vi "CRYO_MASTER_FULL_old.vi"() -> ()   [LabVIEW 2017]
uses:
  LSI218Data.lvclass
  LSI336Data.lvclass
  USBData.lvclass
  6240AData.lvclass
  DMMsData.lvclass
  <vilib>/DAQmx/miscellaneous.llb/DAQmx Fill In Error Info.vi
  <vilib>/DAQmx/create/channels.llb/DAQmx Create Channel (DO-Digital Output).vi
  <vilib>/DAQmx/create/channels.llb/DAQmx Create Channel (AO-Voltage-Basic).vi
  <vilib>/express/express arith-compare/Formula/XNode/ExpressFormulaBlockNode.xnode
  <vilib>/Analysis/NI_AALBase.lvlib
panel:
  in  "Automatic \nScreenshots?":bool=TRUE
  in  "Frontpanel screenshots":bool
  in  "Screenshots interval":i64=3605
  in  "Record interval":i64=10
  out "Cycle #":u32=48
  in  "Measurement Interval (s)":dbl=1.0
  in  "Stop Button":bool
  in  "?":T1(tab)=enum."VALVE/HEATER CTRL"
  out "RUN Identifier":string="20201116_123919_RUNII"
  in  "Base Path (screenshots)":path=path "C:/LabVIEW/DATA/Google/TUCAN Experiments/KEK_cryotests_2019-2020/data/screenshots"
  out "error out (USB6210/6218 AOUT)":errorcluster
  in  "AOUT Labels":string[](array[string])=["PWR400H_I", "PMC183A_I"]
  in  "DOUT Labels":string[](array[string])=["D_V1_NO", "D_V2_NC", "D_CV1", "D_H1"]
  in  "AOUT assignment":tag[](array[tag])=["Dev1/ao0", "Dev1/ao1"]
  out "AO task out":refnum<k21>="20201116_123919_RUNII_AO"
  in  "Analog Out ON?":bool=TRUE
  in  "InstName (USB6218)":string="USB6218"
  in  "USB6218 Config":T2(array[cluster])=[{"Label"="F_1", "FileFormat"="%5.5f", "Active?"=TRUE, "Physical CH"="Dev1/ai0", " terminal\n type"=10083, "ConversionType"={"Type"=enum."SimpleProp", "ConversionParameters"=[0.0, 5.0, 0.0, 500.0]}, "VoltageLimits"=[0.0, 5.0]}, {"Label"="F_2", "FileFormat"="%5.5f", "Active?"=TRUE, "Physical CH"="Dev1/ai1", " terminal\n type"=10083, "ConversionType"={"Type"=enum."SimpleProp", "ConversionParameters"=[0.0, 5.0, 0.0, 200.0]}, "VoltageLimits"=[0.0, 5.0]}, {"Label"="F_3", "FileFormat"="%5.5f", "Active?"=TRUE, "Physical CH"="Dev1/ai2", " terminal\n type"=10083, "ConversionType"={"Type"=enum."SimpleProp", "ConversionParameters"=[0.0, 5.0, 0.0, 200.0]}, "VoltageLimits"=[0.0, 5.0]}, {"Label"="F_4", "FileFormat"="%5.5f", "Active?"=TRUE, "Physical CH"="Dev1/ai3", " terminal\n type"=10083, "ConversionType"={"Type"=enum."SimpleProp", "ConversionParameters"=[0.0, 5.0, 0.0, 500.0]}, "VoltageLimits"=[0.0, 5.0]}, {"Label"="F_5", "FileFormat"="%5.5f", "Active?"=TRUE, "Physical CH"="Dev1/ai4", " terminal\n type"=10083, "ConversionType"={"Type"=enum."SimpleProp", "ConversionParameters"=[0.0, 5.0, 0.0, 500.0]}, "VoltageLimits"=[0.0, 5.0]}, {"Label"="I_CV", "FileFormat"="%3.5f", "Active?"=TRUE, "Physical CH"="Dev1/ai5", " terminal\n type"=10083, "ConversionType"={"Type"=enum."Raw", "ConversionParameters"=[0.0, 0.0, 0.0, 0.0]}, "VoltageLimits"=[0.0, 10.0]}, {"Label"="CV1_answer", "FileFormat"="%3.5f", "Active?"=TRUE, "Physical CH"="Dev1/ai6", " terminal\n type"=10083, "ConversionType"={"Type"=enum."SimpleProp", "ConversionParameters"=[1.0, 5.0, 0.0, 100.0]}, "VoltageLimits"=[0.0, 5.0]}, {"Label"="P_Dewar", "FileFormat"="%5.5e", "Active?"=TRUE, "Physical CH"="Dev1/ai7", " terminal\n type"=10083, "ConversionType"={"Type"=enum."SimpleProp", "ConversionParameters"=[1.0, 5.0, 0.0, 200000.0]}, "VoltageLimits"=[0.0, 5.0]}] {"terminal\n type" items=["Default"=-1, "RSE"=10083, "NRSE"=10078, "Differential"=10106, "Pseudodifferential"=12529]}
  out "error out (USB6218)":errorcluster
  out "error out (USB6210/6218 DOUT)":errorcluster
  out "DOUT task out":refnum<k21>="20201116_123919_DO"
  in  "DOUT Physical CH":tag[](array[tag])=["Dev1/port1/line0", "Dev1/port1/line1", "Dev1/port1/line2", "Dev1/port1/line3"]
  in  "Digital Out ON?":bool=TRUE
  in  "USB6210 Config":T2(array[cluster])=[{"Label"="P_ins", "FileFormat"="%5.5e", "Active?"=TRUE, "Physical CH"="Dev2/ai0", " terminal\n type"=10083, "ConversionType"={"Type"=enum."CC-10_LOG", "ConversionParameters"=[0.5, 9.0, 0.0, 1.0]}, "VoltageLimits"=[0.0, 10.0]}, {"Label"="P_4Kres", "FileFormat"="%5.5e", "Active?"=TRUE, "Physical CH"="Dev2/ai1", " terminal\n type"=10083, "ConversionType"={"Type"=enum."SimpleProp", "ConversionParameters"=[1.0, 5.0, 0.0, 200000.0]}, "VoltageLimits"=[0.0, 5.0]}, {"Label"="P_3HeIN", "FileFormat"="%5.5e", "Active?"=TRUE, "Physical CH"="Dev2/ai2", " terminal\n type"=10083, "ConversionType"={"Type"=enum."SimpleProp", "ConversionParameters"=[1.0, 5.0, 0.0, 200000.0]}, "VoltageLimits"=[0.0, 5.0]}, {"Label"="P_SldRTN", "FileFormat"="%5.5e", "Active?"=TRUE, "Physical CH"="Dev2/ai3", " terminal\n type"=10083, "ConversionType"={"Type"=enum."SimpleProp", "ConversionParameters"=[1.0, 5.0, 0.0, 200000.0]}, "VoltageLimits"=[0.0, 5.0]}, {"Label"="P_3Hepot", "FileFormat"="%5.5e", "Active?"=TRUE, "Physical CH"="Dev2/ai4", " terminal\n type"=10083, "ConversionType"={"Type"=enum."SimpleProp", "ConversionParameters"=[0.0, 10.0, 0.0, 133320.0]}, "VoltageLimits"=[0.0, 10.0]}, {"Label"="P_1Kpot", "FileFormat"="%5.5e", "Active?"=TRUE, "Physical CH"="Dev2/ai5", " terminal\n type"=10083, "ConversionType"={"Type"=enum."SimpleProp", "ConversionParameters"=[0.0, 10.0, 0.0, 133320.0]}, "VoltageLimits"=[0.0, 10.0]}, {"Label"="P_Dewar(old)", "FileFormat"="%5.5e", "Active?"=FALSE, "Physical CH"="Dev2/ai6", " terminal\n type"=10083, "ConversionType"={"Type"=enum."SimpleProp", "ConversionParameters"=[1.0, 5.0, 0.0, 200000.0]}, "VoltageLimits"=[0.0, 5.0]}, {"Label"="DP_HEX4", "FileFormat"="%5.5e", "Active?"=TRUE, "Physical CH"="Dev2/ai7", " terminal\n type"=10083, "ConversionType"={"Type"=enum."SimpleProp", "ConversionParameters"=[1.0, 5.0, 0.0, 1000.0]}, "VoltageLimits"=[0.0, 5.0]}, {"Label"="DP_HEX5", "FileFormat"="%5.5e", "Active?"=TRUE, "Physical CH"="Dev2/ai8", " terminal\n type"=10083, "ConversionType"={"Type"=enum."SimpleProp", "ConversionParameters"=[1.0, 5.0, 0.0, 20000.0]}, "VoltageLimits"=[0.0, 5.0]}, {"Label"="L1", "FileFormat"="%5.5f", "Active?"=TRUE, "Physical CH"="Dev2/ai9", " terminal\n type"=10083, "ConversionType"={"Type"=enum."SimpleProp", "ConversionParameters"=[0.0, 10.0, 0.0, 100.0]}, "VoltageLimits"=[0.0, 10.0]}, {"Label"="L2-1", "FileFormat"="%5.5f", "Active?"=TRUE, "Physical CH"="Dev2/ai10", " terminal\n type"=10083, "ConversionType"={"Type"=enum."SimpleProp", "ConversionParameters"=[0.0, 10.0, 0.0, 100.0]}, "VoltageLimits"=[0.0, 10.0]}, {"Label"="L2-2", "FileFormat"="%5.5f", "Active?"=TRUE, "Physical CH"="Dev2/ai11", " terminal\n type"=10083, "ConversionType"={"Type"=enum."SimpleProp", "ConversionParameters"=[0.0, 10.0, 0.0, 100.0]}, "VoltageLimits"=[0.0, 10.0]}, {"Label"="L3", "FileFormat"="%5.5f", "Active?"=TRUE, "Physical CH"="Dev2/ai12", " terminal\n type"=10083, "ConversionType"={"Type"=enum."SimpleProp", "ConversionParameters"=[0.0, 10.0, 0.0, 100.0]}, "VoltageLimits"=[0.0, 10.0]}, {"Label"="P_HEX7OUT", "FileFormat"="%5.5e", "Active?"=TRUE, "Physical CH"="Dev2/ai13", " terminal\n type"=10083, "ConversionType"={"Type"=enum."SimpleProp", "ConversionParameters"=[1.0, 5.0, 0.0, 200000.0]}, "VoltageLimits"=[0.0, 5.0]}, {"Label"="P_IP", "FileFormat"="%5.5e", "Active?"=TRUE, "Physical CH"="Dev2/ai14", " terminal\n type"=10083, "ConversionType"={"Type"=enum."CC-10_LOG", "ConversionParameters"=[0.5, 9.0, 0.0, 1.0]}, "VoltageLimits"=[0.0, 10.0]}, {"Label"="V_H1", "FileFormat"="%3.5f", "Active?"=TRUE, "Physical CH"="Dev2/ai15", " terminal\n type"=10083, "ConversionType"={"Type"=enum."Raw", "ConversionParameters"=[0.0, 1.0, 0.0, 1.0]}, "VoltageLimits"=[0.0, 10.0]}] {"terminal\n type" items=["Default"=-1, "RSE"=10083, "NRSE"=10078, "Differential"=10106, "Pseudodifferential"=12529]}
  in  "RUN label":string="RUNII"
  in  "Base Path":path=path "C:/LabVIEW/DATA/RUN_2"
  in  "InstName (USB6210)":string="USB6210"
  out "error out (USB6210)":errorcluster
  out "File Refn USB AO":refnum<file>
  out "File Refn USB DO":refnum<file>
  out "error out (LSI336)":errorcluster
  in  "InstName (LSI336)":string="LSI336"
  in  "FileFormat (336)":string="%4.4f"
  in  "LSI336Settings(X,Y)":T3(array[cluster])=[{"LSIName"="LSi336X", "Labels"=["T1K3-1", "T1K3-2", "T3He5", "T3He8"], "SensorLocations"=[enum."T1K3-1", enum."T1K3-2", enum."T3He5", enum."T3He8"], "Active?"=TRUE, "VISA res. name"="GPIB0::6::INSTR"}, {"LSIName"="LSi336Y", "Labels"=["T3He6-1", "T3He6-2", "T3He7-1", "T3He7-2"], "SensorLocations"=[enum."T3He6-1", enum."T3He6-2", enum."T3He7-1", enum."T3He7-2"], "Active?"=TRUE, "VISA res. name"="GPIB0::2::INSTR"}]
  in  "FileFormat (218)":string="%4.4f"
  in  "InstName (LSI218)":string="LSI218"
  in  "LSI218Settings(A-F)":T3(array[cluster])=[{"LSIName"="LSI218A", "Labels"=["T3He10", "T3He1-1", "TTH3", "TTH4", "TTH1", "TTH2", "T4He1", "T1K1"], "SensorLocations"=[enum."T3He10", enum."T3He1-1", enum."TTH3", enum."TTH4", enum."TTH1", enum."TTH2", enum."T4He1", enum."T1K1"], "Active?"=TRUE, "VISA res. name"="GPIB0::7::INSTR"}, {"LSIName"="LSI218B", "Labels"=["N.C.", "N.C.", "N.C.", "N.C.", "T3He2-1", "T3He2-2", "T3He3", "T3He1-4"], "SensorLocations"=[enum."N.C.", enum."N.C.", enum."N.C.", enum."N.C.", enum."T3He2-1", enum."T3He2-2", enum."T3He3", enum."T3He1-4"], "Active?"=TRUE, "VISA res. name"="GPIB0::4::INSTR"}, {"LSIName"="LSI218C", "Labels"=["T4He3-1", "T4He3-2", "T4He3-3", "T4He3-4", "T4He2-1", "T4He2-2", "T4He4", "T4He5"], "SensorLocations"=[enum."T4He3-1", enum."T4He3-2", enum."T4He3-3", enum."T4He3-4", enum."T4He2-1", enum."T4He2-2", enum."T4He4", enum."T4He5"], "Active?"=TRUE, "VISA res. name"="GPIB0::3::INSTR"}, {"LSIName"="LSI218D", "Labels"=["T4He6", "T4He9", "T3He1-2", "T3He1-3", "T4He7", "T4He8", "T4He10", "T1K6"], "SensorLocations"=[enum."T4He6", enum."T4He9", enum."T3He1-2", enum."T3He1-3", enum."T4He7", enum."T4He8", enum."T4He10", enum."T1K6"], "Active?"=TRUE, "VISA res. name"="GPIB0::5::INSTR"}, {"LSIName"="LSI218E", "Labels"=["TIP1", "N.C.", "TIP2", "N.C.", "TIP3", "TIP4", "TIP5", "N.C."], "SensorLocations"=[enum."TIP1", enum."N.C.", enum."TIP2", enum."N.C.", enum."TIP3", enum."TIP4", enum."TIP5", enum."N.C."], "Active?"=TRUE, "VISA res. name"="GPIB0::11::INSTR"}, {"LSIName"="LSI218F", "Labels"=["T1K2", "T1K4", "T1K5", "T3He4", "T3He9", "TIP6", "N.C.", "N.C."], "SensorLocations"=[enum."T1K2", enum."T1K4", enum."T1K5", enum."T3He4", enum."T3He9", enum."TIP6", enum."N.C.", enum."N.C."], "Active?"=TRUE, "VISA res. name"="GPIB0::8::INSTR"}]
  out "error out (LSI218)":errorcluster
  out "RUN Identifier 2":string="20201116_123919_RUNII" caption="RUN Identifier"
  out "Graph 3":T4(graph)=[{"TimeArray"=[timestamp(3688342761.3994594 s since 1904-01-01), timestamp(3688342762.4680505 s since 1904-01-01), timestamp(3688342763.4675946 s since 1904-01-01), timestamp(3688342764.4676514 s since 1904-01-01), timestamp(3688342765.4686737 s since 1904-01-01), timestamp(3688342766.469984 s since 1904-01-01), timestamp(3688342767.470159 s since 1904-01-01), timestamp(3688342768.47213 s since 1904-01-01), timestamp(3688342769.8238606 s since 1904-01-01), timestamp(3688342770.8245606 s since 1904-01-01), timestamp(3688342771.8237367 s since 1904-01-01), timestamp(3688342772.8240294 s since 1904-01-01), timestamp(3688342773.823701 s since 1904-01-01), timestamp(3688342774.8247466 s since 1904-01-01), timestamp(3688342775.8255386 s since 1904-01-01), timestamp(3688342776.8254576 s since 1904-01-01), timestamp(3688342777.825836 s since 1904-01-01), timestamp(3688342778.8261266 s since 1904-01-01), timestamp(3688342779.826581 s since 1904-01-01), timestamp(3688342780.8273554 s since 1904-01-01), timestamp(3688342781.826626 s since 1904-01-01), timestamp(3688342782.8268657 s since 1904-01-01), timestamp(3688342783.8258696 s since 1904-01-01), timestamp(3688342784.825906 s since 1904-01-01), timestamp(3688342785.825819 s since 1904-01-01), timestamp(3688342786.827296 s since 1904-01-01), timestamp(3688342787.829418 s since 1904-01-01), timestamp(3688342788.8291 s since 1904-01-01), timestamp(3688342789.8296633 s since 1904-01-01), timestamp(3688342790.829848 s since 1904-01-01), timestamp(3688342791.829139 s since 1904-01-01), timestamp(3688342792.8296423 s since 1904-01-01), timestamp(3688342793.831637 s since 1904-01-01), timestamp(3688342794.8306546 s since 1904-01-01), timestamp(3688342795.829824 s since 1904-01-01), timestamp(3688342796.830819 s since 1904-01-01), timestamp(3688342798.0479465 s since 1904-01-01), timestamp(3688342799.047389 s since 1904-01-01), timestamp(3688342800.047347 s since 1904-01-01), timestamp(3688342801.0487537 s since 1904-01-01), timestamp(3688342802.047892 s since 1904-01-01), timestamp(3688342803.047963 s since 1904-01-01), timestamp(3688342804.0478578 s since 1904-01-01), timestamp(3688342805.0488462 s since 1904-01-01), timestamp(3688342806.0497985 s since 1904-01-01), timestamp(3688342807.0502543 s since 1904-01-01), timestamp(3688342808.049495 s since 1904-01-01), timestamp(3688342809.0488415 s since 1904-01-01)], "DataArray"=[1.6108772064644081, 1.4727858772132323, 1.1538606722402807, 1.28208833184731, 1.7785595282840228, 1.0256330125875925, 1.6897865359634758, 0.7987686882211862, 0.8809659041921434, 1.3248308864318687, 1.1111181148543707, 1.2492094468908674, 0.8415112314716219, 1.2031790040723394, 0.8645264589454551, 1.702938093987531, 0.8711022389190866, 1.7686958683374852, 1.6569076467914272, 1.3248308880823247, 1.1275575630145545, 1.9002114182612835, 0.9006932376829025, 1.4892253229450763, 0.976314680985114, 1.5221042083621306, 0.6606773585654712, 1.3807249976849918, 1.4366191035745401, 1.4333312156222522, 1.4366191049902393, 1.8180141959680036, 1.1505727850948726, 0.7330109051260003, 1.7917110860245415, 1.1538606736707524, 1.5056647632332703, 0.9269963444433174, 1.7128017563643017, 1.449770660594799, 1.5681346563036929, 0.8283596875451974, 0.6902683536947601, 0.8415112382027863, 1.6108772080587708, 1.7785595285218954, 1.5418315461474963, 1.236057890033779]}, {"TimeArray"=[timestamp(3688342761.3994594 s since 1904-01-01), timestamp(3688342762.4680505 s since 1904-01-01), timestamp(3688342763.4675946 s since 1904-01-01), timestamp(3688342764.4676514 s since 1904-01-01), timestamp(3688342765.4686737 s since 1904-01-01), timestamp(3688342766.469984 s since 1904-01-01), timestamp(3688342767.470159 s since 1904-01-01), timestamp(3688342768.47213 s since 1904-01-01), timestamp(3688342769.8238606 s since 1904-01-01), timestamp(3688342770.8245606 s since 1904-01-01), timestamp(3688342771.8237367 s since 1904-01-01), timestamp(3688342772.8240294 s since 1904-01-01), timestamp(3688342773.823701 s since 1904-01-01), timestamp(3688342774.8247466 s since 1904-01-01), timestamp(3688342775.8255386 s since 1904-01-01), timestamp(3688342776.8254576 s since 1904-01-01), timestamp(3688342777.825836 s since 1904-01-01), timestamp(3688342778.8261266 s since 1904-01-01), timestamp(3688342779.826581 s since 1904-01-01), timestamp(3688342780.8273554 s since 1904-01-01), timestamp(3688342781.826626 s since 1904-01-01), timestamp(3688342782.8268657 s since 1904-01-01), timestamp(3688342783.8258696 s since 1904-01-01), timestamp(3688342784.825906 s since 1904-01-01), timestamp(3688342785.825819 s since 1904-01-01), timestamp(3688342786.827296 s since 1904-01-01), timestamp(3688342787.829418 s since 1904-01-01), timestamp(3688342788.8291 s since 1904-01-01), timestamp(3688342789.8296633 s since 1904-01-01), timestamp(3688342790.829848 s since 1904-01-01), timestamp(3688342791.829139 s since 1904-01-01), timestamp(3688342792.8296423 s since 1904-01-01), timestamp(3688342793.831637 s since 1904-01-01), timestamp(3688342794.8306546 s since 1904-01-01), timestamp(3688342795.829824 s since 1904-01-01), timestamp(3688342796.830819 s since 1904-01-01), timestamp(3688342798.0479465 s since 1904-01-01), timestamp(3688342799.047389 s since 1904-01-01), timestamp(3688342800.047347 s since 1904-01-01), timestamp(3688342801.0487537 s since 1904-01-01), timestamp(3688342802.047892 s since 1904-01-01), timestamp(3688342803.047963 s since 1904-01-01), timestamp(3688342804.0478578 s since 1904-01-01), timestamp(3688342805.0488462 s since 1904-01-01), timestamp(3688342806.0497985 s since 1904-01-01), timestamp(3688342807.0502543 s since 1904-01-01), timestamp(3688342808.049495 s since 1904-01-01), timestamp(3688342809.0488415 s since 1904-01-01)], "DataArray"=[0.11960383538282587, 0.12354930467748859, 0.16957974721691593, 0.3168771630474284, 0.10513712477879456, 0.14327663545986008, -0.056627000773362635, 0.020967174002287814, -0.09345135530386744, 0.06173699470083205, 0.40630773776805706, 0.03543388286570193, -0.015857179683996525, 0.43787147030971574, 0.1353857036464915, 0.2813679649924926, 0.06305215107903633, 0.3707985383052794, 0.16168881415673564, 0.05910668305857897, 0.07488855063108274, -0.05925731348622698, 0.08804010289037423, 0.3655379148996485, 0.152482725397677, 0.42603506628065013, 0.3537015180628369, 0.3168771643021264, 0.084094637595031, 0.10776743816760453, 0.31687716261188875, 0.2116647226957259, 0.007815619052014, 0.09724619411048441, -0.14868788814255518, 0.26032547695418784, 0.21955565491787643, 0.26690125441051665, 0.4457624026836094, 0.1774706797542605, 0.114343214789281, 0.0380641963143703, -0.1026574444303443, 0.013076240296714503, 0.1840464575827528, 0.055161216108252864, 0.06042183752267505, 0.32608325247707837]}, {"TimeArray"=[timestamp(3688342761.3994594 s since 1904-01-01), timestamp(3688342762.4680505 s since 1904-01-01), timestamp(3688342763.4675946 s since 1904-01-01), timestamp(3688342764.4676514 s since 1904-01-01), timestamp(3688342765.4686737 s since 1904-01-01), timestamp(3688342766.469984 s since 1904-01-01), timestamp(3688342767.470159 s since 1904-01-01), timestamp(3688342768.47213 s since 1904-01-01), timestamp(3688342769.8238606 s since 1904-01-01), timestamp(3688342770.8245606 s since 1904-01-01), timestamp(3688342771.8237367 s since 1904-01-01), timestamp(3688342772.8240294 s since 1904-01-01), timestamp(3688342773.823701 s since 1904-01-01), timestamp(3688342774.8247466 s since 1904-01-01), timestamp(3688342775.8255386 s since 1904-01-01), timestamp(3688342776.8254576 s since 1904-01-01), timestamp(3688342777.825836 s since 1904-01-01), timestamp(3688342778.8261266 s since 1904-01-01), timestamp(3688342779.826581 s since 1904-01-01), timestamp(3688342780.8273554 s since 1904-01-01), timestamp(3688342781.826626 s since 1904-01-01), timestamp(3688342782.8268657 s since 1904-01-01), timestamp(3688342783.8258696 s since 1904-01-01), timestamp(3688342784.825906 s since 1904-01-01), timestamp(3688342785.825819 s since 1904-01-01), timestamp(3688342786.827296 s since 1904-01-01), timestamp(3688342787.829418 s since 1904-01-01), timestamp(3688342788.8291 s since 1904-01-01), timestamp(3688342789.8296633 s since 1904-01-01), timestamp(3688342790.829848 s since 1904-01-01), timestamp(3688342791.829139 s since 1904-01-01), timestamp(3688342792.8296423 s since 1904-01-01), timestamp(3688342793.831637 s since 1904-01-01), timestamp(3688342794.8306546 s since 1904-01-01), timestamp(3688342795.829824 s since 1904-01-01), timestamp(3688342796.830819 s since 1904-01-01), timestamp(3688342798.0479465 s since 1904-01-01), timestamp(3688342799.047389 s since 1904-01-01), timestamp(3688342800.047347 s since 1904-01-01), timestamp(3688342801.0487537 s since 1904-01-01), timestamp(3688342802.047892 s since 1904-01-01), timestamp(3688342803.047963 s since 1904-01-01), timestamp(3688342804.0478578 s since 1904-01-01), timestamp(3688342805.0488462 s since 1904-01-01), timestamp(3688342806.0497985 s since 1904-01-01), timestamp(3688342807.0502543 s since 1904-01-01), timestamp(3688342808.049495 s since 1904-01-01), timestamp(3688342809.0488415 s since 1904-01-01)], "DataArray"=[0.19719801289443417, 0.3234529413982592, 0.41025320470314475, 0.35501667385679236, 0.08277948336150942, 0.1866767679337933, 0.03674904061937184, 0.11434321402546777, 0.22481627750062233, 0.47995644469336163, 0.5549203093056583, 0.29320436503981057, 0.10382197109764235, 0.46680489114965856, 0.36553791656749685, 0.37605916077701856, 0.3721136950929542, 0.09856134863620536, 0.282683121071797, 0.16957974638882117, 0.28268311956998077, -0.015857180631994205, 0.30241045223936386, 0.13275539146300835, 0.19325254588015484, 0.3984168045158203, 0.5391384442450727, 0.3971016486305656, 0.17878583614480142, 0.43129569272124, 0.47469582441796065, -0.01848749114242587, 0.11039774877546588, 0.31950747311050975, 0.2392829882600312, 0.5102050229214992, 0.24717392215355527, 0.5036292443284728, 0.30372560924621067, 0.293204364993237, 0.19851316847145212, 0.7219450557978133, 0.04332481675159766, 0.4273502264943859, 0.27347703224226, -0.006651091545683108, 0.16300396733772582, 0.27610734304609297]}, {"TimeArray"=[timestamp(3688342761.3994594 s since 1904-01-01), timestamp(3688342762.4680505 s since 1904-01-01), timestamp(3688342763.4675946 s since 1904-01-01), timestamp(3688342764.4676514 s since 1904-01-01), timestamp(3688342765.4686737 s since 1904-01-01), timestamp(3688342766.469984 s since 1904-01-01), timestamp(3688342767.470159 s since 1904-01-01), timestamp(3688342768.47213 s since 1904-01-01), timestamp(3688342769.8238606 s since 1904-01-01), timestamp(3688342770.8245606 s since 1904-01-01), timestamp(3688342771.8237367 s since 1904-01-01), timestamp(3688342772.8240294 s since 1904-01-01), timestamp(3688342773.823701 s since 1904-01-01), timestamp(3688342774.8247466 s since 1904-01-01), timestamp(3688342775.8255386 s since 1904-01-01), timestamp(3688342776.8254576 s since 1904-01-01), timestamp(3688342777.825836 s since 1904-01-01), timestamp(3688342778.8261266 s since 1904-01-01), timestamp(3688342779.826581 s since 1904-01-01), timestamp(3688342780.8273554 s since 1904-01-01), timestamp(3688342781.826626 s since 1904-01-01), timestamp(3688342782.8268657 s since 1904-01-01), timestamp(3688342783.8258696 s since 1904-01-01), timestamp(3688342784.825906 s since 1904-01-01), timestamp(3688342785.825819 s since 1904-01-01), timestamp(3688342786.827296 s since 1904-01-01), timestamp(3688342787.829418 s since 1904-01-01), timestamp(3688342788.8291 s since 1904-01-01), timestamp(3688342789.8296633 s since 1904-01-01), timestamp(3688342790.829848 s since 1904-01-01), timestamp(3688342791.829139 s since 1904-01-01), timestamp(3688342792.8296423 s since 1904-01-01), timestamp(3688342793.831637 s since 1904-01-01), timestamp(3688342794.8306546 s since 1904-01-01), timestamp(3688342795.829824 s since 1904-01-01), timestamp(3688342796.830819 s since 1904-01-01), timestamp(3688342798.0479465 s since 1904-01-01), timestamp(3688342799.047389 s since 1904-01-01), timestamp(3688342800.047347 s since 1904-01-01), timestamp(3688342801.0487537 s since 1904-01-01), timestamp(3688342802.047892 s since 1904-01-01), timestamp(3688342803.047963 s since 1904-01-01), timestamp(3688342804.0478578 s since 1904-01-01), timestamp(3688342805.0488462 s since 1904-01-01), timestamp(3688342806.0497985 s since 1904-01-01), timestamp(3688342807.0502543 s since 1904-01-01), timestamp(3688342808.049495 s since 1904-01-01), timestamp(3688342809.0488415 s since 1904-01-01)], "DataArray"=[-8.8117305470801, -8.611169313327453, -8.785427429519835, -9.633702805164498, -8.772275883378784, -8.920230878437964, -7.933864177873465, -7.756318171036431, -8.183743745254892, -8.699942315071391, -8.959685549532404, -8.683502874153833, -8.36128975034523, -8.739396983469396, -8.20675896381145, -8.427047526402006, -7.808924396791847, -9.295050229778404, -8.23634996633052, -8.41718386312757, -8.07195551659595, -7.6774088373668965, -7.749742396156548, -8.279092521170103, -8.10483440461572, -8.831457878899462, -9.27532289384464, -9.120792109971513, -7.831939618345252, -9.48574779160318, -9.683021136151854, -8.413895971885601, -8.085107074198529, -7.924000508555038, -7.595211611507303, -8.81830632687022, -8.31525930182675, -8.736109095904842, -9.702748470003478, -9.081337441634272, -7.989758296191559, -8.542123642001318, -7.108604041882277, -7.187513380811203, -9.581096575868242, -8.374441303730787, -8.496093212698424, -8.229774188754428]}, {"TimeArray"=[timestamp(3688342761.3994594 s since 1904-01-01), timestamp(3688342762.4680505 s since 1904-01-01), timestamp(3688342763.4675946 s since 1904-01-01), timestamp(3688342764.4676514 s since 1904-01-01), timestamp(3688342765.4686737 s since 1904-01-01), timestamp(3688342766.469984 s since 1904-01-01), timestamp(3688342767.470159 s since 1904-01-01), timestamp(3688342768.47213 s since 1904-01-01), timestamp(3688342769.8238606 s since 1904-01-01), timestamp(3688342770.8245606 s since 1904-01-01), timestamp(3688342771.8237367 s since 1904-01-01), timestamp(3688342772.8240294 s since 1904-01-01), timestamp(3688342773.823701 s since 1904-01-01), timestamp(3688342774.8247466 s since 1904-01-01), timestamp(3688342775.8255386 s since 1904-01-01), timestamp(3688342776.8254576 s since 1904-01-01), timestamp(3688342777.825836 s since 1904-01-01), timestamp(3688342778.8261266 s since 1904-01-01), timestamp(3688342779.826581 s since 1904-01-01), timestamp(3688342780.8273554 s since 1904-01-01), timestamp(3688342781.826626 s since 1904-01-01), timestamp(3688342782.8268657 s since 1904-01-01), timestamp(3688342783.8258696 s since 1904-01-01), timestamp(3688342784.825906 s since 1904-01-01), timestamp(3688342785.825819 s since 1904-01-01), timestamp(3688342786.827296 s since 1904-01-01), timestamp(3688342787.829418 s since 1904-01-01), timestamp(3688342788.8291 s since 1904-01-01), timestamp(3688342789.8296633 s since 1904-01-01), timestamp(3688342790.829848 s since 1904-01-01), timestamp(3688342791.829139 s since 1904-01-01), timestamp(3688342792.8296423 s since 1904-01-01), timestamp(3688342793.831637 s since 1904-01-01), timestamp(3688342794.8306546 s since 1904-01-01), timestamp(3688342795.829824 s since 1904-01-01), timestamp(3688342796.830819 s since 1904-01-01), timestamp(3688342798.0479465 s since 1904-01-01), timestamp(3688342799.047389 s since 1904-01-01), timestamp(3688342800.047347 s since 1904-01-01), timestamp(3688342801.0487537 s since 1904-01-01), timestamp(3688342802.047892 s since 1904-01-01), timestamp(3688342803.047963 s since 1904-01-01), timestamp(3688342804.0478578 s since 1904-01-01), timestamp(3688342805.0488462 s since 1904-01-01), timestamp(3688342806.0497985 s since 1904-01-01), timestamp(3688342807.0502543 s since 1904-01-01), timestamp(3688342808.049495 s since 1904-01-01), timestamp(3688342809.0488415 s since 1904-01-01)], "DataArray"=[25.42834097532839, 24.86611211032151, 25.507250294604013, 25.129143157252333, 25.579583820368846, 25.043658067331226, 26.286479774866073, 25.80316022068847, 26.358813307865177, 24.87597576883828, 24.58006584160019, 25.240931356366875, 25.586159610342886, 24.67870248438199, 25.918236307585516, 25.471083526447114, 25.704523579221565, 24.5636263966979, 25.540129173409465, 25.257370793132907, 25.448068304775234, 26.15496424988605, 25.28367389255778, 25.826175439613337, 25.58287171880491, 24.889127324747573, 23.883033555139072, 24.55376273747171, 25.990569845070805, 25.408613646662076, 24.132913048272638, 25.536841282754608, 26.227297790428917, 26.043176056850676, 25.582871718122018, 24.68856614483606, 25.6552052559632, 24.58006583695763, 24.626096274245686, 24.879263660377774, 25.740690349871215, 24.504444409982383, 26.365389089597326, 26.010297173875607, 25.066673284606118, 25.717675133782908, 25.54341705535066, 25.19818880738261]}, {"TimeArray"=[timestamp(3688342761.3994594 s since 1904-01-01), timestamp(3688342762.4680505 s since 1904-01-01), timestamp(3688342763.4675946 s since 1904-01-01), timestamp(3688342764.4676514 s since 1904-01-01), timestamp(3688342765.4686737 s since 1904-01-01), timestamp(3688342766.469984 s since 1904-01-01), timestamp(3688342767.470159 s since 1904-01-01), timestamp(3688342768.47213 s since 1904-01-01), timestamp(3688342769.8238606 s since 1904-01-01), timestamp(3688342770.8245606 s since 1904-01-01), timestamp(3688342771.8237367 s since 1904-01-01), timestamp(3688342772.8240294 s since 1904-01-01), timestamp(3688342773.823701 s since 1904-01-01), timestamp(3688342774.8247466 s since 1904-01-01), timestamp(3688342775.8255386 s since 1904-01-01), timestamp(3688342776.8254576 s since 1904-01-01), timestamp(3688342777.825836 s since 1904-01-01), timestamp(3688342778.8261266 s since 1904-01-01), timestamp(3688342779.826581 s since 1904-01-01), timestamp(3688342780.8273554 s since 1904-01-01), timestamp(3688342781.826626 s since 1904-01-01), timestamp(3688342782.8268657 s since 1904-01-01), timestamp(3688342783.8258696 s since 1904-01-01), timestamp(3688342784.825906 s since 1904-01-01), timestamp(3688342785.825819 s since 1904-01-01), timestamp(3688342786.827296 s since 1904-01-01), timestamp(3688342787.829418 s since 1904-01-01), timestamp(3688342788.8291 s since 1904-01-01), timestamp(3688342789.8296633 s since 1904-01-01), timestamp(3688342790.829848 s since 1904-01-01), timestamp(3688342791.829139 s since 1904-01-01), timestamp(3688342792.8296423 s since 1904-01-01), timestamp(3688342793.831637 s since 1904-01-01), timestamp(3688342794.8306546 s since 1904-01-01), timestamp(3688342795.829824 s since 1904-01-01), timestamp(3688342796.830819 s since 1904-01-01), timestamp(3688342798.0479465 s since 1904-01-01), timestamp(3688342799.047389 s since 1904-01-01), timestamp(3688342800.047347 s since 1904-01-01), timestamp(3688342801.0487537 s since 1904-01-01), timestamp(3688342802.047892 s since 1904-01-01), timestamp(3688342803.047963 s since 1904-01-01), timestamp(3688342804.0478578 s since 1904-01-01), timestamp(3688342805.0488462 s since 1904-01-01), timestamp(3688342806.0497985 s since 1904-01-01), timestamp(3688342807.0502543 s since 1904-01-01), timestamp(3688342808.049495 s since 1904-01-01), timestamp(3688342809.0488415 s since 1904-01-01)], "DataArray"=[-0.005193268383660984, -0.004930182610743403, -0.007561039877274372, -0.007824125581124733, 0.0005946176173860784, 0.0009892461834888455, -0.008350297054780385, 0.0020415890984940926, -0.010586525749650461, -0.0165717259712373, -0.004009382596067648, 0.0044751320298084376, -0.006508696976678557, -0.003746296849714206, 0.01644553246086406, 0.018418675382905786, 0.006777132117386087, 0.022299189798510845, 0.01986564686698383, 0.0103945608264739, 0.015722046716312395, 0.015590503844082615, 0.007961017869320528, 0.01703747532627037, 0.019668332547804077, 0.02052336112517377, 0.01598513245021415, 0.018089818237418558, 0.0174978753332058, 0.019339475400628702, 0.013946218060777175, 0.024206561247617227, 0.027823989933317538, 0.019142161099012175, 0.008355646456888863, 0.021838789776919672, 0.016379761005772927, 0.019931418285493475, 0.028284389977942748, 0.026377018469227166, 0.018155589606191617, -0.0012469824561334246, 0.009473760777586143, 0.010328789405961273, 0.025850847009992406, 0.020720675452570142, 0.021509932578620914, 0.004212046304753189]}, {"TimeArray"=[timestamp(3688342761.3994594 s since 1904-01-01), timestamp(3688342762.4680505 s since 1904-01-01), timestamp(3688342763.4675946 s since 1904-01-01), timestamp(3688342764.4676514 s since 1904-01-01), timestamp(3688342765.4686737 s since 1904-01-01), timestamp(3688342766.469984 s since 1904-01-01), timestamp(3688342767.470159 s since 1904-01-01), timestamp(3688342768.47213 s since 1904-01-01), timestamp(3688342769.8238606 s since 1904-01-01), timestamp(3688342770.8245606 s since 1904-01-01), timestamp(3688342771.8237367 s since 1904-01-01), timestamp(3688342772.8240294 s since 1904-01-01), timestamp(3688342773.823701 s since 1904-01-01), timestamp(3688342774.8247466 s since 1904-01-01), timestamp(3688342775.8255386 s since 1904-01-01), timestamp(3688342776.8254576 s since 1904-01-01), timestamp(3688342777.825836 s since 1904-01-01), timestamp(3688342778.8261266 s since 1904-01-01), timestamp(3688342779.826581 s since 1904-01-01), timestamp(3688342780.8273554 s since 1904-01-01), timestamp(3688342781.826626 s since 1904-01-01), timestamp(3688342782.8268657 s since 1904-01-01), timestamp(3688342783.8258696 s since 1904-01-01), timestamp(3688342784.825906 s since 1904-01-01), timestamp(3688342785.825819 s since 1904-01-01), timestamp(3688342786.827296 s since 1904-01-01), timestamp(3688342787.829418 s since 1904-01-01), timestamp(3688342788.8291 s since 1904-01-01), timestamp(3688342789.8296633 s since 1904-01-01), timestamp(3688342790.829848 s since 1904-01-01), timestamp(3688342791.829139 s since 1904-01-01), timestamp(3688342792.8296423 s since 1904-01-01), timestamp(3688342793.831637 s since 1904-01-01), timestamp(3688342794.8306546 s since 1904-01-01), timestamp(3688342795.829824 s since 1904-01-01), timestamp(3688342796.830819 s since 1904-01-01), timestamp(3688342798.0479465 s since 1904-01-01), timestamp(3688342799.047389 s since 1904-01-01), timestamp(3688342800.047347 s since 1904-01-01), timestamp(3688342801.0487537 s since 1904-01-01), timestamp(3688342802.047892 s since 1904-01-01), timestamp(3688342803.047963 s since 1904-01-01), timestamp(3688342804.0478578 s since 1904-01-01), timestamp(3688342805.0488462 s since 1904-01-01), timestamp(3688342806.0497985 s since 1904-01-01), timestamp(3688342807.0502543 s since 1904-01-01), timestamp(3688342808.049495 s since 1904-01-01), timestamp(3688342809.0488415 s since 1904-01-01)], "DataArray"=[101763.76778005705, 101441.5552574628, 101712.80559595322, 101605.94940418932, 102048.16965721699, 102148.45008278092, 101822.94967516132, 102820.8221420409, 101765.41172578087, 101411.96430850294, 102064.60907132704, 102385.17765603494, 102021.8665918818, 102113.92731541373, 102342.43517662614, 101952.82105008146, 101640.47217360992, 101982.41199679034, 101883.77551160513, 101275.51716733717, 101554.98721685537, 101314.97176370079, 101619.10093268016, 102457.51108097668, 101859.11638700173, 101990.63170464033, 101625.67670103439, 101686.50253584248, 102230.6471546882, 102110.63943060939, 101563.20692537277, 102686.0189403731, 102615.32945958685, 102125.43490180184, 101106.19119599719, 101730.88895455986, 101977.48017289658, 101563.20692370029, 102720.54171254052, 101992.275644626, 101596.08575338517, 101114.41090367321, 101762.12384323322, 101748.97231164195, 102429.56407407322, 102166.53343982312, 102163.24555458283, 102197.76832945186]}] caption="XY Graph"
  out "Graph 1":T4(graph)=[{"TimeArray"=[timestamp(3688342761.39444 s since 1904-01-01), timestamp(3688342762.463024 s since 1904-01-01), timestamp(3688342763.463638 s since 1904-01-01), timestamp(3688342764.463637 s since 1904-01-01), timestamp(3688342765.464684 s since 1904-01-01), timestamp(3688342766.465038 s since 1904-01-01), timestamp(3688342767.4661665 s since 1904-01-01), timestamp(3688342768.4671426 s since 1904-01-01), timestamp(3688342769.818876 s since 1904-01-01), timestamp(3688342770.819616 s since 1904-01-01), timestamp(3688342771.819715 s since 1904-01-01), timestamp(3688342772.8190737 s since 1904-01-01), timestamp(3688342773.819743 s since 1904-01-01), timestamp(3688342774.820112 s since 1904-01-01), timestamp(3688342775.820584 s since 1904-01-01), timestamp(3688342776.8214664 s since 1904-01-01), timestamp(3688342777.821848 s since 1904-01-01), timestamp(3688342778.822177 s since 1904-01-01), timestamp(3688342779.8225975 s since 1904-01-01), timestamp(3688342780.8223686 s since 1904-01-01), timestamp(3688342781.8226385 s since 1904-01-01), timestamp(3688342782.8219137 s since 1904-01-01), timestamp(3688342783.8218846 s since 1904-01-01), timestamp(3688342784.821887 s since 1904-01-01), timestamp(3688342785.821828 s since 1904-01-01), timestamp(3688342786.8223386 s since 1904-01-01), timestamp(3688342787.825325 s since 1904-01-01), timestamp(3688342788.8251424 s since 1904-01-01), timestamp(3688342789.825672 s since 1904-01-01), timestamp(3688342790.824856 s since 1904-01-01), timestamp(3688342791.8251505 s since 1904-01-01), timestamp(3688342792.8256593 s since 1904-01-01), timestamp(3688342793.8266897 s since 1904-01-01), timestamp(3688342794.826625 s since 1904-01-01), timestamp(3688342795.825836 s since 1904-01-01), timestamp(3688342796.826832 s since 1904-01-01), timestamp(3688342798.0429673 s since 1904-01-01), timestamp(3688342799.0433993 s since 1904-01-01), timestamp(3688342800.043396 s since 1904-01-01), timestamp(3688342801.0437655 s since 1904-01-01), timestamp(3688342802.0438714 s since 1904-01-01), timestamp(3688342803.043973 s since 1904-01-01), timestamp(3688342804.043901 s since 1904-01-01), timestamp(3688342805.044822 s since 1904-01-01), timestamp(3688342806.0448112 s since 1904-01-01), timestamp(3688342807.045269 s since 1904-01-01), timestamp(3688342808.0455375 s since 1904-01-01), timestamp(3688342809.0448914 s since 1904-01-01)], "DataArray"=[0.0016985076469113389, 0.0016856962957262024, 0.001682126465642948, 0.001715567839314439, 0.0016892737021061356, 0.0016856962957120887, 0.001702112241654899, 0.0017052079822400363, 0.0016933714637543337, 0.0017072749367236463, 0.0016826359779464751, 0.0016872285413077606, 0.0016821264654510507, 0.0016780559153745326, 0.0016765319999805606, 0.0016790726286288712, 0.0016897853794054498, 0.0016811079031505553, 0.0016760243357404382, 0.001691833639435517, 0.0016938843822185505, 0.0017093443965102329, 0.0017129719893116283, 0.0017129719890873456, 0.0016938843822442617, 0.0016959376109104611, 0.0016785641952298419, 0.0017160874811014547, 0.0017021122417920991, 0.0017072749366225796, 0.0016892737021326888, 0.0016918336397340093, 0.0016933714635912413, 0.001678564194927532, 0.001717647351208853, 0.0016985076469424835, 0.001697993328234986, 0.001678564194898545, 0.0016918336395347422, 0.0016949106856096797, 0.0016816171071247375, 0.0016877395991853987, 0.0016867176382062941, 0.0017077920665341275, 0.001709344396578268, 0.0017166072803434422, 0.001694910685758757, 0.001713490844762899]}, {"TimeArray"=[timestamp(3688342761.39444 s since 1904-01-01), timestamp(3688342762.463024 s since 1904-01-01), timestamp(3688342763.463638 s since 1904-01-01), timestamp(3688342764.463637 s since 1904-01-01), timestamp(3688342765.464684 s since 1904-01-01), timestamp(3688342766.465038 s since 1904-01-01), timestamp(3688342767.4661665 s since 1904-01-01), timestamp(3688342768.4671426 s since 1904-01-01), timestamp(3688342769.818876 s since 1904-01-01), timestamp(3688342770.819616 s since 1904-01-01), timestamp(3688342771.819715 s since 1904-01-01), timestamp(3688342772.8190737 s since 1904-01-01), timestamp(3688342773.819743 s since 1904-01-01), timestamp(3688342774.820112 s since 1904-01-01), timestamp(3688342775.820584 s since 1904-01-01), timestamp(3688342776.8214664 s since 1904-01-01), timestamp(3688342777.821848 s since 1904-01-01), timestamp(3688342778.822177 s since 1904-01-01), timestamp(3688342779.8225975 s since 1904-01-01), timestamp(3688342780.8223686 s since 1904-01-01), timestamp(3688342781.8226385 s since 1904-01-01), timestamp(3688342782.8219137 s since 1904-01-01), timestamp(3688342783.8218846 s since 1904-01-01), timestamp(3688342784.821887 s since 1904-01-01), timestamp(3688342785.821828 s since 1904-01-01), timestamp(3688342786.8223386 s since 1904-01-01), timestamp(3688342787.825325 s since 1904-01-01), timestamp(3688342788.8251424 s since 1904-01-01), timestamp(3688342789.825672 s since 1904-01-01), timestamp(3688342790.824856 s since 1904-01-01), timestamp(3688342791.8251505 s since 1904-01-01), timestamp(3688342792.8256593 s since 1904-01-01), timestamp(3688342793.8266897 s since 1904-01-01), timestamp(3688342794.826625 s since 1904-01-01), timestamp(3688342795.825836 s since 1904-01-01), timestamp(3688342796.826832 s since 1904-01-01), timestamp(3688342798.0429673 s since 1904-01-01), timestamp(3688342799.0433993 s since 1904-01-01), timestamp(3688342800.043396 s since 1904-01-01), timestamp(3688342801.0437655 s since 1904-01-01), timestamp(3688342802.0438714 s since 1904-01-01), timestamp(3688342803.043973 s since 1904-01-01), timestamp(3688342804.043901 s since 1904-01-01), timestamp(3688342805.044822 s since 1904-01-01), timestamp(3688342806.0448112 s since 1904-01-01), timestamp(3688342807.045269 s since 1904-01-01), timestamp(3688342808.0455375 s since 1904-01-01), timestamp(3688342809.0448914 s since 1904-01-01)], "DataArray"=[101832.16872606815, 101865.05725721586, 101930.83432063498, 102022.92221153466, 101886.43480239325, 101893.01250845697, 101917.67890710325, 102090.34370130418, 101930.83432102836, 101925.90103834363, 101820.6577388149, 101919.32333270369, 101893.01250808984, 101911.10120015097, 101958.78957279451, 101945.63415735995, 101975.23383811218, 101929.18989874606, 101787.76920710821, 101911.10120028359, 101893.01250978821, 101934.12317371284, 101873.2793909497, 101835.45757890653, 101912.74562778191, 101993.32253005449, 101904.52349626606, 101916.03448062438, 101930.8343234091, 101950.56744309909, 101833.81315271331, 101981.81154448308, 101891.36808722572, 101957.14514474105, 102044.2997573318, 101948.92301428551, 101907.81234645745, 101993.32253287372, 101868.34611126423, 101939.05645180488, 102022.92220923673, 102031.14434168766, 101929.18989208799, 101962.07842325009, 101833.81315122647, 101971.94498410224, 102072.25500773212, 102021.27778594472]}, {"TimeArray"=[timestamp(3688342761.39444 s since 1904-01-01), timestamp(3688342762.463024 s since 1904-01-01), timestamp(3688342763.463638 s since 1904-01-01), timestamp(3688342764.463637 s since 1904-01-01), timestamp(3688342765.464684 s since 1904-01-01), timestamp(3688342766.465038 s since 1904-01-01), timestamp(3688342767.4661665 s since 1904-01-01), timestamp(3688342768.4671426 s since 1904-01-01), timestamp(3688342769.818876 s since 1904-01-01), timestamp(3688342770.819616 s since 1904-01-01), timestamp(3688342771.819715 s since 1904-01-01), timestamp(3688342772.8190737 s since 1904-01-01), timestamp(3688342773.819743 s since 1904-01-01), timestamp(3688342774.820112 s since 1904-01-01), timestamp(3688342775.820584 s since 1904-01-01), timestamp(3688342776.8214664 s since 1904-01-01), timestamp(3688342777.821848 s since 1904-01-01), timestamp(3688342778.822177 s since 1904-01-01), timestamp(3688342779.8225975 s since 1904-01-01), timestamp(3688342780.8223686 s since 1904-01-01), timestamp(3688342781.8226385 s since 1904-01-01), timestamp(3688342782.8219137 s since 1904-01-01), timestamp(3688342783.8218846 s since 1904-01-01), timestamp(3688342784.821887 s since 1904-01-01), timestamp(3688342785.821828 s since 1904-01-01), timestamp(3688342786.8223386 s since 1904-01-01), timestamp(3688342787.825325 s since 1904-01-01), timestamp(3688342788.8251424 s since 1904-01-01), timestamp(3688342789.825672 s since 1904-01-01), timestamp(3688342790.824856 s since 1904-01-01), timestamp(3688342791.8251505 s since 1904-01-01), timestamp(3688342792.8256593 s since 1904-01-01), timestamp(3688342793.8266897 s since 1904-01-01), timestamp(3688342794.826625 s since 1904-01-01), timestamp(3688342795.825836 s since 1904-01-01), timestamp(3688342796.826832 s since 1904-01-01), timestamp(3688342798.0429673 s since 1904-01-01), timestamp(3688342799.0433993 s since 1904-01-01), timestamp(3688342800.043396 s since 1904-01-01), timestamp(3688342801.0437655 s since 1904-01-01), timestamp(3688342802.0438714 s since 1904-01-01), timestamp(3688342803.043973 s since 1904-01-01), timestamp(3688342804.043901 s since 1904-01-01), timestamp(3688342805.044822 s since 1904-01-01), timestamp(3688342806.0448112 s since 1904-01-01), timestamp(3688342807.045269 s since 1904-01-01), timestamp(3688342808.0455375 s since 1904-01-01), timestamp(3688342809.0448914 s since 1904-01-01)], "DataArray"=[101220.44208291276, 101199.06455156975, 101513.14998300378, 101241.81962803326, 101463.81719402097, 101481.90587993711, 101340.4852112232, 101508.21670489587, 101490.12801634865, 101248.39733731847, 101335.55193726094, 101240.17520126232, 101286.21914874509, 101169.46487132157, 101356.92948141521, 101490.12802344664, 101320.75209365552, 101351.99619589996, 101036.26634084422, 101345.41848871365, 101351.9961964771, 101264.84160035982, 101332.26307903595, 101389.81800331481, 101445.72850297844, 101478.61702956482, 101273.0637300145, 101495.06129681651, 101328.97422691758, 101363.50717862732, 101166.17602163501, 101279.64143487849, 101210.57553413912, 101274.70816508321, 101365.15161434854, 101356.92947504071, 101422.70654141511, 101406.26226875046, 101207.2866806673, 101467.10604803392, 101179.33142810284, 101250.04176417911, 101281.28585936227, 101361.86275192664, 101404.6178377322, 101240.17521622375, 101356.92948144057, 101355.28505120106]}, {"TimeArray"=[timestamp(3688342761.39444 s since 1904-01-01), timestamp(3688342762.463024 s since 1904-01-01), timestamp(3688342763.463638 s since 1904-01-01), timestamp(3688342764.463637 s since 1904-01-01), timestamp(3688342765.464684 s since 1904-01-01), timestamp(3688342766.465038 s since 1904-01-01), timestamp(3688342767.4661665 s since 1904-01-01), timestamp(3688342768.4671426 s since 1904-01-01), timestamp(3688342769.818876 s since 1904-01-01), timestamp(3688342770.819616 s since 1904-01-01), timestamp(3688342771.819715 s since 1904-01-01), timestamp(3688342772.8190737 s since 1904-01-01), timestamp(3688342773.819743 s since 1904-01-01), timestamp(3688342774.820112 s since 1904-01-01), timestamp(3688342775.820584 s since 1904-01-01), timestamp(3688342776.8214664 s since 1904-01-01), timestamp(3688342777.821848 s since 1904-01-01), timestamp(3688342778.822177 s since 1904-01-01), timestamp(3688342779.8225975 s since 1904-01-01), timestamp(3688342780.8223686 s since 1904-01-01), timestamp(3688342781.8226385 s since 1904-01-01), timestamp(3688342782.8219137 s since 1904-01-01), timestamp(3688342783.8218846 s since 1904-01-01), timestamp(3688342784.821887 s since 1904-01-01), timestamp(3688342785.821828 s since 1904-01-01), timestamp(3688342786.8223386 s since 1904-01-01), timestamp(3688342787.825325 s since 1904-01-01), timestamp(3688342788.8251424 s since 1904-01-01), timestamp(3688342789.825672 s since 1904-01-01), timestamp(3688342790.824856 s since 1904-01-01), timestamp(3688342791.8251505 s since 1904-01-01), timestamp(3688342792.8256593 s since 1904-01-01), timestamp(3688342793.8266897 s since 1904-01-01), timestamp(3688342794.826625 s since 1904-01-01), timestamp(3688342795.825836 s since 1904-01-01), timestamp(3688342796.826832 s since 1904-01-01), timestamp(3688342798.0429673 s since 1904-01-01), timestamp(3688342799.0433993 s since 1904-01-01), timestamp(3688342800.043396 s since 1904-01-01), timestamp(3688342801.0437655 s since 1904-01-01), timestamp(3688342802.0438714 s since 1904-01-01), timestamp(3688342803.043973 s since 1904-01-01), timestamp(3688342804.043901 s since 1904-01-01), timestamp(3688342805.044822 s since 1904-01-01), timestamp(3688342806.0448112 s since 1904-01-01), timestamp(3688342807.045269 s since 1904-01-01), timestamp(3688342808.0455375 s since 1904-01-01), timestamp(3688342809.0448914 s since 1904-01-01)], "DataArray"=[101291.15241755564, 101499.99457770793, 101284.57471698422, 101526.30539526748, 101231.95306928418, 101401.32898870594, 101355.28504938849, 101585.50475168884, 101388.17357644875, 101391.46242696735, 101504.92785874543, 101241.81963982515, 101294.44127166664, 101383.24029797112, 101342.1296400169, 101347.06292102697, 101164.53158856047, 101488.48359058959, 101437.5063683032, 101294.44127569096, 101261.55274654811, 101279.64143503254, 101430.92866322373, 101332.26308075344, 101411.19554633378, 101524.66097025927, 101291.1524215649, 101412.83997287438, 101286.21914323398, 101555.90507255693, 101358.57390073559, 101368.44045797281, 101192.48683711959, 101281.28586588813, 101457.23948682897, 101399.68455922755, 101325.68537368043, 101376.66259333238, 101246.75290715377, 101345.41848776913, 101210.57552840498, 101284.57471573919, 101601.94901872858, 101427.63981002072, 101253.33061046888, 101187.55356507898, 101386.52915740103, 101348.70734634637]}, {"TimeArray"=[timestamp(3688342761.39444 s since 1904-01-01), timestamp(3688342762.463024 s since 1904-01-01), timestamp(3688342763.463638 s since 1904-01-01), timestamp(3688342764.463637 s since 1904-01-01), timestamp(3688342765.464684 s since 1904-01-01), timestamp(3688342766.465038 s since 1904-01-01), timestamp(3688342767.4661665 s since 1904-01-01), timestamp(3688342768.4671426 s since 1904-01-01), timestamp(3688342769.818876 s since 1904-01-01), timestamp(3688342770.819616 s since 1904-01-01), timestamp(3688342771.819715 s since 1904-01-01), timestamp(3688342772.8190737 s since 1904-01-01), timestamp(3688342773.819743 s since 1904-01-01), timestamp(3688342774.820112 s since 1904-01-01), timestamp(3688342775.820584 s since 1904-01-01), timestamp(3688342776.8214664 s since 1904-01-01), timestamp(3688342777.821848 s since 1904-01-01), timestamp(3688342778.822177 s since 1904-01-01), timestamp(3688342779.8225975 s since 1904-01-01), timestamp(3688342780.8223686 s since 1904-01-01), timestamp(3688342781.8226385 s since 1904-01-01), timestamp(3688342782.8219137 s since 1904-01-01), timestamp(3688342783.8218846 s since 1904-01-01), timestamp(3688342784.821887 s since 1904-01-01), timestamp(3688342785.821828 s since 1904-01-01), timestamp(3688342786.8223386 s since 1904-01-01), timestamp(3688342787.825325 s since 1904-01-01), timestamp(3688342788.8251424 s since 1904-01-01), timestamp(3688342789.825672 s since 1904-01-01), timestamp(3688342790.824856 s since 1904-01-01), timestamp(3688342791.8251505 s since 1904-01-01), timestamp(3688342792.8256593 s since 1904-01-01), timestamp(3688342793.8266897 s since 1904-01-01), timestamp(3688342794.826625 s since 1904-01-01), timestamp(3688342795.825836 s since 1904-01-01), timestamp(3688342796.826832 s since 1904-01-01), timestamp(3688342798.0429673 s since 1904-01-01), timestamp(3688342799.0433993 s since 1904-01-01), timestamp(3688342800.043396 s since 1904-01-01), timestamp(3688342801.0437655 s since 1904-01-01), timestamp(3688342802.0438714 s since 1904-01-01), timestamp(3688342803.043973 s since 1904-01-01), timestamp(3688342804.043901 s since 1904-01-01), timestamp(3688342805.044822 s since 1904-01-01), timestamp(3688342806.0448112 s since 1904-01-01), timestamp(3688342807.045269 s since 1904-01-01), timestamp(3688342808.0455375 s since 1904-01-01), timestamp(3688342809.0448914 s since 1904-01-01)], "DataArray"=[101690.29108855205, 101706.07288687328, 101675.38605520307, 101749.03445268972, 101701.68905404501, 101739.39002005248, 101753.41828612429, 101697.30522150912, 101732.37588687218, 101737.63648599591, 101693.79815439775, 101743.77385267452, 101720.97791972595, 101739.3900203105, 101716.59408645888, 101754.29505288789, 101722.73145375543, 101703.44258741802, 101696.42845503839, 101717.47085415754, 101697.30522122844, 101685.90725504457, 101710.45672222658, 101704.31935497867, 101701.68905363319, 101707.82642008652, 101717.47085340918, 101688.5375550485, 101753.4182860876, 101699.05875491144, 101680.64665537974, 101713.08702017475, 101727.11528707815, 101705.19612072366, 101756.92535255839, 101705.19612113175, 101735.88295381088, 101695.55168733191, 101716.59408829284, 101769.20008581369, 101698.1819880936, 101747.28092016382, 101728.8688195061, 101726.2385198258, 101671.87898830316, 101719.22438681862, 101725.36175301031, 101748.15768651912]}, {"TimeArray"=[timestamp(3688342761.39444 s since 1904-01-01), timestamp(3688342762.463024 s since 1904-01-01), timestamp(3688342763.463638 s since 1904-01-01), timestamp(3688342764.463637 s since 1904-01-01), timestamp(3688342765.464684 s since 1904-01-01), timestamp(3688342766.465038 s since 1904-01-01), timestamp(3688342767.4661665 s since 1904-01-01), timestamp(3688342768.4671426 s since 1904-01-01), timestamp(3688342769.818876 s since 1904-01-01), timestamp(3688342770.819616 s since 1904-01-01), timestamp(3688342771.819715 s since 1904-01-01), timestamp(3688342772.8190737 s since 1904-01-01), timestamp(3688342773.819743 s since 1904-01-01), timestamp(3688342774.820112 s since 1904-01-01), timestamp(3688342775.820584 s since 1904-01-01), timestamp(3688342776.8214664 s since 1904-01-01), timestamp(3688342777.821848 s since 1904-01-01), timestamp(3688342778.822177 s since 1904-01-01), timestamp(3688342779.8225975 s since 1904-01-01), timestamp(3688342780.8223686 s since 1904-01-01), timestamp(3688342781.8226385 s since 1904-01-01), timestamp(3688342782.8219137 s since 1904-01-01), timestamp(3688342783.8218846 s since 1904-01-01), timestamp(3688342784.821887 s since 1904-01-01), timestamp(3688342785.821828 s since 1904-01-01), timestamp(3688342786.8223386 s since 1904-01-01), timestamp(3688342787.825325 s since 1904-01-01), timestamp(3688342788.8251424 s since 1904-01-01), timestamp(3688342789.825672 s since 1904-01-01), timestamp(3688342790.824856 s since 1904-01-01), timestamp(3688342791.8251505 s since 1904-01-01), timestamp(3688342792.8256593 s since 1904-01-01), timestamp(3688342793.8266897 s since 1904-01-01), timestamp(3688342794.826625 s since 1904-01-01), timestamp(3688342795.825836 s since 1904-01-01), timestamp(3688342796.826832 s since 1904-01-01), timestamp(3688342798.0429673 s since 1904-01-01), timestamp(3688342799.0433993 s since 1904-01-01), timestamp(3688342800.043396 s since 1904-01-01), timestamp(3688342801.0437655 s since 1904-01-01), timestamp(3688342802.0438714 s since 1904-01-01), timestamp(3688342803.043973 s since 1904-01-01), timestamp(3688342804.043901 s since 1904-01-01), timestamp(3688342805.044822 s since 1904-01-01), timestamp(3688342806.0448112 s since 1904-01-01), timestamp(3688342807.045269 s since 1904-01-01), timestamp(3688342808.0455375 s since 1904-01-01), timestamp(3688342809.0448914 s since 1904-01-01)], "DataArray"=[101713.08702033253, 101745.52738662114, 101709.57995401025, 101737.63648680823, 101773.58391905762, 101769.20008681675, 101756.04858572363, 101706.94965350973, 101773.58391935991, 101720.97792017243, 101706.94965427966, 101733.25265412086, 101763.06271961458, 101814.79195255824, 101707.82642020396, 101784.10511980281, 101777.0909881104, 101734.12942049542, 101721.85468829313, 101765.6930191484, 101707.82642028482, 101744.65061930713, 101763.06272007298, 101747.28092162542, 101754.29505260289, 101720.97792120202, 101717.47085454458, 101753.4182864131, 101756.92535364449, 101742.02032019466, 101687.66078754594, 101706.07288789151, 101737.6364877865, 101731.49912168967, 101740.26678735143, 101770.07685262537, 101733.25265347392, 101722.73145330299, 101719.22438845664, 101777.96775212817, 101749.03445332125, 101742.89708621129, 101774.46068564971, 101760.43242115337, 101678.89312250512, 101748.15768582988, 101777.9677527887, 101758.67888665742]}, {"TimeArray"=[timestamp(3688342761.39444 s since 1904-01-01), timestamp(3688342762.463024 s since 1904-01-01), timestamp(3688342763.463638 s since 1904-01-01), timestamp(3688342764.463637 s since 1904-01-01), timestamp(3688342765.464684 s since 1904-01-01), timestamp(3688342766.465038 s since 1904-01-01), timestamp(3688342767.4661665 s since 1904-01-01), timestamp(3688342768.4671426 s since 1904-01-01), timestamp(3688342769.818876 s since 1904-01-01), timestamp(3688342770.819616 s since 1904-01-01), timestamp(3688342771.819715 s since 1904-01-01), timestamp(3688342772.8190737 s since 1904-01-01), timestamp(3688342773.819743 s since 1904-01-01), timestamp(3688342774.820112 s since 1904-01-01), timestamp(3688342775.820584 s since 1904-01-01), timestamp(3688342776.8214664 s since 1904-01-01), timestamp(3688342777.821848 s since 1904-01-01), timestamp(3688342778.822177 s since 1904-01-01), timestamp(3688342779.8225975 s since 1904-01-01), timestamp(3688342780.8223686 s since 1904-01-01), timestamp(3688342781.8226385 s since 1904-01-01), timestamp(3688342782.8219137 s since 1904-01-01), timestamp(3688342783.8218846 s since 1904-01-01), timestamp(3688342784.821887 s since 1904-01-01), timestamp(3688342785.821828 s since 1904-01-01), timestamp(3688342786.8223386 s since 1904-01-01), timestamp(3688342787.825325 s since 1904-01-01), timestamp(3688342788.8251424 s since 1904-01-01), timestamp(3688342789.825672 s since 1904-01-01), timestamp(3688342790.824856 s since 1904-01-01), timestamp(3688342791.8251505 s since 1904-01-01), timestamp(3688342792.8256593 s since 1904-01-01), timestamp(3688342793.8266897 s since 1904-01-01), timestamp(3688342794.826625 s since 1904-01-01), timestamp(3688342795.825836 s since 1904-01-01), timestamp(3688342796.826832 s since 1904-01-01), timestamp(3688342798.0429673 s since 1904-01-01), timestamp(3688342799.0433993 s since 1904-01-01), timestamp(3688342800.043396 s since 1904-01-01), timestamp(3688342801.0437655 s since 1904-01-01), timestamp(3688342802.0438714 s since 1904-01-01), timestamp(3688342803.043973 s since 1904-01-01), timestamp(3688342804.043901 s since 1904-01-01), timestamp(3688342805.044822 s since 1904-01-01), timestamp(3688342806.0448112 s since 1904-01-01), timestamp(3688342807.045269 s since 1904-01-01), timestamp(3688342808.0455375 s since 1904-01-01), timestamp(3688342809.0448914 s since 1904-01-01)], "DataArray"=[0.0, 0.0, 0.0, 0.0, 0.0, 0.0, 0.0, 0.0, 0.0, 0.0, 0.0, 0.0, 0.0, 0.0, 0.0, 0.0, 0.0, 0.0, 0.0, 0.0, 0.0, 0.0, 0.0, 0.0, 0.0, 0.0, 0.0, 0.0, 0.0, 0.0, 0.0, 0.0, 0.0, 0.0, 0.0, 0.0, 0.0, 0.0, 0.0, 0.0, 0.0, 0.0, 0.0, 0.0, 0.0, 0.0, 0.0, 0.0]}, {"TimeArray"=[timestamp(3688342761.39444 s since 1904-01-01), timestamp(3688342762.463024 s since 1904-01-01), timestamp(3688342763.463638 s since 1904-01-01), timestamp(3688342764.463637 s since 1904-01-01), timestamp(3688342765.464684 s since 1904-01-01), timestamp(3688342766.465038 s since 1904-01-01), timestamp(3688342767.4661665 s since 1904-01-01), timestamp(3688342768.4671426 s since 1904-01-01), timestamp(3688342769.818876 s since 1904-01-01), timestamp(3688342770.819616 s since 1904-01-01), timestamp(3688342771.819715 s since 1904-01-01), timestamp(3688342772.8190737 s since 1904-01-01), timestamp(3688342773.819743 s since 1904-01-01), timestamp(3688342774.820112 s since 1904-01-01), timestamp(3688342775.820584 s since 1904-01-01), timestamp(3688342776.8214664 s since 1904-01-01), timestamp(3688342777.821848 s since 1904-01-01), timestamp(3688342778.822177 s since 1904-01-01), timestamp(3688342779.8225975 s since 1904-01-01), timestamp(3688342780.8223686 s since 1904-01-01), timestamp(3688342781.8226385 s since 1904-01-01), timestamp(3688342782.8219137 s since 1904-01-01), timestamp(3688342783.8218846 s since 1904-01-01), timestamp(3688342784.821887 s since 1904-01-01), timestamp(3688342785.821828 s since 1904-01-01), timestamp(3688342786.8223386 s since 1904-01-01), timestamp(3688342787.825325 s since 1904-01-01), timestamp(3688342788.8251424 s since 1904-01-01), timestamp(3688342789.825672 s since 1904-01-01), timestamp(3688342790.824856 s since 1904-01-01), timestamp(3688342791.8251505 s since 1904-01-01), timestamp(3688342792.8256593 s since 1904-01-01), timestamp(3688342793.8266897 s since 1904-01-01), timestamp(3688342794.826625 s since 1904-01-01), timestamp(3688342795.825836 s since 1904-01-01), timestamp(3688342796.826832 s since 1904-01-01), timestamp(3688342798.0429673 s since 1904-01-01), timestamp(3688342799.0433993 s since 1904-01-01), timestamp(3688342800.043396 s since 1904-01-01), timestamp(3688342801.0437655 s since 1904-01-01), timestamp(3688342802.0438714 s since 1904-01-01), timestamp(3688342803.043973 s since 1904-01-01), timestamp(3688342804.043901 s since 1904-01-01), timestamp(3688342805.044822 s since 1904-01-01), timestamp(3688342806.0448112 s since 1904-01-01), timestamp(3688342807.045269 s since 1904-01-01), timestamp(3688342808.0455375 s since 1904-01-01), timestamp(3688342809.0448914 s since 1904-01-01)], "DataArray"=[101445.72850084068, 101493.4168698453, 101467.10605043583, 101475.32818254823, 101401.3289997052, 101401.32899644942, 101603.59344600132, 101195.77569372964, 101572.34933848385, 101430.92866380943, 101485.19473516897, 101715.41444699641, 101230.30864340856, 101506.57229160522, 101273.06373993873, 101325.68539825853, 101550.97180146168, 101394.75128129986, 101547.68293945766, 101677.59263162475, 101598.66016783372, 101601.94901782386, 101667.72607876257, 101427.63982190206, 101404.61784928897, 101435.86194323712, 101472.03932931261, 101513.14999647114, 101463.81719326794, 101435.86195303871, 101480.2614619057, 101399.68456194161, 101605.2378738045, 101467.10605565517, 101394.75128367601, 101350.35177321837, 101593.72689368669, 101728.56986132935, 101552.616232476, 101532.88310808288, 101541.10523583164, 101274.70815979305, 101180.97587496797, 101504.9278637119, 101710.48117470111, 101698.97019386955, 101266.48603690336, 101325.68537503395]}, {"TimeArray"=[timestamp(3688342761.39444 s since 1904-01-01), timestamp(3688342762.463024 s since 1904-01-01), timestamp(3688342763.463638 s since 1904-01-01), timestamp(3688342764.463637 s since 1904-01-01), timestamp(3688342765.464684 s since 1904-01-01), timestamp(3688342766.465038 s since 1904-01-01), timestamp(3688342767.4661665 s since 1904-01-01), timestamp(3688342768.4671426 s since 1904-01-01), timestamp(3688342769.818876 s since 1904-01-01), timestamp(3688342770.819616 s since 1904-01-01), timestamp(3688342771.819715 s since 1904-01-01), timestamp(3688342772.8190737 s since 1904-01-01), timestamp(3688342773.819743 s since 1904-01-01), timestamp(3688342774.820112 s since 1904-01-01), timestamp(3688342775.820584 s since 1904-01-01), timestamp(3688342776.8214664 s since 1904-01-01), timestamp(3688342777.821848 s since 1904-01-01), timestamp(3688342778.822177 s since 1904-01-01), timestamp(3688342779.8225975 s since 1904-01-01), timestamp(3688342780.8223686 s since 1904-01-01), timestamp(3688342781.8226385 s since 1904-01-01), timestamp(3688342782.8219137 s since 1904-01-01), timestamp(3688342783.8218846 s since 1904-01-01), timestamp(3688342784.821887 s since 1904-01-01), timestamp(3688342785.821828 s since 1904-01-01), timestamp(3688342786.8223386 s since 1904-01-01), timestamp(3688342787.825325 s since 1904-01-01), timestamp(3688342788.8251424 s since 1904-01-01), timestamp(3688342789.825672 s since 1904-01-01), timestamp(3688342790.824856 s since 1904-01-01), timestamp(3688342791.8251505 s since 1904-01-01), timestamp(3688342792.8256593 s since 1904-01-01), timestamp(3688342793.8266897 s since 1904-01-01), timestamp(3688342794.826625 s since 1904-01-01), timestamp(3688342795.825836 s since 1904-01-01), timestamp(3688342796.826832 s since 1904-01-01), timestamp(3688342798.0429673 s since 1904-01-01), timestamp(3688342799.0433993 s since 1904-01-01), timestamp(3688342800.043396 s since 1904-01-01), timestamp(3688342801.0437655 s since 1904-01-01), timestamp(3688342802.0438714 s since 1904-01-01), timestamp(3688342803.043973 s since 1904-01-01), timestamp(3688342804.043901 s since 1904-01-01), timestamp(3688342805.044822 s since 1904-01-01), timestamp(3688342806.0448112 s since 1904-01-01), timestamp(3688342807.045269 s since 1904-01-01), timestamp(3688342808.0455375 s since 1904-01-01), timestamp(3688342809.0448914 s since 1904-01-01)], "DataArray"=[0.00015794392082601466, 0.00014527857457659758, 0.0001612303236722782, 0.00013225994060034175, 0.00014558688545089616, 0.00014624975809092566, 0.00014745054197010484, 0.00016270186273131826, 0.00015083803725969138, 0.000153000418941653, 0.00016142575747488726, 0.00014361624215080963, 0.00014825653834920106, 0.0001447954042376404, 0.00015885537746714444, 0.0001444887692259696, 0.0001483912978320738, 0.00015406987566298966, 0.00015318587672950214, 0.00015047302647334682, 0.00015102087320363603, 0.00015263017661396096, 0.00015239923156078213, 0.00014970031234038994, 0.00015514680781186815, 0.00015775270241722642, 0.00015718043610256062, 0.0001610839043479135, 0.00013992401920005955, 0.0001550998287190593, 0.00016816241133741627, 0.00015369704584851536, 0.00015661024640693013, 0.0001551468076217685, 0.0001533251178390125, 0.00015074670138303243, 0.00015083803621330125, 0.0001478082195316557, 0.00015379016984874418, 0.00013707190891229566, 0.0001470046627129244, 0.00015276891279361772, 0.00014514664144137354, 0.00014669334861615104, 0.00015775270273420098, 0.00014453253399511162, 0.00014673778134435226, 0.00015001800729686586]}] caption="XY Graph"
  in  "FIle suffix 4":string="Graph4_1KPot_oscillation"
  in  "Take Screenshot! 4":bool
  in  "Take Screenshot! 3":bool
  in  "Take Screenshot! 2":bool
  in  "Take Screenshot! 1":bool
  in  "FIle suffix 3":string="Graph3_1KPot_oscillation"
  in  "FIle suffix 2":string="Graph2_1KPot_oscillation"
  in  "FIle suffix 1":string="Graph1_1KPot_oscillation"
  in  "log/linear 2":bool
  in  "Tab Control 2":T5(tab)=enum."USB6218"
  in  "Plot selecter (USB6210)\n    1      2     3     4":bool[][](array[boolean])=[[TRUE, FALSE, FALSE, FALSE], [TRUE, FALSE, FALSE, FALSE], [TRUE, FALSE, FALSE, FALSE], [TRUE, FALSE, FALSE, FALSE], [TRUE, FALSE, FALSE, FALSE], [TRUE, FALSE, FALSE, FALSE], [TRUE, FALSE, FALSE, FALSE], [FALSE, TRUE, FALSE, FALSE], [FALSE, TRUE, FALSE, FALSE], [FALSE, TRUE, FALSE, FALSE], [FALSE, TRUE, FALSE, FALSE], [FALSE, TRUE, FALSE, FALSE], [FALSE, TRUE, FALSE, FALSE], [TRUE, FALSE, FALSE, FALSE], [TRUE, FALSE, FALSE, FALSE], [FALSE, FALSE, FALSE, FALSE]]
  out "All Labels (USB6210)":string[](array[string])=["P_ins", "P_4Kres", "P_3HeIN", "P_SldRTN", "P_3Hepot", "P_1Kpot", "P_Dewar(old)", "DP_HEX4", "DP_HEX5", "L1", "L2-1", "L2-2", "L3", "P_HEX7OUT", "P_IP", "V_H1"]
  out "Last Data \n(USB6210)":dbl[](array[numeric])=[0.001713490844762899, 102021.27778594472, 101355.28505120106, 101348.70734634637, 101748.15768651912, 101758.67888665742, 0.0, -12.307228287251254, -3.5949330203699503, 100.19921295176155, 0.09220134592968446, 0.08102171791361665, 0.09614709699847113, 101325.68537503395, 0.00015001800729686586, 5.514153752001237] format="%#_6e"
  out "Time of Last Measurement (USB6210)":timestamp=timestamp(3688342809.0448914 s since 1904-01-01)
  out "USB6210 Status":T6(ring)=enum."Ready"
  out "Last Vol\n(USB6210)":dbl[](array[numeric])=[6.116940894161298, 3.0404255557188944, 3.027105701024021, 3.0269741469269276, 7.631875013990333, 7.6326641829175985, 0.0, 0.950771086850995, 0.999281013395926, 10.019921295176156, 0.009220134592968447, 0.008102171791361665, 0.009614709699847113, 3.026513707500679, 5.588071696195447, 5.514153752001237] format="%_5f"
  out "Time of Last Measurement (USB6218)":timestamp=timestamp(3688342809.0488415 s since 1904-01-01)
  out "USB6218 Status":T6(ring)=enum."Ready"
  out "Last Vol \n(USB6218)":dbl[](array[numeric])=[0.012360578900337791, 0.008152081311926958, 0.006902683576152324, -0.08229774188754428, 0.2519818880738261, 0.004212046304753189, -0.00016627727782198148, 3.0439553665890373] format="%_5f"
  out "Last Data \n(USB6218)":dbl[](array[numeric])=[1.236057890033779, 0.32608325247707837, 0.27610734304609297, -8.229774188754428, 25.19818880738261, 0.004212046304753189, -25.00415693194555, 102197.76832945186] format="%#_6e"
  out "All Labels (USB6218)":string[](array[string])=["F_1", "F_2", "F_3", "F_4", "F_5", "I_CV", "CV1_answer", "P_Dewar"]
  in  "Plot selecter (USB6218)\n    1      2     3     4":bool[][](array[boolean])=[[FALSE, FALSE, TRUE, FALSE], [FALSE, FALSE, TRUE, FALSE], [FALSE, FALSE, TRUE, FALSE], [FALSE, FALSE, TRUE, FALSE], [FALSE, FALSE, TRUE, FALSE], [FALSE, FALSE, TRUE, FALSE], [FALSE, FALSE, FALSE, FALSE], [FALSE, FALSE, TRUE, FALSE], [FALSE, FALSE, TRUE, FALSE], [FALSE, FALSE, FALSE, TRUE], [FALSE, FALSE, FALSE, TRUE], [FALSE, FALSE, FALSE, TRUE], [FALSE, FALSE, FALSE, TRUE], [FALSE, FALSE, FALSE, FALSE], [FALSE, FALSE, FALSE, FALSE], [FALSE, FALSE, FALSE, FALSE]]
  out "Time of Last Measurement (LSI218)":timestamp=timestamp(3688342809.0448914 s since 1904-01-01)
  out "LSI218 Status":T7(ring)=enum."Measuring"
  out "Last Data \nLSI218 (1)":dbl[](array[numeric])=[278.76, 287.23, 205.57, 197.31, 93.015, 90.402, 59.35, 73.73, 30.0, 0.0, 0.0, 0.0, 149.39, 148.1, 73.063, 286.33, 289.87, 290.01, 289.1, 289.16, 148.02, 152.67, 122.79, 109.94]
  out "Labels LSI218 (1)":string[](array[string])=["T3He10", "T3He1-1", "TTH3", "TTH4", "TTH1", "TTH2", "T4He1", "T1K1", "N.C.", "N.C.", "N.C.", "N.C.", "T3He2-1", "T3He2-2", "T3He3", "T3He1-4", "T4He3-1", "T4He3-2", "T4He3-3", "T4He3-4", "T4He2-1", "T4He2-2", "T4He4", "T4He5"]
  in  "Plot selecter LSI218(1)\n    1      2     3     4":bool[][](array[boolean])=[[FALSE, FALSE, FALSE, FALSE], [FALSE, FALSE, FALSE, FALSE], [FALSE, FALSE, FALSE, TRUE], [FALSE, FALSE, FALSE, TRUE], [FALSE, FALSE, FALSE, TRUE], [FALSE, FALSE, FALSE, TRUE], [FALSE, FALSE, FALSE, TRUE], [FALSE, FALSE, FALSE, TRUE], [FALSE, FALSE, FALSE, FALSE], [FALSE, FALSE, FALSE, FALSE], [FALSE, FALSE, FALSE, FALSE], [FALSE, FALSE, FALSE, FALSE], [FALSE, FALSE, FALSE, TRUE], [FALSE, FALSE, FALSE, TRUE], [FALSE, FALSE, FALSE, FALSE], [FALSE, FALSE, FALSE, FALSE], [FALSE, FALSE, FALSE, TRUE], [FALSE, FALSE, FALSE, TRUE], [FALSE, FALSE, FALSE, TRUE], [FALSE, FALSE, FALSE, TRUE], [FALSE, FALSE, FALSE, TRUE], [FALSE, FALSE, FALSE, TRUE], [FALSE, FALSE, FALSE, TRUE], [FALSE, FALSE, FALSE, FALSE]]
  out "Active?\n (1)":bool[](array[boolean])=[TRUE, TRUE, TRUE, TRUE, TRUE, TRUE, TRUE, TRUE, TRUE, TRUE, TRUE, TRUE, TRUE, TRUE, TRUE, TRUE, TRUE, TRUE, TRUE, TRUE, TRUE, TRUE, TRUE, TRUE]
  out "Labels LSI218 (2)":string[](array[string])=["T4He6", "T4He9", "T3He1-2", "T3He1-3", "T4He7", "T4He8", "T4He10", "T1K6", "TIP1", "N.C.", "TIP2", "N.C.", "TIP3", "TIP4", "TIP5", "N.C.", "T1K2", "T1K4", "T1K5", "T3He4", "T3He9", "TIP6", "N.C.", "N.C."]
  out "Active?\n(2)":bool[](array[boolean])=[TRUE, TRUE, TRUE, TRUE, TRUE, TRUE, TRUE, TRUE, TRUE, TRUE, TRUE, TRUE, TRUE, TRUE, TRUE, TRUE, TRUE, TRUE, TRUE, TRUE, TRUE, TRUE, TRUE, TRUE]
  out "Last Data \nLSI218 (2)":dbl[](array[numeric])=[115.85, 186.16, 287.33, 286.78, 211.21, 254.77, 250.0, 277.86, 265.54, 0.0, 182.55, 688.49, 128.86, 64.91, 64.659, 688.58, 59.451, 48.966, 66.774, 56.763, 67.829, 63.827, 0.433, 0.0]
  in  "Plot selecter LSI218(2)\n    1      2     3     4":bool[][](array[boolean])=[[FALSE, FALSE, FALSE, FALSE], [FALSE, FALSE, FALSE, FALSE], [FALSE, FALSE, FALSE, FALSE], [FALSE, FALSE, FALSE, FALSE], [FALSE, FALSE, FALSE, FALSE], [FALSE, FALSE, FALSE, FALSE], [FALSE, FALSE, FALSE, FALSE], [FALSE, FALSE, FALSE, FALSE], [FALSE, FALSE, FALSE, FALSE], [FALSE, FALSE, FALSE, FALSE], [FALSE, FALSE, FALSE, FALSE], [FALSE, FALSE, FALSE, FALSE], [FALSE, FALSE, FALSE, FALSE], [FALSE, FALSE, FALSE, FALSE], [FALSE, FALSE, FALSE, FALSE], [FALSE, FALSE, FALSE, FALSE], [FALSE, FALSE, FALSE, TRUE], [FALSE, FALSE, FALSE, TRUE], [FALSE, FALSE, FALSE, TRUE], [FALSE, FALSE, FALSE, FALSE], [FALSE, FALSE, FALSE, FALSE], [FALSE, FALSE, FALSE, FALSE], [FALSE, FALSE, FALSE, FALSE], [FALSE, FALSE, FALSE, FALSE]]
  in  "Plot selecter LSI336 \n     1      2     3     4":bool[][](array[boolean])=[[FALSE, FALSE, FALSE, TRUE], [FALSE, FALSE, FALSE, TRUE], [FALSE, FALSE, FALSE, TRUE], [FALSE, FALSE, FALSE, TRUE], [FALSE, FALSE, FALSE, TRUE], [FALSE, FALSE, FALSE, TRUE], [FALSE, FALSE, FALSE, TRUE], [FALSE, FALSE, FALSE, TRUE]]
  out "Time of Last Measurement (LSI336)":timestamp=timestamp(3688342809.0448914 s since 1904-01-01)
  out "Last Data \nLSI336":dbl[](array[numeric])=[44.0737, 44.0488, 63.4557, 53.3294, 56.5704, 56.5561, 56.5737, 56.1152]
  out "Active?\n(LSI336)":bool[](array[boolean])=[TRUE, TRUE, TRUE, TRUE, TRUE, TRUE, TRUE, TRUE]
  out "Labels LSI336":string[](array[string])=["T1K3-1", "T1K3-2", "T3He5", "T3He8", "T3He6-1", "T3He6-2", "T3He7-1", "T3He7-2"]
  out "LSI336 Status":T7(ring)=enum."Measuring"
  in  "log/linear 1":bool
  out "Graph 2":T4(graph)=[{"TimeArray"=[timestamp(3688342761.39444 s since 1904-01-01), timestamp(3688342762.463024 s since 1904-01-01), timestamp(3688342763.463638 s since 1904-01-01), timestamp(3688342764.463637 s since 1904-01-01), timestamp(3688342765.464684 s since 1904-01-01), timestamp(3688342766.465038 s since 1904-01-01), timestamp(3688342767.4661665 s since 1904-01-01), timestamp(3688342768.4671426 s since 1904-01-01), timestamp(3688342769.818876 s since 1904-01-01), timestamp(3688342770.819616 s since 1904-01-01), timestamp(3688342771.819715 s since 1904-01-01), timestamp(3688342772.8190737 s since 1904-01-01), timestamp(3688342773.819743 s since 1904-01-01), timestamp(3688342774.820112 s since 1904-01-01), timestamp(3688342775.820584 s since 1904-01-01), timestamp(3688342776.8214664 s since 1904-01-01), timestamp(3688342777.821848 s since 1904-01-01), timestamp(3688342778.822177 s since 1904-01-01), timestamp(3688342779.8225975 s since 1904-01-01), timestamp(3688342780.8223686 s since 1904-01-01), timestamp(3688342781.8226385 s since 1904-01-01), timestamp(3688342782.8219137 s since 1904-01-01), timestamp(3688342783.8218846 s since 1904-01-01), timestamp(3688342784.821887 s since 1904-01-01), timestamp(3688342785.821828 s since 1904-01-01), timestamp(3688342786.8223386 s since 1904-01-01), timestamp(3688342787.825325 s since 1904-01-01), timestamp(3688342788.8251424 s since 1904-01-01), timestamp(3688342789.825672 s since 1904-01-01), timestamp(3688342790.824856 s since 1904-01-01), timestamp(3688342791.8251505 s since 1904-01-01), timestamp(3688342792.8256593 s since 1904-01-01), timestamp(3688342793.8266897 s since 1904-01-01), timestamp(3688342794.826625 s since 1904-01-01), timestamp(3688342795.825836 s since 1904-01-01), timestamp(3688342796.826832 s since 1904-01-01), timestamp(3688342798.0429673 s since 1904-01-01), timestamp(3688342799.0433993 s since 1904-01-01), timestamp(3688342800.043396 s since 1904-01-01), timestamp(3688342801.0437655 s since 1904-01-01), timestamp(3688342802.0438714 s since 1904-01-01), timestamp(3688342803.043973 s since 1904-01-01), timestamp(3688342804.043901 s since 1904-01-01), timestamp(3688342805.044822 s since 1904-01-01), timestamp(3688342806.0448112 s since 1904-01-01), timestamp(3688342807.045269 s since 1904-01-01), timestamp(3688342808.0455375 s since 1904-01-01), timestamp(3688342809.0448914 s since 1904-01-01)], "DataArray"=[-14.58472805516084, -11.665910666875446, -11.05748111470345, -12.035901604533272, -11.115035260684719, -9.93106421754808, -11.411027997547091, -12.6689972146794, -13.022544125408208, -12.019457533253814, -10.86015261028711, -11.56724640891954, -11.337029835953722, -12.183897976992764, -10.90948473209355, -12.915657844999012, -11.961903396566553, -14.453175739544522, -12.175675957747822, -11.024593017420786, -12.134565860956126, -14.634060181933917, -11.871461182531961, -11.427472064826361, -12.825215618469166, -12.077011703639117, -11.896127252572164, -10.728600276382366, -11.72346482206929, -14.27229128211488, -13.663861749815403, -12.553888925297462, -11.961903410629526, -10.720378254392315, -13.12120837957803, -11.961903433253346, -12.01945757468495, -13.236316654715807, -11.698798761406643, -10.547715817769282, -13.762525973974732, -13.524087373262356, -11.35347387159888, -11.378139941417592, -11.27125364694509, -10.21061294287512, -13.071876252658488, -12.307228287251254]}, {"TimeArray"=[timestamp(3688342761.39444 s since 1904-01-01), timestamp(3688342762.463024 s since 1904-01-01), timestamp(3688342763.463638 s since 1904-01-01), timestamp(3688342764.463637 s since 1904-01-01), timestamp(3688342765.464684 s since 1904-01-01), timestamp(3688342766.465038 s since 1904-01-01), timestamp(3688342767.4661665 s since 1904-01-01), timestamp(3688342768.4671426 s since 1904-01-01), timestamp(3688342769.818876 s since 1904-01-01), timestamp(3688342770.819616 s since 1904-01-01), timestamp(3688342771.819715 s since 1904-01-01), timestamp(3688342772.8190737 s since 1904-01-01), timestamp(3688342773.819743 s since 1904-01-01), timestamp(3688342774.820112 s since 1904-01-01), timestamp(3688342775.820584 s since 1904-01-01), timestamp(3688342776.8214664 s since 1904-01-01), timestamp(3688342777.821848 s since 1904-01-01), timestamp(3688342778.822177 s since 1904-01-01), timestamp(3688342779.8225975 s since 1904-01-01), timestamp(3688342780.8223686 s since 1904-01-01), timestamp(3688342781.8226385 s since 1904-01-01), timestamp(3688342782.8219137 s since 1904-01-01), timestamp(3688342783.8218846 s since 1904-01-01), timestamp(3688342784.821887 s since 1904-01-01), timestamp(3688342785.821828 s since 1904-01-01), timestamp(3688342786.8223386 s since 1904-01-01), timestamp(3688342787.825325 s since 1904-01-01), timestamp(3688342788.8251424 s since 1904-01-01), timestamp(3688342789.825672 s since 1904-01-01), timestamp(3688342790.824856 s since 1904-01-01), timestamp(3688342791.8251505 s since 1904-01-01), timestamp(3688342792.8256593 s since 1904-01-01), timestamp(3688342793.8266897 s since 1904-01-01), timestamp(3688342794.826625 s since 1904-01-01), timestamp(3688342795.825836 s since 1904-01-01), timestamp(3688342796.826832 s since 1904-01-01), timestamp(3688342798.0429673 s since 1904-01-01), timestamp(3688342799.0433993 s since 1904-01-01), timestamp(3688342800.043396 s since 1904-01-01), timestamp(3688342801.0437655 s since 1904-01-01), timestamp(3688342802.0438714 s since 1904-01-01), timestamp(3688342803.043973 s since 1904-01-01), timestamp(3688342804.043901 s since 1904-01-01), timestamp(3688342805.044822 s since 1904-01-01), timestamp(3688342806.0448112 s since 1904-01-01), timestamp(3688342807.045269 s since 1904-01-01), timestamp(3688342808.0455375 s since 1904-01-01), timestamp(3688342809.0448914 s since 1904-01-01)], "DataArray"=[-3.7593731160273647, 16.466800869346933, -17.079048716840404, -1.621647579482799, 25.346585889716167, 24.853263053700168, -2.1149691056238096, -34.18085471315613, 6.1070527372864, 71.55435072561778, 33.07528543448734, 35.377451936993154, 3.4760067505701375, 21.235573406630515, -4.252694378406585, -12.803597630295371, 95.06933587075883, -2.114969105721509, 73.52763482644909, 45.40831880739504, -40.594030132280466, 64.48341078485909, 11.862468345331667, 49.51933207329118, -15.105763950596373, 5.942612372294986, 48.20380658039136, 52.150377482029775, -8.19926519956493, -4.91045665409362, 22.386656386026438, 55.110306476439106, -21.683380136412467, 19.262288053315537, 14.00019391494145, -13.296918621765741, -36.48302079347576, -21.190060255552588, 86.6828718697632, -2.279409637019336, -21.847821824532154, 74.84315986737933, 32.910845104363595, 68.42998149528823, -15.599085085889474, 39.4884632112269, 24.853263706915428, -3.5949330203699503]}, {"TimeArray"=[timestamp(3688342761.39444 s since 1904-01-01), timestamp(3688342762.463024 s since 1904-01-01), timestamp(3688342763.463638 s since 1904-01-01), timestamp(3688342764.463637 s since 1904-01-01), timestamp(3688342765.464684 s since 1904-01-01), timestamp(3688342766.465038 s since 1904-01-01), timestamp(3688342767.4661665 s since 1904-01-01), timestamp(3688342768.4671426 s since 1904-01-01), timestamp(3688342769.818876 s since 1904-01-01), timestamp(3688342770.819616 s since 1904-01-01), timestamp(3688342771.819715 s since 1904-01-01), timestamp(3688342772.8190737 s since 1904-01-01), timestamp(3688342773.819743 s since 1904-01-01), timestamp(3688342774.820112 s since 1904-01-01), timestamp(3688342775.820584 s since 1904-01-01), timestamp(3688342776.8214664 s since 1904-01-01), timestamp(3688342777.821848 s since 1904-01-01), timestamp(3688342778.822177 s since 1904-01-01), timestamp(3688342779.8225975 s since 1904-01-01), timestamp(3688342780.8223686 s since 1904-01-01), timestamp(3688342781.8226385 s since 1904-01-01), timestamp(3688342782.8219137 s since 1904-01-01), timestamp(3688342783.8218846 s since 1904-01-01), timestamp(3688342784.821887 s since 1904-01-01), timestamp(3688342785.821828 s since 1904-01-01), timestamp(3688342786.8223386 s since 1904-01-01), timestamp(3688342787.825325 s since 1904-01-01), timestamp(3688342788.8251424 s since 1904-01-01), timestamp(3688342789.825672 s since 1904-01-01), timestamp(3688342790.824856 s since 1904-01-01), timestamp(3688342791.8251505 s since 1904-01-01), timestamp(3688342792.8256593 s since 1904-01-01), timestamp(3688342793.8266897 s since 1904-01-01), timestamp(3688342794.826625 s since 1904-01-01), timestamp(3688342795.825836 s since 1904-01-01), timestamp(3688342796.826832 s since 1904-01-01), timestamp(3688342798.0429673 s since 1904-01-01), timestamp(3688342799.0433993 s since 1904-01-01), timestamp(3688342800.043396 s since 1904-01-01), timestamp(3688342801.0437655 s since 1904-01-01), timestamp(3688342802.0438714 s since 1904-01-01), timestamp(3688342803.043973 s since 1904-01-01), timestamp(3688342804.043901 s since 1904-01-01), timestamp(3688342805.044822 s since 1904-01-01), timestamp(3688342806.0448112 s since 1904-01-01), timestamp(3688342807.045269 s since 1904-01-01), timestamp(3688342808.0455375 s since 1904-01-01), timestamp(3688342809.0448914 s since 1904-01-01)], "DataArray"=[100.02033130195804, 100.01901599603929, 100.01638538424609, 100.03743027703277, 100.01572773170821, 100.0157277313541, 100.02559252494399, 100.04203384733069, 100.01638538431729, 100.03151140103552, 100.01375477272042, 100.0367726240272, 100.03085374795297, 100.03479966541471, 100.03479966540314, 100.00980885549924, 100.02559252485926, 100.03282670696193, 100.0354573184203, 100.02690783064907, 100.04269150040554, 100.01901599615667, 100.04795272384771, 100.01901599594885, 100.01638538480807, 100.03019609549787, 100.03874558303818, 100.02953844234602, 100.00586293801635, 100.01835834285669, 100.03085374811465, 100.03808792994593, 100.01178181389622, 100.01441242558933, 100.0262501777436, 100.02164660751687, 100.03282670700432, 100.0380879299652, 100.04269150063466, 100.03348435976736, 100.0420338474096, 100.04597976485402, 100.03611497118908, 100.03348435956718, 100.11832159997704, 100.02559252476306, 100.03348435966727, 100.19921295176155]}, {"TimeArray"=[timestamp(3688342761.39444 s since 1904-01-01), timestamp(3688342762.463024 s since 1904-01-01), timestamp(3688342763.463638 s since 1904-01-01), timestamp(3688342764.463637 s since 1904-01-01), timestamp(3688342765.464684 s since 1904-01-01), timestamp(3688342766.465038 s since 1904-01-01), timestamp(3688342767.4661665 s since 1904-01-01), timestamp(3688342768.4671426 s since 1904-01-01), timestamp(3688342769.818876 s since 1904-01-01), timestamp(3688342770.819616 s since 1904-01-01), timestamp(3688342771.819715 s since 1904-01-01), timestamp(3688342772.8190737 s since 1904-01-01), timestamp(3688342773.819743 s since 1904-01-01), timestamp(3688342774.820112 s since 1904-01-01), timestamp(3688342775.820584 s since 1904-01-01), timestamp(3688342776.8214664 s since 1904-01-01), timestamp(3688342777.821848 s since 1904-01-01), timestamp(3688342778.822177 s since 1904-01-01), timestamp(3688342779.8225975 s since 1904-01-01), timestamp(3688342780.8223686 s since 1904-01-01), timestamp(3688342781.8226385 s since 1904-01-01), timestamp(3688342782.8219137 s since 1904-01-01), timestamp(3688342783.8218846 s since 1904-01-01), timestamp(3688342784.821887 s since 1904-01-01), timestamp(3688342785.821828 s since 1904-01-01), timestamp(3688342786.8223386 s since 1904-01-01), timestamp(3688342787.825325 s since 1904-01-01), timestamp(3688342788.8251424 s since 1904-01-01), timestamp(3688342789.825672 s since 1904-01-01), timestamp(3688342790.824856 s since 1904-01-01), timestamp(3688342791.8251505 s since 1904-01-01), timestamp(3688342792.8256593 s since 1904-01-01), timestamp(3688342793.8266897 s since 1904-01-01), timestamp(3688342794.826625 s since 1904-01-01), timestamp(3688342795.825836 s since 1904-01-01), timestamp(3688342796.826832 s since 1904-01-01), timestamp(3688342798.0429673 s since 1904-01-01), timestamp(3688342799.0433993 s since 1904-01-01), timestamp(3688342800.043396 s since 1904-01-01), timestamp(3688342801.0437655 s since 1904-01-01), timestamp(3688342802.0438714 s since 1904-01-01), timestamp(3688342803.043973 s since 1904-01-01), timestamp(3688342804.043901 s since 1904-01-01), timestamp(3688342805.044822 s since 1904-01-01), timestamp(3688342806.0448112 s since 1904-01-01), timestamp(3688342807.045269 s since 1904-01-01), timestamp(3688342808.0455375 s since 1904-01-01), timestamp(3688342809.0448914 s since 1904-01-01)], "DataArray"=[0.09680472216883765, 0.0856250941222492, 0.10272334875069622, 0.0823369682619271, 0.11982160335626449, 0.1231097292068519, 0.11061485087663162, 0.07378784094485494, 0.09483184662552932, 0.09614709695613116, 0.0856250941451212, 0.09154372074948794, 0.09351659626786335, 0.08825559483278658, 0.08628271927790962, 0.08233696823210371, 0.10535384948209497, 0.08036409273191733, 0.08562509416150313, 0.09943522288286516, 0.10009284806285693, 0.07970646756035346, 0.1066690997654503, 0.09746234734177431, 0.1336317319665327, 0.08628271933695833, 0.08759796967635775, 0.11258772641687786, 0.10140809840991075, 0.08628271925850953, 0.10864197531300018, 0.08562509414773817, 0.10075047323552361, 0.08233696821786596, 0.12376735434914118, 0.0961470969909575, 0.094174221460295, 0.09417422145992005, 0.0948318466200812, 0.12574022994657183, 0.09483184660307273, 0.08891322003955524, 0.07313021578192988, 0.08167934302691235, 0.1007504732268858, 0.1073267250044955, 0.07904884235852952, 0.09220134592968446]}, {"TimeArray"=[timestamp(3688342761.39444 s since 1904-01-01), timestamp(3688342762.463024 s since 1904-01-01), timestamp(3688342763.463638 s since 1904-01-01), timestamp(3688342764.463637 s since 1904-01-01), timestamp(3688342765.464684 s since 1904-01-01), timestamp(3688342766.465038 s since 1904-01-01), timestamp(3688342767.4661665 s since 1904-01-01), timestamp(3688342768.4671426 s since 1904-01-01), timestamp(3688342769.818876 s since 1904-01-01), timestamp(3688342770.819616 s since 1904-01-01), timestamp(3688342771.819715 s since 1904-01-01), timestamp(3688342772.8190737 s since 1904-01-01), timestamp(3688342773.819743 s since 1904-01-01), timestamp(3688342774.820112 s since 1904-01-01), timestamp(3688342775.820584 s since 1904-01-01), timestamp(3688342776.8214664 s since 1904-01-01), timestamp(3688342777.821848 s since 1904-01-01), timestamp(3688342778.822177 s since 1904-01-01), timestamp(3688342779.8225975 s since 1904-01-01), timestamp(3688342780.8223686 s since 1904-01-01), timestamp(3688342781.8226385 s since 1904-01-01), timestamp(3688342782.8219137 s since 1904-01-01), timestamp(3688342783.8218846 s since 1904-01-01), timestamp(3688342784.821887 s since 1904-01-01), timestamp(3688342785.821828 s since 1904-01-01), timestamp(3688342786.8223386 s since 1904-01-01), timestamp(3688342787.825325 s since 1904-01-01), timestamp(3688342788.8251424 s since 1904-01-01), timestamp(3688342789.825672 s since 1904-01-01), timestamp(3688342790.824856 s since 1904-01-01), timestamp(3688342791.8251505 s since 1904-01-01), timestamp(3688342792.8256593 s since 1904-01-01), timestamp(3688342793.8266897 s since 1904-01-01), timestamp(3688342794.826625 s since 1904-01-01), timestamp(3688342795.825836 s since 1904-01-01), timestamp(3688342796.826832 s since 1904-01-01), timestamp(3688342798.0429673 s since 1904-01-01), timestamp(3688342799.0433993 s since 1904-01-01), timestamp(3688342800.043396 s since 1904-01-01), timestamp(3688342801.0437655 s since 1904-01-01), timestamp(3688342802.0438714 s since 1904-01-01), timestamp(3688342803.043973 s since 1904-01-01), timestamp(3688342804.043901 s since 1904-01-01), timestamp(3688342805.044822 s since 1904-01-01), timestamp(3688342806.0448112 s since 1904-01-01), timestamp(3688342807.045269 s since 1904-01-01), timestamp(3688342808.0455375 s since 1904-01-01), timestamp(3688342809.0448914 s since 1904-01-01)], "DataArray"=[0.0928589711067572, 0.110614850901225, 0.11784872782819483, 0.11061485089033349, 0.10666909982112965, 0.09088609557892624, 0.09614709700198834, 0.09220134593649923, 0.10666909983274891, 0.08825559486610221, 0.11127247607640156, 0.08365221862333744, 0.08430984379709675, 0.08233696827611237, 0.10798435018011024, 0.08628271933183773, 0.10009284806124849, 0.1014080984088988, 0.1369198579456621, 0.09417422145990806, 0.09548947181950596, 0.10403859913064109, 0.10272334877207187, 0.10469622429029102, 0.10469622430661588, 0.08628271933354992, 0.10666909983584733, 0.11916397818045257, 0.08496746896842622, 0.11982160335618988, 0.10075047322387898, 0.09680472217446534, 0.10075047322328137, 0.10929960053125665, 0.08825559486315551, 0.11193010123896543, 0.09548947182109846, 0.08957084522064646, 0.10272334876996597, 0.06984208989584345, 0.08891322005171653, 0.09811997252651306, 0.10338097394513843, 0.10535384948089216, 0.12968598099932982, 0.0928589711172974, 0.09811997252509147, 0.08102171791361665]}, {"TimeArray"=[timestamp(3688342761.39444 s since 1904-01-01), timestamp(3688342762.463024 s since 1904-01-01), timestamp(3688342763.463638 s since 1904-01-01), timestamp(3688342764.463637 s since 1904-01-01), timestamp(3688342765.464684 s since 1904-01-01), timestamp(3688342766.465038 s since 1904-01-01), timestamp(3688342767.4661665 s since 1904-01-01), timestamp(3688342768.4671426 s since 1904-01-01), timestamp(3688342769.818876 s since 1904-01-01), timestamp(3688342770.819616 s since 1904-01-01), timestamp(3688342771.819715 s since 1904-01-01), timestamp(3688342772.8190737 s since 1904-01-01), timestamp(3688342773.819743 s since 1904-01-01), timestamp(3688342774.820112 s since 1904-01-01), timestamp(3688342775.820584 s since 1904-01-01), timestamp(3688342776.8214664 s since 1904-01-01), timestamp(3688342777.821848 s since 1904-01-01), timestamp(3688342778.822177 s since 1904-01-01), timestamp(3688342779.8225975 s since 1904-01-01), timestamp(3688342780.8223686 s since 1904-01-01), timestamp(3688342781.8226385 s since 1904-01-01), timestamp(3688342782.8219137 s since 1904-01-01), timestamp(3688342783.8218846 s since 1904-01-01), timestamp(3688342784.821887 s since 1904-01-01), timestamp(3688342785.821828 s since 1904-01-01), timestamp(3688342786.8223386 s since 1904-01-01), timestamp(3688342787.825325 s since 1904-01-01), timestamp(3688342788.8251424 s since 1904-01-01), timestamp(3688342789.825672 s since 1904-01-01), timestamp(3688342790.824856 s since 1904-01-01), timestamp(3688342791.8251505 s since 1904-01-01), timestamp(3688342792.8256593 s since 1904-01-01), timestamp(3688342793.8266897 s since 1904-01-01), timestamp(3688342794.826625 s since 1904-01-01), timestamp(3688342795.825836 s since 1904-01-01), timestamp(3688342796.826832 s since 1904-01-01), timestamp(3688342798.0429673 s since 1904-01-01), timestamp(3688342799.0433993 s since 1904-01-01), timestamp(3688342800.043396 s since 1904-01-01), timestamp(3688342801.0437655 s since 1904-01-01), timestamp(3688342802.0438714 s since 1904-01-01), timestamp(3688342803.043973 s since 1904-01-01), timestamp(3688342804.043901 s since 1904-01-01), timestamp(3688342805.044822 s since 1904-01-01), timestamp(3688342806.0448112 s since 1904-01-01), timestamp(3688342807.045269 s since 1904-01-01), timestamp(3688342808.0455375 s since 1904-01-01), timestamp(3688342809.0448914 s since 1904-01-01)], "DataArray"=[0.09285897110562968, 0.08694034451505128, 0.0882555948658934, 0.10140809841931961, 0.0882555948622622, 0.08957084522668168, 0.10206572358988894, 0.10338097395305981, 0.08891322004558086, 0.11456060195989323, 0.0889132200492053, 0.10469622429598657, 0.0954894718143463, 0.09548947182601278, 0.11982160335837219, 0.10075047323232106, 0.09220134593509657, 0.09877759770890365, 0.09154372074318548, 0.09943522286249523, 0.10009284806184715, 0.09483184663978972, 0.08167934308211428, 0.08628271933586429, 0.09943522287654274, 0.109957225693192, 0.10666909983775433, 0.09088609557339636, 0.08825559486026241, 0.0981199725277064, 0.09351659627431821, 0.10995722571543565, 0.10009284806435811, 0.09877759770698699, 0.0968047221647878, 0.08167934309300484, 0.09746234734269646, 0.10995722571854372, 0.09943522287635259, 0.10403859911541599, 0.10535384947677798, 0.10403859912523186, 0.11982160336152853, 0.10732672501153062, 0.10009284805986082, 0.10929960054586751, 0.11324535160603699, 0.09614709699847113]}] caption="XY Graph"
  out "Graph 4":T4(graph)=[{"TimeArray"=[timestamp(3688342761.39444 s since 1904-01-01), timestamp(3688342762.463024 s since 1904-01-01), timestamp(3688342763.463638 s since 1904-01-01), timestamp(3688342764.463637 s since 1904-01-01), timestamp(3688342765.464684 s since 1904-01-01), timestamp(3688342766.465038 s since 1904-01-01), timestamp(3688342767.4661665 s since 1904-01-01), timestamp(3688342768.4671426 s since 1904-01-01), timestamp(3688342769.818876 s since 1904-01-01), timestamp(3688342770.819616 s since 1904-01-01), timestamp(3688342771.819715 s since 1904-01-01), timestamp(3688342772.8190737 s since 1904-01-01), timestamp(3688342773.819743 s since 1904-01-01), timestamp(3688342774.820112 s since 1904-01-01), timestamp(3688342775.820584 s since 1904-01-01), timestamp(3688342776.8214664 s since 1904-01-01), timestamp(3688342777.821848 s since 1904-01-01), timestamp(3688342778.822177 s since 1904-01-01), timestamp(3688342779.8225975 s since 1904-01-01), timestamp(3688342780.8223686 s since 1904-01-01), timestamp(3688342781.8226385 s since 1904-01-01), timestamp(3688342782.8219137 s since 1904-01-01), timestamp(3688342783.8218846 s since 1904-01-01), timestamp(3688342784.821887 s since 1904-01-01), timestamp(3688342785.821828 s since 1904-01-01), timestamp(3688342786.8223386 s since 1904-01-01), timestamp(3688342787.825325 s since 1904-01-01), timestamp(3688342788.8251424 s since 1904-01-01), timestamp(3688342789.825672 s since 1904-01-01), timestamp(3688342790.824856 s since 1904-01-01), timestamp(3688342791.8251505 s since 1904-01-01), timestamp(3688342792.8256593 s since 1904-01-01), timestamp(3688342793.8266897 s since 1904-01-01), timestamp(3688342794.826625 s since 1904-01-01), timestamp(3688342795.825836 s since 1904-01-01), timestamp(3688342796.826832 s since 1904-01-01), timestamp(3688342798.0429673 s since 1904-01-01), timestamp(3688342799.0433993 s since 1904-01-01), timestamp(3688342800.043396 s since 1904-01-01), timestamp(3688342801.0437655 s since 1904-01-01), timestamp(3688342802.0438714 s since 1904-01-01), timestamp(3688342803.043973 s since 1904-01-01), timestamp(3688342804.043901 s since 1904-01-01), timestamp(3688342805.044822 s since 1904-01-01), timestamp(3688342806.0448112 s since 1904-01-01), timestamp(3688342807.045269 s since 1904-01-01), timestamp(3688342808.0455375 s since 1904-01-01), timestamp(3688342809.0448914 s since 1904-01-01)], "DataArray"=[205.57, 205.58, 205.57, 205.56, 205.57, 205.56, 205.57, 205.56, 205.55, 205.57, 205.56, 205.57, 205.57, 205.56, 205.57, 205.57, 205.56, 205.56, 205.56, 205.59, 205.57, 205.57, 205.56, 205.58, 205.58, 205.56, 205.56, 205.58, 205.56, 205.59, 205.56, 205.59, 205.58, 205.57, 205.57, 205.57, 205.58, 205.57, 205.56, 205.58, 205.57, 205.57, 205.56, 205.57, 205.56, 205.59, 205.57, 205.57]}, {"TimeArray"=[timestamp(3688342761.39444 s since 1904-01-01), timestamp(3688342762.463024 s since 1904-01-01), timestamp(3688342763.463638 s since 1904-01-01), timestamp(3688342764.463637 s since 1904-01-01), timestamp(3688342765.464684 s since 1904-01-01), timestamp(3688342766.465038 s since 1904-01-01), timestamp(3688342767.4661665 s since 1904-01-01), timestamp(3688342768.4671426 s since 1904-01-01), timestamp(3688342769.818876 s since 1904-01-01), timestamp(3688342770.819616 s since 1904-01-01), timestamp(3688342771.819715 s since 1904-01-01), timestamp(3688342772.8190737 s since 1904-01-01), timestamp(3688342773.819743 s since 1904-01-01), timestamp(3688342774.820112 s since 1904-01-01), timestamp(3688342775.820584 s since 1904-01-01), timestamp(3688342776.8214664 s since 1904-01-01), timestamp(3688342777.821848 s since 1904-01-01), timestamp(3688342778.822177 s since 1904-01-01), timestamp(3688342779.8225975 s since 1904-01-01), timestamp(3688342780.8223686 s since 1904-01-01), timestamp(3688342781.8226385 s since 1904-01-01), timestamp(3688342782.8219137 s since 1904-01-01), timestamp(3688342783.8218846 s since 1904-01-01), timestamp(3688342784.821887 s since 1904-01-01), timestamp(3688342785.821828 s since 1904-01-01), timestamp(3688342786.8223386 s since 1904-01-01), timestamp(3688342787.825325 s since 1904-01-01), timestamp(3688342788.8251424 s since 1904-01-01), timestamp(3688342789.825672 s since 1904-01-01), timestamp(3688342790.824856 s since 1904-01-01), timestamp(3688342791.8251505 s since 1904-01-01), timestamp(3688342792.8256593 s since 1904-01-01), timestamp(3688342793.8266897 s since 1904-01-01), timestamp(3688342794.826625 s since 1904-01-01), timestamp(3688342795.825836 s since 1904-01-01), timestamp(3688342796.826832 s since 1904-01-01), timestamp(3688342798.0429673 s since 1904-01-01), timestamp(3688342799.0433993 s since 1904-01-01), timestamp(3688342800.043396 s since 1904-01-01), timestamp(3688342801.0437655 s since 1904-01-01), timestamp(3688342802.0438714 s since 1904-01-01), timestamp(3688342803.043973 s since 1904-01-01), timestamp(3688342804.043901 s since 1904-01-01), timestamp(3688342805.044822 s since 1904-01-01), timestamp(3688342806.0448112 s since 1904-01-01), timestamp(3688342807.045269 s since 1904-01-01), timestamp(3688342808.0455375 s since 1904-01-01), timestamp(3688342809.0448914 s since 1904-01-01)], "DataArray"=[197.3, 197.31, 197.31, 197.32, 197.31, 197.31, 197.32, 197.31, 197.32, 197.31, 197.3, 197.32, 197.32, 197.3, 197.3, 197.31, 197.31, 197.31, 197.29, 197.31, 197.31, 197.32, 197.31, 197.32, 197.32, 197.32, 197.31, 197.32, 197.32, 197.32, 197.31, 197.32, 197.31, 197.31, 197.32, 197.33, 197.31, 197.31, 197.31, 197.32, 197.32, 197.32, 197.32, 197.31, 197.32, 197.31, 197.32, 197.31]}, {"TimeArray"=[timestamp(3688342761.39444 s since 1904-01-01), timestamp(3688342762.463024 s since 1904-01-01), timestamp(3688342763.463638 s since 1904-01-01), timestamp(3688342764.463637 s since 1904-01-01), timestamp(3688342765.464684 s since 1904-01-01), timestamp(3688342766.465038 s since 1904-01-01), timestamp(3688342767.4661665 s since 1904-01-01), timestamp(3688342768.4671426 s since 1904-01-01), timestamp(3688342769.818876 s since 1904-01-01), timestamp(3688342770.819616 s since 1904-01-01), timestamp(3688342771.819715 s since 1904-01-01), timestamp(3688342772.8190737 s since 1904-01-01), timestamp(3688342773.819743 s since 1904-01-01), timestamp(3688342774.820112 s since 1904-01-01), timestamp(3688342775.820584 s since 1904-01-01), timestamp(3688342776.8214664 s since 1904-01-01), timestamp(3688342777.821848 s since 1904-01-01), timestamp(3688342778.822177 s since 1904-01-01), timestamp(3688342779.8225975 s since 1904-01-01), timestamp(3688342780.8223686 s since 1904-01-01), timestamp(3688342781.8226385 s since 1904-01-01), timestamp(3688342782.8219137 s since 1904-01-01), timestamp(3688342783.8218846 s since 1904-01-01), timestamp(3688342784.821887 s since 1904-01-01), timestamp(3688342785.821828 s since 1904-01-01), timestamp(3688342786.8223386 s since 1904-01-01), timestamp(3688342787.825325 s since 1904-01-01), timestamp(3688342788.8251424 s since 1904-01-01), timestamp(3688342789.825672 s since 1904-01-01), timestamp(3688342790.824856 s since 1904-01-01), timestamp(3688342791.8251505 s since 1904-01-01), timestamp(3688342792.8256593 s since 1904-01-01), timestamp(3688342793.8266897 s since 1904-01-01), timestamp(3688342794.826625 s since 1904-01-01), timestamp(3688342795.825836 s since 1904-01-01), timestamp(3688342796.826832 s since 1904-01-01), timestamp(3688342798.0429673 s since 1904-01-01), timestamp(3688342799.0433993 s since 1904-01-01), timestamp(3688342800.043396 s since 1904-01-01), timestamp(3688342801.0437655 s since 1904-01-01), timestamp(3688342802.0438714 s since 1904-01-01), timestamp(3688342803.043973 s since 1904-01-01), timestamp(3688342804.043901 s since 1904-01-01), timestamp(3688342805.044822 s since 1904-01-01), timestamp(3688342806.0448112 s since 1904-01-01), timestamp(3688342807.045269 s since 1904-01-01), timestamp(3688342808.0455375 s since 1904-01-01), timestamp(3688342809.0448914 s since 1904-01-01)], "DataArray"=[92.994, 92.994, 92.998, 92.998, 93.004, 92.999, 92.981, 92.997, 92.999, 92.994, 93.0, 93.002, 93.005, 92.998, 93.001, 93.002, 92.993, 92.999, 93.006, 92.989, 93.008, 93.003, 92.996, 93.002, 92.995, 93.003, 93.0, 93.008, 93.014, 93.013, 93.004, 93.001, 93.005, 93.003, 93.002, 93.005, 93.007, 92.99, 93.003, 93.005, 93.014, 93.007, 93.008, 92.997, 93.009, 93.013, 93.008, 93.015]}, {"TimeArray"=[timestamp(3688342761.39444 s since 1904-01-01), timestamp(3688342762.463024 s since 1904-01-01), timestamp(3688342763.463638 s since 1904-01-01), timestamp(3688342764.463637 s since 1904-01-01), timestamp(3688342765.464684 s since 1904-01-01), timestamp(3688342766.465038 s since 1904-01-01), timestamp(3688342767.4661665 s since 1904-01-01), timestamp(3688342768.4671426 s since 1904-01-01), timestamp(3688342769.818876 s since 1904-01-01), timestamp(3688342770.819616 s since 1904-01-01), timestamp(3688342771.819715 s since 1904-01-01), timestamp(3688342772.8190737 s since 1904-01-01), timestamp(3688342773.819743 s since 1904-01-01), timestamp(3688342774.820112 s since 1904-01-01), timestamp(3688342775.820584 s since 1904-01-01), timestamp(3688342776.8214664 s since 1904-01-01), timestamp(3688342777.821848 s since 1904-01-01), timestamp(3688342778.822177 s since 1904-01-01), timestamp(3688342779.8225975 s since 1904-01-01), timestamp(3688342780.8223686 s since 1904-01-01), timestamp(3688342781.8226385 s since 1904-01-01), timestamp(3688342782.8219137 s since 1904-01-01), timestamp(3688342783.8218846 s since 1904-01-01), timestamp(3688342784.821887 s since 1904-01-01), timestamp(3688342785.821828 s since 1904-01-01), timestamp(3688342786.8223386 s since 1904-01-01), timestamp(3688342787.825325 s since 1904-01-01), timestamp(3688342788.8251424 s since 1904-01-01), timestamp(3688342789.825672 s since 1904-01-01), timestamp(3688342790.824856 s since 1904-01-01), timestamp(3688342791.8251505 s since 1904-01-01), timestamp(3688342792.8256593 s since 1904-01-01), timestamp(3688342793.8266897 s since 1904-01-01), timestamp(3688342794.826625 s since 1904-01-01), timestamp(3688342795.825836 s since 1904-01-01), timestamp(3688342796.826832 s since 1904-01-01), timestamp(3688342798.0429673 s since 1904-01-01), timestamp(3688342799.0433993 s since 1904-01-01), timestamp(3688342800.043396 s since 1904-01-01), timestamp(3688342801.0437655 s since 1904-01-01), timestamp(3688342802.0438714 s since 1904-01-01), timestamp(3688342803.043973 s since 1904-01-01), timestamp(3688342804.043901 s since 1904-01-01), timestamp(3688342805.044822 s since 1904-01-01), timestamp(3688342806.0448112 s since 1904-01-01), timestamp(3688342807.045269 s since 1904-01-01), timestamp(3688342808.0455375 s since 1904-01-01), timestamp(3688342809.0448914 s since 1904-01-01)], "DataArray"=[90.402, 90.396, 90.391, 90.4, 90.406, 90.397, 90.406, 90.397, 90.393, 90.399, 90.401, 90.403, 90.412, 90.405, 90.406, 90.409, 90.399, 90.406, 90.403, 90.402, 90.405, 90.406, 90.404, 90.403, 90.408, 90.403, 90.405, 90.41, 90.399, 90.409, 90.4, 90.408, 90.417, 90.408, 90.406, 90.404, 90.41, 90.397, 90.409, 90.398, 90.408, 90.41, 90.408, 90.406, 90.405, 90.407, 90.409, 90.402]}, {"TimeArray"=[timestamp(3688342761.39444 s since 1904-01-01), timestamp(3688342762.463024 s since 1904-01-01), timestamp(3688342763.463638 s since 1904-01-01), timestamp(3688342764.463637 s since 1904-01-01), timestamp(3688342765.464684 s since 1904-01-01), timestamp(3688342766.465038 s since 1904-01-01), timestamp(3688342767.4661665 s since 1904-01-01), timestamp(3688342768.4671426 s since 1904-01-01), timestamp(3688342769.818876 s since 1904-01-01), timestamp(3688342770.819616 s since 1904-01-01), timestamp(3688342771.819715 s since 1904-01-01), timestamp(3688342772.8190737 s since 1904-01-01), timestamp(3688342773.819743 s since 1904-01-01), timestamp(3688342774.820112 s since 1904-01-01), timestamp(3688342775.820584 s since 1904-01-01), timestamp(3688342776.8214664 s since 1904-01-01), timestamp(3688342777.821848 s since 1904-01-01), timestamp(3688342778.822177 s since 1904-01-01), timestamp(3688342779.8225975 s since 1904-01-01), timestamp(3688342780.8223686 s since 1904-01-01), timestamp(3688342781.8226385 s since 1904-01-01), timestamp(3688342782.8219137 s since 1904-01-01), timestamp(3688342783.8218846 s since 1904-01-01), timestamp(3688342784.821887 s since 1904-01-01), timestamp(3688342785.821828 s since 1904-01-01), timestamp(3688342786.8223386 s since 1904-01-01), timestamp(3688342787.825325 s since 1904-01-01), timestamp(3688342788.8251424 s since 1904-01-01), timestamp(3688342789.825672 s since 1904-01-01), timestamp(3688342790.824856 s since 1904-01-01), timestamp(3688342791.8251505 s since 1904-01-01), timestamp(3688342792.8256593 s since 1904-01-01), timestamp(3688342793.8266897 s since 1904-01-01), timestamp(3688342794.826625 s since 1904-01-01), timestamp(3688342795.825836 s since 1904-01-01), timestamp(3688342796.826832 s since 1904-01-01), timestamp(3688342798.0429673 s since 1904-01-01), timestamp(3688342799.0433993 s since 1904-01-01), timestamp(3688342800.043396 s since 1904-01-01), timestamp(3688342801.0437655 s since 1904-01-01), timestamp(3688342802.0438714 s since 1904-01-01), timestamp(3688342803.043973 s since 1904-01-01), timestamp(3688342804.043901 s since 1904-01-01), timestamp(3688342805.044822 s since 1904-01-01), timestamp(3688342806.0448112 s since 1904-01-01), timestamp(3688342807.045269 s since 1904-01-01), timestamp(3688342808.0455375 s since 1904-01-01), timestamp(3688342809.0448914 s since 1904-01-01)], "DataArray"=[59.33, 59.328, 59.328, 59.327, 59.326, 59.326, 59.34, 59.355, 59.356, 59.356, 59.358, 59.357, 59.356, 59.352, 59.352, 59.351, 59.348, 59.347, 59.346, 59.345, 59.342, 59.34, 59.34, 59.338, 59.339, 59.337, 59.338, 59.335, 59.337, 59.335, 59.334, 59.335, 59.334, 59.333, 59.331, 59.331, 59.351, 59.36, 59.358, 59.358, 59.36, 59.357, 59.357, 59.356, 59.353, 59.354, 59.351, 59.35]}, {"TimeArray"=[timestamp(3688342761.39444 s since 1904-01-01), timestamp(3688342762.463024 s since 1904-01-01), timestamp(3688342763.463638 s since 1904-01-01), timestamp(3688342764.463637 s since 1904-01-01), timestamp(3688342765.464684 s since 1904-01-01), timestamp(3688342766.465038 s since 1904-01-01), timestamp(3688342767.4661665 s since 1904-01-01), timestamp(3688342768.4671426 s since 1904-01-01), timestamp(3688342769.818876 s since 1904-01-01), timestamp(3688342770.819616 s since 1904-01-01), timestamp(3688342771.819715 s since 1904-01-01), timestamp(3688342772.8190737 s since 1904-01-01), timestamp(3688342773.819743 s since 1904-01-01), timestamp(3688342774.820112 s since 1904-01-01), timestamp(3688342775.820584 s since 1904-01-01), timestamp(3688342776.8214664 s since 1904-01-01), timestamp(3688342777.821848 s since 1904-01-01), timestamp(3688342778.822177 s since 1904-01-01), timestamp(3688342779.8225975 s since 1904-01-01), timestamp(3688342780.8223686 s since 1904-01-01), timestamp(3688342781.8226385 s since 1904-01-01), timestamp(3688342782.8219137 s since 1904-01-01), timestamp(3688342783.8218846 s since 1904-01-01), timestamp(3688342784.821887 s since 1904-01-01), timestamp(3688342785.821828 s since 1904-01-01), timestamp(3688342786.8223386 s since 1904-01-01), timestamp(3688342787.825325 s since 1904-01-01), timestamp(3688342788.8251424 s since 1904-01-01), timestamp(3688342789.825672 s since 1904-01-01), timestamp(3688342790.824856 s since 1904-01-01), timestamp(3688342791.8251505 s since 1904-01-01), timestamp(3688342792.8256593 s since 1904-01-01), timestamp(3688342793.8266897 s since 1904-01-01), timestamp(3688342794.826625 s since 1904-01-01), timestamp(3688342795.825836 s since 1904-01-01), timestamp(3688342796.826832 s since 1904-01-01), timestamp(3688342798.0429673 s since 1904-01-01), timestamp(3688342799.0433993 s since 1904-01-01), timestamp(3688342800.043396 s since 1904-01-01), timestamp(3688342801.0437655 s since 1904-01-01), timestamp(3688342802.0438714 s since 1904-01-01), timestamp(3688342803.043973 s since 1904-01-01), timestamp(3688342804.043901 s since 1904-01-01), timestamp(3688342805.044822 s since 1904-01-01), timestamp(3688342806.0448112 s since 1904-01-01), timestamp(3688342807.045269 s since 1904-01-01), timestamp(3688342808.0455375 s since 1904-01-01), timestamp(3688342809.0448914 s since 1904-01-01)], "DataArray"=[73.716, 73.721, 73.719, 73.72, 73.727, 73.716, 73.727, 73.718, 73.723, 73.722, 73.717, 73.721, 73.726, 73.727, 73.723, 73.718, 73.728, 73.728, 73.726, 73.723, 73.721, 73.726, 73.724, 73.722, 73.723, 73.721, 73.726, 73.73, 73.726, 73.728, 73.727, 73.729, 73.728, 73.732, 73.728, 73.731, 73.732, 73.73, 73.725, 73.727, 73.729, 73.733, 73.733, 73.727, 73.725, 73.732, 73.73, 73.73]}, {"TimeArray"=[timestamp(3688342761.39444 s since 1904-01-01), timestamp(3688342762.463024 s since 1904-01-01), timestamp(3688342763.463638 s since 1904-01-01), timestamp(3688342764.463637 s since 1904-01-01), timestamp(3688342765.464684 s since 1904-01-01), timestamp(3688342766.465038 s since 1904-01-01), timestamp(3688342767.4661665 s since 1904-01-01), timestamp(3688342768.4671426 s since 1904-01-01), timestamp(3688342769.818876 s since 1904-01-01), timestamp(3688342770.819616 s since 1904-01-01), timestamp(3688342771.819715 s since 1904-01-01), timestamp(3688342772.8190737 s since 1904-01-01), timestamp(3688342773.819743 s since 1904-01-01), timestamp(3688342774.820112 s since 1904-01-01), timestamp(3688342775.820584 s since 1904-01-01), timestamp(3688342776.8214664 s since 1904-01-01), timestamp(3688342777.821848 s since 1904-01-01), timestamp(3688342778.822177 s since 1904-01-01), timestamp(3688342779.8225975 s since 1904-01-01), timestamp(3688342780.8223686 s since 1904-01-01), timestamp(3688342781.8226385 s since 1904-01-01), timestamp(3688342782.8219137 s since 1904-01-01), timestamp(3688342783.8218846 s since 1904-01-01), timestamp(3688342784.821887 s since 1904-01-01), timestamp(3688342785.821828 s since 1904-01-01), timestamp(3688342786.8223386 s since 1904-01-01), timestamp(3688342787.825325 s since 1904-01-01), timestamp(3688342788.8251424 s since 1904-01-01), timestamp(3688342789.825672 s since 1904-01-01), timestamp(3688342790.824856 s since 1904-01-01), timestamp(3688342791.8251505 s since 1904-01-01), timestamp(3688342792.8256593 s since 1904-01-01), timestamp(3688342793.8266897 s since 1904-01-01), timestamp(3688342794.826625 s since 1904-01-01), timestamp(3688342795.825836 s since 1904-01-01), timestamp(3688342796.826832 s since 1904-01-01), timestamp(3688342798.0429673 s since 1904-01-01), timestamp(3688342799.0433993 s since 1904-01-01), timestamp(3688342800.043396 s since 1904-01-01), timestamp(3688342801.0437655 s since 1904-01-01), timestamp(3688342802.0438714 s since 1904-01-01), timestamp(3688342803.043973 s since 1904-01-01), timestamp(3688342804.043901 s since 1904-01-01), timestamp(3688342805.044822 s since 1904-01-01), timestamp(3688342806.0448112 s since 1904-01-01), timestamp(3688342807.045269 s since 1904-01-01), timestamp(3688342808.0455375 s since 1904-01-01), timestamp(3688342809.0448914 s since 1904-01-01)], "DataArray"=[149.38, 149.38, 149.37, 149.38, 149.38, 149.38, 149.38, 149.37, 149.38, 149.38, 149.38, 149.38, 149.38, 149.38, 149.38, 149.38, 149.38, 149.38, 149.38, 149.38, 149.38, 149.38, 149.37, 149.38, 149.39, 149.38, 149.38, 149.38, 149.38, 149.38, 149.38, 149.38, 149.38, 149.38, 149.38, 149.38, 149.39, 149.38, 149.38, 149.38, 149.39, 149.38, 149.38, 149.39, 149.38, 149.38, 149.39, 149.39]}, {"TimeArray"=[timestamp(3688342761.39444 s since 1904-01-01), timestamp(3688342762.463024 s since 1904-01-01), timestamp(3688342763.463638 s since 1904-01-01), timestamp(3688342764.463637 s since 1904-01-01), timestamp(3688342765.464684 s since 1904-01-01), timestamp(3688342766.465038 s since 1904-01-01), timestamp(3688342767.4661665 s since 1904-01-01), timestamp(3688342768.4671426 s since 1904-01-01), timestamp(3688342769.818876 s since 1904-01-01), timestamp(3688342770.819616 s since 1904-01-01), timestamp(3688342771.819715 s since 1904-01-01), timestamp(3688342772.8190737 s since 1904-01-01), timestamp(3688342773.819743 s since 1904-01-01), timestamp(3688342774.820112 s since 1904-01-01), timestamp(3688342775.820584 s since 1904-01-01), timestamp(3688342776.8214664 s since 1904-01-01), timestamp(3688342777.821848 s since 1904-01-01), timestamp(3688342778.822177 s since 1904-01-01), timestamp(3688342779.8225975 s since 1904-01-01), timestamp(3688342780.8223686 s since 1904-01-01), timestamp(3688342781.8226385 s since 1904-01-01), timestamp(3688342782.8219137 s since 1904-01-01), timestamp(3688342783.8218846 s since 1904-01-01), timestamp(3688342784.821887 s since 1904-01-01), timestamp(3688342785.821828 s since 1904-01-01), timestamp(3688342786.8223386 s since 1904-01-01), timestamp(3688342787.825325 s since 1904-01-01), timestamp(3688342788.8251424 s since 1904-01-01), timestamp(3688342789.825672 s since 1904-01-01), timestamp(3688342790.824856 s since 1904-01-01), timestamp(3688342791.8251505 s since 1904-01-01), timestamp(3688342792.8256593 s since 1904-01-01), timestamp(3688342793.8266897 s since 1904-01-01), timestamp(3688342794.826625 s since 1904-01-01), timestamp(3688342795.825836 s since 1904-01-01), timestamp(3688342796.826832 s since 1904-01-01), timestamp(3688342798.0429673 s since 1904-01-01), timestamp(3688342799.0433993 s since 1904-01-01), timestamp(3688342800.043396 s since 1904-01-01), timestamp(3688342801.0437655 s since 1904-01-01), timestamp(3688342802.0438714 s since 1904-01-01), timestamp(3688342803.043973 s since 1904-01-01), timestamp(3688342804.043901 s since 1904-01-01), timestamp(3688342805.044822 s since 1904-01-01), timestamp(3688342806.0448112 s since 1904-01-01), timestamp(3688342807.045269 s since 1904-01-01), timestamp(3688342808.0455375 s since 1904-01-01), timestamp(3688342809.0448914 s since 1904-01-01)], "DataArray"=[148.09, 148.09, 148.1, 148.09, 148.1, 148.08, 148.09, 148.09, 148.08, 148.09, 148.09, 148.08, 148.09, 148.09, 148.09, 148.09, 148.09, 148.09, 148.09, 148.1, 148.09, 148.09, 148.09, 148.1, 148.09, 148.09, 148.09, 148.1, 148.09, 148.09, 148.09, 148.09, 148.1, 148.1, 148.1, 148.09, 148.09, 148.1, 148.1, 148.1, 148.1, 148.1, 148.1, 148.11, 148.09, 148.1, 148.1, 148.1]}, {"TimeArray"=[timestamp(3688342761.39444 s since 1904-01-01), timestamp(3688342762.463024 s since 1904-01-01), timestamp(3688342763.463638 s since 1904-01-01), timestamp(3688342764.463637 s since 1904-01-01), timestamp(3688342765.464684 s since 1904-01-01), timestamp(3688342766.465038 s since 1904-01-01), timestamp(3688342767.4661665 s since 1904-01-01), timestamp(3688342768.4671426 s since 1904-01-01), timestamp(3688342769.818876 s since 1904-01-01), timestamp(3688342770.819616 s since 1904-01-01), timestamp(3688342771.819715 s since 1904-01-01), timestamp(3688342772.8190737 s since 1904-01-01), timestamp(3688342773.819743 s since 1904-01-01), timestamp(3688342774.820112 s since 1904-01-01), timestamp(3688342775.820584 s since 1904-01-01), timestamp(3688342776.8214664 s since 1904-01-01), timestamp(3688342777.821848 s since 1904-01-01), timestamp(3688342778.822177 s since 1904-01-01), timestamp(3688342779.8225975 s since 1904-01-01), timestamp(3688342780.8223686 s since 1904-01-01), timestamp(3688342781.8226385 s since 1904-01-01), timestamp(3688342782.8219137 s since 1904-01-01), timestamp(3688342783.8218846 s since 1904-01-01), timestamp(3688342784.821887 s since 1904-01-01), timestamp(3688342785.821828 s since 1904-01-01), timestamp(3688342786.8223386 s since 1904-01-01), timestamp(3688342787.825325 s since 1904-01-01), timestamp(3688342788.8251424 s since 1904-01-01), timestamp(3688342789.825672 s since 1904-01-01), timestamp(3688342790.824856 s since 1904-01-01), timestamp(3688342791.8251505 s since 1904-01-01), timestamp(3688342792.8256593 s since 1904-01-01), timestamp(3688342793.8266897 s since 1904-01-01), timestamp(3688342794.826625 s since 1904-01-01), timestamp(3688342795.825836 s since 1904-01-01), timestamp(3688342796.826832 s since 1904-01-01), timestamp(3688342798.0429673 s since 1904-01-01), timestamp(3688342799.0433993 s since 1904-01-01), timestamp(3688342800.043396 s since 1904-01-01), timestamp(3688342801.0437655 s since 1904-01-01), timestamp(3688342802.0438714 s since 1904-01-01), timestamp(3688342803.043973 s since 1904-01-01), timestamp(3688342804.043901 s since 1904-01-01), timestamp(3688342805.044822 s since 1904-01-01), timestamp(3688342806.0448112 s since 1904-01-01), timestamp(3688342807.045269 s since 1904-01-01), timestamp(3688342808.0455375 s since 1904-01-01), timestamp(3688342809.0448914 s since 1904-01-01)], "DataArray"=[289.87, 289.87, 289.87, 289.88, 289.87, 289.87, 289.87, 289.87, 289.88, 289.87, 289.87, 289.87, 289.87, 289.87, 289.87, 289.88, 289.87, 289.87, 289.87, 289.87, 289.87, 289.87, 289.87, 289.87, 289.87, 289.87, 289.87, 289.87, 289.87, 289.87, 289.87, 289.87, 289.87, 289.87, 289.88, 289.87, 289.87, 289.87, 289.87, 289.87, 289.87, 289.87, 289.87, 289.87, 289.87, 289.87, 289.88, 289.87]}, {"TimeArray"=[timestamp(3688342761.39444 s since 1904-01-01), timestamp(3688342762.463024 s since 1904-01-01), timestamp(3688342763.463638 s since 1904-01-01), timestamp(3688342764.463637 s since 1904-01-01), timestamp(3688342765.464684 s since 1904-01-01), timestamp(3688342766.465038 s since 1904-01-01), timestamp(3688342767.4661665 s since 1904-01-01), timestamp(3688342768.4671426 s since 1904-01-01), timestamp(3688342769.818876 s since 1904-01-01), timestamp(3688342770.819616 s since 1904-01-01), timestamp(3688342771.819715 s since 1904-01-01), timestamp(3688342772.8190737 s since 1904-01-01), timestamp(3688342773.819743 s since 1904-01-01), timestamp(3688342774.820112 s since 1904-01-01), timestamp(3688342775.820584 s since 1904-01-01), timestamp(3688342776.8214664 s since 1904-01-01), timestamp(3688342777.821848 s since 1904-01-01), timestamp(3688342778.822177 s since 1904-01-01), timestamp(3688342779.8225975 s since 1904-01-01), timestamp(3688342780.8223686 s since 1904-01-01), timestamp(3688342781.8226385 s since 1904-01-01), timestamp(3688342782.8219137 s since 1904-01-01), timestamp(3688342783.8218846 s since 1904-01-01), timestamp(3688342784.821887 s since 1904-01-01), timestamp(3688342785.821828 s since 1904-01-01), timestamp(3688342786.8223386 s since 1904-01-01), timestamp(3688342787.825325 s since 1904-01-01), timestamp(3688342788.8251424 s since 1904-01-01), timestamp(3688342789.825672 s since 1904-01-01), timestamp(3688342790.824856 s since 1904-01-01), timestamp(3688342791.8251505 s since 1904-01-01), timestamp(3688342792.8256593 s since 1904-01-01), timestamp(3688342793.8266897 s since 1904-01-01), timestamp(3688342794.826625 s since 1904-01-01), timestamp(3688342795.825836 s since 1904-01-01), timestamp(3688342796.826832 s since 1904-01-01), timestamp(3688342798.0429673 s since 1904-01-01), timestamp(3688342799.0433993 s since 1904-01-01), timestamp(3688342800.043396 s since 1904-01-01), timestamp(3688342801.0437655 s since 1904-01-01), timestamp(3688342802.0438714 s since 1904-01-01), timestamp(3688342803.043973 s since 1904-01-01), timestamp(3688342804.043901 s since 1904-01-01), timestamp(3688342805.044822 s since 1904-01-01), timestamp(3688342806.0448112 s since 1904-01-01), timestamp(3688342807.045269 s since 1904-01-01), timestamp(3688342808.0455375 s since 1904-01-01), timestamp(3688342809.0448914 s since 1904-01-01)], "DataArray"=[290.02, 290.02, 290.01, 290.01, 290.02, 290.01, 290.01, 290.03, 290.01, 290.02, 290.01, 290.01, 290.01, 290.01, 290.02, 290.0, 290.02, 290.01, 290.01, 290.01, 290.0, 290.02, 290.01, 290.01, 290.01, 290.02, 290.0, 290.01, 290.01, 290.01, 290.01, 290.01, 290.01, 290.02, 290.0, 290.01, 290.02, 290.01, 290.0, 290.01, 290.03, 290.01, 290.01, 290.02, 290.01, 290.02, 290.01, 290.01]}, {"TimeArray"=[timestamp(3688342761.39444 s since 1904-01-01), timestamp(3688342762.463024 s since 1904-01-01), timestamp(3688342763.463638 s since 1904-01-01), timestamp(3688342764.463637 s since 1904-01-01), timestamp(3688342765.464684 s since 1904-01-01), timestamp(3688342766.465038 s since 1904-01-01), timestamp(3688342767.4661665 s since 1904-01-01), timestamp(3688342768.4671426 s since 1904-01-01), timestamp(3688342769.818876 s since 1904-01-01), timestamp(3688342770.819616 s since 1904-01-01), timestamp(3688342771.819715 s since 1904-01-01), timestamp(3688342772.8190737 s since 1904-01-01), timestamp(3688342773.819743 s since 1904-01-01), timestamp(3688342774.820112 s since 1904-01-01), timestamp(3688342775.820584 s since 1904-01-01), timestamp(3688342776.8214664 s since 1904-01-01), timestamp(3688342777.821848 s since 1904-01-01), timestamp(3688342778.822177 s since 1904-01-01), timestamp(3688342779.8225975 s since 1904-01-01), timestamp(3688342780.8223686 s since 1904-01-01), timestamp(3688342781.8226385 s since 1904-01-01), timestamp(3688342782.8219137 s since 1904-01-01), timestamp(3688342783.8218846 s since 1904-01-01), timestamp(3688342784.821887 s since 1904-01-01), timestamp(3688342785.821828 s since 1904-01-01), timestamp(3688342786.8223386 s since 1904-01-01), timestamp(3688342787.825325 s since 1904-01-01), timestamp(3688342788.8251424 s since 1904-01-01), timestamp(3688342789.825672 s since 1904-01-01), timestamp(3688342790.824856 s since 1904-01-01), timestamp(3688342791.8251505 s since 1904-01-01), timestamp(3688342792.8256593 s since 1904-01-01), timestamp(3688342793.8266897 s since 1904-01-01), timestamp(3688342794.826625 s since 1904-01-01), timestamp(3688342795.825836 s since 1904-01-01), timestamp(3688342796.826832 s since 1904-01-01), timestamp(3688342798.0429673 s since 1904-01-01), timestamp(3688342799.0433993 s since 1904-01-01), timestamp(3688342800.043396 s since 1904-01-01), timestamp(3688342801.0437655 s since 1904-01-01), timestamp(3688342802.0438714 s since 1904-01-01), timestamp(3688342803.043973 s since 1904-01-01), timestamp(3688342804.043901 s since 1904-01-01), timestamp(3688342805.044822 s since 1904-01-01), timestamp(3688342806.0448112 s since 1904-01-01), timestamp(3688342807.045269 s since 1904-01-01), timestamp(3688342808.0455375 s since 1904-01-01), timestamp(3688342809.0448914 s since 1904-01-01)], "DataArray"=[289.09, 289.09, 289.09, 289.09, 289.09, 289.09, 289.1, 289.09, 289.09, 289.09, 289.09, 289.09, 289.09, 289.09, 289.09, 289.09, 289.09, 289.09, 289.09, 289.09, 289.09, 289.09, 289.09, 289.09, 289.09, 289.09, 289.09, 289.09, 289.09, 289.09, 289.09, 289.09, 289.09, 289.09, 289.09, 289.09, 289.09, 289.09, 289.09, 289.1, 289.09, 289.09, 289.09, 289.09, 289.09, 289.09, 289.09, 289.1]}, {"TimeArray"=[timestamp(3688342761.39444 s since 1904-01-01), timestamp(3688342762.463024 s since 1904-01-01), timestamp(3688342763.463638 s since 1904-01-01), timestamp(3688342764.463637 s since 1904-01-01), timestamp(3688342765.464684 s since 1904-01-01), timestamp(3688342766.465038 s since 1904-01-01), timestamp(3688342767.4661665 s since 1904-01-01), timestamp(3688342768.4671426 s since 1904-01-01), timestamp(3688342769.818876 s since 1904-01-01), timestamp(3688342770.819616 s since 1904-01-01), timestamp(3688342771.819715 s since 1904-01-01), timestamp(3688342772.8190737 s since 1904-01-01), timestamp(3688342773.819743 s since 1904-01-01), timestamp(3688342774.820112 s since 1904-01-01), timestamp(3688342775.820584 s since 1904-01-01), timestamp(3688342776.8214664 s since 1904-01-01), timestamp(3688342777.821848 s since 1904-01-01), timestamp(3688342778.822177 s since 1904-01-01), timestamp(3688342779.8225975 s since 1904-01-01), timestamp(3688342780.8223686 s since 1904-01-01), timestamp(3688342781.8226385 s since 1904-01-01), timestamp(3688342782.8219137 s since 1904-01-01), timestamp(3688342783.8218846 s since 1904-01-01), timestamp(3688342784.821887 s since 1904-01-01), timestamp(3688342785.821828 s since 1904-01-01), timestamp(3688342786.8223386 s since 1904-01-01), timestamp(3688342787.825325 s since 1904-01-01), timestamp(3688342788.8251424 s since 1904-01-01), timestamp(3688342789.825672 s since 1904-01-01), timestamp(3688342790.824856 s since 1904-01-01), timestamp(3688342791.8251505 s since 1904-01-01), timestamp(3688342792.8256593 s since 1904-01-01), timestamp(3688342793.8266897 s since 1904-01-01), timestamp(3688342794.826625 s since 1904-01-01), timestamp(3688342795.825836 s since 1904-01-01), timestamp(3688342796.826832 s since 1904-01-01), timestamp(3688342798.0429673 s since 1904-01-01), timestamp(3688342799.0433993 s since 1904-01-01), timestamp(3688342800.043396 s since 1904-01-01), timestamp(3688342801.0437655 s since 1904-01-01), timestamp(3688342802.0438714 s since 1904-01-01), timestamp(3688342803.043973 s since 1904-01-01), timestamp(3688342804.043901 s since 1904-01-01), timestamp(3688342805.044822 s since 1904-01-01), timestamp(3688342806.0448112 s since 1904-01-01), timestamp(3688342807.045269 s since 1904-01-01), timestamp(3688342808.0455375 s since 1904-01-01), timestamp(3688342809.0448914 s since 1904-01-01)], "DataArray"=[289.17, 289.16, 289.17, 289.16, 289.17, 289.16, 289.17, 289.16, 289.17, 289.17, 289.17, 289.17, 289.17, 289.17, 289.16, 289.16, 289.17, 289.16, 289.16, 289.17, 289.17, 289.17, 289.17, 289.17, 289.17, 289.17, 289.17, 289.17, 289.17, 289.16, 289.17, 289.17, 289.17, 289.16, 289.17, 289.16, 289.17, 289.16, 289.16, 289.16, 289.17, 289.17, 289.17, 289.17, 289.17, 289.16, 289.16, 289.16]}, {"TimeArray"=[timestamp(3688342761.39444 s since 1904-01-01), timestamp(3688342762.463024 s since 1904-01-01), timestamp(3688342763.463638 s since 1904-01-01), timestamp(3688342764.463637 s since 1904-01-01), timestamp(3688342765.464684 s since 1904-01-01), timestamp(3688342766.465038 s since 1904-01-01), timestamp(3688342767.4661665 s since 1904-01-01), timestamp(3688342768.4671426 s since 1904-01-01), timestamp(3688342769.818876 s since 1904-01-01), timestamp(3688342770.819616 s since 1904-01-01), timestamp(3688342771.819715 s since 1904-01-01), timestamp(3688342772.8190737 s since 1904-01-01), timestamp(3688342773.819743 s since 1904-01-01), timestamp(3688342774.820112 s since 1904-01-01), timestamp(3688342775.820584 s since 1904-01-01), timestamp(3688342776.8214664 s since 1904-01-01), timestamp(3688342777.821848 s since 1904-01-01), timestamp(3688342778.822177 s since 1904-01-01), timestamp(3688342779.8225975 s since 1904-01-01), timestamp(3688342780.8223686 s since 1904-01-01), timestamp(3688342781.8226385 s since 1904-01-01), timestamp(3688342782.8219137 s since 1904-01-01), timestamp(3688342783.8218846 s since 1904-01-01), timestamp(3688342784.821887 s since 1904-01-01), timestamp(3688342785.821828 s since 1904-01-01), timestamp(3688342786.8223386 s since 1904-01-01), timestamp(3688342787.825325 s since 1904-01-01), timestamp(3688342788.8251424 s since 1904-01-01), timestamp(3688342789.825672 s since 1904-01-01), timestamp(3688342790.824856 s since 1904-01-01), timestamp(3688342791.8251505 s since 1904-01-01), timestamp(3688342792.8256593 s since 1904-01-01), timestamp(3688342793.8266897 s since 1904-01-01), timestamp(3688342794.826625 s since 1904-01-01), timestamp(3688342795.825836 s since 1904-01-01), timestamp(3688342796.826832 s since 1904-01-01), timestamp(3688342798.0429673 s since 1904-01-01), timestamp(3688342799.0433993 s since 1904-01-01), timestamp(3688342800.043396 s since 1904-01-01), timestamp(3688342801.0437655 s since 1904-01-01), timestamp(3688342802.0438714 s since 1904-01-01), timestamp(3688342803.043973 s since 1904-01-01), timestamp(3688342804.043901 s since 1904-01-01), timestamp(3688342805.044822 s since 1904-01-01), timestamp(3688342806.0448112 s since 1904-01-01), timestamp(3688342807.045269 s since 1904-01-01), timestamp(3688342808.0455375 s since 1904-01-01), timestamp(3688342809.0448914 s since 1904-01-01)], "DataArray"=[148.0, 147.99, 148.0, 148.0, 148.0, 148.0, 148.0, 148.0, 148.0, 148.0, 148.0, 148.0, 148.0, 148.01, 148.0, 148.0, 148.0, 148.0, 148.01, 148.01, 148.01, 148.01, 148.01, 148.0, 148.01, 148.01, 148.01, 148.01, 148.0, 148.01, 148.01, 148.01, 148.0, 148.01, 148.0, 148.01, 148.01, 148.01, 148.02, 148.01, 148.01, 148.02, 148.01, 148.02, 148.02, 148.02, 148.01, 148.02]}, {"TimeArray"=[timestamp(3688342761.39444 s since 1904-01-01), timestamp(3688342762.463024 s since 1904-01-01), timestamp(3688342763.463638 s since 1904-01-01), timestamp(3688342764.463637 s since 1904-01-01), timestamp(3688342765.464684 s since 1904-01-01), timestamp(3688342766.465038 s since 1904-01-01), timestamp(3688342767.4661665 s since 1904-01-01), timestamp(3688342768.4671426 s since 1904-01-01), timestamp(3688342769.818876 s since 1904-01-01), timestamp(3688342770.819616 s since 1904-01-01), timestamp(3688342771.819715 s since 1904-01-01), timestamp(3688342772.8190737 s since 1904-01-01), timestamp(3688342773.819743 s since 1904-01-01), timestamp(3688342774.820112 s since 1904-01-01), timestamp(3688342775.820584 s since 1904-01-01), timestamp(3688342776.8214664 s since 1904-01-01), timestamp(3688342777.821848 s since 1904-01-01), timestamp(3688342778.822177 s since 1904-01-01), timestamp(3688342779.8225975 s since 1904-01-01), timestamp(3688342780.8223686 s since 1904-01-01), timestamp(3688342781.8226385 s since 1904-01-01), timestamp(3688342782.8219137 s since 1904-01-01), timestamp(3688342783.8218846 s since 1904-01-01), timestamp(3688342784.821887 s since 1904-01-01), timestamp(3688342785.821828 s since 1904-01-01), timestamp(3688342786.8223386 s since 1904-01-01), timestamp(3688342787.825325 s since 1904-01-01), timestamp(3688342788.8251424 s since 1904-01-01), timestamp(3688342789.825672 s since 1904-01-01), timestamp(3688342790.824856 s since 1904-01-01), timestamp(3688342791.8251505 s since 1904-01-01), timestamp(3688342792.8256593 s since 1904-01-01), timestamp(3688342793.8266897 s since 1904-01-01), timestamp(3688342794.826625 s since 1904-01-01), timestamp(3688342795.825836 s since 1904-01-01), timestamp(3688342796.826832 s since 1904-01-01), timestamp(3688342798.0429673 s since 1904-01-01), timestamp(3688342799.0433993 s since 1904-01-01), timestamp(3688342800.043396 s since 1904-01-01), timestamp(3688342801.0437655 s since 1904-01-01), timestamp(3688342802.0438714 s since 1904-01-01), timestamp(3688342803.043973 s since 1904-01-01), timestamp(3688342804.043901 s since 1904-01-01), timestamp(3688342805.044822 s since 1904-01-01), timestamp(3688342806.0448112 s since 1904-01-01), timestamp(3688342807.045269 s since 1904-01-01), timestamp(3688342808.0455375 s since 1904-01-01), timestamp(3688342809.0448914 s since 1904-01-01)], "DataArray"=[152.67, 152.67, 152.67, 152.67, 152.67, 152.67, 152.67, 152.67, 152.67, 152.67, 152.67, 152.67, 152.67, 152.67, 152.68, 152.67, 152.67, 152.67, 152.67, 152.67, 152.67, 152.68, 152.67, 152.67, 152.67, 152.67, 152.68, 152.68, 152.68, 152.68, 152.68, 152.67, 152.68, 152.68, 152.68, 152.67, 152.68, 152.68, 152.68, 152.67, 152.67, 152.68, 152.68, 152.68, 152.68, 152.68, 152.68, 152.67]}, {"TimeArray"=[timestamp(3688342761.39444 s since 1904-01-01), timestamp(3688342762.463024 s since 1904-01-01), timestamp(3688342763.463638 s since 1904-01-01), timestamp(3688342764.463637 s since 1904-01-01), timestamp(3688342765.464684 s since 1904-01-01), timestamp(3688342766.465038 s since 1904-01-01), timestamp(3688342767.4661665 s since 1904-01-01), timestamp(3688342768.4671426 s since 1904-01-01), timestamp(3688342769.818876 s since 1904-01-01), timestamp(3688342770.819616 s since 1904-01-01), timestamp(3688342771.819715 s since 1904-01-01), timestamp(3688342772.8190737 s since 1904-01-01), timestamp(3688342773.819743 s since 1904-01-01), timestamp(3688342774.820112 s since 1904-01-01), timestamp(3688342775.820584 s since 1904-01-01), timestamp(3688342776.8214664 s since 1904-01-01), timestamp(3688342777.821848 s since 1904-01-01), timestamp(3688342778.822177 s since 1904-01-01), timestamp(3688342779.8225975 s since 1904-01-01), timestamp(3688342780.8223686 s since 1904-01-01), timestamp(3688342781.8226385 s since 1904-01-01), timestamp(3688342782.8219137 s since 1904-01-01), timestamp(3688342783.8218846 s since 1904-01-01), timestamp(3688342784.821887 s since 1904-01-01), timestamp(3688342785.821828 s since 1904-01-01), timestamp(3688342786.8223386 s since 1904-01-01), timestamp(3688342787.825325 s since 1904-01-01), timestamp(3688342788.8251424 s since 1904-01-01), timestamp(3688342789.825672 s since 1904-01-01), timestamp(3688342790.824856 s since 1904-01-01), timestamp(3688342791.8251505 s since 1904-01-01), timestamp(3688342792.8256593 s since 1904-01-01), timestamp(3688342793.8266897 s since 1904-01-01), timestamp(3688342794.826625 s since 1904-01-01), timestamp(3688342795.825836 s since 1904-01-01), timestamp(3688342796.826832 s since 1904-01-01), timestamp(3688342798.0429673 s since 1904-01-01), timestamp(3688342799.0433993 s since 1904-01-01), timestamp(3688342800.043396 s since 1904-01-01), timestamp(3688342801.0437655 s since 1904-01-01), timestamp(3688342802.0438714 s since 1904-01-01), timestamp(3688342803.043973 s since 1904-01-01), timestamp(3688342804.043901 s since 1904-01-01), timestamp(3688342805.044822 s since 1904-01-01), timestamp(3688342806.0448112 s since 1904-01-01), timestamp(3688342807.045269 s since 1904-01-01), timestamp(3688342808.0455375 s since 1904-01-01), timestamp(3688342809.0448914 s since 1904-01-01)], "DataArray"=[122.78, 122.78, 122.78, 122.78, 122.77, 122.78, 122.78, 122.79, 122.79, 122.78, 122.78, 122.78, 122.78, 122.78, 122.78, 122.78, 122.78, 122.78, 122.79, 122.78, 122.78, 122.79, 122.79, 122.78, 122.79, 122.78, 122.79, 122.79, 122.79, 122.78, 122.79, 122.79, 122.79, 122.79, 122.78, 122.79, 122.78, 122.79, 122.79, 122.79, 122.79, 122.79, 122.79, 122.79, 122.79, 122.79, 122.8, 122.79]}, {"TimeArray"=[timestamp(3688342761.39444 s since 1904-01-01), timestamp(3688342762.463024 s since 1904-01-01), timestamp(3688342763.463638 s since 1904-01-01), timestamp(3688342764.463637 s since 1904-01-01), timestamp(3688342765.464684 s since 1904-01-01), timestamp(3688342766.465038 s since 1904-01-01), timestamp(3688342767.4661665 s since 1904-01-01), timestamp(3688342768.4671426 s since 1904-01-01), timestamp(3688342769.818876 s since 1904-01-01), timestamp(3688342770.819616 s since 1904-01-01), timestamp(3688342771.819715 s since 1904-01-01), timestamp(3688342772.8190737 s since 1904-01-01), timestamp(3688342773.819743 s since 1904-01-01), timestamp(3688342774.820112 s since 1904-01-01), timestamp(3688342775.820584 s since 1904-01-01), timestamp(3688342776.8214664 s since 1904-01-01), timestamp(3688342777.821848 s since 1904-01-01), timestamp(3688342778.822177 s since 1904-01-01), timestamp(3688342779.8225975 s since 1904-01-01), timestamp(3688342780.8223686 s since 1904-01-01), timestamp(3688342781.8226385 s since 1904-01-01), timestamp(3688342782.8219137 s since 1904-01-01), timestamp(3688342783.8218846 s since 1904-01-01), timestamp(3688342784.821887 s since 1904-01-01), timestamp(3688342785.821828 s since 1904-01-01), timestamp(3688342786.8223386 s since 1904-01-01), timestamp(3688342787.825325 s since 1904-01-01), timestamp(3688342788.8251424 s since 1904-01-01), timestamp(3688342789.825672 s since 1904-01-01), timestamp(3688342790.824856 s since 1904-01-01), timestamp(3688342791.8251505 s since 1904-01-01), timestamp(3688342792.8256593 s since 1904-01-01), timestamp(3688342793.8266897 s since 1904-01-01), timestamp(3688342794.826625 s since 1904-01-01), timestamp(3688342795.825836 s since 1904-01-01), timestamp(3688342796.826832 s since 1904-01-01), timestamp(3688342798.0429673 s since 1904-01-01), timestamp(3688342799.0433993 s since 1904-01-01), timestamp(3688342800.043396 s since 1904-01-01), timestamp(3688342801.0437655 s since 1904-01-01), timestamp(3688342802.0438714 s since 1904-01-01), timestamp(3688342803.043973 s since 1904-01-01), timestamp(3688342804.043901 s since 1904-01-01), timestamp(3688342805.044822 s since 1904-01-01), timestamp(3688342806.0448112 s since 1904-01-01), timestamp(3688342807.045269 s since 1904-01-01), timestamp(3688342808.0455375 s since 1904-01-01), timestamp(3688342809.0448914 s since 1904-01-01)], "DataArray"=[59.37, 59.244, 59.409, 59.412, 59.409, 59.507, 59.523, 59.408, 59.417, 59.62, 59.619, 59.414, 59.406, 59.395, 59.209, 59.412, 59.414, 59.413, 59.464, 59.61, 59.429, 59.42, 59.421, 59.338, 59.271, 59.425, 59.419, 59.494, 59.59, 59.436, 59.415, 59.417, 59.311, 59.311, 59.42, 59.432, 59.385, 59.237, 59.429, 59.432, 59.462, 59.641, 59.444, 59.432, 59.44, 59.388, 59.261, 59.451]}, {"TimeArray"=[timestamp(3688342761.39444 s since 1904-01-01), timestamp(3688342762.463024 s since 1904-01-01), timestamp(3688342763.463638 s since 1904-01-01), timestamp(3688342764.463637 s since 1904-01-01), timestamp(3688342765.464684 s since 1904-01-01), timestamp(3688342766.465038 s since 1904-01-01), timestamp(3688342767.4661665 s since 1904-01-01), timestamp(3688342768.4671426 s since 1904-01-01), timestamp(3688342769.818876 s since 1904-01-01), timestamp(3688342770.819616 s since 1904-01-01), timestamp(3688342771.819715 s since 1904-01-01), timestamp(3688342772.8190737 s since 1904-01-01), timestamp(3688342773.819743 s since 1904-01-01), timestamp(3688342774.820112 s since 1904-01-01), timestamp(3688342775.820584 s since 1904-01-01), timestamp(3688342776.8214664 s since 1904-01-01), timestamp(3688342777.821848 s since 1904-01-01), timestamp(3688342778.822177 s since 1904-01-01), timestamp(3688342779.8225975 s since 1904-01-01), timestamp(3688342780.8223686 s since 1904-01-01), timestamp(3688342781.8226385 s since 1904-01-01), timestamp(3688342782.8219137 s since 1904-01-01), timestamp(3688342783.8218846 s since 1904-01-01), timestamp(3688342784.821887 s since 1904-01-01), timestamp(3688342785.821828 s since 1904-01-01), timestamp(3688342786.8223386 s since 1904-01-01), timestamp(3688342787.825325 s since 1904-01-01), timestamp(3688342788.8251424 s since 1904-01-01), timestamp(3688342789.825672 s since 1904-01-01), timestamp(3688342790.824856 s since 1904-01-01), timestamp(3688342791.8251505 s since 1904-01-01), timestamp(3688342792.8256593 s since 1904-01-01), timestamp(3688342793.8266897 s since 1904-01-01), timestamp(3688342794.826625 s since 1904-01-01), timestamp(3688342795.825836 s since 1904-01-01), timestamp(3688342796.826832 s since 1904-01-01), timestamp(3688342798.0429673 s since 1904-01-01), timestamp(3688342799.0433993 s since 1904-01-01), timestamp(3688342800.043396 s since 1904-01-01), timestamp(3688342801.0437655 s since 1904-01-01), timestamp(3688342802.0438714 s since 1904-01-01), timestamp(3688342803.043973 s since 1904-01-01), timestamp(3688342804.043901 s since 1904-01-01), timestamp(3688342805.044822 s since 1904-01-01), timestamp(3688342806.0448112 s since 1904-01-01), timestamp(3688342807.045269 s since 1904-01-01), timestamp(3688342808.0455375 s since 1904-01-01), timestamp(3688342809.0448914 s since 1904-01-01)], "DataArray"=[49.133, 49.144, 49.287, 49.164, 49.117, 49.104, 48.956, 49.074, 49.116, 49.121, 49.044, 49.006, 49.131, 49.14, 49.137, 49.243, 49.211, 49.115, 49.116, 49.018, 49.03, 49.138, 49.145, 49.142, 49.277, 49.192, 49.12, 49.119, 49.116, 48.964, 49.101, 49.135, 49.146, 49.289, 49.167, 49.12, 49.128, 49.115, 48.953, 49.125, 49.137, 49.144, 49.172, 49.163, 49.132, 49.138, 49.115, 48.966]}, {"TimeArray"=[timestamp(3688342761.39444 s since 1904-01-01), timestamp(3688342762.463024 s since 1904-01-01), timestamp(3688342763.463638 s since 1904-01-01), timestamp(3688342764.463637 s since 1904-01-01), timestamp(3688342765.464684 s since 1904-01-01), timestamp(3688342766.465038 s since 1904-01-01), timestamp(3688342767.4661665 s since 1904-01-01), timestamp(3688342768.4671426 s since 1904-01-01), timestamp(3688342769.818876 s since 1904-01-01), timestamp(3688342770.819616 s since 1904-01-01), timestamp(3688342771.819715 s since 1904-01-01), timestamp(3688342772.8190737 s since 1904-01-01), timestamp(3688342773.819743 s since 1904-01-01), timestamp(3688342774.820112 s since 1904-01-01), timestamp(3688342775.820584 s since 1904-01-01), timestamp(3688342776.8214664 s since 1904-01-01), timestamp(3688342777.821848 s since 1904-01-01), timestamp(3688342778.822177 s since 1904-01-01), timestamp(3688342779.8225975 s since 1904-01-01), timestamp(3688342780.8223686 s since 1904-01-01), timestamp(3688342781.8226385 s since 1904-01-01), timestamp(3688342782.8219137 s since 1904-01-01), timestamp(3688342783.8218846 s since 1904-01-01), timestamp(3688342784.821887 s since 1904-01-01), timestamp(3688342785.821828 s since 1904-01-01), timestamp(3688342786.8223386 s since 1904-01-01), timestamp(3688342787.825325 s since 1904-01-01), timestamp(3688342788.8251424 s since 1904-01-01), timestamp(3688342789.825672 s since 1904-01-01), timestamp(3688342790.824856 s since 1904-01-01), timestamp(3688342791.8251505 s since 1904-01-01), timestamp(3688342792.8256593 s since 1904-01-01), timestamp(3688342793.8266897 s since 1904-01-01), timestamp(3688342794.826625 s since 1904-01-01), timestamp(3688342795.825836 s since 1904-01-01), timestamp(3688342796.826832 s since 1904-01-01), timestamp(3688342798.0429673 s since 1904-01-01), timestamp(3688342799.0433993 s since 1904-01-01), timestamp(3688342800.043396 s since 1904-01-01), timestamp(3688342801.0437655 s since 1904-01-01), timestamp(3688342802.0438714 s since 1904-01-01), timestamp(3688342803.043973 s since 1904-01-01), timestamp(3688342804.043901 s since 1904-01-01), timestamp(3688342805.044822 s since 1904-01-01), timestamp(3688342806.0448112 s since 1904-01-01), timestamp(3688342807.045269 s since 1904-01-01), timestamp(3688342808.0455375 s since 1904-01-01), timestamp(3688342809.0448914 s since 1904-01-01)], "DataArray"=[66.806, 66.731, 66.73, 66.717, 66.743, 66.739, 66.74, 66.747, 66.736, 66.735, 66.741, 66.746, 66.742, 66.736, 66.737, 66.741, 66.729, 66.741, 66.746, 66.735, 66.733, 66.756, 66.746, 66.741, 66.749, 66.733, 66.735, 66.741, 66.741, 66.739, 66.754, 66.752, 66.751, 66.754, 66.743, 66.728, 66.743, 66.744, 66.753, 66.779, 66.763, 66.753, 66.751, 66.738, 66.733, 66.763, 66.761, 66.774]}, {"TimeArray"=[timestamp(3688342761.39444 s since 1904-01-01), timestamp(3688342762.463024 s since 1904-01-01), timestamp(3688342763.463638 s since 1904-01-01), timestamp(3688342764.463637 s since 1904-01-01), timestamp(3688342765.464684 s since 1904-01-01), timestamp(3688342766.465038 s since 1904-01-01), timestamp(3688342767.4661665 s since 1904-01-01), timestamp(3688342768.4671426 s since 1904-01-01), timestamp(3688342769.818876 s since 1904-01-01), timestamp(3688342770.819616 s since 1904-01-01), timestamp(3688342771.819715 s since 1904-01-01), timestamp(3688342772.8190737 s since 1904-01-01), timestamp(3688342773.819743 s since 1904-01-01), timestamp(3688342774.820112 s since 1904-01-01), timestamp(3688342775.820584 s since 1904-01-01), timestamp(3688342776.8214664 s since 1904-01-01), timestamp(3688342777.821848 s since 1904-01-01), timestamp(3688342778.822177 s since 1904-01-01), timestamp(3688342779.8225975 s since 1904-01-01), timestamp(3688342780.8223686 s since 1904-01-01), timestamp(3688342781.8226385 s since 1904-01-01), timestamp(3688342782.8219137 s since 1904-01-01), timestamp(3688342783.8218846 s since 1904-01-01), timestamp(3688342784.821887 s since 1904-01-01), timestamp(3688342785.821828 s since 1904-01-01), timestamp(3688342786.8223386 s since 1904-01-01), timestamp(3688342787.825325 s since 1904-01-01), timestamp(3688342788.8251424 s since 1904-01-01), timestamp(3688342789.825672 s since 1904-01-01), timestamp(3688342790.824856 s since 1904-01-01), timestamp(3688342791.8251505 s since 1904-01-01), timestamp(3688342792.8256593 s since 1904-01-01), timestamp(3688342793.8266897 s since 1904-01-01), timestamp(3688342794.826625 s since 1904-01-01), timestamp(3688342795.825836 s since 1904-01-01), timestamp(3688342796.826832 s since 1904-01-01), timestamp(3688342798.0429673 s since 1904-01-01), timestamp(3688342799.0433993 s since 1904-01-01), timestamp(3688342800.043396 s since 1904-01-01), timestamp(3688342801.0437655 s since 1904-01-01), timestamp(3688342802.0438714 s since 1904-01-01), timestamp(3688342803.043973 s since 1904-01-01), timestamp(3688342804.043901 s since 1904-01-01), timestamp(3688342805.044822 s since 1904-01-01), timestamp(3688342806.0448112 s since 1904-01-01), timestamp(3688342807.045269 s since 1904-01-01), timestamp(3688342808.0455375 s since 1904-01-01), timestamp(3688342809.0448914 s since 1904-01-01)], "DataArray"=[44.0656, 44.0661, 44.0687, 44.0686, 44.0657, 44.0665, 44.0683, 44.0655, 44.0686, 44.0681, 44.0714, 44.0673, 44.0696, 44.0713, 44.0706, 44.0674, 44.0686, 44.0686, 44.0706, 44.0691, 44.0709, 44.0689, 44.0732, 44.0686, 44.0707, 44.0713, 44.0706, 44.0679, 44.0728, 44.071, 44.0694, 44.0714, 44.07, 44.0726, 44.0711, 44.0718, 44.0716, 44.0723, 44.0717, 44.0725, 44.0703, 44.0724, 44.0742, 44.0735, 44.0725, 44.0739, 44.0707, 44.0737]}, {"TimeArray"=[timestamp(3688342761.39444 s since 1904-01-01), timestamp(3688342762.463024 s since 1904-01-01), timestamp(3688342763.463638 s since 1904-01-01), timestamp(3688342764.463637 s since 1904-01-01), timestamp(3688342765.464684 s since 1904-01-01), timestamp(3688342766.465038 s since 1904-01-01), timestamp(3688342767.4661665 s since 1904-01-01), timestamp(3688342768.4671426 s since 1904-01-01), timestamp(3688342769.818876 s since 1904-01-01), timestamp(3688342770.819616 s since 1904-01-01), timestamp(3688342771.819715 s since 1904-01-01), timestamp(3688342772.8190737 s since 1904-01-01), timestamp(3688342773.819743 s since 1904-01-01), timestamp(3688342774.820112 s since 1904-01-01), timestamp(3688342775.820584 s since 1904-01-01), timestamp(3688342776.8214664 s since 1904-01-01), timestamp(3688342777.821848 s since 1904-01-01), timestamp(3688342778.822177 s since 1904-01-01), timestamp(3688342779.8225975 s since 1904-01-01), timestamp(3688342780.8223686 s since 1904-01-01), timestamp(3688342781.8226385 s since 1904-01-01), timestamp(3688342782.8219137 s since 1904-01-01), timestamp(3688342783.8218846 s since 1904-01-01), timestamp(3688342784.821887 s since 1904-01-01), timestamp(3688342785.821828 s since 1904-01-01), timestamp(3688342786.8223386 s since 1904-01-01), timestamp(3688342787.825325 s since 1904-01-01), timestamp(3688342788.8251424 s since 1904-01-01), timestamp(3688342789.825672 s since 1904-01-01), timestamp(3688342790.824856 s since 1904-01-01), timestamp(3688342791.8251505 s since 1904-01-01), timestamp(3688342792.8256593 s since 1904-01-01), timestamp(3688342793.8266897 s since 1904-01-01), timestamp(3688342794.826625 s since 1904-01-01), timestamp(3688342795.825836 s since 1904-01-01), timestamp(3688342796.826832 s since 1904-01-01), timestamp(3688342798.0429673 s since 1904-01-01), timestamp(3688342799.0433993 s since 1904-01-01), timestamp(3688342800.043396 s since 1904-01-01), timestamp(3688342801.0437655 s since 1904-01-01), timestamp(3688342802.0438714 s since 1904-01-01), timestamp(3688342803.043973 s since 1904-01-01), timestamp(3688342804.043901 s since 1904-01-01), timestamp(3688342805.044822 s since 1904-01-01), timestamp(3688342806.0448112 s since 1904-01-01), timestamp(3688342807.045269 s since 1904-01-01), timestamp(3688342808.0455375 s since 1904-01-01), timestamp(3688342809.0448914 s since 1904-01-01)], "DataArray"=[44.0449, 44.0437, 44.0434, 44.043, 44.0461, 44.0431, 44.0439, 44.0452, 44.0442, 44.0463, 44.0436, 44.0451, 44.0473, 44.0456, 44.0463, 44.0445, 44.0434, 44.0434, 44.0462, 44.0458, 44.0454, 44.0467, 44.0482, 44.0442, 44.0482, 44.0464, 44.0462, 44.0458, 44.0461, 44.048, 44.048, 44.0462, 44.0474, 44.0483, 44.0454, 44.0492, 44.0461, 44.048, 44.0498, 44.0494, 44.0502, 44.0498, 44.0469, 44.0504, 44.0485, 44.0496, 44.0491, 44.0488]}, {"TimeArray"=[timestamp(3688342761.39444 s since 1904-01-01), timestamp(3688342762.463024 s since 1904-01-01), timestamp(3688342763.463638 s since 1904-01-01), timestamp(3688342764.463637 s since 1904-01-01), timestamp(3688342765.464684 s since 1904-01-01), timestamp(3688342766.465038 s since 1904-01-01), timestamp(3688342767.4661665 s since 1904-01-01), timestamp(3688342768.4671426 s since 1904-01-01), timestamp(3688342769.818876 s since 1904-01-01), timestamp(3688342770.819616 s since 1904-01-01), timestamp(3688342771.819715 s since 1904-01-01), timestamp(3688342772.8190737 s since 1904-01-01), timestamp(3688342773.819743 s since 1904-01-01), timestamp(3688342774.820112 s since 1904-01-01), timestamp(3688342775.820584 s since 1904-01-01), timestamp(3688342776.8214664 s since 1904-01-01), timestamp(3688342777.821848 s since 1904-01-01), timestamp(3688342778.822177 s since 1904-01-01), timestamp(3688342779.8225975 s since 1904-01-01), timestamp(3688342780.8223686 s since 1904-01-01), timestamp(3688342781.8226385 s since 1904-01-01), timestamp(3688342782.8219137 s since 1904-01-01), timestamp(3688342783.8218846 s since 1904-01-01), timestamp(3688342784.821887 s since 1904-01-01), timestamp(3688342785.821828 s since 1904-01-01), timestamp(3688342786.8223386 s since 1904-01-01), timestamp(3688342787.825325 s since 1904-01-01), timestamp(3688342788.8251424 s since 1904-01-01), timestamp(3688342789.825672 s since 1904-01-01), timestamp(3688342790.824856 s since 1904-01-01), timestamp(3688342791.8251505 s since 1904-01-01), timestamp(3688342792.8256593 s since 1904-01-01), timestamp(3688342793.8266897 s since 1904-01-01), timestamp(3688342794.826625 s since 1904-01-01), timestamp(3688342795.825836 s since 1904-01-01), timestamp(3688342796.826832 s since 1904-01-01), timestamp(3688342798.0429673 s since 1904-01-01), timestamp(3688342799.0433993 s since 1904-01-01), timestamp(3688342800.043396 s since 1904-01-01), timestamp(3688342801.0437655 s since 1904-01-01), timestamp(3688342802.0438714 s since 1904-01-01), timestamp(3688342803.043973 s since 1904-01-01), timestamp(3688342804.043901 s since 1904-01-01), timestamp(3688342805.044822 s since 1904-01-01), timestamp(3688342806.0448112 s since 1904-01-01), timestamp(3688342807.045269 s since 1904-01-01), timestamp(3688342808.0455375 s since 1904-01-01), timestamp(3688342809.0448914 s since 1904-01-01)], "DataArray"=[63.4418, 63.4423, 63.4445, 63.4448, 63.4482, 63.4469, 63.4445, 63.4441, 63.4478, 63.4441, 63.4476, 63.448, 63.4482, 63.4487, 63.4517, 63.4515, 63.4492, 63.4509, 63.4498, 63.4486, 63.45, 63.4523, 63.449, 63.4486, 63.4542, 63.4507, 63.4509, 63.4538, 63.4578, 63.4525, 63.4501, 63.4528, 63.4525, 63.4509, 63.454, 63.4586, 63.4546, 63.4554, 63.4549, 63.4558, 63.4557, 63.4568, 63.4552, 63.4545, 63.4606, 63.4591, 63.4594, 63.4557]}, {"TimeArray"=[timestamp(3688342761.39444 s since 1904-01-01), timestamp(3688342762.463024 s since 1904-01-01), timestamp(3688342763.463638 s since 1904-01-01), timestamp(3688342764.463637 s since 1904-01-01), timestamp(3688342765.464684 s since 1904-01-01), timestamp(3688342766.465038 s since 1904-01-01), timestamp(3688342767.4661665 s since 1904-01-01), timestamp(3688342768.4671426 s since 1904-01-01), timestamp(3688342769.818876 s since 1904-01-01), timestamp(3688342770.819616 s since 1904-01-01), timestamp(3688342771.819715 s since 1904-01-01), timestamp(3688342772.8190737 s since 1904-01-01), timestamp(3688342773.819743 s since 1904-01-01), timestamp(3688342774.820112 s since 1904-01-01), timestamp(3688342775.820584 s since 1904-01-01), timestamp(3688342776.8214664 s since 1904-01-01), timestamp(3688342777.821848 s since 1904-01-01), timestamp(3688342778.822177 s since 1904-01-01), timestamp(3688342779.8225975 s since 1904-01-01), timestamp(3688342780.8223686 s since 1904-01-01), timestamp(3688342781.8226385 s since 1904-01-01), timestamp(3688342782.8219137 s since 1904-01-01), timestamp(3688342783.8218846 s since 1904-01-01), timestamp(3688342784.821887 s since 1904-01-01), timestamp(3688342785.821828 s since 1904-01-01), timestamp(3688342786.8223386 s since 1904-01-01), timestamp(3688342787.825325 s since 1904-01-01), timestamp(3688342788.8251424 s since 1904-01-01), timestamp(3688342789.825672 s since 1904-01-01), timestamp(3688342790.824856 s since 1904-01-01), timestamp(3688342791.8251505 s since 1904-01-01), timestamp(3688342792.8256593 s since 1904-01-01), timestamp(3688342793.8266897 s since 1904-01-01), timestamp(3688342794.826625 s since 1904-01-01), timestamp(3688342795.825836 s since 1904-01-01), timestamp(3688342796.826832 s since 1904-01-01), timestamp(3688342798.0429673 s since 1904-01-01), timestamp(3688342799.0433993 s since 1904-01-01), timestamp(3688342800.043396 s since 1904-01-01), timestamp(3688342801.0437655 s since 1904-01-01), timestamp(3688342802.0438714 s since 1904-01-01), timestamp(3688342803.043973 s since 1904-01-01), timestamp(3688342804.043901 s since 1904-01-01), timestamp(3688342805.044822 s since 1904-01-01), timestamp(3688342806.0448112 s since 1904-01-01), timestamp(3688342807.045269 s since 1904-01-01), timestamp(3688342808.0455375 s since 1904-01-01), timestamp(3688342809.0448914 s since 1904-01-01)], "DataArray"=[53.3249, 53.3229, 53.324, 53.3229, 53.3256, 53.3269, 53.3236, 53.3239, 53.3292, 53.3269, 53.3269, 53.3267, 53.3293, 53.3271, 53.3292, 53.3286, 53.3275, 53.3256, 53.3268, 53.3308, 53.3274, 53.3291, 53.3261, 53.3272, 53.3339, 53.329, 53.3299, 53.3321, 53.3332, 53.3271, 53.3305, 53.3293, 53.3315, 53.3314, 53.3339, 53.3352, 53.3287, 53.3326, 53.3304, 53.3313, 53.3335, 53.3385, 53.3293, 53.3318, 53.3364, 53.3319, 53.3341, 53.3294]}, {"TimeArray"=[timestamp(3688342761.39444 s since 1904-01-01), timestamp(3688342762.463024 s since 1904-01-01), timestamp(3688342763.463638 s since 1904-01-01), timestamp(3688342764.463637 s since 1904-01-01), timestamp(3688342765.464684 s since 1904-01-01), timestamp(3688342766.465038 s since 1904-01-01), timestamp(3688342767.4661665 s since 1904-01-01), timestamp(3688342768.4671426 s since 1904-01-01), timestamp(3688342769.818876 s since 1904-01-01), timestamp(3688342770.819616 s since 1904-01-01), timestamp(3688342771.819715 s since 1904-01-01), timestamp(3688342772.8190737 s since 1904-01-01), timestamp(3688342773.819743 s since 1904-01-01), timestamp(3688342774.820112 s since 1904-01-01), timestamp(3688342775.820584 s since 1904-01-01), timestamp(3688342776.8214664 s since 1904-01-01), timestamp(3688342777.821848 s since 1904-01-01), timestamp(3688342778.822177 s since 1904-01-01), timestamp(3688342779.8225975 s since 1904-01-01), timestamp(3688342780.8223686 s since 1904-01-01), timestamp(3688342781.8226385 s since 1904-01-01), timestamp(3688342782.8219137 s since 1904-01-01), timestamp(3688342783.8218846 s since 1904-01-01), timestamp(3688342784.821887 s since 1904-01-01), timestamp(3688342785.821828 s since 1904-01-01), timestamp(3688342786.8223386 s since 1904-01-01), timestamp(3688342787.825325 s since 1904-01-01), timestamp(3688342788.8251424 s since 1904-01-01), timestamp(3688342789.825672 s since 1904-01-01), timestamp(3688342790.824856 s since 1904-01-01), timestamp(3688342791.8251505 s since 1904-01-01), timestamp(3688342792.8256593 s since 1904-01-01), timestamp(3688342793.8266897 s since 1904-01-01), timestamp(3688342794.826625 s since 1904-01-01), timestamp(3688342795.825836 s since 1904-01-01), timestamp(3688342796.826832 s since 1904-01-01), timestamp(3688342798.0429673 s since 1904-01-01), timestamp(3688342799.0433993 s since 1904-01-01), timestamp(3688342800.043396 s since 1904-01-01), timestamp(3688342801.0437655 s since 1904-01-01), timestamp(3688342802.0438714 s since 1904-01-01), timestamp(3688342803.043973 s since 1904-01-01), timestamp(3688342804.043901 s since 1904-01-01), timestamp(3688342805.044822 s since 1904-01-01), timestamp(3688342806.0448112 s since 1904-01-01), timestamp(3688342807.045269 s since 1904-01-01), timestamp(3688342808.0455375 s since 1904-01-01), timestamp(3688342809.0448914 s since 1904-01-01)], "DataArray"=[56.562, 56.5688, 56.5642, 56.568, 56.5712, 56.5685, 56.5708, 56.5722, 56.5674, 56.5677, 56.5663, 56.5693, 56.5666, 56.5681, 56.5663, 56.5728, 56.5666, 56.5681, 56.5714, 56.5684, 56.5697, 56.5695, 56.567, 56.5674, 56.5714, 56.5709, 56.5678, 56.572, 56.5723, 56.5681, 56.5696, 56.5733, 56.5708, 56.5718, 56.5714, 56.571, 56.5699, 56.5743, 56.5765, 56.5759, 56.5725, 56.5688, 56.5701, 56.5693, 56.5742, 56.5707, 56.5713, 56.5704]}, {"TimeArray"=[timestamp(3688342761.39444 s since 1904-01-01), timestamp(3688342762.463024 s since 1904-01-01), timestamp(3688342763.463638 s since 1904-01-01), timestamp(3688342764.463637 s since 1904-01-01), timestamp(3688342765.464684 s since 1904-01-01), timestamp(3688342766.465038 s since 1904-01-01), timestamp(3688342767.4661665 s since 1904-01-01), timestamp(3688342768.4671426 s since 1904-01-01), timestamp(3688342769.818876 s since 1904-01-01), timestamp(3688342770.819616 s since 1904-01-01), timestamp(3688342771.819715 s since 1904-01-01), timestamp(3688342772.8190737 s since 1904-01-01), timestamp(3688342773.819743 s since 1904-01-01), timestamp(3688342774.820112 s since 1904-01-01), timestamp(3688342775.820584 s since 1904-01-01), timestamp(3688342776.8214664 s since 1904-01-01), timestamp(3688342777.821848 s since 1904-01-01), timestamp(3688342778.822177 s since 1904-01-01), timestamp(3688342779.8225975 s since 1904-01-01), timestamp(3688342780.8223686 s since 1904-01-01), timestamp(3688342781.8226385 s since 1904-01-01), timestamp(3688342782.8219137 s since 1904-01-01), timestamp(3688342783.8218846 s since 1904-01-01), timestamp(3688342784.821887 s since 1904-01-01), timestamp(3688342785.821828 s since 1904-01-01), timestamp(3688342786.8223386 s since 1904-01-01), timestamp(3688342787.825325 s since 1904-01-01), timestamp(3688342788.8251424 s since 1904-01-01), timestamp(3688342789.825672 s since 1904-01-01), timestamp(3688342790.824856 s since 1904-01-01), timestamp(3688342791.8251505 s since 1904-01-01), timestamp(3688342792.8256593 s since 1904-01-01), timestamp(3688342793.8266897 s since 1904-01-01), timestamp(3688342794.826625 s since 1904-01-01), timestamp(3688342795.825836 s since 1904-01-01), timestamp(3688342796.826832 s since 1904-01-01), timestamp(3688342798.0429673 s since 1904-01-01), timestamp(3688342799.0433993 s since 1904-01-01), timestamp(3688342800.043396 s since 1904-01-01), timestamp(3688342801.0437655 s since 1904-01-01), timestamp(3688342802.0438714 s since 1904-01-01), timestamp(3688342803.043973 s since 1904-01-01), timestamp(3688342804.043901 s since 1904-01-01), timestamp(3688342805.044822 s since 1904-01-01), timestamp(3688342806.0448112 s since 1904-01-01), timestamp(3688342807.045269 s since 1904-01-01), timestamp(3688342808.0455375 s since 1904-01-01), timestamp(3688342809.0448914 s since 1904-01-01)], "DataArray"=[56.5508, 56.5534, 56.5484, 56.5535, 56.5539, 56.5556, 56.5535, 56.5519, 56.5556, 56.5518, 56.5513, 56.5545, 56.5527, 56.5509, 56.551, 56.555, 56.5523, 56.5508, 56.555, 56.5524, 56.5578, 56.5524, 56.5521, 56.5548, 56.5559, 56.5567, 56.5536, 56.5561, 56.5574, 56.5541, 56.5521, 56.5572, 56.5611, 56.5581, 56.5601, 56.5592, 56.5525, 56.5569, 56.5582, 56.5588, 56.5563, 56.5565, 56.5578, 56.5575, 56.5582, 56.558, 56.5576, 56.5561]}, {"TimeArray"=[timestamp(3688342761.39444 s since 1904-01-01), timestamp(3688342762.463024 s since 1904-01-01), timestamp(3688342763.463638 s since 1904-01-01), timestamp(3688342764.463637 s since 1904-01-01), timestamp(3688342765.464684 s since 1904-01-01), timestamp(3688342766.465038 s since 1904-01-01), timestamp(3688342767.4661665 s since 1904-01-01), timestamp(3688342768.4671426 s since 1904-01-01), timestamp(3688342769.818876 s since 1904-01-01), timestamp(3688342770.819616 s since 1904-01-01), timestamp(3688342771.819715 s since 1904-01-01), timestamp(3688342772.8190737 s since 1904-01-01), timestamp(3688342773.819743 s since 1904-01-01), timestamp(3688342774.820112 s since 1904-01-01), timestamp(3688342775.820584 s since 1904-01-01), timestamp(3688342776.8214664 s since 1904-01-01), timestamp(3688342777.821848 s since 1904-01-01), timestamp(3688342778.822177 s since 1904-01-01), timestamp(3688342779.8225975 s since 1904-01-01), timestamp(3688342780.8223686 s since 1904-01-01), timestamp(3688342781.8226385 s since 1904-01-01), timestamp(3688342782.8219137 s since 1904-01-01), timestamp(3688342783.8218846 s since 1904-01-01), timestamp(3688342784.821887 s since 1904-01-01), timestamp(3688342785.821828 s since 1904-01-01), timestamp(3688342786.8223386 s since 1904-01-01), timestamp(3688342787.825325 s since 1904-01-01), timestamp(3688342788.8251424 s since 1904-01-01), timestamp(3688342789.825672 s since 1904-01-01), timestamp(3688342790.824856 s since 1904-01-01), timestamp(3688342791.8251505 s since 1904-01-01), timestamp(3688342792.8256593 s since 1904-01-01), timestamp(3688342793.8266897 s since 1904-01-01), timestamp(3688342794.826625 s since 1904-01-01), timestamp(3688342795.825836 s since 1904-01-01), timestamp(3688342796.826832 s since 1904-01-01), timestamp(3688342798.0429673 s since 1904-01-01), timestamp(3688342799.0433993 s since 1904-01-01), timestamp(3688342800.043396 s since 1904-01-01), timestamp(3688342801.0437655 s since 1904-01-01), timestamp(3688342802.0438714 s since 1904-01-01), timestamp(3688342803.043973 s since 1904-01-01), timestamp(3688342804.043901 s since 1904-01-01), timestamp(3688342805.044822 s since 1904-01-01), timestamp(3688342806.0448112 s since 1904-01-01), timestamp(3688342807.045269 s since 1904-01-01), timestamp(3688342808.0455375 s since 1904-01-01), timestamp(3688342809.0448914 s since 1904-01-01)], "DataArray"=[56.5706, 56.5722, 56.5706, 56.5727, 56.5774, 56.5704, 56.5731, 56.5714, 56.5706, 56.5769, 56.5717, 56.5756, 56.5772, 56.5747, 56.5741, 56.5748, 56.5721, 56.5725, 56.5736, 56.5717, 56.5786, 56.5708, 56.5728, 56.577, 56.5745, 56.5758, 56.5792, 56.5759, 56.5784, 56.578, 56.5784, 56.5781, 56.5786, 56.5742, 56.5801, 56.5787, 56.5764, 56.5767, 56.5788, 56.5791, 56.5763, 56.577, 56.577, 56.575, 56.5809, 56.5788, 56.5787, 56.5737]}, {"TimeArray"=[timestamp(3688342761.39444 s since 1904-01-01), timestamp(3688342762.463024 s since 1904-01-01), timestamp(3688342763.463638 s since 1904-01-01), timestamp(3688342764.463637 s since 1904-01-01), timestamp(3688342765.464684 s since 1904-01-01), timestamp(3688342766.465038 s since 1904-01-01), timestamp(3688342767.4661665 s since 1904-01-01), timestamp(3688342768.4671426 s since 1904-01-01), timestamp(3688342769.818876 s since 1904-01-01), timestamp(3688342770.819616 s since 1904-01-01), timestamp(3688342771.819715 s since 1904-01-01), timestamp(3688342772.8190737 s since 1904-01-01), timestamp(3688342773.819743 s since 1904-01-01), timestamp(3688342774.820112 s since 1904-01-01), timestamp(3688342775.820584 s since 1904-01-01), timestamp(3688342776.8214664 s since 1904-01-01), timestamp(3688342777.821848 s since 1904-01-01), timestamp(3688342778.822177 s since 1904-01-01), timestamp(3688342779.8225975 s since 1904-01-01), timestamp(3688342780.8223686 s since 1904-01-01), timestamp(3688342781.8226385 s since 1904-01-01), timestamp(3688342782.8219137 s since 1904-01-01), timestamp(3688342783.8218846 s since 1904-01-01), timestamp(3688342784.821887 s since 1904-01-01), timestamp(3688342785.821828 s since 1904-01-01), timestamp(3688342786.8223386 s since 1904-01-01), timestamp(3688342787.825325 s since 1904-01-01), timestamp(3688342788.8251424 s since 1904-01-01), timestamp(3688342789.825672 s since 1904-01-01), timestamp(3688342790.824856 s since 1904-01-01), timestamp(3688342791.8251505 s since 1904-01-01), timestamp(3688342792.8256593 s since 1904-01-01), timestamp(3688342793.8266897 s since 1904-01-01), timestamp(3688342794.826625 s since 1904-01-01), timestamp(3688342795.825836 s since 1904-01-01), timestamp(3688342796.826832 s since 1904-01-01), timestamp(3688342798.0429673 s since 1904-01-01), timestamp(3688342799.0433993 s since 1904-01-01), timestamp(3688342800.043396 s since 1904-01-01), timestamp(3688342801.0437655 s since 1904-01-01), timestamp(3688342802.0438714 s since 1904-01-01), timestamp(3688342803.043973 s since 1904-01-01), timestamp(3688342804.043901 s since 1904-01-01), timestamp(3688342805.044822 s since 1904-01-01), timestamp(3688342806.0448112 s since 1904-01-01), timestamp(3688342807.045269 s since 1904-01-01), timestamp(3688342808.0455375 s since 1904-01-01), timestamp(3688342809.0448914 s since 1904-01-01)], "DataArray"=[56.1058, 56.1076, 56.1051, 56.1064, 56.1119, 56.1056, 56.1088, 56.1054, 56.1116, 56.1108, 56.1137, 56.1122, 56.1139, 56.1102, 56.1116, 56.1079, 56.1119, 56.1093, 56.1118, 56.1133, 56.1112, 56.1124, 56.11, 56.1106, 56.1155, 56.1113, 56.1128, 56.1142, 56.1133, 56.1121, 56.1114, 56.1158, 56.1121, 56.1132, 56.1117, 56.1163, 56.1156, 56.1162, 56.1122, 56.1188, 56.114, 56.1116, 56.1168, 56.1173, 56.1145, 56.1132, 56.1115, 56.1152]}] caption="XY Graph"
  in  "log/linear 4":bool
  in  "log/linear 3":bool
  out "RUN Identifier 3":string="20201116_123919_RUNII" caption="RUN Identifier"
  in  "AutoFill Source (P)":T8(ring)=enum."USB6218AI"
  in  "AutoFill Source (L)":T8(ring)
  out "RUN Identifier 4":string="20201116_123919_RUNII" caption="RUN Identifier"
  out "Fill (false)":bool=TRUE
  in  "Fill state":bool
  out "state 1 (false)":bool=TRUE
  out "state 1":bool
  out "state 2":bool
  out "state 2 (false)":bool=TRUE
  out "Status V2 CTRL":enum16{"Pressurize", "Release"}(ring)
  out "Status V1 CTRL":enum16{"Pressurize", "Release"}(ring)
  out "Lav (%)":dbl=0.0976032670246936 format="%0.2f"
  out "Lstd":dbl=0.006099539014485866 format="%0.2f"
  out "Last N M.A. Levels":dbl[](array[numeric])=[0.09170812704799956, 0.09516065922615755, 0.09285897110351615, 0.09828437881161062, 0.09581828439634932, 0.09285897110092221, 0.09483184663640502, 0.08825559486583706, 0.09483184663881794, 0.1042030054093872, 0.105682662056137, 0.1083131627679897, 0.10584706835032069, 0.09779115993426052] format="%_5e"
  out "Lstd history":dbl(graph)=0.00731168899349361
  out "Lav history":dbl(graph)=0.09651113949810401
  out "Target Index (L)":i32=12
  in  "Auto Fll He L. label":string="L3"
  out "Target Index (P)":i32=7
  in  "Auto Fll Dewar P. label":string="P_Dewar"
  out "He Level":T9(graph)=[{"TimeArray"=[timestamp(3688342141.8225985 s since 1904-01-01), timestamp(3688342142.822563 s since 1904-01-01), timestamp(3688342143.822707 s since 1904-01-01), timestamp(3688342144.8219824 s since 1904-01-01), timestamp(3688342145.8260326 s since 1904-01-01), timestamp(3688342146.8264246 s since 1904-01-01), timestamp(3688342147.822299 s since 1904-01-01), timestamp(3688342148.8218455 s since 1904-01-01), timestamp(3688342149.8223214 s since 1904-01-01), timestamp(3688342150.8218794 s since 1904-01-01), timestamp(3688342151.822046 s since 1904-01-01), timestamp(3688342152.8222423 s since 1904-01-01), timestamp(3688342153.8230624 s since 1904-01-01), timestamp(3688342154.824749 s since 1904-01-01)], "Filtered X"=[0.10206572358848559, 0.09220134592084622, 0.08759796968468272, 0.11127247605242796, 0.09220134592744034, 0.08036409273913786, 0.09548947182661394, 0.08496746897015614, 0.11850635301936385, 0.1178487278214149, 0.10140809841361312, 0.09548947181756695, 0.1086419753486878, 0.0856250941571742]}, {"TimeArray"=[timestamp(3688342141.8225985 s since 1904-01-01), timestamp(3688342142.822563 s since 1904-01-01), timestamp(3688342143.822707 s since 1904-01-01), timestamp(3688342144.8219824 s since 1904-01-01), timestamp(3688342145.8260326 s since 1904-01-01), timestamp(3688342146.8264246 s since 1904-01-01), timestamp(3688342147.822299 s since 1904-01-01), timestamp(3688342148.8218455 s since 1904-01-01), timestamp(3688342149.8223214 s since 1904-01-01), timestamp(3688342150.8218794 s since 1904-01-01), timestamp(3688342151.822046 s since 1904-01-01), timestamp(3688342152.8222423 s since 1904-01-01), timestamp(3688342153.8230624 s since 1904-01-01), timestamp(3688342154.824749 s since 1904-01-01)], "Filtered X"=[0.09170812704799956, 0.09516065922615755, 0.09285897110351615, 0.09828437881161062, 0.09581828439634932, 0.09285897110092221, 0.09483184663640502, 0.08825559486583706, 0.09483184663881794, 0.1042030054093872, 0.105682662056137, 0.1083131627679897, 0.10584706835032069, 0.09779115993426052]}] caption="XY Graph"
  in  "P_safelimit_high (Pa)":dbl=300000.0 format="%_4e"
  in  "P_safelimit_low (Pa)":dbl=100.0 format="%_4e"
  in  "Auto Fill ON?":bool
  out "Pstd history":dbl(graph)=117.46659253087824
  out "Pav history":dbl(graph)=101915.24524654578
  in  "Mov. Avg Interval":i64=4
  in  "V2 (N.C.)":bool
  in  "V1 (N.O.)":bool=TRUE
  in  "N for sampling":i64=7
  in  "L_low (%)":dbl=60.0 format="%_3f"
  in  "L_high (%)":dbl=80.0 format="%_3g"
  in  "P_2_low (Pa)":dbl=125000.0 format="%_4e"
  in  "P_1_low (Pa)":dbl=135000.0 format="%_4g"
  in  "P_2_high (Pa)":dbl=135000.0 format="%_4e"
  in  "P_1_high (Pa)":dbl=140000.0 format="%_4e"
  out "Dewar Pressure":T9(graph)=[{"TimeArray"=[timestamp(3688342141.8225985 s since 1904-01-01), timestamp(3688342142.822563 s since 1904-01-01), timestamp(3688342143.822707 s since 1904-01-01), timestamp(3688342144.8219824 s since 1904-01-01), timestamp(3688342145.8260326 s since 1904-01-01), timestamp(3688342146.8264246 s since 1904-01-01), timestamp(3688342147.822299 s since 1904-01-01), timestamp(3688342148.8218455 s since 1904-01-01), timestamp(3688342149.8223214 s since 1904-01-01), timestamp(3688342150.8218794 s since 1904-01-01), timestamp(3688342151.822046 s since 1904-01-01), timestamp(3688342152.8222423 s since 1904-01-01), timestamp(3688342153.8230624 s since 1904-01-01), timestamp(3688342154.824749 s since 1904-01-01)], "Filtered X"=[101900.21492630574, 101972.54834933586, 102219.139569938, 102199.41227091734, 101610.88122677642, 102102.41972557292, 101841.033030673, 101926.5179875198, 101457.99466908885, 101859.11638932188, 102151.73796770729, 101357.71424114726, 101753.90413484225, 101319.90358778057]}, {"TimeArray"=[timestamp(3688342141.8225985 s since 1904-01-01), timestamp(3688342142.822563 s since 1904-01-01), timestamp(3688342143.822707 s since 1904-01-01), timestamp(3688342144.8219824 s since 1904-01-01), timestamp(3688342145.8260326 s since 1904-01-01), timestamp(3688342146.8264246 s since 1904-01-01), timestamp(3688342147.822299 s since 1904-01-01), timestamp(3688342148.8218455 s since 1904-01-01), timestamp(3688342149.8223214 s since 1904-01-01), timestamp(3688342150.8218794 s since 1904-01-01), timestamp(3688342151.822046 s since 1904-01-01), timestamp(3688342152.8222423 s since 1904-01-01), timestamp(3688342153.8230624 s since 1904-01-01), timestamp(3688342154.824749 s since 1904-01-01)], "Filtered X"=[101934.73769549772, 101923.64109101302, 102058.03330567844, 102072.82877912423, 102000.4953542419, 102032.96319830116, 101938.43656348491, 101870.21299263553, 101831.99135321364, 101771.16551915088, 101848.84175340945, 101706.64081681632, 101780.61818325467, 101645.81498286934]}] caption="XY Graph"
  out "Last N M.A. Pressures":dbl[](array[numeric])=[101934.73769549772, 101923.64109101302, 102058.03330567844, 102072.82877912423, 102000.4953542419, 102032.96319830116, 101938.43656348491, 101870.21299263553, 101831.99135321364, 101771.16551915088, 101848.84175340945, 101706.64081681632, 101780.61818325467, 101645.81498286934] format="%_5e"
  out "Pav (Pa)":dbl=101886.8872563351 format="%0.4e"
  out "Pstd":dbl=131.39381459485313 format="%0.4e"
  out "File Refn DewarCTRL":refnum<file>
  out "Error Out (Dewar CTRL":errorcluster
  in  "lower limit (mA) \n(PMC)":dbl=4.0 format="%_3f"
  in  "upper limit (mA)\n (PMC)":dbl=40.0 format="%_3f"
  in  "OUTPUT\n(PMC)":bool
  in  "Set Current (mA)\n (PMC)":dbl=4.0 min=4.0 max=40.0 format="%_3g"
  in  "update values":bool
  out "Monitor Current (mA)":dbl=-0.3751088182058693 min=0.0 max=1.9 format="%_4e"
  in  "update current":bool
  out "USB 6218 AOUT":dbl[](array[numeric])=[0.004, 0.004, 0.06969546425555169, 0.06969546425555169]
  out "Graph 7":T10(graph)=[{"TimeArray (USB6218)"=[timestamp(3688342774.983717 s since 1904-01-01)], "DataArrayConv (USB6218)"=[]}, {"TimeArray (USB6218)"=[], "DataArrayConv (USB6218)"=[]}] caption="XY Graph"
  in  "lower limit (mA) \n(PWR)":dbl=4.0 format="%_3f"
  in  "upper limit (mA)\n (PWR)":dbl=20.0 format="%_3f"
  in  "lower limit (mA)":dbl=4.0 format="%_3f"
  in  "SetCurrent 2 (mA)":dbl=4.0 min=4.0 max=500.0 format="%_3f"
  in  "upper limit (mA)":dbl=500.0 format="%_3f"
  out "error out (KIKUSI CTRL)":errorcluster
  out "ActualVoltage (V)":dbl[](array[numeric]) format="%_6g"
  out "ActualCurrent (A)":dbl[](array[numeric])=[0.004, 0.004] format="%_3e"
  in  "SetCurrent 1 (mA)":dbl=4.0 min=4.0 max=500.0 format="%_3g"
  in  "Output\n (ADCMT)":bool[](array[boolean])=[FALSE, FALSE]
  out "error out (ADCMT6420A)":errorcluster
  in  "Voltage limits (V)":dbl[](array[numeric])=[12.0, 12.0] format="%_3f"
  in  "CtrlLabels":string[](array[string])=["CV2", "CV3"]
  in  "VISA":refnum<visa-resource-name>[](array[refnum])=["GPIB0::1::INSTR", "GPIB0::12::INSTR"]
  out "Initialized?":bool
  in  "InstName":string="ADCMT6240"
  out "Graph 6":T9(graph)=[{"TimeArray"=[timestamp(3688340149.108854 s since 1904-01-01), timestamp(3688340157.5607233 s since 1904-01-01), timestamp(3688340164.198473 s since 1904-01-01)], "Filtered X"=[0.004, 0.004, 0.004]}, {"TimeArray"=[timestamp(3688340149.108854 s since 1904-01-01), timestamp(3688340157.5607233 s since 1904-01-01), timestamp(3688340164.198473 s since 1904-01-01)], "Filtered X"=[0.004, 0.008, 0.004]}, {"TimeArray"=[timestamp(3688340149.108854 s since 1904-01-01), timestamp(3688340157.5607233 s since 1904-01-01), timestamp(3688340164.198473 s since 1904-01-01)], "Filtered X"=[0.004, 0.004, 0.004]}, {"TimeArray"=[timestamp(3688340149.108854 s since 1904-01-01), timestamp(3688340157.5607233 s since 1904-01-01), timestamp(3688340164.198473 s since 1904-01-01)], "Filtered X"=[0.004, 0.008, 0.004]}] caption="XY Graph"
  in  "Initialize":bool
  in  "CONTROL KIKUSUI?":bool=TRUE
  in  "OUTPUT\n(PWR)":bool
  in  "Set Current (mA)\n (PWR)":dbl=4.0 min=4.0 max=20.0 format="%_3g"
  out "RUN Identifier 5":string="20201116_123919_RUNII" caption="RUN Identifier"
  out "Graph DMMs 3":T4(graph) caption="XY Graph"
  out "Power":dbl
  in  "index I":i64
  in  "index V":i64
  out "VariableSources":T11(array[ring])
  in  "DMMsConfig (variables)":T12(array[cluster])=[{"Label"="V_H1", "Active?"=TRUE, "Source"=enum."USB6210", "SourceLabel"="V_H1", "FileFormat"="%4.4e"}, {"Label"="I_H1", "Active?"=TRUE, "Source"=enum."USB6218AO", "SourceLabel"="I_H1", "FileFormat"="%4.6e"}]
  in  "Measure DMMs?":bool
  out "DMMsLabels":string[](array[string])=["V_H2", "V_H4", "I_H2", "I_H4"]
  out "Active?":bool[](array[boolean])=[TRUE, FALSE, TRUE, FALSE]
  out "DMM LastMeasurements":dbl[](array[numeric])=[2.6334599999999997e-05, 0.0, 0.0, 0.0]
  out "Graph DMMs 2":T4(graph) caption="XY Graph"
  out "DMMFileName":string="20201001_162428_PreCooling_DMMs_20201001_162516.csv"
  out "error out (DMMs)":errorcluster
  out "cycle # (DMMs)":i32=100
  in  "DMMsConfig":T13(array[cluster])=[{"Label"="V_H2", "Active?"=TRUE, "VISA resource name"="GPIB0::22::INSTR", "Device"=enum."Agilent34401A", "Measurement"=enum."DC Volts", "FileFormat"="%4.6e"}, {"Label"="V_H4", "Active?"=FALSE, "VISA resource name"="USB0::0x1334::0x0204::262800451::INSTR", "Device"=enum."ADCMT7351", "Measurement"=enum."DC Volts", "FileFormat"="%4.6e"}, {"Label"="I_H2", "Active?"=TRUE, "VISA resource name"="USB0::0x1334::0x0204::262800066::INSTR", "Device"=enum."ADCMT7351", "Measurement"=enum."DC Currents", "FileFormat"="%4.4e"}, {"Label"="I_H4", "Active?"=FALSE, "VISA resource name"="GPIB0::23::INSTR", "Device"=enum."HP3478A", "Measurement"=enum."DC Currents", "FileFormat"="%4.4e"}]
  in  "Measurement Interval DMMs (ms)":i64=500
  in  "InstName DMMs":string="DMMs"
  in  "Initialize (DMMs)":bool
  out "Graph DMMs 1":T4(graph) caption="XY Graph"
  out "error out (DMM graphs)":errorcluster
  in  "Sample #":i32=5
  out "P_HEX7OUT":dbl=101266.48603690336 format="%_4e"
  out "P (HEX7 out)":dbl=101266.48603690336 format="%_4e"
  out "DP HEX5":dbl=24.853263706915428 format="%_4e"
  out "DP_HEX5":dbl=24.853263706915428 format="%_4e"
  in  "Diff pressure HEX5":string="DP_HEX5"
  out "3He pot level":dbl=100.03348435966727 format="%_4f"
  in  "3He pot":string="L1"
  out "He level (3He)":dbl(slide)=100.03348435966727 scale=0.0..100.0
  out "He level (1K) b":dbl(slide)=0.09811997252509147 scale=0.0..100.0
  out "He level (1K)":dbl(slide)=0.07904884235852952 scale=0.0..100.0
  out "He level (4K)":dbl(slide)=0.11324535160603699 scale=0.0..100.0
  out "1K pot(b1)":dbl=0.09811997252509147 format="%_4f"
  in  "1K pot (b)":string="L2-2"
  in  "1K pot level":string="L2-1"
  out "L(1K) (a1)":dbl=0.07904884235852952 format="%_4f"
  in  "SensorLocation 2":T14(ring)=enum."T3He5"
  out "Temperature 2":dbl=63.4594
  out "DP HEX4":dbl=-13.071876252658488 format="%_4e"
  in  "Diff pressure HEX4":string="DP_HEX4"
  out "V2":bool
  out "V1":bool=TRUE
  out "F5 (3He pump ex.)":dbl=25.54341705535066 format="%_4f"
  out "F4 (3He in to HEX7)":dbl=-8.496093212698424 format="%_3f"
  out "F3 (4He rtn flw via HEX7)":dbl=0.16300396733772582 format="%_4f"
  out "F1 (1K pump exhaust) flow":dbl=1.5418315461474963 format="%_4f"
  out "P (Dewar)":dbl=102163.24555458283 format="%_4e"
  out "P (1K pot)":dbl=101777.9677527887 format="%_4e"
  out "P (3He pot)":dbl=101725.36175301031 format="%_4e"
  out "P (shield return)":dbl=101386.52915740103 format="%_4e"
  out "P (3He IN)":dbl=101356.92948144057 format="%_4e"
  out "P (4K reservoir)":dbl=102072.25500773212 format="%_4e"
  out "P (insulation)":dbl=0.001694910685758757 format="%_4e"
  in  "3He pump exhaust flow":string="F_5"
  out "F_5":dbl=25.54341705535066 format="%_4f"
  in  "3He incoming flow into HEX7":string="F_4"
  out "F_4":dbl=-8.496093212698424 format="%_4f"
  out "F_3":dbl=0.16300396733772582 format="%_4f"
  in  "4He return flow from HEX7":string="F_3"
  out "F_2":dbl=0.06042183752267505 format="%_4f"
  in  "Shield flow":string="F_2"
  out "P_SldRTN":dbl=101386.52915740103 format="%_4e"
  in  "3He pot pressure":string="P_3Hepot"
  out "P_3Hepot":dbl=101725.36175301031 format="%_4e"
  in  "Shield return press.":string="P_SldRTN"
  out "F_1":dbl=1.5418315461474963 format="%_4f"
  in  "1K pump exhaust flow":string="F_1"
  out "P_Dewar":dbl=102163.24555458283 format="%_4e"
  in  "Dewar pressure":string="P_Dewar"
  out "P_1Kpot":dbl=101777.9677527887 format="%_4e"
  in  "1Kpot pressure":string="P_1Kpot"
  out "P_3HeIN":dbl=101356.92948144057 format="%_4e"
  in  "3He inlet pressure":string="P_3HeIN"
  in  "4K reservoir pressure":string="P_4Kres"
  out "P_4Kres":dbl=102072.25500773212 format="%_4e"
  out "P_ins":dbl=0.001694910685758757 format="%_4e"
  in  "Insulation vacuum":string="P_ins"
  out "T3He7-1/6-2 (3He pot) 2":dbl=56.1115 format="%_4f"
  out "T3He7-1/7-2 (HEX1)":dbl=56.5787 format="%_4f"
  out "T3He6-1/6-2 (3He pot) 2":dbl=56.5576 format="%_4f"
  out "T3He6-1/6-2 (HEX1)":dbl=56.5713 format="%_4f"
  out "T1K3-1/3-2 (1K pot) 2":dbl=44.0491 format="%_4f"
  out "T1K3-1/3-2 (1K pot)":dbl=44.0707 format="%_4f"
  out "T4He1 (4K reservoir )":dbl=59.351 format="%_4f"
  out "Temperature 1":dbl=90.409
  in  "SensorLocation 1":T14(ring)=enum."TTH2"
  out "TIP7":dbl format="%_4g"
  out "T3He6-2":dbl=56.5576 format="%_4g"
  out "T3He7-2":dbl=56.1115 format="%_4g"
  out "T3He6-1":dbl=56.5713 format="%_4g"
  out "T3He4":dbl=56.764 format="%_4g"
  out "T3He7-1":dbl=56.5787 format="%_4g"
  out "T3He8":dbl=53.3341 format="%_4g"
  out "T3He5":dbl=63.4594 format="%_4g"
  out "T1K3-2":dbl=44.0491 format="%_4g"
  out "T1K3-1":dbl=44.0707 format="%_4g"
  out "TIP6":dbl=63.802 format="%_4g"
  out "T3He9":dbl=67.587 format="%_4g"
  out "T1K5":dbl=66.761 format="%_4g"
  out "T1K4":dbl=49.115 format="%_4g"
  out "T1K2":dbl=59.261 format="%_4g"
  out "TIP5":dbl=64.662 format="%_4g"
  out "TIP4":dbl=64.912 format="%_4g"
  out "TIP3":dbl=128.87 format="%_4g"
  out "TIP2":dbl=182.56 format="%_4g"
  out "TIP1":dbl=265.54 format="%_4g"
  out "T1K6":dbl=277.86 format="%_4g"
  out "T4He10":dbl=250.02 format="%_4g"
  out "T4He8":dbl=254.76 format="%_4g"
  out "T4He7":dbl=211.21 format="%_4g"
  out "T3He1-3":dbl=286.77 format="%_4g"
  out "T3He1-2":dbl=287.33 format="%_4g"
  out "T4He9":dbl=186.15 format="%_4g"
  out "T4He6":dbl=115.87 format="%_4g"
  out "T4He5":dbl=109.94 format="%_4g"
  out "T4He4":dbl=122.8 format="%_4g"
  out "T4He2-2":dbl=152.68 format="%_4g"
  out "T4He2-1":dbl=148.01 format="%_4g"
  out "T4He3-4":dbl=289.16 format="%_4g"
  out "T4He3-3":dbl=289.09 format="%_4g"
  out "T4He3-2":dbl=290.01 format="%_4g"
  out "T4He3-1":dbl=289.88 format="%_4g"
  out "T3He1-4":dbl=286.32 format="%_4g"
  out "T3He3":dbl=73.062 format="%_4g"
  out "T3He2-2":dbl=148.1 format="%_4g"
  out "T3He2-1":dbl=149.39 format="%_4g"
  out "T1K1":dbl=73.73 format="%_4g"
  out "T4He1":dbl=59.351 format="%_4g"
  out "TTH1":dbl=93.008 format="%_4g"
  out "TTH2":dbl=90.409 format="%_4g"
  out "TTH4":dbl=197.32 format="%_4g"
  out "TTH3":dbl=205.57 format="%_4g"
  out "T3He1-1":dbl=287.22 format="%_4g"
  out "T3He10":dbl=278.8 format="%_4g"
  out "F2 (shield flow)":dbl=0.06042183752267505 format="%_4f"
  out "DP_HEX4":dbl=-13.071876252658488 format="%_4e"
  in  "4K reservoir level":string="L3"
  out "L3":dbl=0.11324535160603699 format="%_4f"
  out "RUN Identifier 6":string="20201116_123919_RUNII" caption="RUN Identifier"
  in  "HEX7 out pressure":string="P_HEX7OUT"
  out "Series 1":string[](array[string])=["P_ins", "P_4Kres", "P_3HeIN", "P_SldRTN", "P_3Hepot", "P_1Kpot", "P_Dewar(old)", "P_HEX7OUT", "P_IP"]
  out "Series 2":string[](array[string])=["DP_HEX4", "DP_HEX5", "L1", "L2-1", "L2-2", "L3"]
  out "Series 3":string[](array[string])=["F_1", "F_2", "F_3", "F_4", "F_5", "I_CV", "P_Dewat"]
  out "Series 4":string[](array[string])=["TTH3", "TTH4", "TTH1", "TTH2", "T4He1", "T1K1", "T3He2-1", "T3He2-2", "T4He3-1", "T4He3-2", "T4He3-3", "T4He3-4", "T4He2-1", "T4He2-2", "T4He4", "T1K2", "T1K4", "T1K5", "T1K3-1", "T1K3-2", "T3He5", "T3He8", "T3He6-1", "T3He6-2", "T3He7-1", "T3He7-2"]
  out "Plot errors":errorcluster
  out "LastMeasurementConfig (218)":T15(array[cluster])=[{"LSIName"="LSI218A", "Active?"=TRUE, "LastData"=[278.76, 287.23, 205.57, 197.31, 93.015, 90.402, 59.35, 73.73], "Labels"=["T3He10", "T3He1-1", "TTH3", "TTH4", "TTH1", "TTH2", "T4He1", "T1K1"]}, {"LSIName"="LSI218B", "Active?"=TRUE, "LastData"=[30.0, 0.0, 0.0, 0.0, 149.39, 148.1, 73.063, 286.33], "Labels"=["N.C.", "N.C.", "N.C.", "N.C.", "T3He2-1", "T3He2-2", "T3He3", "T3He1-4"]}, {"LSIName"="LSI218C", "Active?"=TRUE, "LastData"=[289.87, 290.01, 289.1, 289.16, 148.02, 152.67, 122.79, 109.94], "Labels"=["T4He3-1", "T4He3-2", "T4He3-3", "T4He3-4", "T4He2-1", "T4He2-2", "T4He4", "T4He5"]}, {"LSIName"="LSI218D", "Active?"=TRUE, "LastData"=[115.85, 186.16, 287.33, 286.78, 211.21, 254.77, 250.0, 277.86], "Labels"=["T4He6", "T4He9", "T3He1-2", "T3He1-3", "T4He7", "T4He8", "T4He10", "T1K6"]}, {"LSIName"="LSI218E", "Active?"=TRUE, "LastData"=[265.54, 0.0, 182.55, 688.49, 128.86, 64.91, 64.659, 688.58], "Labels"=["TIP1", "N.C.", "TIP2", "N.C.", "TIP3", "TIP4", "TIP5", "N.C."]}, {"LSIName"="LSI218F", "Active?"=TRUE, "LastData"=[59.451, 48.966, 66.774, 56.763, 67.829, 63.827, 0.433, 0.0], "Labels"=["T1K2", "T1K4", "T1K5", "T3He4", "T3He9", "TIP6", "N.C.", "N.C."]}]
  out "DataArrayConv (USB6210)":dbl[][](array[numeric])=[[0.0016985076469113389, 101832.16872606815, 101220.44208291276, 101291.15241755564, 101690.29108855205, 101713.08702033253, 0.0, -14.58472805516084, -3.7593731160273647, 100.02033130195804, 0.09680472216883765, 0.0928589711067572, 0.09285897110562968, 101445.72850084068, 0.00015794392082601466, 5.8750634943484386], [0.0016856962957262024, 101865.05725721586, 101199.06455156975, 101499.99457770793, 101706.07288687328, 101745.52738662114, 0.0, -11.665910666875446, 16.466800869346933, 100.01901599603929, 0.0856250941222492, 0.110614850901225, 0.08694034451505128, 101493.4168698453, 0.00014527857457659758, 5.53888075049061], [0.001682126465642948, 101930.83432063498, 101513.14998300378, 101284.57471698422, 101675.38605520307, 101709.57995401025, 0.0, -11.05748111470345, -17.079048716840404, 100.01638538424609, 0.10272334875069622, 0.11784872782819483, 0.0882555948658934, 101467.10605043583, 0.0001612303236722782, 5.520138211099], [0.001715567839314439, 102022.92221153466, 101241.81962803326, 101526.30539526748, 101749.03445268972, 101737.63648680823, 0.0, -12.035901604533272, -1.621647579482799, 100.03743027703277, 0.0823369682619271, 0.11061485089033349, 0.10140809841931961, 101475.32818254823, 0.00013225994060034175, 5.508695399166593], [0.0016892737021061356, 101886.43480239325, 101463.81719402097, 101231.95306928418, 101701.68905404501, 101773.58391905762, 0.0, -11.115035260684719, 25.346585889716167, 100.01572773170821, 0.11982160335626449, 0.10666909982112965, 0.0882555948622622, 101401.3289997052, 0.00014558688545089616, 5.514942911015214], [0.0016856962957120887, 101893.01250845697, 101481.90587993711, 101401.32898870594, 101739.39002005248, 101769.20008681675, 0.0, -9.93106421754808, 24.853263053700168, 100.0157277313541, 0.1231097292068519, 0.09088609557892624, 0.08957084522668168, 101401.32899644942, 0.00014624975809092566, 5.5091557421963575], [0.001702112241654899, 101917.67890710325, 101340.4852112232, 101355.28504938849, 101753.41828612429, 101756.04858572363, 0.0, -11.411027997547091, -2.1149691056238096, 100.02559252494399, 0.11061485087663162, 0.09614709700198834, 0.10206572358988894, 101603.59344600132, 0.00014745054197010484, 5.512772722471448], [0.0017052079822400363, 102090.34370130418, 101508.21670489587, 101585.50475168884, 101697.30522150912, 101706.94965350973, 0.0, -12.6689972146794, -34.18085471315613, 100.04203384733069, 0.07378784094485494, 0.09220134593649923, 0.10338097395305981, 101195.77569372964, 0.00016270186273131826, 5.504420786466018], [0.0016933714637543337, 101930.83432102836, 101490.12801634865, 101388.17357644875, 101732.37588687218, 101773.58391935991, 0.0, -13.022544125408208, 6.1070527372864, 100.01638538431729, 0.09483184662552932, 0.10666909983274891, 0.08891322004558086, 101572.34933848385, 0.00015083803725969138, 5.509155741782502], [0.0017072749367236463, 101925.90103834363, 101248.39733731847, 101391.46242696735, 101737.63648599591, 101720.97792017243, 0.0, -12.019457533253814, 71.55435072561778, 100.03151140103552, 0.09614709695613116, 0.08825559486610221, 0.11456060195989323, 101430.92866380943, 0.000153000418941653, 5.507511660144301], [0.0016826359779464751, 101820.6577388149, 101335.55193726094, 101504.92785874543, 101693.79815439775, 101706.94965427966, 0.0, -10.86015261028711, 33.07528543448734, 100.01375477272042, 0.0856250941451212, 0.11127247607640156, 0.0889132200492053, 101485.19473516897, 0.00016142575747488726, 5.509813375025615], [0.0016872285413077606, 101919.32333270369, 101240.17520126232, 101241.81963982515, 101743.77385267452, 101733.25265412086, 0.0, -11.56724640891954, 35.377451936993154, 100.0367726240272, 0.09154372074948794, 0.08365221862333744, 0.10469622429598657, 101715.41444699641, 0.00014361624215080963, 5.52000668384524], [0.0016821264654510507, 101893.01250808984, 101286.21914874509, 101294.44127166664, 101720.97791972595, 101763.06271961458, 0.0, -11.337029835953722, 3.4760067505701375, 100.03085374795297, 0.09351659626786335, 0.08430984379709675, 0.0954894718143463, 101230.30864340856, 0.00014825653834920106, 5.524675877489673], [0.0016780559153745326, 101911.10120015097, 101169.46487132157, 101383.24029797112, 101739.3900203105, 101814.79195255824, 0.0, -12.183897976992764, 21.235573406630515, 100.03479966541471, 0.08825559483278658, 0.08233696827611237, 0.09548947182601278, 101506.57229160522, 0.0001447954042376404, 5.524675877155692], [0.0016765319999805606, 101958.78957279451, 101356.92948141521, 101342.1296400169, 101716.59408645888, 101707.82642020396, 0.0, -10.90948473209355, -4.252694378406585, 100.03479966540314, 0.08628271927790962, 0.10798435018011024, 0.11982160335837219, 101273.06373993873, 0.00015885537746714444, 5.518296838785524], [0.0016790726286288712, 101945.63415735995, 101490.12802344664, 101347.06292102697, 101754.29505288789, 101784.10511980281, 0.0, -12.915657844999012, -12.803597630295371, 100.00980885549924, 0.08233696823210371, 0.08628271933183773, 0.10075047323232106, 101325.68539825853, 0.0001444887692259696, 5.506130631390961], [0.0016897853794054498, 101975.23383811218, 101320.75209365552, 101164.53158856047, 101722.73145375543, 101777.0909881104, 0.0, -11.961903396566553, 95.06933587075883, 100.02559252485926, 0.10535384948209497, 0.10009284806124849, 0.09220134593509657, 101550.97180146168, 0.0001483912978320738, 5.5221768722714515], [0.0016811079031505553, 101929.18989874606, 101351.99619589996, 101488.48359058959, 101703.44258741802, 101734.12942049542, 0.0, -14.453175739544522, -2.114969105721509, 100.03282670696193, 0.08036409273191733, 0.1014080984088988, 0.09877759770890365, 101394.75128129986, 0.00015406987566298966, 5.5070513167877975], [0.0016760243357404382, 101787.76920710821, 101036.26634084422, 101437.5063683032, 101696.42845503839, 101721.85468829313, 0.0, -12.175675957747822, 73.52763482644909, 100.0354573184203, 0.08562509416150313, 0.1369198579456621, 0.09154372074318548, 101547.68293945766, 0.00015318587672950214, 5.527240645311515], [0.001691833639435517, 101911.10120028359, 101345.41848871365, 101294.44127569096, 101717.47085415754, 101765.6930191484, 0.0, -11.024593017420786, 45.40831880739504, 100.02690783064907, 0.09943522288286516, 0.09417422145990806, 0.09943522286249523, 101677.59263162475, 0.00015047302647334682, 5.538223114773727], [0.0016938843822185505, 101893.01250978821, 101351.9961964771, 101261.55274654811, 101697.30522122844, 101707.82642028482, 0.0, -12.134565860956126, -40.594030132280466, 100.04269150040554, 0.10009284806285693, 0.09548947181950596, 0.10009284806184715, 101598.66016783372, 0.00015102087320363603, 5.517441916165722], [0.0017093443965102329, 101934.12317371284, 101264.84160035982, 101279.64143503254, 101685.90725504457, 101744.65061930713, 0.0, -14.634060181933917, 64.48341078485909, 100.01901599615667, 0.07970646756035346, 0.10403859913064109, 0.09483184663978972, 101601.94901782386, 0.00015263017661396096, 5.522834505722459], [0.0017129719893116283, 101873.2793909497, 101332.26307903595, 101430.92866322373, 101710.45672222658, 101763.06272007298, 0.0, -11.871461182531961, 11.862468345331667, 100.04795272384771, 0.1066690997654503, 0.10272334877207187, 0.08167934308211428, 101667.72607876257, 0.00015239923156078213, 5.533751211238024], [0.0017129719890873456, 101835.45757890653, 101389.81800331481, 101332.26308075344, 101704.31935497867, 101747.28092162542, 0.0, -11.427472064826361, 49.51933207329118, 100.01901599594885, 0.09746234734177431, 0.10469622429029102, 0.08628271933586429, 101427.63982190206, 0.00014970031234038994, 5.507643186381635], [0.0016938843822442617, 101912.74562778191, 101445.72850297844, 101411.19554633378, 101701.68905363319, 101754.29505260289, 0.0, -12.825215618469166, -15.105763950596373, 100.01638538480807, 0.1336317319665327, 0.10469622430661588, 0.09943522287654274, 101404.61784928897, 0.00015514680781186815, 5.519743630885226], [0.0016959376109104611, 101993.32253005449, 101478.61702956482, 101524.66097025927, 101707.82642008652, 101720.97792120202, 0.0, -12.077011703639117, 5.942612372294986, 100.03019609549787, 0.08628271933695833, 0.08628271933354992, 0.109957225693192, 101435.86194323712, 0.00015775270241722642, 5.5165869931993985], [0.0016785641952298419, 101904.52349626606, 101273.0637300145, 101291.1524215649, 101717.47085340918, 101717.47085454458, 0.0, -11.896127252572164, 48.20380658039136, 100.03874558303818, 0.08759796967635775, 0.10666909983584733, 0.10666909983775433, 101472.03932931261, 0.00015718043610256062, 5.526122670023445], [0.0017160874811014547, 101916.03448062438, 101495.06129681651, 101412.83997287438, 101688.5375550485, 101753.4182864131, 0.0, -10.728600276382366, 52.150377482029775, 100.02953844234602, 0.11258772641687786, 0.11916397818045257, 0.09088609557339636, 101513.14999647114, 0.0001610839043479135, 5.520203973995838], [0.0017021122417920991, 101930.8343234091, 101328.97422691758, 101286.21914323398, 101753.4182860876, 101756.92535364449, 0.0, -11.72346482206929, -8.19926519956493, 100.00586293801635, 0.10140809840991075, 0.08496746896842622, 0.08825559486026241, 101463.81719326794, 0.00013992401920005955, 5.498502090882933], [0.0017072749366225796, 101950.56744309909, 101363.50717862732, 101555.90507255693, 101699.05875491144, 101742.02032019466, 0.0, -14.27229128211488, -4.91045665409362, 100.01835834285669, 0.08628271925850953, 0.11982160335618988, 0.0981199725277064, 101435.86195303871, 0.0001550998287190593, 5.508826925726199], [0.0016892737021326888, 101833.81315271331, 101166.17602163501, 101358.57390073559, 101680.64665537974, 101687.66078754594, 0.0, -13.663861749815403, 22.386656386026438, 100.03085374811465, 0.10864197531300018, 0.10075047322387898, 0.09351659627431821, 101480.2614619057, 0.00016816241133741627, 5.513233065581237], [0.0016918336397340093, 101981.81154448308, 101279.64143487849, 101368.44045797281, 101713.08702017475, 101706.07288789151, 0.0, -12.553888925297462, 55.110306476439106, 100.03808792994593, 0.08562509414773817, 0.09680472217446534, 0.10995722571543565, 101399.68456194161, 0.00015369704584851536, 5.507972003209853], [0.0016933714635912413, 101891.36808722572, 101210.57553413912, 101192.48683711959, 101727.11528707815, 101737.6364877865, 0.0, -11.961903410629526, -21.683380136412467, 100.01178181389622, 0.10075047323552361, 0.10075047322328137, 0.10009284806435811, 101605.2378738045, 0.00015661024640693013, 5.511391693779112], [0.001678564194927532, 101957.14514474105, 101274.70816508321, 101281.28586588813, 101705.19612072366, 101731.49912168967, 0.0, -10.720378254392315, 19.262288053315537, 100.01441242558933, 0.08233696821786596, 0.10929960053125665, 0.09877759770698699, 101467.10605565517, 0.0001551468076217685, 5.513430355222738], [0.001717647351208853, 102044.2997573318, 101365.15161434854, 101457.23948682897, 101756.92535255839, 101740.26678735143, 0.0, -13.12120837957803, 14.00019391494145, 100.0262501777436, 0.12376735434914118, 0.08825559486315551, 0.0968047221647878, 101394.75128367601, 0.0001533251178390125, 5.506196394837313], [0.0016985076469424835, 101948.92301428551, 101356.92947504071, 101399.68455922755, 101705.19612113175, 101770.07685262537, 0.0, -11.961903433253346, -13.296918621765741, 100.02164660751687, 0.0961470969909575, 0.11193010123896543, 0.08167934309300484, 101350.35177321837, 0.00015074670138303243, 5.509353031851748], [0.001697993328234986, 101907.81234645745, 101422.70654141511, 101325.68537368043, 101735.88295381088, 101733.25265347392, 0.0, -12.01945757468495, -36.48302079347576, 100.03282670700432, 0.094174221460295, 0.09548947182109846, 0.09746234734269646, 101593.72689368669, 0.00015083803621330125, 5.511062877969592], [0.001678564194898545, 101993.32253287372, 101406.26226875046, 101376.66259333238, 101695.55168733191, 101722.73145330299, 0.0, -13.236316654715807, -21.190060255552588, 100.0380879299652, 0.09417422145992005, 0.08957084522064646, 0.10995722571854372, 101728.56986132935, 0.0001478082195316557, 5.518888707924622], [0.0016918336395347422, 101868.34611126423, 101207.2866806673, 101246.75290715377, 101716.59408829284, 101719.22438845664, 0.0, -11.698798761406643, 86.6828718697632, 100.04269150063466, 0.0948318466200812, 0.10272334876996597, 0.09943522287635259, 101552.616232476, 0.00015379016984874418, 5.5221768725965195], [0.0016949106856096797, 101939.05645180488, 101467.10604803392, 101345.41848776913, 101769.20008581369, 101777.96775212817, 0.0, -10.547715817769282, -2.279409637019336, 100.03348435976736, 0.12574022994657183, 0.06984208989584345, 0.10403859911541599, 101532.88310808288, 0.00013707190891229566, 5.506130631105108], [0.0016816171071247375, 102022.92220923673, 101179.33142810284, 101210.57552840498, 101698.1819880936, 101749.03445332125, 0.0, -13.762525973974732, -21.847821824532154, 100.0420338474096, 0.09483184660307273, 0.08891322005171653, 0.10535384947677798, 101541.10523583164, 0.0001470046627129244, 5.530660336088755], [0.0016877395991853987, 102031.14434168766, 101250.04176417911, 101284.57471573919, 101747.28092016382, 101742.89708621129, 0.0, -13.524087373262356, 74.84315986737933, 100.04597976485402, 0.08891322003955524, 0.09811997252651306, 0.10403859912523186, 101274.70815979305, 0.00015276891279361772, 5.52053279015318], [0.0016867176382062941, 101929.18989208799, 101281.28585936227, 101601.94901872858, 101728.8688195061, 101774.46068564971, 0.0, -11.35347387159888, 32.910845104363595, 100.03611497118908, 0.07313021578192988, 0.10338097394513843, 0.11982160336152853, 101180.97587496797, 0.00014514664144137354, 5.508169292924249], [0.0017077920665341275, 101962.07842325009, 101361.86275192664, 101427.63981002072, 101726.2385198258, 101760.43242115337, 0.0, -11.378139941417592, 68.42998149528823, 100.03348435956718, 0.08167934302691235, 0.10535384948089216, 0.10732672501153062, 101504.9278637119, 0.00014669334861615104, 5.520138210168808], [0.001709344396578268, 101833.81315122647, 101404.6178377322, 101253.33061046888, 101671.87898830316, 101678.89312250512, 0.0, -11.27125364694509, -15.599085085889474, 100.11832159997704, 0.1007504732268858, 0.12968598099932982, 0.10009284805986082, 101710.48117470111, 0.00015775270273420098, 5.52184805558587], [0.0017166072803434422, 101971.94498410224, 101240.17521622375, 101187.55356507898, 101719.22438681862, 101748.15768582988, 0.0, -10.21061294287512, 39.4884632112269, 100.02559252476306, 0.1073267250044955, 0.0928589711172974, 0.10929960054586751, 101698.97019386955, 0.00014453253399511162, 5.517507679127268], [0.001694910685758757, 102072.25500773212, 101356.92948144057, 101386.52915740103, 101725.36175301031, 101777.9677527887, 0.0, -13.071876252658488, 24.853263706915428, 100.03348435966727, 0.07904884235852952, 0.09811997252509147, 0.11324535160603699, 101266.48603690336, 0.00014673778134435226, 5.515600544379195], [0.001713490844762899, 102021.27778594472, 101355.28505120106, 101348.70734634637, 101748.15768651912, 101758.67888665742, 0.0, -12.307228287251254, -3.5949330203699503, 100.19921295176155, 0.09220134592968446, 0.08102171791361665, 0.09614709699847113, 101325.68537503395, 0.00015001800729686586, 5.514153752001237]]
  out "LastMeasurementConfig (336)":T15(array[cluster])=[{"LSIName"="LSi336X", "Active?"=TRUE, "LastData"=[44.0737, 44.0488, 63.4557, 53.3294], "Labels"=["T1K3-1", "T1K3-2", "T3He5", "T3He8"]}, {"LSIName"="LSi336Y", "Active?"=TRUE, "LastData"=[56.5704, 56.5561, 56.5737, 56.1152], "Labels"=["T3He6-1", "T3He6-2", "T3He7-1", "T3He7-2"]}]
  out "DataArrayConv (USB6218)":dbl[][](array[numeric])=[[1.6108772064644081, 0.11960383538282587, 0.19719801289443417, -8.8117305470801, 25.42834097532839, -0.005193268383660984, -25.030460042043373, 101763.76778005705], [1.4727858772132323, 0.12354930467748859, 0.3234529413982592, -8.611169313327453, 24.86611211032151, -0.004930182610743403, -24.949906766882535, 101441.5552574628], [1.1538606722402807, 0.16957974721691593, 0.41025320470314475, -8.785427429519835, 25.507250294604013, -0.007561039877274372, -24.962236349926822, 101712.80559595322], [1.28208833184731, 0.3168771630474284, 0.35501667385679236, -9.633702805164498, 25.129143157252333, -0.007824125581124733, -24.987717487896862, 101605.94940418932], [1.7785595282840228, 0.10513712477879456, 0.08277948336150942, -8.772275883378784, 25.579583820368846, 0.0005946176173860784, -25.072380624134254, 102048.16965721699], [1.0256330125875925, 0.14327663545986008, 0.1866767679337933, -8.920230878437964, 25.043658067331226, 0.0009892461834888455, -24.96141437769199, 102148.45008278092], [1.6897865359634758, -0.056627000773362635, 0.03674904061937184, -7.933864177873465, 26.286479774866073, -0.008350297054780385, -25.038679764026632, 101822.94967516132], [0.7987686882211862, 0.020967174002287814, 0.11434321402546777, -7.756318171036431, 25.80316022068847, 0.0020415890984940926, -25.009910737115952, 102820.8221420409], [0.8809659041921434, -0.09345135530386744, 0.22481627750062233, -8.183743745254892, 26.358813307865177, -0.010586525749650461, -25.067448791048253, 101765.41172578087], [1.3248308864318687, 0.06173699470083205, 0.47995644469336163, -8.699942315071391, 24.87597576883828, -0.0165717259712373, -25.049365402618758, 101411.96430850294], [1.1111181148543707, 0.40630773776805706, 0.5549203093056583, -8.959685549532404, 24.58006584160019, -0.004009382596067648, -24.958948461036716, 102064.60907132704], [1.2492094468908674, 0.03543388286570193, 0.29320436503981057, -8.683502874153833, 25.240931356366875, 0.0044751320298084376, -25.040323708437434, 102385.17765603494], [0.8415112314716219, -0.015857179683996525, 0.10382197109764235, -8.36128975034523, 25.586159610342886, -0.006508696976678557, -24.964702266460513, 102021.8665918818], [1.2031790040723394, 0.43787147030971574, 0.46680489114965856, -8.739396983469396, 24.67870248438199, -0.003746296849714206, -24.949906767057783, 102113.92731541373], [0.8645264589454551, 0.1353857036464915, 0.36553791656749685, -8.20675896381145, 25.918236307585516, 0.01644553246086406, -25.040323708498708, 102342.43517662614], [1.702938093987531, 0.2813679649924926, 0.37605916077701856, -8.427047526402006, 25.471083526447114, 0.018418675382905786, -24.954838600076375, 101952.82105008146], [0.8711022389190866, 0.06305215107903633, 0.3721136950929542, -7.808924396791847, 25.704523579221565, 0.006777132117386087, -25.04278962507835, 101640.47217360992], [1.7686958683374852, 0.3707985383052794, 0.09856134863620536, -9.295050229778404, 24.5636263966979, 0.022299189798510845, -24.979497766021474, 101982.41199679034], [1.6569076467914272, 0.16168881415673564, 0.282683121071797, -8.23634996633052, 25.540129173409465, 0.01986564686698383, -25.059229068969085, 101883.77551160513], [1.3248308880823247, 0.05910668305857897, 0.16957974638882117, -8.41718386312757, 25.257370793132907, 0.0103945608264739, -25.009910737203782, 101275.51716733717], [1.1275575630145545, 0.07488855063108274, 0.28268311956998077, -8.07195551659595, 25.448068304775234, 0.015722046716312395, -24.985251571325826, 101554.98721685537], [1.9002114182612835, -0.05925731348622698, -0.015857180631994205, -7.6774088373668965, 26.15496424988605, 0.015590503844082615, -25.009910737184466, 101314.97176370079], [0.9006932376829025, 0.08804010289037423, 0.30241045223936386, -7.749742396156548, 25.28367389255778, 0.007961017869320528, -24.988539460147837, 101619.10093268016], [1.4892253229450763, 0.3655379148996485, 0.13275539146300835, -8.279092521170103, 25.826175439613337, 0.01703747532627037, -24.95319465573693, 102457.51108097668], [0.976314680985114, 0.152482725397677, 0.19325254588015484, -8.10483440461572, 25.58287171880491, 0.019668332547804077, -25.06909273538919, 101859.11638700173], [1.5221042083621306, 0.42603506628065013, 0.3984168045158203, -8.831457878899462, 24.889127324747573, 0.02052336112517377, -25.047721458212337, 101990.63170464033], [0.6606773585654712, 0.3537015180628369, 0.5391384442450727, -9.27532289384464, 23.883033555139072, 0.01598513245021415, -24.99100537668246, 101625.67670103439], [1.3807249976849918, 0.3168771643021264, 0.3971016486305656, -9.120792109971513, 24.55376273747171, 0.018089818237418558, -24.946618878141738, 101686.50253584248], [1.4366191035745401, 0.084094637595031, 0.17878583614480142, -7.831939618345252, 25.990569845070805, 0.0174978753332058, -25.01319862594501, 102230.6471546882], [1.4333312156222522, 0.10776743816760453, 0.43129569272124, -9.48574779160318, 25.408613646662076, 0.019339475400628702, -25.03785779186825, 102110.63943060939], [1.4366191049902393, 0.31687716261188875, 0.47469582441796065, -9.683021136151854, 24.132913048272638, 0.013946218060777175, -24.991827348924836, 101563.20692537277], [1.8180141959680036, 0.2116647226957259, -0.01848749114242587, -8.413895971885601, 25.536841282754608, 0.024206561247617227, -25.079778373896843, 102686.0189403731], [1.1505727850948726, 0.007815619052014, 0.11039774877546588, -8.085107074198529, 26.227297790428917, 0.027823989933317538, -24.968812127518447, 102615.32945958685], [0.7330109051260003, 0.09724619411048441, 0.31950747311050975, -7.924000508555038, 26.043176056850676, 0.019142161099012175, -25.00908876497941, 102125.43490180184], [1.7917110860245415, -0.14868788814255518, 0.2392829882600312, -7.595211611507303, 25.582871718122018, 0.008355646456888863, -25.074846540710134, 101106.19119599719], [1.1538606736707524, 0.26032547695418784, 0.5102050229214992, -8.81830632687022, 24.68856614483606, 0.021838789776919672, -25.011554681646892, 101730.88895455986], [1.5056647632332703, 0.21955565491787643, 0.24717392215355527, -8.31525930182675, 25.6552052559632, 0.016379761005772927, -25.02717215335727, 101977.48017289658], [0.9269963444433174, 0.26690125441051665, 0.5036292443284728, -8.736109095904842, 24.58006583695763, 0.019931418285493475, -25.08964204035279, 101563.20692370029], [1.7128017563643017, 0.4457624026836094, 0.30372560924621067, -9.702748470003478, 24.626096274245686, 0.028284389977942748, -25.014842570443662, 102720.54171254052], [1.449770660594799, 0.1774706797542605, 0.293204364993237, -9.081337441634272, 24.879263660377774, 0.026377018469227166, -25.067448790983782, 101992.275644626], [1.5681346563036929, 0.114343214789281, 0.19851316847145212, -7.989758296191559, 25.740690349871215, 0.018155589606191617, -25.013198625910206, 101596.08575338517], [0.8283596875451974, 0.0380641963143703, 0.7219450557978133, -8.542123642001318, 24.504444409982383, -0.0012469824561334246, -25.02141834787766, 101114.41090367321], [0.6902683536947601, -0.1026574444303443, 0.04332481675159766, -7.108604041882277, 26.365389089597326, 0.009473760777586143, -24.99511523769957, 101762.12384323322], [0.8415112382027863, 0.013076240296714503, 0.4273502264943859, -7.187513380811203, 26.010297173875607, 0.010328789405961273, -25.04443356965621, 101748.97231164195], [1.6108772080587708, 0.1840464575827528, 0.27347703224226, -9.581096575868242, 25.066673284606118, 0.025850847009992406, -24.971278044189056, 102429.56407407322], [1.7785595285218954, 0.055161216108252864, -0.006651091545683108, -8.374441303730787, 25.717675133782908, 0.020720675452570142, -25.037035819736413, 102166.53343982312], [1.5418315461474963, 0.06042183752267505, 0.16300396733772582, -8.496093212698424, 25.54341705535066, 0.021509932578620914, -25.029638069886833, 102163.24555458283], [1.236057890033779, 0.32608325247707837, 0.27610734304609297, -8.229774188754428, 25.19818880738261, 0.004212046304753189, -25.00415693194555, 102197.76832945186]]
  out "TimeArray (USB6218)":timestamp[](array[timestamp])=[timestamp(3688342761.3994594 s since 1904-01-01), timestamp(3688342762.4680505 s since 1904-01-01), timestamp(3688342763.4675946 s since 1904-01-01), timestamp(3688342764.4676514 s since 1904-01-01), timestamp(3688342765.4686737 s since 1904-01-01), timestamp(3688342766.469984 s since 1904-01-01), timestamp(3688342767.470159 s since 1904-01-01), timestamp(3688342768.47213 s since 1904-01-01), timestamp(3688342769.8238606 s since 1904-01-01), timestamp(3688342770.8245606 s since 1904-01-01), timestamp(3688342771.8237367 s since 1904-01-01), timestamp(3688342772.8240294 s since 1904-01-01), timestamp(3688342773.823701 s since 1904-01-01), timestamp(3688342774.8247466 s since 1904-01-01), timestamp(3688342775.8255386 s since 1904-01-01), timestamp(3688342776.8254576 s since 1904-01-01), timestamp(3688342777.825836 s since 1904-01-01), timestamp(3688342778.8261266 s since 1904-01-01), timestamp(3688342779.826581 s since 1904-01-01), timestamp(3688342780.8273554 s since 1904-01-01), timestamp(3688342781.826626 s since 1904-01-01), timestamp(3688342782.8268657 s since 1904-01-01), timestamp(3688342783.8258696 s since 1904-01-01), timestamp(3688342784.825906 s since 1904-01-01), timestamp(3688342785.825819 s since 1904-01-01), timestamp(3688342786.827296 s since 1904-01-01), timestamp(3688342787.829418 s since 1904-01-01), timestamp(3688342788.8291 s since 1904-01-01), timestamp(3688342789.8296633 s since 1904-01-01), timestamp(3688342790.829848 s since 1904-01-01), timestamp(3688342791.829139 s since 1904-01-01), timestamp(3688342792.8296423 s since 1904-01-01), timestamp(3688342793.831637 s since 1904-01-01), timestamp(3688342794.8306546 s since 1904-01-01), timestamp(3688342795.829824 s since 1904-01-01), timestamp(3688342796.830819 s since 1904-01-01), timestamp(3688342798.0479465 s since 1904-01-01), timestamp(3688342799.047389 s since 1904-01-01), timestamp(3688342800.047347 s since 1904-01-01), timestamp(3688342801.0487537 s since 1904-01-01), timestamp(3688342802.047892 s since 1904-01-01), timestamp(3688342803.047963 s since 1904-01-01), timestamp(3688342804.0478578 s since 1904-01-01), timestamp(3688342805.0488462 s since 1904-01-01), timestamp(3688342806.0497985 s since 1904-01-01), timestamp(3688342807.0502543 s since 1904-01-01), timestamp(3688342808.049495 s since 1904-01-01), timestamp(3688342809.0488415 s since 1904-01-01)]
  out "Data Array sizes (6210)":i32[](array[numeric])=[48, 16]
  out "DataArraySize (6218)":i32[](array[numeric])=[48, 8]
  out "TimeArray size (6218)":i32=48
  out "TimeArray (LSI336)":timestamp[](array[timestamp])=[timestamp(3688342761.39444 s since 1904-01-01), timestamp(3688342762.463024 s since 1904-01-01), timestamp(3688342763.463638 s since 1904-01-01), timestamp(3688342764.463637 s since 1904-01-01), timestamp(3688342765.464684 s since 1904-01-01), timestamp(3688342766.465038 s since 1904-01-01), timestamp(3688342767.4661665 s since 1904-01-01), timestamp(3688342768.4671426 s since 1904-01-01), timestamp(3688342769.818876 s since 1904-01-01), timestamp(3688342770.819616 s since 1904-01-01), timestamp(3688342771.819715 s since 1904-01-01), timestamp(3688342772.8190737 s since 1904-01-01), timestamp(3688342773.819743 s since 1904-01-01), timestamp(3688342774.820112 s since 1904-01-01), timestamp(3688342775.820584 s since 1904-01-01), timestamp(3688342776.8214664 s since 1904-01-01), timestamp(3688342777.821848 s since 1904-01-01), timestamp(3688342778.822177 s since 1904-01-01), timestamp(3688342779.8225975 s since 1904-01-01), timestamp(3688342780.8223686 s since 1904-01-01), timestamp(3688342781.8226385 s since 1904-01-01), timestamp(3688342782.8219137 s since 1904-01-01), timestamp(3688342783.8218846 s since 1904-01-01), timestamp(3688342784.821887 s since 1904-01-01), timestamp(3688342785.821828 s since 1904-01-01), timestamp(3688342786.8223386 s since 1904-01-01), timestamp(3688342787.825325 s since 1904-01-01), timestamp(3688342788.8251424 s since 1904-01-01), timestamp(3688342789.825672 s since 1904-01-01), timestamp(3688342790.824856 s since 1904-01-01), timestamp(3688342791.8251505 s since 1904-01-01), timestamp(3688342792.8256593 s since 1904-01-01), timestamp(3688342793.8266897 s since 1904-01-01), timestamp(3688342794.826625 s since 1904-01-01), timestamp(3688342795.825836 s since 1904-01-01), timestamp(3688342796.826832 s since 1904-01-01), timestamp(3688342798.0429673 s since 1904-01-01), timestamp(3688342799.0433993 s since 1904-01-01), timestamp(3688342800.043396 s since 1904-01-01), timestamp(3688342801.0437655 s since 1904-01-01), timestamp(3688342802.0438714 s since 1904-01-01), timestamp(3688342803.043973 s since 1904-01-01), timestamp(3688342804.043901 s since 1904-01-01), timestamp(3688342805.044822 s since 1904-01-01), timestamp(3688342806.0448112 s since 1904-01-01), timestamp(3688342807.045269 s since 1904-01-01), timestamp(3688342808.0455375 s since 1904-01-01), timestamp(3688342809.0448914 s since 1904-01-01)]
  out "TimeArray Size (336)":i32=48
  out "DataArray (336)":dbl[][](array[numeric])=[[44.0656, 44.0449, 63.4418, 53.3249, 56.562, 56.5508, 56.5706, 56.1058], [44.0661, 44.0437, 63.4423, 53.3229, 56.5688, 56.5534, 56.5722, 56.1076], [44.0687, 44.0434, 63.4445, 53.324, 56.5642, 56.5484, 56.5706, 56.1051], [44.0686, 44.043, 63.4448, 53.3229, 56.568, 56.5535, 56.5727, 56.1064], [44.0657, 44.0461, 63.4482, 53.3256, 56.5712, 56.5539, 56.5774, 56.1119], [44.0665, 44.0431, 63.4469, 53.3269, 56.5685, 56.5556, 56.5704, 56.1056], [44.0683, 44.0439, 63.4445, 53.3236, 56.5708, 56.5535, 56.5731, 56.1088], [44.0655, 44.0452, 63.4441, 53.3239, 56.5722, 56.5519, 56.5714, 56.1054], [44.0686, 44.0442, 63.4478, 53.3292, 56.5674, 56.5556, 56.5706, 56.1116], [44.0681, 44.0463, 63.4441, 53.3269, 56.5677, 56.5518, 56.5769, 56.1108], [44.0714, 44.0436, 63.4476, 53.3269, 56.5663, 56.5513, 56.5717, 56.1137], [44.0673, 44.0451, 63.448, 53.3267, 56.5693, 56.5545, 56.5756, 56.1122], [44.0696, 44.0473, 63.4482, 53.3293, 56.5666, 56.5527, 56.5772, 56.1139], [44.0713, 44.0456, 63.4487, 53.3271, 56.5681, 56.5509, 56.5747, 56.1102], [44.0706, 44.0463, 63.4517, 53.3292, 56.5663, 56.551, 56.5741, 56.1116], [44.0674, 44.0445, 63.4515, 53.3286, 56.5728, 56.555, 56.5748, 56.1079], [44.0686, 44.0434, 63.4492, 53.3275, 56.5666, 56.5523, 56.5721, 56.1119], [44.0686, 44.0434, 63.4509, 53.3256, 56.5681, 56.5508, 56.5725, 56.1093], [44.0706, 44.0462, 63.4498, 53.3268, 56.5714, 56.555, 56.5736, 56.1118], [44.0691, 44.0458, 63.4486, 53.3308, 56.5684, 56.5524, 56.5717, 56.1133], [44.0709, 44.0454, 63.45, 53.3274, 56.5697, 56.5578, 56.5786, 56.1112], [44.0689, 44.0467, 63.4523, 53.3291, 56.5695, 56.5524, 56.5708, 56.1124], [44.0732, 44.0482, 63.449, 53.3261, 56.567, 56.5521, 56.5728, 56.11], [44.0686, 44.0442, 63.4486, 53.3272, 56.5674, 56.5548, 56.577, 56.1106], [44.0707, 44.0482, 63.4542, 53.3339, 56.5714, 56.5559, 56.5745, 56.1155], [44.0713, 44.0464, 63.4507, 53.329, 56.5709, 56.5567, 56.5758, 56.1113], [44.0706, 44.0462, 63.4509, 53.3299, 56.5678, 56.5536, 56.5792, 56.1128], [44.0679, 44.0458, 63.4538, 53.3321, 56.572, 56.5561, 56.5759, 56.1142], [44.0728, 44.0461, 63.4578, 53.3332, 56.5723, 56.5574, 56.5784, 56.1133], [44.071, 44.048, 63.4525, 53.3271, 56.5681, 56.5541, 56.578, 56.1121], [44.0694, 44.048, 63.4501, 53.3305, 56.5696, 56.5521, 56.5784, 56.1114], [44.0714, 44.0462, 63.4528, 53.3293, 56.5733, 56.5572, 56.5781, 56.1158], [44.07, 44.0474, 63.4525, 53.3315, 56.5708, 56.5611, 56.5786, 56.1121], [44.0726, 44.0483, 63.4509, 53.3314, 56.5718, 56.5581, 56.5742, 56.1132], [44.0711, 44.0454, 63.454, 53.3339, 56.5714, 56.5601, 56.5801, 56.1117], [44.0718, 44.0492, 63.4586, 53.3352, 56.571, 56.5592, 56.5787, 56.1163], [44.0716, 44.0461, 63.4546, 53.3287, 56.5699, 56.5525, 56.5764, 56.1156], [44.0723, 44.048, 63.4554, 53.3326, 56.5743, 56.5569, 56.5767, 56.1162], [44.0717, 44.0498, 63.4549, 53.3304, 56.5765, 56.5582, 56.5788, 56.1122], [44.0725, 44.0494, 63.4558, 53.3313, 56.5759, 56.5588, 56.5791, 56.1188], [44.0703, 44.0502, 63.4557, 53.3335, 56.5725, 56.5563, 56.5763, 56.114], [44.0724, 44.0498, 63.4568, 53.3385, 56.5688, 56.5565, 56.577, 56.1116], [44.0742, 44.0469, 63.4552, 53.3293, 56.5701, 56.5578, 56.577, 56.1168], [44.0735, 44.0504, 63.4545, 53.3318, 56.5693, 56.5575, 56.575, 56.1173], [44.0725, 44.0485, 63.4606, 53.3364, 56.5742, 56.5582, 56.5809, 56.1145], [44.0739, 44.0496, 63.4591, 53.3319, 56.5707, 56.558, 56.5788, 56.1132], [44.0707, 44.0491, 63.4594, 53.3341, 56.5713, 56.5576, 56.5787, 56.1115], [44.0737, 44.0488, 63.4557, 53.3294, 56.5704, 56.5561, 56.5737, 56.1152]]
  out "DataArray size (336)":i32[](array[numeric])=[48, 8]
  out "LastData (LSI218)":dbl[](array[numeric])=[278.76, 287.23, 205.57, 197.31, 93.015, 90.402, 59.35, 73.73, 30.0, 0.0, 0.0, 0.0, 149.39, 148.1, 73.063, 286.33, 289.87, 290.01, 289.1, 289.16, 148.02, 152.67, 122.79, 109.94, 115.85, 186.16, 287.33, 286.78, 211.21, 254.77, 250.0, 277.86, 265.54, 0.0, 182.55, 688.49, 128.86, 64.91, 64.659, 688.58, 59.451, 48.966, 66.774, 56.763, 67.829, 63.827, 0.433, 0.0]
  out "TempSensorsLocations":T16(array[ring])=[enum."T3He10", enum."T3He1-1", enum."TTH3", enum."TTH4", enum."TTH1", enum."TTH2", enum."T4He1", enum."T1K1", enum."N.C.", enum."N.C.", enum."N.C.", enum."N.C.", enum."T3He2-1", enum."T3He2-2", enum."T3He3", enum."T3He1-4", enum."T4He3-1", enum."T4He3-2", enum."T4He3-3", enum."T4He3-4", enum."T4He2-1", enum."T4He2-2", enum."T4He4", enum."T4He5", enum."T4He6", enum."T4He9", enum."T3He1-2", enum."T3He1-3", enum."T4He7", enum."T4He8", enum."T4He10", enum."T1K6", enum."TIP1", enum."N.C.", enum."TIP2", enum."N.C.", enum."TIP3", enum."TIP4", enum."TIP5", enum."N.C.", enum."T1K2", enum."T1K4", enum."T1K5", enum."T3He4", enum."T3He9", enum."TIP6", enum."N.C.", enum."N.C.", enum."T1K3-1", enum."T1K3-2", enum."T3He5", enum."T3He8", enum."T3He6-1", enum."T3He6-2", enum."T3He7-1", enum."T3He7-2"]
  out "AllTemperatures":dbl[](array[numeric])=[278.8, 287.22, 205.57, 197.32, 93.008, 90.409, 59.351, 73.73, 30.0, 0.0, 0.0, 0.0, 149.39, 148.1, 73.062, 286.32, 289.88, 290.01, 289.09, 289.16, 148.01, 152.68, 122.8, 109.94, 115.87, 186.15, 287.33, 286.77, 211.21, 254.76, 250.02, 277.86, 265.54, 0.0, 182.56, 688.49, 128.87, 64.912, 64.662, 688.58, 59.261, 49.115, 66.761, 56.764, 67.587, 63.802, 0.433, 0.0, 44.0707, 44.0491, 63.4594, 53.3341, 56.5713, 56.5576, 56.5787, 56.1115]
  out "error out (frontpanel screenshots)":errorcluster
  out "error out (graph operations)":errorcluster
  out "error out (monthly folder creation)":errorcluster={"status"=TRUE, "code"=10, "source"="Create Folder in CRYO_MASTER_FULL.vi<APPEND>\nC:\\LabVIEW\\DATA\\Google\\TUCAN Experiments\\KEK_cryotests_2019-2020\\data\\screenshots\\202011"}
  out "RUN Identifier 7":string="20201116_123919_RUNII" caption="RUN Identifier"
  out "error out (notifier)":errorcluster
  # "GLOBAL STATUS/CONTROL"
  # "Global Settings"
  # "USB6210 Analog inputs Settings"
  # "USB6218 Analog inputs Settings"
  # "USB6218 Digital Output Settings"
  # "USB6218 Analog Output Settings"
  # "LSI218 Settings"
  # "LSI336 Settings"
  # "Graph screenshots"
  # "Configuration"
  # "Activated only when *FIll state* = TRUE"
  # "Activated only when *FIll state* = TRUE"
  # "Vavle Status"
  # "OPEN"
  # "CLOSED"
  # "ADCMT6240A Control/Status"
  # "ADCMT6240A Initialization"
  # "Set Currents (mA)"
  # "PWR400H CTRL via USB6218"
  # "PMC18-3A CTRL via USB621"
  # "DMM configurations"
  # "DMM measurements"
  # "CAUTION: ADCMT 7351 does not have 4-wire resistance measurement function. \n 4-Wire Resistance --> 2-Wire Resistance wih Low Power for this device"
  # "Representative temperatures"
  # "Pressures / Flows"
  # "Labels"
  # "Values"
  # "Helium Levels"
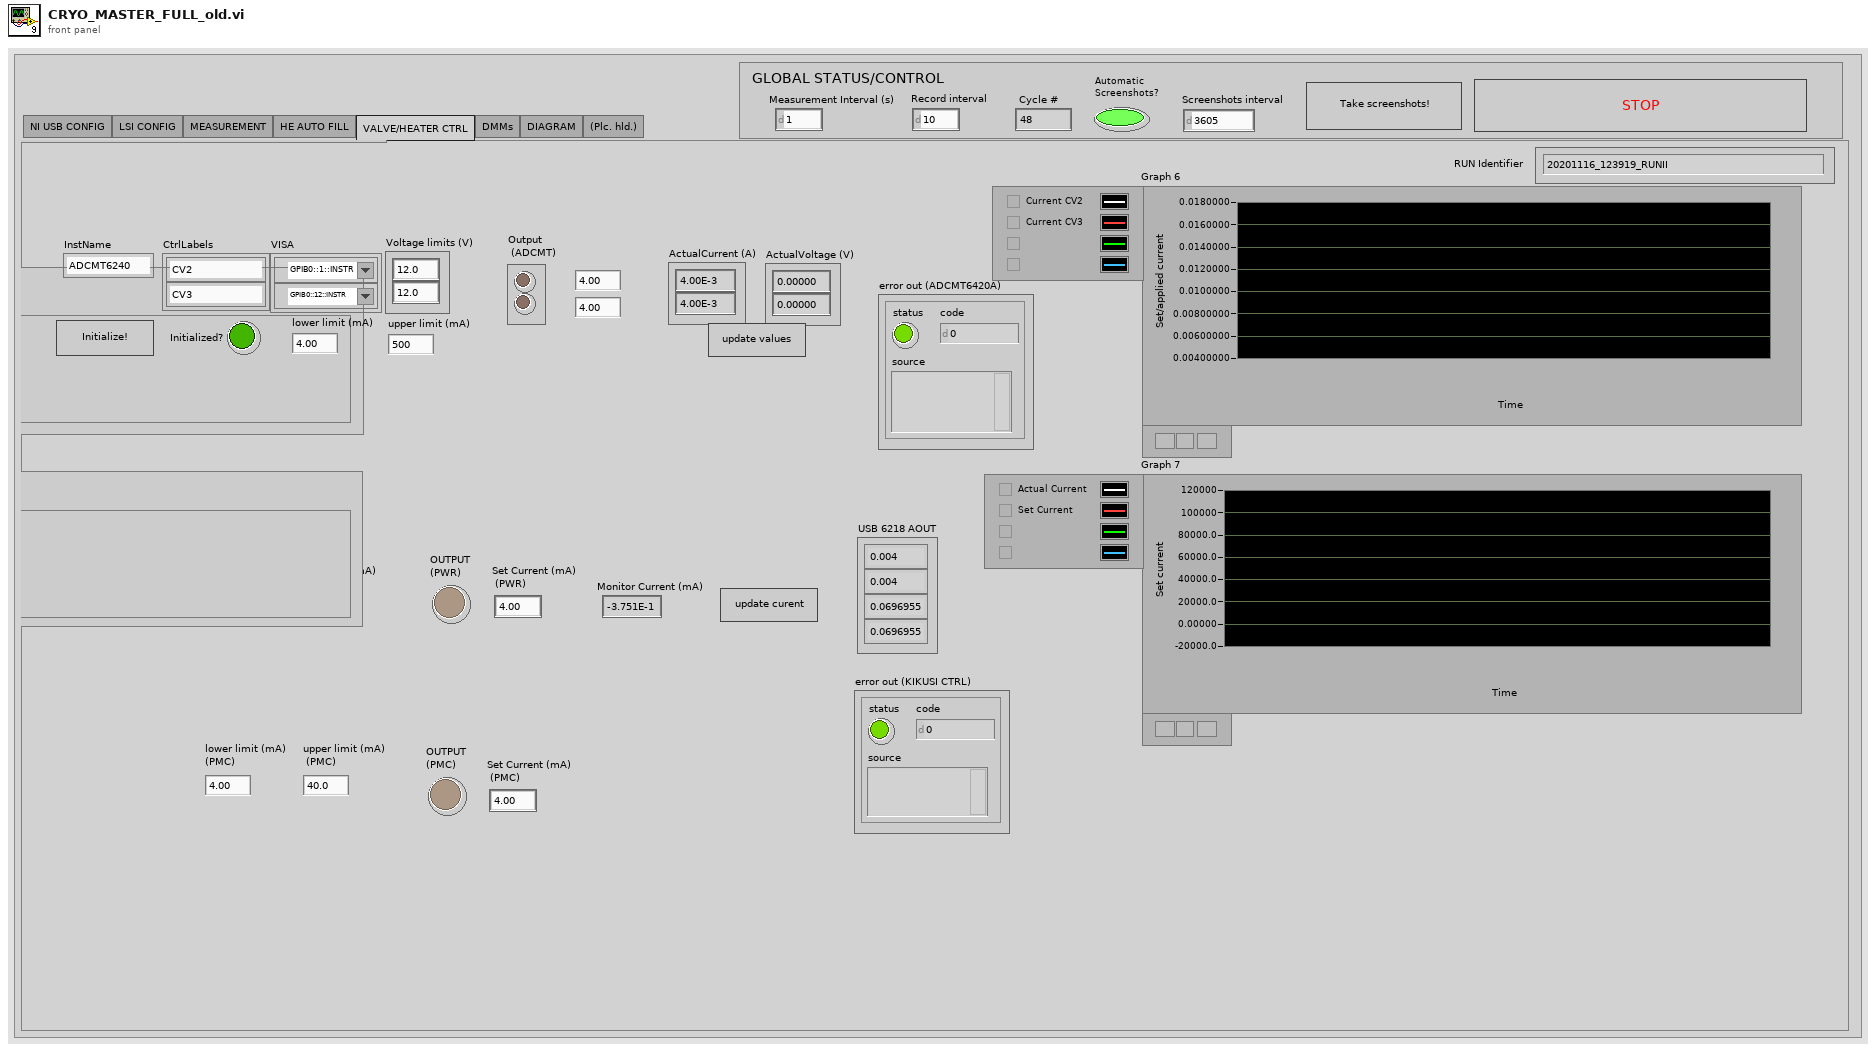
[diagram p1: front panel]
types:
  T1 = enum32{"NI USB CONFIG", "LSI CONFIG", "MEASUREMENT", "HE AUTO FILL", "VALVE/HEATER CTRL", "DMMs", "DIAGRAM", "(Plc. hld.)"}
  T2 = cluster{"Label":string, "FileFormat":string, "Active?":bool, "Physical CH":tag, " terminal\n type":i32, "ConversionType":cluster{"Type":enum16{"Raw", "SimpleProp", "CC-10_COMBINED", "CC-10_LOG", "LeakDet_EXP", "LeakDet_Mantissa", "Baratron"}, "ConversionParameters":dbl[]}, "VoltageLimits":dbl[]}[]
  T3 = cluster{"LSIName":string, "Labels":string[], "SensorLocations":enum16{"N.C.", "T3He1-1", "T3He1-2", "T3He1-3", "T3He1-4", "T3He2-1", "T3He2-2", "T3He3", "T3He4", "T3He5", "T3He6-1", "T3He6-2", "T3He7-1", "T3He7-2", "T3He8", "T3He9", "T3He10", "T4He1", "T4He2-1", "T4He2-2", "T4He3-1", "T4He3-2", "T4He3-3", "T4He3-4", "T4He4", "T4He5", "T4He6", "T4He7", "T4He8", "T4He9", "T4He10", "T1K1", "T1K2", "T1K3-1", "T1K3-2", "T1K4", "T1K5", "T1K6", "TIP1", "TIP2", "TIP3", "TIP4", "TIP5", "TIP6", "TIP7", "TTH1", "TTH2", "TTH3", "TTH4"}[], "Active?":bool, "VISA res. name":refnum<visa-resource-name>}[]
  T4 = cluster{"TimeArray":timestamp[], "DataArray":dbl[]}[]
  T5 = enum32{"USB6210", "USB6218", "Temeprature (1)", "Temperature (2)", "Temperature (3)"}
  T6 = enum16{"Intialized", "Ready", "Measuring", "Terminated"}
  T7 = enum16{"Initialized", "Ready", "Measuring", "Terminated"}
  T8 = enum16{"USB6210", "USB6218AI", "USB6218AO", "LSI218", "LSI336"}
  T9 = cluster{"TimeArray":timestamp[], "Filtered X":dbl[]}[]
  T10 = cluster{"TimeArray (USB6218)":timestamp[], "DataArrayConv (USB6218)":dbl[]}[]
  T11 = enum16{"USB6210", "USB6218AI", "USB6218AO", "LSI218", "LSI336"}[]
  T12 = cluster{"Label":string, "Active?":bool, "Source":enum16{"USB6210", "USB6218AI", "USB6218AO", "LSI218", "LSI336"}, "SourceLabel":string, "FileFormat":string}[]
  T13 = cluster{"Label":string, "Active?":bool, "VISA resource name":refnum<visa-resource-name>, "Device":enum16{"Agilent34401A", "ADCMT7351", "HP3478A"}, "Measurement":enum16{"DC Volts", "DC Currents", "2-Wire Resistance", "4-Wire Resistance"}, "FileFormat":string}[]
  T14 = enum16{"N.C.", "T3He1-1", "T3He1-2", "T3He1-3", "T3He1-4", "T3He2-1", "T3He2-2", "T3He3", "T3He4", "T3He5", "T3He6-1", "T3He6-2", "T3He7-1", "T3He7-2", "T3He8", "T3He9", "T3He10", "T4He1", "T4He2-1", "T4He2-2", "T4He3-1", "T4He3-2", "T4He3-3", "T4He3-4", "T4He4", "T4He5", "T4He6", "T4He7", "T4He8", "T4He9", "T4He10", "T1K1", "T1K2", "T1K3-1", "T1K3-2", "T1K4", "T1K5", "T1K6", "TIP1", "TIP2", "TIP3", "TIP4", "TIP5", "TIP6", "TIP7", "TTH1", "TTH2", "TTH3", "TTH4"}
  T15 = cluster{"LSIName":string, "Active?":bool, "LastData":dbl[], "Labels":string[]}[]
  T16 = enum16{"N.C.", "T3He1-1", "T3He1-2", "T3He1-3", "T3He1-4", "T3He2-1", "T3He2-2", "T3He3", "T3He4", "T3He5", "T3He6-1", "T3He6-2", "T3He7-1", "T3He7-2", "T3He8", "T3He9", "T3He10", "T4He1", "T4He2-1", "T4He2-2", "T4He3-1", "T4He3-2", "T4He3-3", "T4He3-4", "T4He4", "T4He5", "T4He6", "T4He7", "T4He8", "T4He9", "T4He10", "T1K1", "T1K2", "T1K3-1", "T1K3-2", "T1K4", "T1K5", "T1K6", "TIP1", "TIP2", "TIP3", "TIP4", "TIP5", "TIP6", "TIP7", "TTH1", "TTH2", "TTH3", "TTH4"}[]
  T17 = cluster{"TimeArray (USB6218)":timestamp[], "DataArrayConv (USB6218)":dbl[]}
  T18 = cluster{"appended array":timestamp[], "ActualCurrentArray":dbl[]}
  T19 = cluster{"appended array":timestamp[], "SetCurrentArray":dbl[]}
  T20 = cluster{"appended array":timestamp[], "SetCurrentArray":dbl[]}[]
  T21 = typedef "imagedata.ctl" = cluster{"image type":i32, "image depth":i32, "image":u8[], "mask":u8[], "colors":u32[], "Rectangle":cluster{"left":i16, "top":i16, "right":i16, "bottom":i16}}
  T22 = enum16{"open", "replace", "create", "open or create", "replace or create", "replace or create with confirmation"}
  T23 = cluster{"TimeArray":timestamp[], "DataArrayConv":dbl[]}[]
  T24 = cluster{"IndexArray":i64[], "TimeArray":timestamp[], "DataArrayRaw":dbl[][], "DataArrayConv":dbl[][], "LDArray":dbl[]}
  T25 = cluster{"InstName":string, "Active?":bool, "Status":enum16{"Intialized", "Ready", "Measuring", "Terminated"}, "Labels":string[], "LabelLD":string, "FileFormat":string[], "FileFormatLD":string, "ReadLeakDet?":bool}
  T26 = cluster{"AOUT Labels[0]":string, "AOUT Labels[1]":string, "AOUT Labels[2]":string, "AOUT Labels[3]":string, "AOUT Labels[4]":string, "AOUT Labels[5]":string, "AOUT Labels[6]":string, "AOUT Labels[7]":string, "AOUT Labels[8]":string}
  T27 = cluster{"TimeArray":timestamp[], "DataArrayConv":dbl[]}
  T28 = cluster{"TimeArray":timestamp[], "DataArrayConv (USB6218)":dbl[]}
  T29 = cluster{"TimeArray":timestamp[], "M.A. Array":dbl[]}
  T30 = cluster{"TimeArray":timestamp[], "M.A. Array":dbl[]}[]
  T31 = cluster{"TimeArray":timestamp[], "DataArray":dbl[]}
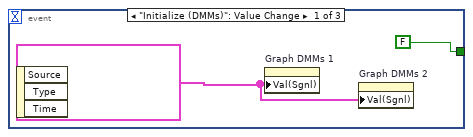
[diagram p2: hidden frame]
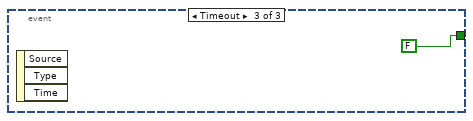
[diagram p3: hidden frame]
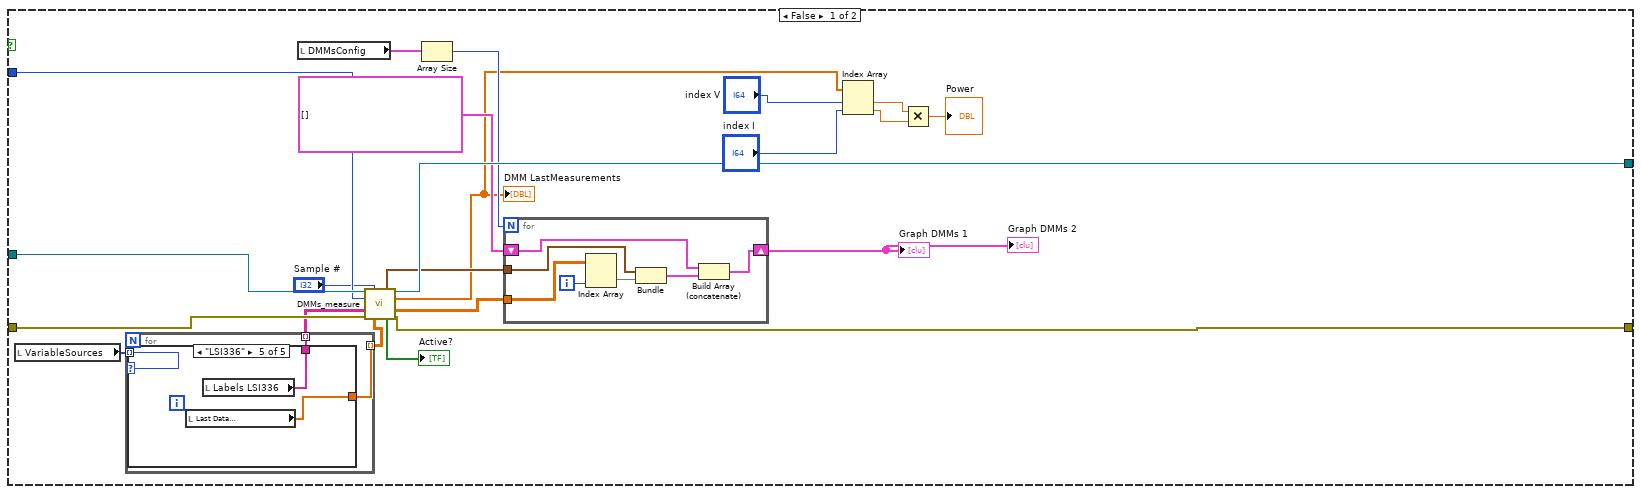
[diagram p5: hidden frame]
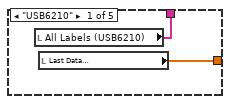
[diagram p6: hidden frame]
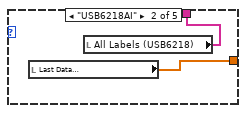
[diagram p7: hidden frame]
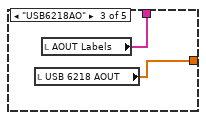
[diagram p8: hidden frame]
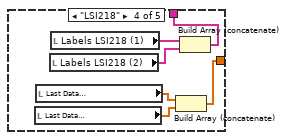
[diagram p9: hidden frame]
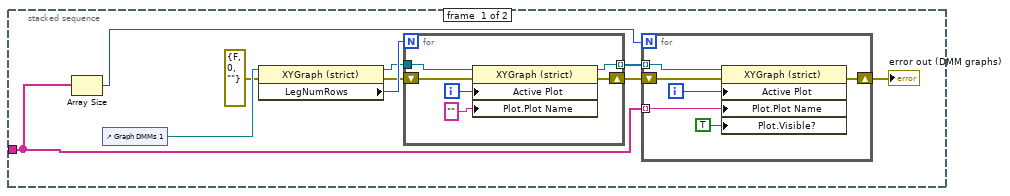
[diagram p10: hidden frame]
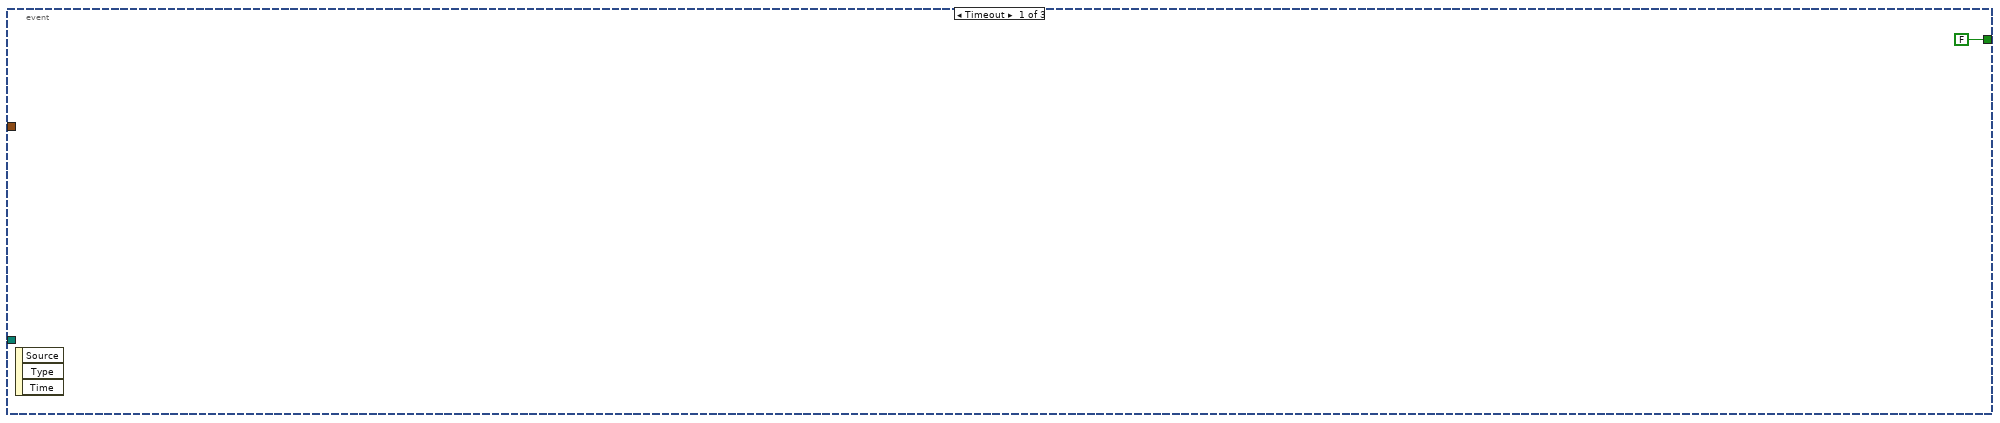
[diagram p11: hidden frame]
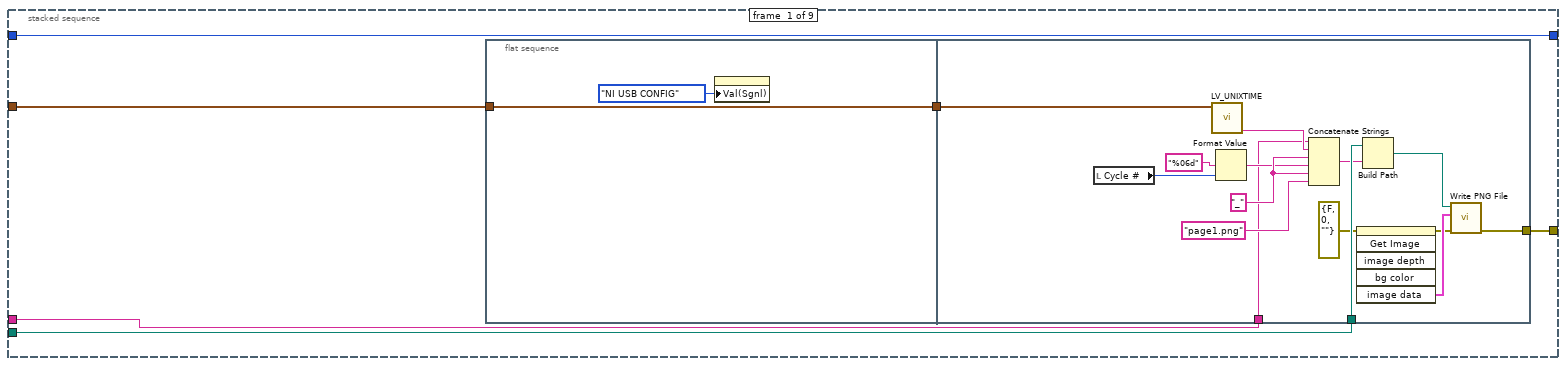
[diagram p12: hidden frame]
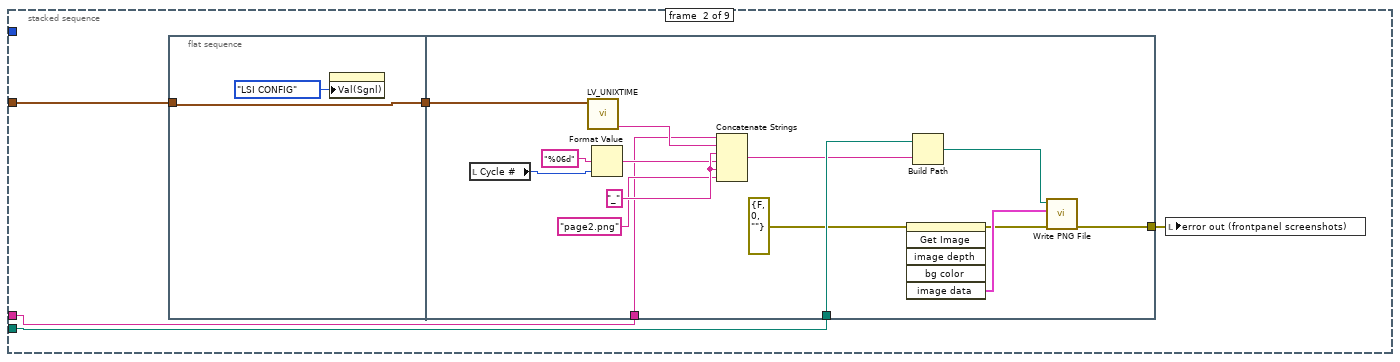
[diagram p13: hidden frame]
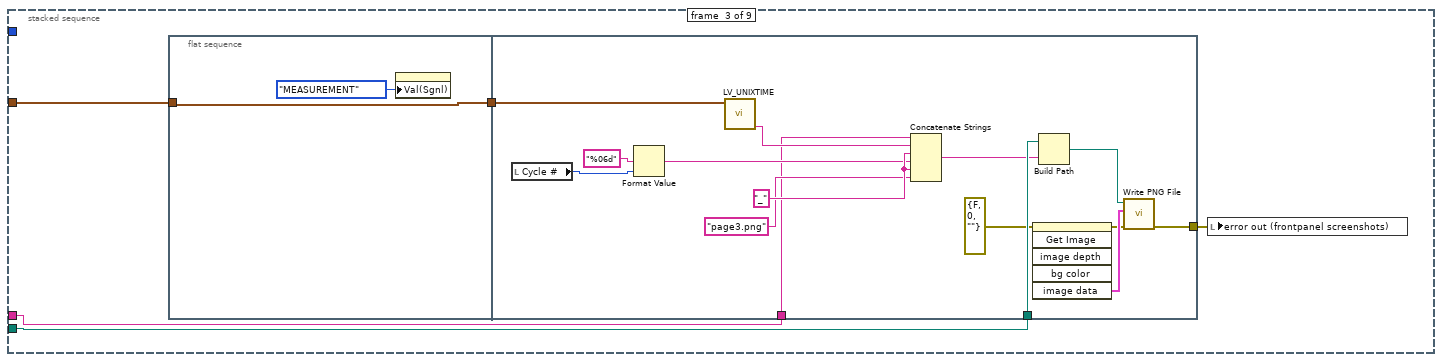
[diagram p14: hidden frame]
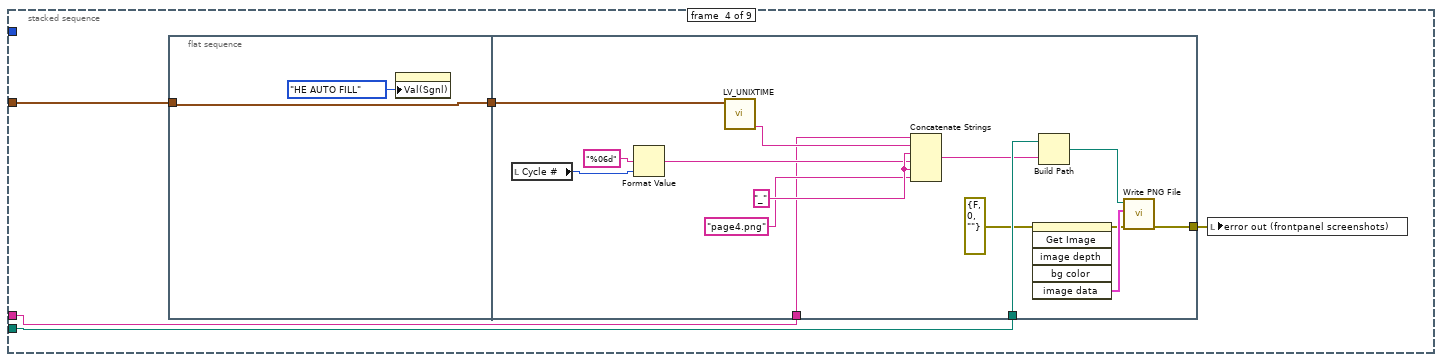
[diagram p15: hidden frame]
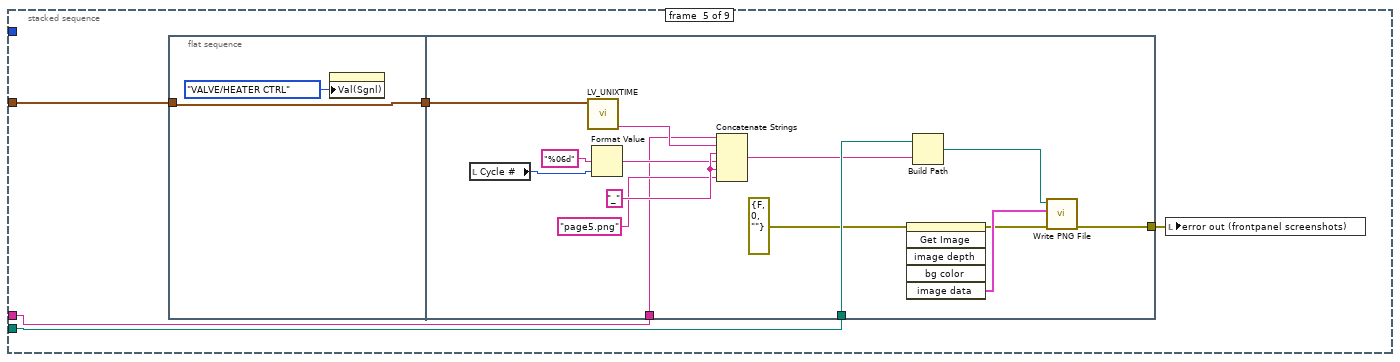
[diagram p16: hidden frame]
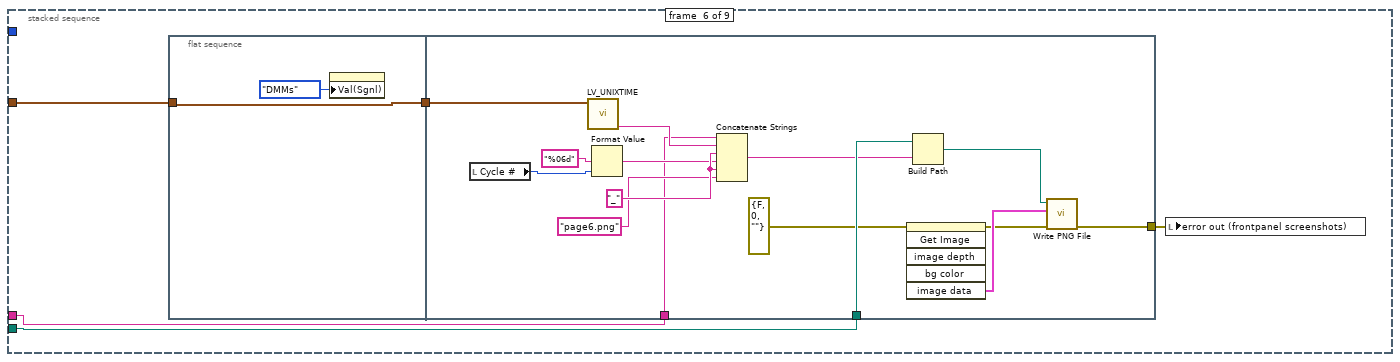
[diagram p17: hidden frame]
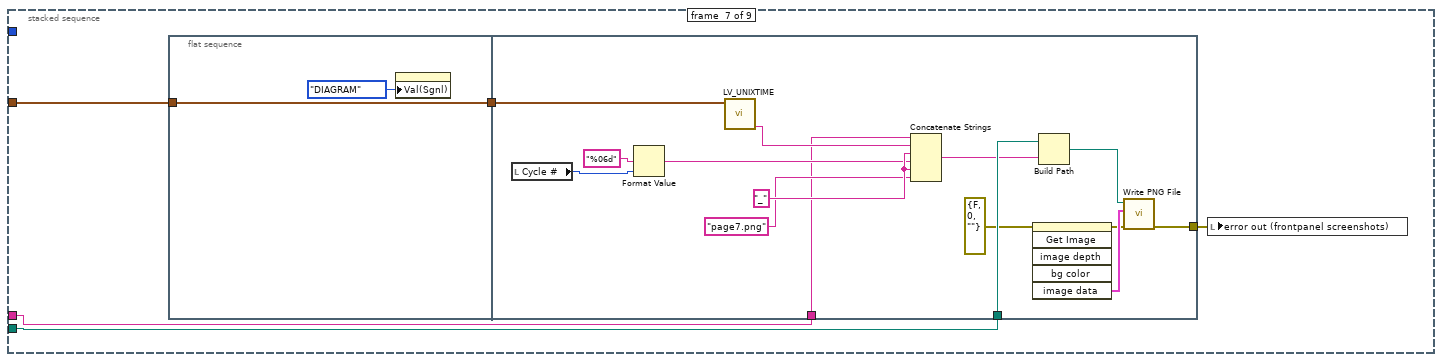
[diagram p18: hidden frame]
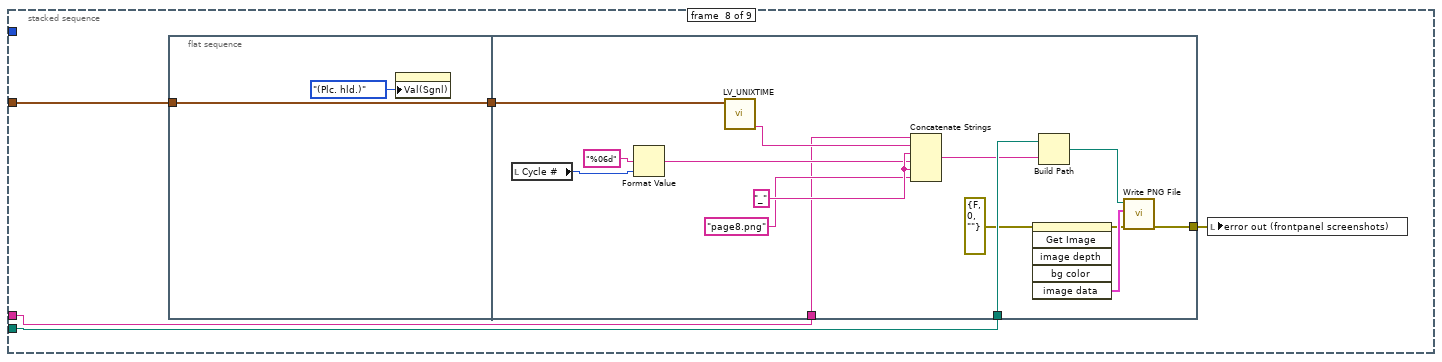
[diagram p19: hidden frame]
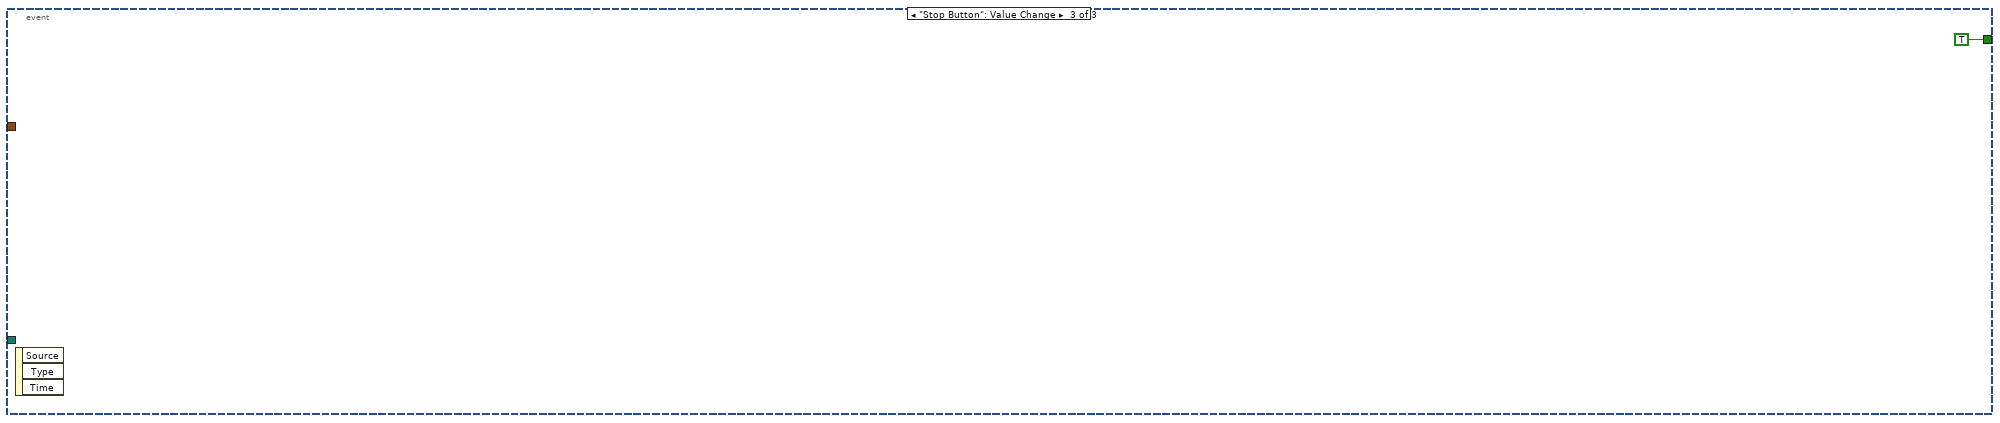
[diagram p20: hidden frame]
diagram:
  w13 = TRUE ("create if not found? (T)")
  w17 = errorcluster {"status"=FALSE, "code"=0, "source"=""} ("error in (no error)")
  n1 = while {
    shift-right: [w43] -> _
    shift-left: dbl[] [] -> [w49]
    shift-right: [w46] -> _
    shift-left: timestamp[] [] -> [w48]
    i -> [w47]
    stop <- w50 stop-if-true
    n2 = Wait (ms)(milliseconds to wait=u32 225) -> ()  [unwired: 1 out]
    n3 = event shown="[6] \"OUTPUT (PWR)\", \"OUTPUT (PMC)\": Value Change" {
      selector: _ -> [_ _ _ _ _ _ _]
      dyn-events: _ -> [_ _ _ _ _ _ _]
      timeout: _ -> [_ _ _ _ _ _ _]
      tunnel: [_ TRUE _ _ _ _ _] -> w50
      tunnel: w47 -> [_ _ _ _ w131 _ _]
      tunnel: [_ _ _ _ w130 w214 _] -> w43
      tunnel: w49 -> [_ _ _ _ w127 w214 _]
      tunnel: [w52 w62 _ _ w129 w213 w217] -> w46
      tunnel: w48 -> [w52 w62 _ _ w128 w213 w217]
      tunnel: w47 -> [_ _ w68 w92 _ _ w218]
      tunnel: [_ _ _ _ w118 _ _] -> w42
      event Timeout {
        n4 = event-data() -> ()  [unwired: 1 in, 3 out]
      }
      event "Stop Button": Value Change {
        w53 = FALSE
        n5 = event-data() -> ()  [unwired: 1 in, 3 out]
        n6 = local read "error out (USB6210/6218 DOUT)"() -> (w61:errorcluster)
        n7 = local read "error out (USB6210/6218 AOUT)"() -> (w58:errorcluster)
        n8 = local read "DOUT task out"() -> (w57:refnum<k21>)
        n9 = local read "AO task out"() -> (w64:refnum<k21>)
        n10 = property on="OUTPUT\n(PWR)" class="Bool (strict)"("Value"=w53) -> ()  [unwired: 2 in, 2 out]
        n11 = property on="V2 (N.C.)" class="Bool (strict)"("Val(Sgnl)"=w53) -> ()  [unwired: 2 in, 2 out]
        n12 = property on="OUTPUT\n(PMC)" class="Bool (strict)"("Value"=w53) -> ()  [unwired: 2 in, 2 out]
        n13 = Build Array(w53, w53, w53, w53) -> (w60:bool[])
        n14 = Not(x=w53) -> (.not. x?=w54:bool)
        n15 = call <vilib>:"DAQmx Clear Task.vi"("task in"=w64, "error in"=w58) -> ("error out"=w63:errorcluster)  [unwired: 13 in]
        n16 = property on="V1 (N.O.)" class="Bool (strict)"("Val(Sgnl)"=w54) -> ()  [unwired: 2 in, 2 out]
        n17 = call <vilib>:"DAQmx Write (Digital 1D Bool NChan 1Samp 1Line).vi"("task/channels in"=w57, "data"=w60, "timeout"=10.0, "error in"=w61) -> ("task out"=w56:refnum<k21>, "error out"=w55:errorcluster)  [unwired: 9 in, 1 out]
        n18 = call <vilib>:"DAQmx Clear Task.vi"("task in"=w56, "error in"=w55) -> ("error out"=w65:errorcluster)  [unwired: 13 in]
        n19 = local write "error out (USB6210/6218 AOUT)"(w63) -> ()
        n20 = local write "error out (USB6210/6218 DOUT)"(w65) -> ()
      }
      event "V1 (N.O.)": Value Change {
        n21 = event-data() -> ()  [unwired: 1 in, 3 out]
        n22 = local read "Cycle #"() -> (w71:u32)
        n23 = Greater?(x=w71, y=u32 0) -> (0:w69:bool)
        n24 = case shown="True" w69 {
          tunnel: "V1 (N.O.)" -> [_ w85]
          tunnel: w68 -> [_ w80]
          frame False {
          }
          frame True {
            n25 = Not(x=w85) -> (.not. x?=w87:bool)
            n26 = property on="OUTPUT\n(PMC)" class="Bool (strict)"() -> ("Value"=w72:bool)  [unwired: 2 in, 2 out]
            n27 = local read "error out (USB6210/6218 DOUT)"() -> (w86:errorcluster)
            n28 = property on="OUTPUT\n(PWR)" class="Bool (strict)"() -> ("Value"=w83:bool)  [unwired: 2 in, 2 out]
            n29 = property on="V2 (N.C.)" class="Bool (strict)"() -> ("Value"=w84:bool)  [unwired: 2 in, 2 out]
            n30 = local read "DOUT task out"() -> (w90:refnum<k21>)
            n31 = Build Array(w87, w84, w83, w72) -> (w76:bool[])
            n32 = local read "File Refn USB DO"() -> (w81:refnum<file>)
            n33 = Boolean To (0,1)(Boolean=w76) -> (0, 1=w75:i16[])
            n34 = Initialize Array("%d" ("element"), 3 ("dimension size")) -> (w79:string[])
            n35 = call <vilib>:"DAQmx Write (Digital 1D Bool NChan 1Samp 1Line).vi"("task/channels in"=w90, "data"=w76, "timeout"=10.0, "error in"=w86) -> ("task out"=w88:refnum<k21>, "error out"=w74:errorcluster)  [unwired: 9 in, 1 out]
            n36 = local write "DOUT task out"(w88) -> ()
            n37 = Get Date/Time In Seconds() -> (seconds since 1Jan1904=w82:timestamp)
            n38 = call "FileWrite.vi"("DataArray"=w75, "Time Stamp"=w82, "Error In"=w74, "FileFormat"=w79, "Index"=w80, "refnum in"=w81) -> ("Error Out"=w73:errorcluster)  [unwired: 4 in, 1 out]
            n39 = local write "error out (USB6210/6218 DOUT)"(w73) -> ()
          }
        }
        "V1" <- "V1 (N.O.)"
      }
      event "V2 (N.C.)": Value Change {
        n40 = event-data() -> ()  [unwired: 1 in, 3 out]
        n41 = local read "Cycle #"() -> (w95:u32)
        n42 = Greater?(x=w95, y=u32 0) -> (0:w93:bool)
        n43 = case shown="True" w93 {
          tunnel: "V2 (N.C.)" -> [_ w110]
          tunnel: w92 -> [_ w102]
          frame False {
          }
          frame True {
            n44 = property on="OUTPUT\n(PMC)" class="Bool (strict)"() -> ("Value"=w96:bool)  [unwired: 2 in, 2 out]
            n45 = property on="V1 (N.O.)" class="Bool (strict)"() -> ("Value"=w109:bool)  [unwired: 2 in, 2 out]
            n46 = Not(x=w109) -> (.not. x?=w108:bool)
            n47 = local read "error out (USB6210/6218 DOUT)"() -> (w113:errorcluster)
            n48 = property on="OUTPUT\n(PWR)" class="Bool (strict)"() -> ("Value"=w107:bool)  [unwired: 2 in, 2 out]
            n49 = local read "DOUT task out"() -> (w114:refnum<k21>)
            n50 = Build Array(w108, w110, w107, w96) -> (w105:bool[])
            n51 = local read "File Refn USB DO"() -> (w106:refnum<file>)
            n52 = Boolean To (0,1)(Boolean=w105) -> (0, 1=w104:i16[])
            n53 = Initialize Array("%d" ("element"), 3 ("dimension size")) -> (w99:string[])
            n54 = call <vilib>:"DAQmx Write (Digital 1D Bool NChan 1Samp 1Line).vi"("task/channels in"=w114, "data"=w105, "timeout"=10.0, "error in"=w113) -> ("task out"=w111:refnum<k21>, "error out"=w98:errorcluster)  [unwired: 9 in, 1 out]
            n55 = local write "DOUT task out"(w111) -> ()
            n56 = Get Date/Time In Seconds() -> (seconds since 1Jan1904=w103:timestamp)
            n57 = call "FileWrite.vi"("DataArray"=w104, "Time Stamp"=w103, "Error In"=w98, "FileFormat"=w99, "Index"=w102, "refnum in"=w106) -> ("Error Out"=w97:errorcluster)  [unwired: 4 in, 1 out]
            n58 = local write "error out (USB6210/6218 DOUT)"(w97) -> ()
          }
        }
        "V2" <- "V2 (N.C.)"
      }
      event "Set Current (mA)\n (PMC)", "Set Current (mA)\n (PWR)", "update current": Value Change {
        n59 = event-data() -> ()  [unwired: 1 in, 3 out]
        n60 = case shown="True" "CONTROL KIKUSUI?" {
          tunnel: w131 -> [_ w182]
          tunnel: [w141 w175] -> w130
          tunnel: [w144 w174] -> w129
          tunnel: w128 -> [w146 w177]
          tunnel: w127 -> [w142 w176]
          tunnel: "Set Current (mA)\n (PWR)" -> [_ w154]
          tunnel: "Set Current (mA)\n (PMC)" -> [_ w158]
          frame False {
            w143 = 0.0 ("element")
            n61 = Get Date/Time In Seconds() -> (seconds since 1Jan1904=w145:timestamp)
            n62 = local read "AO task out"() -> (w151:refnum<k21>)
            n63 = Build Array (concatenate)(w146, w145) -> (w144:timestamp[])
            n64 = Build Array (concatenate)(w142, w143) -> (w141:dbl[])
            n65 = Build Array(w143, w143) -> (w149:dbl[])
            n66 = call <vilib>:"DAQmx Write (Analog 1D DBL NChan 1Samp).vi"("task/channels in"=w151, "data"=w149, "timeout"=100.0, "error in"=errorcluster {"status"=FALSE, "code"=0, "source"=""}) -> ("task out"=w152:refnum<k21>, "error out"=w147:errorcluster)  [unwired: 9 in, 1 out]
            n67 = local write "AO task out"(w152) -> ()
            n68 = local write "error out (KIKUSI CTRL)"(w147) -> ()
          }
          frame True {
            w169 = 2 ("index")
            n69 = xnode "Formula"("X1"=w154) -> ("Result"=w171:dbl)  [unwired: 1 in, 1 out]
            n70 = xnode "Formula"("X1"=w158) -> ("Result"=w165:dbl)  [unwired: 1 in, 1 out]
            n71 = Build Array (concatenate)(w176, w154) -> (w175:dbl[])
            n72 = In Range and Coerce(upper limit=10.0, x=w171, lower limit=0.0 ("y")) -> (coerced(x)=w163:dbl, In Range?=w164:bool)
            n73 = In Range and Coerce(upper limit=10.0, x=w165, lower limit=0.0 ("y")) -> (coerced(x)=w160:dbl, In Range?=w161:bool)
            n74 = case shown="False" w164 {
              tunnel: w163 -> [_ w194]
              tunnel: [0.0 ("upper limit") w194] -> w162
              frame False {
              }
              frame True {
              }
            }
            n75 = case shown="True" w161 {
              tunnel: w160 -> [_ w192]
              tunnel: [0.0 ("upper limit") w192] -> w159
              frame False {
              }
              frame True {
              }
            }
            n76 = Multiply(x=w154, y=0.001) -> (x*y=w153:dbl)
            n77 = Multiply(x=w158, y=0.001) -> (x*y=w157:dbl)
            n78 = local read "File Refn USB AO"() -> (w183:refnum<file>)
            n79 = Build Array(w153, w157, w162, w159) -> (w170:dbl[])
            "USB 6218 AOUT" <- w170
            n80 = Initialize Array("%.3f", 4 ("dimension size")) -> (w184:string[])
            n81 = Get Date/Time In Seconds() -> (seconds since 1Jan1904=w178:timestamp)
            n82 = local read "AO task out"() -> (w188:refnum<k21>)
            n83 = call "FileWrite.vi"("DataArray"=w170, "Time Stamp"=w178, "Error In"=errorcluster {"status"=FALSE, "code"=0, "source"=""} ("error in"), "FileFormat"=w184, "Index"=w182, "refnum in"=w183) -> ("Error Out"=w180:errorcluster, "Byte Stream File Refnum"=w179:refnum<file>)  [unwired: 4 in]
            n84 = Build Array (concatenate)(w177, w178) -> (w174:timestamp[])
            n85 = Array Subset(array=w170, index=w169, length=w169) -> (w168:dbl[])
            n86 = local write "File Refn USB AO"(w179) -> ()
            n87 = call <vilib>:"DAQmx Write (Analog 1D DBL NChan 1Samp).vi"("task/channels in"=w188, "data"=w168, "timeout"=100.0, "error in"=w180) -> ("task out"=w189:refnum<k21>, "error out"=→"error out (KIKUSI CTRL)":errorcluster)  [unwired: 9 in, 1 out]
            n88 = local write "AO task out"(w189) -> ()
          }
        }
        n89 = local read "All Labels (USB6218)"() -> (w124:string[])
        n90 = local read "DataArrayConv (USB6218)"() -> (w123:dbl[][])
        n91 = local read "Last Data \n(USB6218)"() -> (w120:dbl[])
        n92 = local read "TimeArray (USB6218)"() -> (w121:timestamp[])
        n93 = Search 1D Array(1D array=w124, element="I_CV") -> (index of element=w125:i32)  [unwired: 1 in]
        n94 = Index Array(array=w123, index (row)=w125) -> (element=w122:dbl[])  [unwired: 1 in]
        n95 = Index Array(array=w120, index=w125) -> (element=w117:dbl)
        n96 = Bundle("TimeArray (USB6218)"=w121, "DataArrayConv (USB6218)"=w122) -> (w118:T17)  [unwired: 1 in]
        n97 = xnode "Formula"("X1"=w117) -> ("Result"=→"Monitor Current (mA)":dbl)  [unwired: 1 in, 1 out]
      }
      event "upper limit (mA)\n (PWR)", "lower limit (mA) \n(PWR)": Value Change {
        n98 = event-data() -> ()  [unwired: 1 in, 6 out]
        n99 = property on="Set Current (mA)\n (PWR)" class="DigNum (strict)"("Maximum"="upper limit (mA)\n (PWR)", "Minimum"="lower limit (mA) \n(PWR)") -> ()  [unwired: 2 in, 2 out]
        n100 = property on="Set Current (mA)\n (PMC)" class="DigNum (strict)"("Maximum"="upper limit (mA)\n (PMC)", "Minimum"="lower limit (mA) \n(PMC)") -> ()  [unwired: 2 in, 2 out]
      }
      event "OUTPUT\n(PWR)", "OUTPUT\n(PMC)": Value Change {
        n101 = event-data() -> ()  [unwired: 1 in, 6 out]
        n102 = local read "Cycle #"() -> (w221:u32)
        n103 = Greater?(x=w221, y=u32 0) -> (0:w219:bool)
        n104 = case shown="True" w219 {
          tunnel: w218 -> [_ w226]
          frame False {
          }
          frame True {
            n105 = property on="V1 (N.O.)" class="Bool (strict)"() -> ("Value"=w237:bool)  [unwired: 2 in, 2 out]
            n106 = Not(x=w237) -> (.not. x?=w236:bool)
            n107 = local read "error out (USB6210/6218 DOUT)"() -> (w240:errorcluster)
            n108 = property on="V2 (N.C.)" class="Bool (strict)"() -> ("Value"=w235:bool)  [unwired: 2 in, 2 out]
            n109 = local read "DOUT task out"() -> (w241:refnum<k21>)
            n110 = Build Array(w236, w235, "OUTPUT\n(PWR)", "OUTPUT\n(PMC)") -> (w224:bool[])
            n111 = local read "File Refn USB DO"() -> (w227:refnum<file>)
            n112 = Boolean To (0,1)(Boolean=w224) -> (0, 1=w223:i16[])
            n113 = call <vilib>:"DAQmx Write (Digital 1D Bool NChan 1Samp 1Line).vi"("task/channels in"=w241, "data"=w224, "timeout"=10.0, "error in"=w240) -> ("task out"=w238:refnum<k21>, "error out"=w231:errorcluster)  [unwired: 9 in, 1 out]
            n114 = Initialize Array("%d" ("element"), 3 ("dimension size")) -> (w229:string[])
            n115 = local write "DOUT task out"(w238) -> ()
            n116 = Get Date/Time In Seconds() -> (seconds since 1Jan1904=w228:timestamp)
            n117 = call "FileWrite.vi"("DataArray"=w223, "Time Stamp"=w228, "Error In"=w231, "FileFormat"=w229, "Index"=w226, "refnum in"=w227) -> ("Error Out"=w230:errorcluster, "Byte Stream File Refnum"=w225:refnum<file>)  [unwired: 4 in]
            n118 = local write "File Refn USB DO"(w225) -> ()
            n119 = local write "error out (USB6210/6218 DOUT)"(w230) -> ()
          }
        }
      }
    }
    n120 = Bundle(w46, w43) -> (w45:cluster{timestamp[], dbl[]})  [unwired: 1 in]
    n121 = Build Array(w45, w42) -> (→"Graph 7":T10)
  }
  n122 = while {
    shift-right: [w250] -> _
    shift-left: refnum<class "6240AData.lvclass"> refnum ("6240AData.lvclass") -> [w248]
    shift-right: [w246] -> _
    shift-left: errorcluster {"status"=FALSE, "code"=0, "source"=""} ("error in (no error)") -> [w247]
    i -> [w242]
    stop <- w249 stop-if-true
    n123 = Wait (ms)(milliseconds to wait=u32 231) -> ()  [unwired: 1 out]
    n124 = Equal?(x=w242, y=0) -> (x = y?=w244:bool)
    n125 = case shown="True" w244 {
      frame False {
      }
      frame True {
        n126 = property on="Initialized?" class="Bool (strict)"("Val(Sgnl)"=FALSE ("Value (Signaling)")) -> ()  [unwired: 2 in, 2 out]
      }
    }
    n127 = event shown="[3] \"Initialize\": Value Change" {
      selector: _ -> [_ _ _ _ _]
      dyn-events: _ -> [_ _ _ _ _]
      timeout: _ -> [_ _ _ _ _]
      tunnel: [w253 w268 _ w317 w338] -> w250
      tunnel: [_ _ _ _ TRUE ("Value (Signaling)")] -> w249
      tunnel: w248 -> [w253 w267 _ w301 w336]
      tunnel: w247 -> [w252 w266 _ w300 w334]
      tunnel: [w252 w265 _ w315 w337] -> w246
      tunnel: w242 -> [_ w264 _ _ _]
      tunnel: w242 -> [_ _ _ w309 _]
      event Timeout {
        n128 = event-data() -> ()  [unwired: 1 in, 3 out]
      }
      event "update values", "SetCurrent 1 (mA)", "SetCurrent 2 (mA)": Value Change {
        w257 = 1000.0 ("y")
        n129 = event-data() -> ()  [unwired: 1 in, 6 out]
        n130 = local read "Initialized?"() -> (w263:bool)
        n131 = Divide(x="SetCurrent 1 (mA)", y=w257) -> (x/y=w258:dbl)
        n132 = Divide(x="SetCurrent 2 (mA)", y=w257) -> (x/y=w259:dbl)
        n133 = Build Array(w258, w259) -> (w256:dbl[])
        n134 = Not Equal?(x=w263, y=FALSE) -> (x != y?=w261:bool)
        n135 = case shown="True" w261 {
          tunnel: [w270 w294] -> w268
          tunnel: "Output\n (ADCMT)" -> [_ w293]
          tunnel: w267 -> [w270 w292]
          tunnel: w266 -> [w269 w291]
          tunnel: [w269 w290] -> w265
          tunnel: w264 -> [_ w286]
          tunnel: w256 -> [_ w272]
          frame False {
          }
          frame True {
            w279 = 1 ("index (col)")
            w280 = 0 ("disabled index (col)")
            n136 = call-dynamic "6240AData_execute.vi"("6240AData in"=w292, "SetCurrent (A)"=w272, "FileFormat"="%3.5f", "Output status"=w293, "ExecutionIndex"=w286, "error in (no error)"=w291) -> ("ActualVoltage (V)"=w271:dbl[], "ActualCurrent (A)"=w285:dbl[], "6240AData out"=w294:refnum<class "6240AData.lvclass">, "appended array"=w275:timestamp[], "SetCurrentArray"=w281:dbl[][], "ActualCurrentArray"=w288:dbl[][], "error out"=w290:errorcluster)  [unwired: 3 in]
            n137 = property on="ActualVoltage (V)" class="Arr (strict)"("Val(Sgnl)"=w271) -> ()  [unwired: 2 in, 2 out]
            n138 = property on="ActualCurrent (A)" class="Arr (strict)"("Val(Sgnl)"=w285) -> ()  [unwired: 2 in, 2 out]
            n139 = Index Array(array=w288, index (col) #1=w280, index (col) #2=w279) -> (element #1=w289:dbl[], element #2=w283:dbl[])  [unwired: 2 in]
            n140 = Index Array(array=w281, index (col) #1=w280, index (col) #2=w279) -> (element #1=w277:dbl[], element #2=w274:dbl[])  [unwired: 2 in]
            n141 = Bundle("appended array"=w275, "ActualCurrentArray"=w289) -> (w284:T18)  [unwired: 1 in]
            n142 = Bundle("appended array"=w275, "ActualCurrentArray"=w283) -> (w278:T18)  [unwired: 1 in]
            n143 = Bundle("appended array"=w275, "SetCurrentArray"=w277) -> (w276:T19)  [unwired: 1 in]
            n144 = Bundle("appended array"=w275, "SetCurrentArray"=w274) -> (w273:T19)  [unwired: 1 in]
            n145 = Build Array(w284, w278, w276, w273) -> (→"Graph 6":T20)
          }
        }
      }
      event "upper limit (mA)", "lower limit (mA)": Value Change {
        n146 = event-data() -> ()  [unwired: 1 in, 6 out]
        n147 = property on="SetCurrent 1 (mA)" class="DigNum (strict)"("Maximum"="upper limit (mA)", "Minimum"="lower limit (mA)") -> ()  [unwired: 2 in, 2 out]
        n148 = property on="SetCurrent 2 (mA)" class="DigNum (strict)"("Maximum"="upper limit (mA)", "Minimum"="lower limit (mA)") -> ()  [unwired: 2 in, 2 out]
      }
      event "Initialize": Value Change {
        w311 = FALSE
        n149 = event-data() -> ()  [unwired: 1 in, 6 out]
        n150 = local read "Initialized?"() -> (w299:bool)
        n151 = case shown="True" w299 {
          tunnel: w301 -> [w327 w331]
          tunnel: w300 -> [w326 w330]
          tunnel: [w327 w329] -> w298
          tunnel: [w326 w328] -> w297
          frame False {
          }
          frame True {
            n152 = call-dynamic "6240AData_terrminate.vi"("error in (no error)"=w330, "6240AData in"=w331) -> ("error out"=w328:errorcluster, "6240AData out"=w329:refnum<class "6240AData.lvclass">)  [unwired: 8 in]
          }
        }
        n153 = property on="Initialized?" class="Bool (strict)"("Val(Sgnl)"=TRUE ("Value (Signaling)")) -> ()  [unwired: 2 in, 2 out]
        n154 = local read "SetCurrent 2 (mA)"() -> (w304:dbl)
        n155 = local read "SetCurrent 1 (mA)"() -> (w307:dbl)
        n156 = local read "RUN Identifier"() -> (w319:string)
        n157 = local read "Base Path"() -> (w320:path)
        n158 = Divide(x=w307, y=1000.0) -> (x/y=w306:dbl)
        n159 = Divide(x=w304, y=1000.0) -> (x/y=w303:dbl)
        n160 = Get Date/Time In Seconds() -> ()  [unwired: 1 out]
        n161 = call-dynamic "6240AData_initialize.vi"("6240AData in"=w298, "RunIdentifier"=w319, "InstName"="InstName", "base path"=w320, "VISA"="VISA", "error in (no error)"=w297, "CtrlLabels"="CtrlLabels", "Voltage limits (V)"="Voltage limits (V)") -> ("6240AData out"=w318:refnum<class "6240AData.lvclass">, "error out"=w316:errorcluster)  [unwired: 6 in]
        n162 = Build Array(w306, w303) -> (w302:dbl[])
        n163 = Build Array(w311, w311) -> (w310:bool[])
        n164 = call-dynamic "6240AData_execute.vi"("6240AData in"=w318, "SetCurrent (A)"=w302, "FileFormat"="%3.5f", "Output status"=w310, "ExecutionIndex"=w309, "error in (no error)"=w316) -> ("ActualVoltage (V)"=w313:dbl[], "ActualCurrent (A)"=w312:dbl[], "6240AData out"=w317:refnum<class "6240AData.lvclass">, "error out"=w315:errorcluster)  [unwired: 3 in, 3 out]
        n165 = property on="ActualVoltage (V)" class="Arr (strict)"("Val(Sgnl)"=w313) -> ()  [unwired: 2 in, 2 out]
        n166 = property on="ActualCurrent (A)" class="Arr (strict)"("Val(Sgnl)"=w312) -> ()  [unwired: 2 in, 2 out]
      }
      event "Stop Button": Value Change {
        n167 = event-data() -> ()  [unwired: 1 in, 6 out]
        n168 = local read "Initialized?"() -> (w332:bool)
        n169 = case shown="False" w332 {
          tunnel: w336 -> [w341 w353]
          tunnel: [w341 w352] -> w335
          tunnel: w334 -> [w340 w351]
          tunnel: [w340 w350] -> w333
          frame False {
          }
          frame True {
            w357 = FALSE
            n170 = local read "SetCurrent 2 (mA)"() -> (w343:dbl)
            n171 = local read "SetCurrent 1 (mA)"() -> (w347:dbl)
            n172 = Divide(x=w347, y=1000.0) -> (x/y=w345:dbl)
            n173 = Divide(x=w343, y=1000.0) -> (x/y=w342:dbl)
            n174 = Build Array(w345, w342) -> (w349:dbl[])
            n175 = Build Array(w357, w357) -> (w348:bool[])
            n176 = property on="Output\n (ADCMT)" class="Arr (strict)"("Val(Sgnl)"=w348) -> ()  [unwired: 2 in, 2 out]
            n177 = call-dynamic "6240AData_execute.vi"("6240AData in"=w353, "SetCurrent (A)"=w349, "FileFormat"="%3.5f", "Output status"=w348, "error in (no error)"=w351) -> ("ActualVoltage (V)"=w354:dbl[], "ActualCurrent (A)"=w355:dbl[], "6240AData out"=w352:refnum<class "6240AData.lvclass">, "error out"=w350:errorcluster)  [unwired: 4 in, 3 out]
            n178 = property on="ActualVoltage (V)" class="Arr (strict)"("Val(Sgnl)"=w354) -> ()  [unwired: 2 in, 2 out]
            n179 = property on="ActualCurrent (A)" class="Arr (strict)"("Val(Sgnl)"=w355) -> ()  [unwired: 2 in, 2 out]
          }
        }
        n180 = call-dynamic "6240AData_terrminate.vi"("error in (no error)"=w333, "6240AData in"=w335) -> ("error out"=w337:errorcluster, "6240AData out"=w338:refnum<class "6240AData.lvclass">)  [unwired: 8 in]
      }
    }
    "error out (ADCMT6420A)" <- w246
  }
  n181 = while {
    stop <- w366 stop-if-true
    n182 = Get Date/Time In Seconds() -> (seconds since 1Jan1904=w365:timestamp)
    n183 = Format Date/Time String(time format string (%c)="%Y%m", seconds (now)=w365) -> (date/time string=w362:string)  [unwired: 1 in]
    n184 = Build Path(base path="Base Path (screenshots)", name or relative path=w362) -> (appended path=w361:path)
    n185 = Create Folder(path (use dialog)=w361, error in=errorcluster {"status"=FALSE, "code"=0, "source"=""}) -> (created path=w358:path, error out=→"error out (monthly folder creation)":errorcluster)  [unwired: 1 in, 1 out]
    n186 = event shown="[1] \"Frontpanel screenshots\": Value Change" {
      selector: _ -> [_ _ _]
      dyn-events: _ -> [_ _ _]
      timeout: _ -> [_ _ _]
      tunnel: [FALSE _ TRUE] -> w366
      tunnel: w358 -> [_ w374 _]
      tunnel: w365 -> [_ w373 _]
      event Timeout {
        n187 = event-data() -> ()  [unwired: 1 in, 3 out]
      }
      event "Frontpanel screenshots": Value Change {
        n188 = event-data() -> ()  [unwired: 1 in, 3 out]
        n189 = property class="TabCtl (strict)"() -> ("Value"=w371:T1)  [unwired: 2 in, 2 out]
        n190 = stacked-sequence {
          tunnel: w374 -> [w380 w402 w424 w446 w468 w490 w512 w534 _]
          tunnel: w373 -> [w379 w401 w423 w445 w467 w489 w511 w533 _]
          tunnel: [w377 _ _ _ _ _ _ _ _] -> w372
          tunnel: w371 -> [w376 _ _ _ _ _ _ _ _]
          tunnel: [w376 _ _ _ _ _ _ _ _] -> w370
          tunnel: "cryostatus_" ("string") -> [w375 w398 w420 w442 w464 w486 w508 w530 _]
          frame #0 {
            n191 = flat-sequence {
              tunnel: w379 -> [w382]
              tunnel: [w382] -> w378
              tunnel: w380 -> [w397]
              tunnel: w378 -> [w385]
              tunnel: [w384] -> w377
              tunnel: w375 -> [w383]
              frame #0 {
                n192 = property class="TabCtl (strict)"("Val(Sgnl)"=T1."NI USB CONFIG" ("Value (Signaling)")) -> ()  [unwired: 2 in, 2 out]
              }
              frame #1 {
                w395 = "_" ("string")
                n193 = local read "Cycle #"() -> (w393:u32)
                n194 = call "LV_UNIXTIME.vi"("current time"=w385) -> ("date/time string"=w396:string)  [unwired: 9 in, 1 out]
                n195 = Format Value(format string="%06d", value (0)=w393) -> (output string=w392:string)  [unwired: 1 in]
                n196 = Concatenate Strings(w383, w396, w395, w392, w395, "page1.png" ("string")) -> (w390:string)
                n197 = invoke class="TabCtl (strict)" method="Get Image"(error in=errorcluster {"status"=FALSE, "code"=0, "source"=""} ("error in (no error)")) -> (error out=w386:errorcluster, "image data"=w388:T21)  [unwired: 5 in, 4 out]
                n198 = Build Path(base path=w397, name or relative path=w390) -> (appended path=w389:path)
                n199 = call <vilib>:"Write PNG File.vi"("error in (no error)"=w386, "image data"=w388, "path to PNG file"=w389) -> ("error out"=w384:errorcluster)  [unwired: 7 in, 1 out]
              }
            }
          }
          frame #1 {
            n200 = flat-sequence {
              tunnel: w401 -> [w404]
              tunnel: [w404] -> w400
              tunnel: w402 -> [w419]
              tunnel: w400 -> [w407]
              tunnel: [w406] -> w399
              tunnel: w398 -> [w405]
              frame #0 {
                n201 = property class="TabCtl (strict)"("Val(Sgnl)"=T1."LSI CONFIG" ("Value (Signaling)")) -> ()  [unwired: 2 in, 2 out]
              }
              frame #1 {
                w417 = "_" ("string")
                n202 = local read "Cycle #"() -> (w415:u32)
                n203 = call "LV_UNIXTIME.vi"("current time"=w407) -> ("date/time string"=w418:string)  [unwired: 9 in, 1 out]
                n204 = Format Value(format string="%06d", value (0)=w415) -> (output string=w414:string)  [unwired: 1 in]
                n205 = Concatenate Strings(w405, w418, w417, w414, w417, "page2.png" ("string")) -> (w412:string)
                n206 = invoke class="TabCtl (strict)" method="Get Image"(error in=errorcluster {"status"=FALSE, "code"=0, "source"=""} ("error in (no error)")) -> (error out=w408:errorcluster, "image data"=w410:T21)  [unwired: 5 in, 4 out]
                n207 = Build Path(base path=w419, name or relative path=w412) -> (appended path=w411:path)
                n208 = call <vilib>:"Write PNG File.vi"("error in (no error)"=w408, "image data"=w410, "path to PNG file"=w411) -> ("error out"=w406:errorcluster)  [unwired: 7 in, 1 out]
              }
            }
            n209 = local write "error out (frontpanel screenshots)"(w399) -> ()
          }
          frame #2 {
            n210 = flat-sequence {
              tunnel: w423 -> [w426]
              tunnel: [w426] -> w422
              tunnel: w424 -> [w441]
              tunnel: w422 -> [w429]
              tunnel: [w428] -> w421
              tunnel: w420 -> [w427]
              frame #0 {
                n211 = property class="TabCtl (strict)"("Val(Sgnl)"=T1."MEASUREMENT" ("Value (Signaling)")) -> ()  [unwired: 2 in, 2 out]
              }
              frame #1 {
                w439 = "_" ("string")
                n212 = local read "Cycle #"() -> (w437:u32)
                n213 = Format Value(format string="%06d", value (0)=w437) -> (output string=w436:string)  [unwired: 1 in]
                n214 = call "LV_UNIXTIME.vi"("current time"=w429) -> ("date/time string"=w440:string)  [unwired: 9 in, 1 out]
                n215 = Concatenate Strings(w427, w440, w439, w436, w439, "page3.png" ("string")) -> (w434:string)
                n216 = invoke class="TabCtl (strict)" method="Get Image"(error in=errorcluster {"status"=FALSE, "code"=0, "source"=""} ("error in (no error)")) -> (error out=w430:errorcluster, "image data"=w432:T21)  [unwired: 5 in, 4 out]
                n217 = Build Path(base path=w441, name or relative path=w434) -> (appended path=w433:path)
                n218 = call <vilib>:"Write PNG File.vi"("error in (no error)"=w430, "image data"=w432, "path to PNG file"=w433) -> ("error out"=w428:errorcluster)  [unwired: 7 in, 1 out]
              }
            }
            n219 = local write "error out (frontpanel screenshots)"(w421) -> ()
          }
          frame #3 {
            n220 = flat-sequence {
              tunnel: w445 -> [w448]
              tunnel: [w448] -> w444
              tunnel: w446 -> [w463]
              tunnel: w444 -> [w451]
              tunnel: [w450] -> w443
              tunnel: w442 -> [w449]
              frame #0 {
                n221 = property class="TabCtl (strict)"("Val(Sgnl)"=T1."HE AUTO FILL" ("Value (Signaling)")) -> ()  [unwired: 2 in, 2 out]
              }
              frame #1 {
                w461 = "_" ("string")
                n222 = local read "Cycle #"() -> (w459:u32)
                n223 = Format Value(format string="%06d", value (0)=w459) -> (output string=w458:string)  [unwired: 1 in]
                n224 = call "LV_UNIXTIME.vi"("current time"=w451) -> ("date/time string"=w462:string)  [unwired: 9 in, 1 out]
                n225 = Concatenate Strings(w449, w462, w461, w458, w461, "page4.png" ("string")) -> (w456:string)
                n226 = invoke class="TabCtl (strict)" method="Get Image"(error in=errorcluster {"status"=FALSE, "code"=0, "source"=""} ("error in (no error)")) -> (error out=w452:errorcluster, "image data"=w454:T21)  [unwired: 5 in, 4 out]
                n227 = Build Path(base path=w463, name or relative path=w456) -> (appended path=w455:path)
                n228 = call <vilib>:"Write PNG File.vi"("error in (no error)"=w452, "image data"=w454, "path to PNG file"=w455) -> ("error out"=w450:errorcluster)  [unwired: 7 in, 1 out]
              }
            }
            n229 = local write "error out (frontpanel screenshots)"(w443) -> ()
          }
          frame #4 {
            n230 = flat-sequence {
              tunnel: w467 -> [w470]
              tunnel: [w470] -> w466
              tunnel: w468 -> [w485]
              tunnel: w466 -> [w473]
              tunnel: [w472] -> w465
              tunnel: w464 -> [w471]
              frame #0 {
                n231 = property class="TabCtl (strict)"("Val(Sgnl)"=T1."VALVE/HEATER CTRL" ("Value (Signaling)")) -> ()  [unwired: 2 in, 2 out]
              }
              frame #1 {
                w483 = "_" ("string")
                n232 = local read "Cycle #"() -> (w481:u32)
                n233 = call "LV_UNIXTIME.vi"("current time"=w473) -> ("date/time string"=w484:string)  [unwired: 9 in, 1 out]
                n234 = Format Value(format string="%06d", value (0)=w481) -> (output string=w480:string)  [unwired: 1 in]
                n235 = Concatenate Strings(w471, w484, w483, w480, w483, "page5.png" ("string")) -> (w478:string)
                n236 = invoke class="TabCtl (strict)" method="Get Image"(error in=errorcluster {"status"=FALSE, "code"=0, "source"=""} ("error in (no error)")) -> (error out=w474:errorcluster, "image data"=w476:T21)  [unwired: 5 in, 4 out]
                n237 = Build Path(base path=w485, name or relative path=w478) -> (appended path=w477:path)
                n238 = call <vilib>:"Write PNG File.vi"("error in (no error)"=w474, "image data"=w476, "path to PNG file"=w477) -> ("error out"=w472:errorcluster)  [unwired: 7 in, 1 out]
              }
            }
            n239 = local write "error out (frontpanel screenshots)"(w465) -> ()
          }
          frame #5 {
            n240 = flat-sequence {
              tunnel: w489 -> [w492]
              tunnel: [w492] -> w488
              tunnel: w490 -> [w507]
              tunnel: w488 -> [w495]
              tunnel: [w494] -> w487
              tunnel: w486 -> [w493]
              frame #0 {
                n241 = property class="TabCtl (strict)"("Val(Sgnl)"=T1."DMMs" ("Value (Signaling)")) -> ()  [unwired: 2 in, 2 out]
              }
              frame #1 {
                w505 = "_" ("string")
                n242 = local read "Cycle #"() -> (w503:u32)
                n243 = call "LV_UNIXTIME.vi"("current time"=w495) -> ("date/time string"=w506:string)  [unwired: 9 in, 1 out]
                n244 = Format Value(format string="%06d", value (0)=w503) -> (output string=w502:string)  [unwired: 1 in]
                n245 = Concatenate Strings(w493, w506, w505, w502, w505, "page6.png" ("string")) -> (w500:string)
                n246 = invoke class="TabCtl (strict)" method="Get Image"(error in=errorcluster {"status"=FALSE, "code"=0, "source"=""} ("error in (no error)")) -> (error out=w496:errorcluster, "image data"=w498:T21)  [unwired: 5 in, 4 out]
                n247 = Build Path(base path=w507, name or relative path=w500) -> (appended path=w499:path)
                n248 = call <vilib>:"Write PNG File.vi"("error in (no error)"=w496, "image data"=w498, "path to PNG file"=w499) -> ("error out"=w494:errorcluster)  [unwired: 7 in, 1 out]
              }
            }
            n249 = local write "error out (frontpanel screenshots)"(w487) -> ()
          }
          frame #6 {
            n250 = flat-sequence {
              tunnel: w511 -> [w514]
              tunnel: [w514] -> w510
              tunnel: w512 -> [w529]
              tunnel: w510 -> [w517]
              tunnel: [w516] -> w509
              tunnel: w508 -> [w515]
              frame #0 {
                n251 = property class="TabCtl (strict)"("Val(Sgnl)"=T1."DIAGRAM" ("Value (Signaling)")) -> ()  [unwired: 2 in, 2 out]
              }
              frame #1 {
                w527 = "_" ("string")
                n252 = local read "Cycle #"() -> (w525:u32)
                n253 = Format Value(format string="%06d", value (0)=w525) -> (output string=w524:string)  [unwired: 1 in]
                n254 = call "LV_UNIXTIME.vi"("current time"=w517) -> ("date/time string"=w528:string)  [unwired: 9 in, 1 out]
                n255 = Concatenate Strings(w515, w528, w527, w524, w527, "page7.png" ("string")) -> (w522:string)
                n256 = invoke class="TabCtl (strict)" method="Get Image"(error in=errorcluster {"status"=FALSE, "code"=0, "source"=""} ("error in (no error)")) -> (error out=w518:errorcluster, "image data"=w520:T21)  [unwired: 5 in, 4 out]
                n257 = Build Path(base path=w529, name or relative path=w522) -> (appended path=w521:path)
                n258 = call <vilib>:"Write PNG File.vi"("error in (no error)"=w518, "image data"=w520, "path to PNG file"=w521) -> ("error out"=w516:errorcluster)  [unwired: 7 in, 1 out]
              }
            }
            n259 = local write "error out (frontpanel screenshots)"(w509) -> ()
          }
          frame #7 {
            n260 = flat-sequence {
              tunnel: w533 -> [w536]
              tunnel: [w536] -> w532
              tunnel: w534 -> [w551]
              tunnel: w532 -> [w539]
              tunnel: [w538] -> w531
              tunnel: w530 -> [w537]
              frame #0 {
                n261 = property class="TabCtl (strict)"("Val(Sgnl)"=T1."(Plc. hld.)" ("Value (Signaling)")) -> ()  [unwired: 2 in, 2 out]
              }
              frame #1 {
                w549 = "_" ("string")
                n262 = local read "Cycle #"() -> (w547:u32)
                n263 = Format Value(format string="%06d", value (0)=w547) -> (output string=w546:string)  [unwired: 1 in]
                n264 = call "LV_UNIXTIME.vi"("current time"=w539) -> ("date/time string"=w550:string)  [unwired: 9 in, 1 out]
                n265 = Concatenate Strings(w537, w550, w549, w546, w549, "page8.png" ("string")) -> (w544:string)
                n266 = invoke class="TabCtl (strict)" method="Get Image"(error in=errorcluster {"status"=FALSE, "code"=0, "source"=""} ("error in (no error)")) -> (error out=w540:errorcluster, "image data"=w542:T21)  [unwired: 5 in, 4 out]
                n267 = Build Path(base path=w551, name or relative path=w544) -> (appended path=w543:path)
                n268 = call <vilib>:"Write PNG File.vi"("error in (no error)"=w540, "image data"=w542, "path to PNG file"=w543) -> ("error out"=w538:errorcluster)  [unwired: 7 in, 1 out]
              }
            }
            n269 = local write "error out (frontpanel screenshots)"(w531) -> ()
          }
          frame #8 {
            n270 = local write "Frontpanel screenshots"(FALSE ("Frontpanel screenshots")) -> ()
          }
        }
        "error out (frontpanel screenshots)" <- w372
        n271 = property class="TabCtl (strict)"("Val(Sgnl)"=w370) -> ()  [unwired: 2 in, 2 out]
      }
      event "Stop Button": Value Change {
        n272 = event-data() -> ()  [unwired: 1 in, 3 out]
      }
    }
    n273 = Wait (ms)(milliseconds to wait=u32 123) -> ()  [unwired: 1 out]
  }
  n274 = while {
    stop <- w558 stop-if-true
    n275 = event shown="[5] \"Plot selecter LSI218(1)     1      2     3     4\", \"Plot selecter LSI218(2)     1      2     3     4\", \"Plot selecter (USB6210)     1      2     3     4\", \"Plot selecter LSI336       1      2     3     4\", \"Plot selecter (USB6218)     1      2     3     4\": Value Change" {
      selector: _ -> [_ _ _ _ _ _ _ _ _ _ _]
      dyn-events: _ -> [_ _ _ _ _ _ _ _ _ _ _]
      timeout: _ -> [_ _ _ _ _ _ _ _ _ _ _]
      tunnel: [_ _ _ _ _ _ _ _ _ _ TRUE] -> w558
      tunnel: [errorcluster {"status"=FALSE, "code"=0, "source"=""} ("error out") w562 _ _ _ _ w692 w709 w726 w743 errorcluster {"status"=FALSE, "code"=0, "source"=""} ("error out")] -> w554
      event Timeout {
        n276 = event-data() -> ()  [unwired: 1 in, 3 out]
      }
      event "log/linear 1": Value Change {
        n277 = event-data() -> ()  [unwired: 1 in, 6 out]
        n278 = flat-sequence {
          tunnel: [w563] -> w562
          frame #0 {
            n279 = Boolean To (0,1)(Boolean="log/linear 1") -> (0, 1=w568:i16)
            n280 = control-ref of="Graph 1"() -> (w564:refnum<vi>)
            n281 = property class="XYGraph (strict)"(reference=w564, error in=errorcluster {"status"=FALSE, "code"=0, "source"=""} ("error in (no error)"), "YScale.Mapping Mode"=w568) -> (error out=w566:errorcluster)  [unwired: 1 out]
            n282 = control-ref of="error out (USB6210)"() -> (w567:refnum<vi>)
            n283 = property class="Clust (strict)"(reference=w567, "Val(Sgnl)"=w566) -> (error out=w563:errorcluster)  [unwired: 1 in, 1 out]
          }
        }
      }
      event "log/linear 2": Value Change {
        n284 = event-data() -> ()  [unwired: 1 in, 6 out]
        n285 = flat-sequence {
          frame #0 {
            n286 = Boolean To (0,1)(Boolean="log/linear 2") -> (0, 1=w574:i16)
            n287 = control-ref of="Graph 2"() -> (w572:refnum<vi>)
            n288 = property class="XYGraph (strict)"(reference=w572, error in=errorcluster {"status"=FALSE, "code"=0, "source"=""} ("error in (no error)"), "YScale.Mapping Mode"=w574) -> (error out=w573:errorcluster)  [unwired: 1 out]
            n289 = control-ref of="error out (USB6210)"() -> (w571:refnum<vi>)
            n290 = property class="Clust (strict)"(reference=w571, "Value"=w573) -> ()  [unwired: 1 in, 2 out]
          }
        }
      }
      event "log/linear 3": Value Change {
        n291 = event-data() -> ()  [unwired: 1 in, 6 out]
        n292 = flat-sequence {
          frame #0 {
            n293 = Boolean To (0,1)(Boolean="log/linear 3") -> (0, 1=w580:i16)
            n294 = control-ref of="Graph 3"() -> (w576:refnum<vi>)
            n295 = property class="XYGraph (strict)"(reference=w576, error in=errorcluster {"status"=FALSE, "code"=0, "source"=""} ("error in (no error)"), "YScale.Mapping Mode"=w580) -> (error out=w579:errorcluster)  [unwired: 1 out]
            n296 = control-ref of="error out (USB6210)"() -> (w578:refnum<vi>)
            n297 = property class="Clust (strict)"(reference=w578, "Value"=w579) -> ()  [unwired: 1 in, 2 out]
          }
        }
      }
      event "log/linear 4": Value Change {
        n298 = event-data() -> ()  [unwired: 1 in, 6 out]
        n299 = flat-sequence {
          frame #0 {
            n300 = Boolean To (0,1)(Boolean="log/linear 4") -> (0, 1=w586:i16)
            n301 = control-ref of="Graph 4"() -> (w582:refnum<vi>)
            n302 = property class="XYGraph (strict)"(reference=w582, error in=errorcluster {"status"=FALSE, "code"=0, "source"=""} ("error in (no error)"), "YScale.Mapping Mode"=w586) -> (error out=w585:errorcluster)  [unwired: 1 out]
            n303 = control-ref of="error out (USB6210)"() -> (w584:refnum<vi>)
            n304 = property class="Clust (strict)"(reference=w584, "Value"=w585) -> ()  [unwired: 1 in, 2 out]
          }
        }
      }
      event "Plot selecter LSI218(1)\n    1      2     3     4", "Plot selecter LSI218(2)\n    1      2     3     4", "Plot selecter (USB6210)\n    1      2     3     4", "Plot selecter LSI336 \n     1      2     3     4", "Plot selecter (USB6218)\n    1      2     3     4": Value Change {
        n305 = event-data() -> ()  [unwired: 1 in, 6 out]
        n306 = local read "All Labels (USB6210)"() -> (w604:string[])
        n307 = local read "All Labels (USB6218)"() -> (w593:string[])
        n308 = local read "Labels LSI218 (1)"() -> (w606:string[])
        n309 = local read "Labels LSI218 (2)"() -> (w607:string[])
        n310 = local read "Labels LSI336"() -> (w599:string[])
        n311 = call "BuildPlotLegends_LSI218.vi"("Plot selecter (2)\n    1      2     3     5"="Plot selecter LSI218(2)\n    1      2     3     4", "Plot selecter (1)\n    1      2     3     4"="Plot selecter LSI218(1)\n    1      2     3     4", "Labels (2)"=w607, "Labels (1)"=w606) -> ("Series 4"=w617:string[], "Series 3"=w615:string[], "Series 2"=w613:string[], "Series 1"=w611:string[])  [unwired: 4 in]
        n312 = call "BuildPlotLegends.vi"("Plot selecter \n    1      2     3     4"="Plot selecter (USB6210)\n    1      2     3     4", "AllLabels"=w604) -> ("Series 4"=w616:string[], "Series 3"=w614:string[], "Series 2"=w612:string[], "Series 1"=w610:string[])  [unwired: 6 in]
        n313 = call "BuildPlotLegends.vi"("Plot selecter \n    1      2     3     4"="Plot selecter LSI336 \n     1      2     3     4", "AllLabels"=w599) -> ("Series 4"=w594:string[], "Series 3"=w595:string[], "Series 2"=w596:string[], "Series 1"=w597:string[])  [unwired: 6 in]
        n314 = call "BuildPlotLegends.vi"("Plot selecter \n    1      2     3     4"="Plot selecter (USB6218)\n    1      2     3     4", "AllLabels"=w593) -> ("Series 4"=w589:string[], "Series 3"=w588:string[], "Series 2"=w590:string[], "Series 1"=w591:string[])  [unwired: 6 in]
        n315 = Build Array (concatenate)(w612, w613, w596, w590) -> (w601:string[])
        "Series 2" <- w601
        n316 = Build Array (concatenate)(w614, w615, w595, w588) -> (w602:string[])
        "Series 3" <- w602
        n317 = Build Array (concatenate)(w616, w617, w594, w589) -> (w603:string[])
        "Series 4" <- w603
        n318 = Build Array (concatenate)(w610, w611, w597, w591) -> (w600:string[])
        "Series 1" <- w600
        n319 = stacked-sequence {
          tunnel: [w627 _ _ _] -> w621
          tunnel: [_ w645 _ _] -> w622
          tunnel: [_ _ w662 _] -> w620
          tunnel: [_ _ _ w679] -> w619
          tunnel: w600 -> [w625 _ _ _]
          tunnel: w601 -> [_ w643 _ _]
          tunnel: w602 -> [_ _ w660 _]
          tunnel: w603 -> [_ _ _ w677]
          frame #0 {
            n320 = Array Size(array=w625) -> (size(s)=w629:i32)
            n321 = control-ref of="Graph 1"() -> (w623:refnum<vi>)
            n322 = property class="XYGraph (strict)"(reference=w623) -> ("LegNumRows"=w624:u32)  [unwired: 1 in, 2 out]
            n323 = for {
              N: w624 -> [_]
              tunnel: w623 -> [w638]
              shift-right: [w636] -> w628
              shift-left: errorcluster {"status"=FALSE, "code"=0, "source"=""} ("error in (no error)") -> [w637]
              i -> [w640]
              n324 = property class="XYGraph (strict)"(reference=w638, error in=w637, "Active Plot"=w640, "Plot.Plot Name"="") -> (error out=w636:errorcluster)  [unwired: 1 out]
            }
            n325 = for {
              N: w629 -> [_]
              tunnel: w623 -> [w634]
              shift-right: [w632] -> w627
              shift-left: w628 -> [w633]
              tunnel: w625 -> [w631] mode=indexing
              i -> [w635]
              n326 = property class="XYGraph (strict)"(reference=w634, error in=w633, "Active Plot"=w635, "Plot.Plot Name"=w631, "Plot.Visible?"=TRUE ("Plot.Visible")) -> (error out=w632:errorcluster)  [unwired: 1 out]
            }
          }
          frame #1 {
            n327 = Array Size(array=w643) -> (size(s)=w647:i32)
            n328 = control-ref of="Graph 2"() -> (w642:refnum<vi>)
            n329 = property class="XYGraph (strict)"(reference=w642) -> ("LegNumRows"=w641:u32)  [unwired: 1 in, 2 out]
            n330 = for {
              N: w641 -> [_]
              shift-right: [w654] -> w646
              shift-left: errorcluster {"status"=FALSE, "code"=0, "source"=""} ("error in (no error)") -> [w655]
              tunnel: w642 -> [w653]
              i -> [w657]
              n331 = property class="XYGraph (strict)"(reference=w653, error in=w655, "Active Plot"=w657, "Plot.Plot Name"="") -> (error out=w654:errorcluster)  [unwired: 1 out]
            }
            n332 = for {
              N: w647 -> [_]
              shift-right: [w650] -> w645
              shift-left: w646 -> [w651]
              tunnel: w643 -> [w649] mode=indexing
              tunnel: w642 -> [w648]
              i -> [w652]
              n333 = property class="XYGraph (strict)"(reference=w648, error in=w651, "Active Plot"=w652, "Plot.Plot Name"=w649) -> (error out=w650:errorcluster)  [unwired: 1 out]
            }
          }
          frame #2 {
            n334 = Array Size(array=w660) -> (size(s)=w664:i32)
            n335 = control-ref of="Graph 3"() -> (w658:refnum<vi>)
            n336 = property class="XYGraph (strict)"(reference=w658) -> ("LegNumRows"=w659:u32)  [unwired: 1 in, 2 out]
            n337 = for {
              N: w659 -> [_]
              tunnel: w658 -> [w672]
              shift-right: [w670] -> w663
              shift-left: errorcluster {"status"=FALSE, "code"=0, "source"=""} ("error in (no error)") -> [w671]
              i -> [w674]
              n338 = property class="XYGraph (strict)"(reference=w672, error in=w671, "Active Plot"=w674, "Plot.Plot Name"="") -> (error out=w670:errorcluster)  [unwired: 1 out]
            }
            n339 = for {
              N: w664 -> [_]
              tunnel: w658 -> [w668]
              shift-right: [w666] -> w662
              shift-left: w663 -> [w667]
              tunnel: w660 -> [w665] mode=indexing
              i -> [w669]
              n340 = property class="XYGraph (strict)"(reference=w668, error in=w667, "Active Plot"=w669, "Plot.Plot Name"=w665) -> (error out=w666:errorcluster)  [unwired: 1 out]
            }
          }
          frame #3 {
            n341 = Array Size(array=w677) -> (size(s)=w681:i32)
            n342 = control-ref of="Graph 4"() -> (w675:refnum<vi>)
            n343 = property class="XYGraph (strict)"(reference=w675) -> ("LegNumRows"=w676:u32)  [unwired: 1 in, 2 out]
            n344 = for {
              N: w676 -> [_]
              tunnel: w675 -> [w689]
              shift-right: [w687] -> w680
              shift-left: errorcluster {"status"=FALSE, "code"=0, "source"=""} ("error in (no error)") -> [w688]
              i -> [w691]
              n345 = property class="XYGraph (strict)"(reference=w689, error in=w688, "Active Plot"=w691, "Plot.Plot Name"="") -> (error out=w687:errorcluster)  [unwired: 1 out]
            }
            n346 = for {
              N: w681 -> [_]
              tunnel: w675 -> [w685]
              shift-right: [w683] -> w679
              shift-left: w680 -> [w684]
              tunnel: w677 -> [w682] mode=indexing
              i -> [w686]
              n347 = property class="XYGraph (strict)"(reference=w685, error in=w684, "Active Plot"=w686, "Plot.Plot Name"=w682) -> (error out=w683:errorcluster)  [unwired: 1 out]
            }
          }
        }
        n348 = Merge Errors(w621, w622, w620, w619) -> (→"Plot errors":errorcluster)
      }
      event "Take Screenshot! 1": Value Change {
        n349 = event-data() -> ()  [unwired: 1 in, 6 out]
        n350 = flat-sequence {
          tunnel: [w693] -> w692
          frame #0 {
            n351 = flat-sequence {
              tunnel: [w694] -> w693
              frame #0 {
                w703 = "_" ("string")
                n352 = Get Date/Time In Seconds() -> (seconds since 1Jan1904=w700:timestamp)
                n353 = local read "RUN Identifier"() -> (w705:string)
                n354 = call "LV_UNIXTIME.vi"("current time"=w700) -> ("date/time string"=w704:string)  [unwired: 9 in, 1 out]
                n355 = control-ref of="Graph 1"() -> (w699:refnum<vi>)
                n356 = Concatenate Strings(w705, w703, w704, w703, "FIle suffix 1", ".png" ("string")) -> (w707:string)
                n357 = local read "Base Path"() -> (w706:path)
                n358 = invoke class="XYGraph (strict)" method="Get Image"(reference=w699, error in=errorcluster {"status"=FALSE, "code"=0, "source"=""} ("error in (no error)")) -> (error out=w695:errorcluster, "image data"=w698:T21)  [unwired: 4 in, 4 out]
                n359 = Build Path(base path=w706, name or relative path=w707) -> (appended path=w697:path)
                n360 = call <vilib>:"Write PNG File.vi"("error in (no error)"=w695, "image data"=w698, "path to PNG file"=w697) -> ("error out"=w694:errorcluster)  [unwired: 7 in, 1 out]
              }
              frame #1 {
                n361 = local write "Take Screenshot! 1"(FALSE ("Take Screenshot! 1")) -> ()
              }
            }
          }
        }
      }
      event "Take Screenshot! 2": Value Change {
        n362 = event-data() -> ()  [unwired: 1 in, 6 out]
        n363 = flat-sequence {
          tunnel: [w710] -> w709
          frame #0 {
            n364 = flat-sequence {
              tunnel: [w716] -> w710
              frame #0 {
                w720 = "_" ("string")
                n365 = Get Date/Time In Seconds() -> (seconds since 1Jan1904=w717:timestamp)
                n366 = local read "RUN Identifier"() -> (w722:string)
                n367 = call "LV_UNIXTIME.vi"("current time"=w717) -> ("date/time string"=w721:string)  [unwired: 9 in, 1 out]
                n368 = control-ref of="Graph 2"() -> (w711:refnum<vi>)
                n369 = Concatenate Strings(w722, w720, w721, w720, "FIle suffix 2", ".png" ("string")) -> (w724:string)
                n370 = local read "Base Path"() -> (w723:path)
                n371 = invoke class="XYGraph (strict)" method="Get Image"(reference=w711, error in=errorcluster {"status"=FALSE, "code"=0, "source"=""} ("error in (no error)")) -> (error out=w715:errorcluster, "image data"=w713:T21)  [unwired: 4 in, 4 out]
                n372 = Build Path(base path=w723, name or relative path=w724) -> (appended path=w712:path)
                n373 = call <vilib>:"Write PNG File.vi"("error in (no error)"=w715, "image data"=w713, "path to PNG file"=w712) -> ("error out"=w716:errorcluster)  [unwired: 7 in, 1 out]
              }
              frame #1 {
                n374 = local write "Take Screenshot! 2"(FALSE ("Take Screenshot! 1")) -> ()
              }
            }
          }
        }
      }
      event "Take Screenshot! 3": Value Change {
        n375 = event-data() -> ()  [unwired: 1 in, 6 out]
        n376 = flat-sequence {
          tunnel: [w727] -> w726
          frame #0 {
            n377 = flat-sequence {
              tunnel: [w729] -> w727
              frame #0 {
                w737 = "_" ("string")
                n378 = Get Date/Time In Seconds() -> (seconds since 1Jan1904=w735:timestamp)
                n379 = local read "RUN Identifier"() -> (w739:string)
                n380 = call "LV_UNIXTIME.vi"("current time"=w735) -> ("date/time string"=w738:string)  [unwired: 9 in, 1 out]
                n381 = control-ref of="Graph 3"() -> (w732:refnum<vi>)
                n382 = Concatenate Strings(w739, w737, w738, w737, "FIle suffix 3", ".png" ("string")) -> (w741:string)
                n383 = local read "Base Path"() -> (w740:path)
                n384 = invoke class="XYGraph (strict)" method="Get Image"(reference=w732, error in=errorcluster {"status"=FALSE, "code"=0, "source"=""} ("error in (no error)")) -> (error out=w730:errorcluster, "image data"=w728:T21)  [unwired: 4 in, 4 out]
                n385 = Build Path(base path=w740, name or relative path=w741) -> (appended path=w733:path)
                n386 = call <vilib>:"Write PNG File.vi"("error in (no error)"=w730, "image data"=w728, "path to PNG file"=w733) -> ("error out"=w729:errorcluster)  [unwired: 7 in, 1 out]
              }
              frame #1 {
                n387 = local write "Take Screenshot! 3"(FALSE ("Take Screenshot! 1")) -> ()
              }
            }
          }
        }
      }
      event "Take Screenshot! 4": Value Change {
        n388 = event-data() -> ()  [unwired: 1 in, 6 out]
        n389 = flat-sequence {
          tunnel: [w744] -> w743
          frame #0 {
            n390 = flat-sequence {
              tunnel: [w747] -> w744
              frame #0 {
                w754 = "_" ("string")
                n391 = Get Date/Time In Seconds() -> (seconds since 1Jan1904=w752:timestamp)
                n392 = local read "RUN Identifier"() -> (w756:string)
                n393 = call "LV_UNIXTIME.vi"("current time"=w752) -> ("date/time string"=w755:string)  [unwired: 9 in, 1 out]
                n394 = control-ref of="Graph 4"() -> (w748:refnum<vi>)
                n395 = Concatenate Strings(w756, w754, w755, w754, "FIle suffix 4", ".png" ("string")) -> (w758:string)
                n396 = local read "Base Path"() -> (w757:path)
                n397 = invoke class="XYGraph (strict)" method="Get Image"(reference=w748, error in=errorcluster {"status"=FALSE, "code"=0, "source"=""} ("error in (no error)")) -> (error out=w745:errorcluster, "image data"=w749:T21)  [unwired: 4 in, 4 out]
                n398 = Build Path(base path=w757, name or relative path=w758) -> (appended path=w750:path)
                n399 = call <vilib>:"Write PNG File.vi"("error in (no error)"=w745, "image data"=w749, "path to PNG file"=w750) -> ("error out"=w747:errorcluster)  [unwired: 7 in, 1 out]
              }
              frame #1 {
                n400 = local write "Take Screenshot! 4"(FALSE ("Take Screenshot! 1")) -> ()
              }
            }
          }
        }
      }
      event "Stop Button": Value Change {
        n401 = event-data() -> ()  [unwired: 1 in, 6 out]
      }
    }
    "error out (graph operations)" <- w554
    n402 = local write "Take Screenshot! 1"(FALSE ("Take Screenshot! 1")) -> ()
    n403 = local write "Take Screenshot! 2"(FALSE ("Take Screenshot! 1")) -> ()
    n404 = Wait (ms)(milliseconds to wait=u32 1000) -> ()  [unwired: 1 out]
    n405 = local write "Take Screenshot! 3"(FALSE ("Take Screenshot! 1")) -> ()
    n406 = local write "Take Screenshot! 4"(FALSE ("Take Screenshot! 1")) -> ()
  }
  n407 = while {
    stop <- w762 stop-if-true
    n408 = Wait (ms)(milliseconds to wait=u32 101) -> ()  [unwired: 1 out]
    n409 = event shown="[1] \"Stop Button\": Value Change" {
      selector: _ -> [_ _ _]
      dyn-events: _ -> [_ _ _]
      timeout: _ -> [_ _ _]
      tunnel: [FALSE TRUE FALSE] -> w762
      event "Initialize (DMMs)": Value Change {
        w765 = T4 [] ("Value (Signaling)")
        n410 = event-data() -> ()  [unwired: 1 in, 3 out]
        n411 = property on="Graph DMMs 1" class="XYGraph (strict)"("Val(Sgnl)"=w765) -> ()  [unwired: 2 in, 2 out]
        n412 = property on="Graph DMMs 2" class="XYGraph (strict)"("Val(Sgnl)"=w765) -> ()  [unwired: 2 in, 2 out]
      }
      event "Stop Button": Value Change {
        n413 = event-data() -> ()  [unwired: 1 in, 3 out]
      }
      event Timeout {
        n414 = event-data() -> ()  [unwired: 1 in, 3 out]
      }
    }
  }
  n415 = Obtain Notifier(name (unnamed)="stop notifier", notification data type=w13, create if not found? (T)=w13, error in (no error)=errorcluster {"status"=FALSE, "code"=0, "source"=""}) -> (notifier out=w7:refnum<notifier>, error out=w6:errorcluster)  [unwired: 1 out]
  n416 = while {
    shift-right: [w866] -> w38
    shift-left: refnum<class "USBData.lvclass"> refnum ("USBData.lvclass") -> [w869]
    shift-right: [w862] -> w37
    shift-left: errorcluster {"status"=FALSE, "code"=0, "source"=""} ("error in (no error)") -> [w868]
    tunnel: "RUN label" -> [w774]
    tunnel: "Base Path" -> [w806]
    shift-right: [w844] -> w31
    shift-left: errorcluster {"status"=FALSE, "code"=0, "source"=""} ("error in (no error)") -> [w860]
    shift-right: [w845] -> w32
    shift-left: refnum<class "LSI218Data.lvclass"> refnum ("LSI218Data.lvclass") -> [w859]
    shift-right: [w832] -> w28
    shift-left: refnum<class "LSI336Data.lvclass"> refnum ("LSI336Data.lvclass") -> [w841]
    shift-right: [w831] -> w27
    shift-left: w17 -> [w840]
    shift-right: [w820] -> _
    shift-left: errorcluster {"status"=FALSE, "code"=0, "source"=""} ("error in") -> [w821]
    shift-right: [w810] -> w21
    shift-left: refnum<class "USBData.lvclass"> refnum ("USBData.lvclass") -> [w818]
    shift-right: [w809] -> w20
    shift-left: errorcluster {"status"=FALSE, "code"=0, "source"=""} ("error in (no error)") -> [w817]
    shift-right: [w805] -> _
    shift-left: w17 -> [w804]
    tunnel: w7 -> [w772]
    tunnel: w6 -> [w771]
    tunnel: [w769] -> w9
    tunnel: [w768] -> w8
    i -> [w781]
    stop <- "Stop Button" stop-if-true
    w827 = u32 24 ("Number of Rows")
    w837 = T23 [] ("appended array")
    w854 = T23 [] ("appended array")
    n417 = local read "LSI218Settings(A-F)"() -> (w796:T3)
    n418 = control-ref of="Plot selecter LSI218(2)\n    1      2     3     4"() -> (w825:refnum<vi>)
    n419 = control-ref of="Plot selecter LSI218(1)\n    1      2     3     4"() -> (w826:refnum<vi>)
    n420 = control-ref of="Plot selecter LSI336 \n     1      2     3     4"() -> (w824:refnum<vi>)
    n421 = property on="Property Node" class="Arr (strict)"(reference=w825, "Number of Rows"=w827) -> ()  [unwired: 1 in, 2 out]
    n422 = property on="Property Node" class="Arr (strict)"(reference=w826, "Number of Rows"=w827) -> ()  [unwired: 1 in, 2 out]
    n423 = local read "LSI336Settings(X,Y)"() -> (w794:T3)
    n424 = Array Size(array=w796) -> (size(s)=w795:i32)
    n425 = property on="Property Node" class="Arr (strict)"(reference=w824, "Number of Rows"=u32 8) -> ()  [unwired: 1 in, 2 out]
    n426 = Multiply(x="Measurement Interval (s)", y=u32 1000) -> (x*y=w863:dbl)
    n427 = Wait (ms)(milliseconds to wait=w863) -> ()  [unwired: 1 out]
    n428 = for {
      N: w795 -> [_]
      tunnel: w796 -> [w880] mode=indexing
      tunnel: [w879] -> w792 mode=concatenating
      n429 = Unbundle By Name(w880) -> ("SensorLocations"=w879:T16)
    }
    n430 = for {
      tunnel: w794 -> [w878] mode=indexing
      tunnel: [w877] -> w793 mode=concatenating
      n431 = Unbundle By Name(w878) -> ("SensorLocations"=w877:T16)
    }
    n432 = Quotient & Remainder(x=w781, y="Screenshots interval") -> (x-y*floor(x/y)=w779:i64)  [unwired: 1 out]
    n433 = Equal?(x=w781, y=0) -> (x = y?=w773:bool)
    n434 = case shown="True" w773 {
      tunnel: w869 -> [w1936 w1959]
      tunnel: w868 -> [w1930 w1957]
      tunnel: w781 -> [w1921 _]
      tunnel: [w1928 w1954] -> w862
      tunnel: [w1925 w1953] -> w819
      tunnel: [w1926 w1952] -> w866
      tunnel: [w1916 w1947] -> w867
      tunnel: w806 -> [_ w1946]
      tunnel: [w1915 w1943] -> w801
      frame False {
        n435 = call-dynamic "USBData_measure.vi"("USBData in"=w1936, "DAQ sample #"=i64 5, "DAQ timeout"=100.0 ("DAQ timeout (def: 100)"), "MeasurementIndex"=w1921, "error in (no error)"=w1930, "save every ... measurements"="Record interval") -> ("USBData out"=w1935:refnum<class "USBData.lvclass">, "TimeMeasuremeent"=w1932:timestamp, "Status"=→"USB6210 Status":T6, "LastDataAcquired"=w1917:dbl[], "error out"=w1931:errorcluster)  [unwired: 3 in, 2 out]
        "Time of Last Measurement (USB6210)" <- w1932
        "Last Vol\n(USB6210)" <- w1917
        n436 = call-dynamic "USBData_convert.vi"("Save every ... measurements"="Record interval", "MeasurementIndex"=w1921, "error in (no error)"=w1931, "LastDataAcquired"=w1917, "TimeMeasuremeent"=w1932, "USBData in"=w1935) -> ("error out"=w1929:errorcluster, "LeakDet_FULL"=w1924:dbl, "LastDataConverted"=w1918:dbl[], "USBData out"=w1927:refnum<class "USBData.lvclass">)  [unwired: 2 in]
        n437 = call "USBData_read.vi"("USBData in"=w1927, "error in (no error)"=w1929) -> ("Status"=w1919:T6, "USBData out"=w1926:refnum<class "USBData.lvclass">, "Data"=w1925:T24, "Basic"=w1916:T25, "error out"=w1928:errorcluster)  [unwired: 2 in, 2 out]
        n438 = local write "USB6210 Status"(w1919) -> ()
        n439 = Unbundle By Name(w1916) -> ("ReadLeakDet?"=w1923:bool)
        n440 = Unbundle By Name(w1916) -> ("Labels"=w1915:string[])
        n441 = case shown="False" w1923 {
          tunnel: w1918 -> [w1937 w1940]
          tunnel: w1924 -> [_ w1939]
          tunnel: [w1937 w1938] -> w1922
          frame False {
          }
          frame True {
            n442 = Build Array (concatenate)(w1940, w1939) -> (w1938:dbl[])
          }
        }
        "Last Data \n(USB6210)" <- w1922
      }
      frame True {
        n443 = local read "RUN Identifier"() -> (w1941:string)
        n444 = call-dynamic "USBData_initialize.vi"("USBData in"=w1959, "SeriesSetting"="USB6210 Config", "BasePath"=w1946, "RunIdentifier"=w1941, "FileName"="InstName (USB6210)", "error in (no error)"=w1957) -> ("Status"=w1942:T6, "USBData out"=w1955:refnum<class "USBData.lvclass">, "error out"=w1956:errorcluster)  [unwired: 5 in, 2 out]
        n445 = local write "USB6210 Status"(w1942) -> ()
        n446 = call "USBData_read.vi"("USBData in"=w1955, "error in (no error)"=w1956) -> ("Status"=w1945:T6, "USBData out"=w1952:refnum<class "USBData.lvclass">, "Data"=w1953:T24, "Basic"=w1947:T25, "error out"=w1954:errorcluster)  [unwired: 2 in, 2 out]
        n447 = local write "USB6210 Status"(w1945) -> ()
        n448 = Unbundle By Name(w1947) -> ("ReadLeakDet?"=w1951:bool, "Labels"=w1943:string[])
        n449 = Array Size(array=w1943) -> (size(s)=w1950:i32)
        n450 = case shown="True" w1951 {
          tunnel: w1950 -> [w1960 w1962]
          tunnel: [w1960 w1961] -> w1948
          frame False {
          }
          frame True {
            n451 = Add(x=w1962, y=1) -> (x+y=w1961:i32)
          }
        }
        n452 = Initialize Array(TRUE ("Activate 2"), w1948) -> ()  [unwired: 1 out]
      }
    }
    "error out (USB6210)" <- w862
    n453 = case shown="False" w773 {
      tunnel: [w1451 w1478] -> w809
      tunnel: [w1448 w1477] -> w816
      tunnel: [w1449 w1476] -> w810
      tunnel: [w1440 w1471] -> w815
      tunnel: [w1439 w1469] -> _
      tunnel: w818 -> [w1438 w1467]
      tunnel: w806 -> [_ w1466]
      tunnel: w817 -> [w1437 w1465]
      tunnel: w781 -> [w1436 _]
      frame False {
        n454 = local read "Record interval"() -> (w1435:i64)
        n455 = call-dynamic "USBData_measure.vi"("USBData in"=w1438, "DAQ sample #"=i64 5, "DAQ timeout"=100.0 ("DAQ timeout (def: 100)"), "MeasurementIndex"=w1436, "error in (no error)"=w1437, "save every ... measurements"=w1435) -> ("USBData out"=w1457:refnum<class "USBData.lvclass">, "TimeMeasuremeent"=w1454:timestamp, "Status"=→"USB6218 Status":T6, "LastDataAcquired"=w1441:dbl[], "error out"=w1453:errorcluster)  [unwired: 3 in, 2 out]
        "Time of Last Measurement (USB6218)" <- w1454
        "Last Vol \n(USB6218)" <- w1441
        n456 = call-dynamic "USBData_convert.vi"("Save every ... measurements"=w1435, "MeasurementIndex"=w1436, "error in (no error)"=w1453, "LastDataAcquired"=w1441, "TimeMeasuremeent"=w1454, "USBData in"=w1457) -> ("error out"=w1452:errorcluster, "LeakDet_FULL"=w1447:dbl, "LastDataConverted"=w1442:dbl[], "USBData out"=w1450:refnum<class "USBData.lvclass">)  [unwired: 2 in]
        n457 = call "USBData_read.vi"("USBData in"=w1450, "error in (no error)"=w1452) -> ("Status"=w1443:T6, "USBData out"=w1449:refnum<class "USBData.lvclass">, "Data"=w1448:T24, "Basic"=w1440:T25, "error out"=w1451:errorcluster)  [unwired: 2 in, 2 out]
        n458 = local write "USB6218 Status"(w1443) -> ()
        n459 = Unbundle By Name(w1440) -> ("ReadLeakDet?"=w1446:bool)
        n460 = Unbundle By Name(w1440) -> ("Labels"=w1439:string[])
        n461 = case shown="True" w1446 {
          tunnel: w1442 -> [w1458 w1461]
          tunnel: w1447 -> [_ w1460]
          tunnel: [w1458 w1459] -> w1445
          frame False {
          }
          frame True {
            n462 = Build Array (concatenate)(w1461, w1460) -> (w1459:dbl[])
          }
        }
        "Last Data \n(USB6218)" <- w1445
      }
      frame True {
        n463 = local read "RUN Identifier"() -> (w1462:string)
        n464 = call-dynamic "USBData_initialize.vi"("USBData in"=w1467, "SeriesSetting"="USB6218 Config", "BasePath"=w1466, "RunIdentifier"=w1462, "FileName"="InstName (USB6218)", "error in (no error)"=w1465) -> ("Status"=w1463:T6, "USBData out"=w1479:refnum<class "USBData.lvclass">, "error out"=w1480:errorcluster)  [unwired: 5 in, 2 out]
        n465 = local write "USB6218 Status"(w1463) -> ()
        n466 = call "USBData_read.vi"("USBData in"=w1479, "error in (no error)"=w1480) -> ("Status"=w1470:T6, "USBData out"=w1476:refnum<class "USBData.lvclass">, "Data"=w1477:T24, "Basic"=w1471:T25, "error out"=w1478:errorcluster)  [unwired: 2 in, 2 out]
        n467 = local write "USB6218 Status"(w1470) -> ()
        n468 = Unbundle By Name(w1471) -> ("ReadLeakDet?"=w1475:bool, "Labels"=w1469:string[])
        n469 = Array Size(array=w1469) -> (size(s)=w1474:i32)
        n470 = case shown="True" w1475 {
          tunnel: w1474 -> [w1481 w1483]
          tunnel: [w1481 w1482] -> w1472
          frame False {
          }
          frame True {
            n471 = Add(x=w1483, y=1) -> (x+y=w1482:i32)
          }
        }
        n472 = Initialize Array(TRUE ("Activate 2"), w1472) -> ()  [unwired: 1 out]
      }
    }
    "error out (USB6218)" <- w809
    n473 = case shown="True" w773 {
      tunnel: w774 -> [_ w872]
      frame False {
      }
      frame True {
        n474 = Get Date/Time In Seconds() -> (seconds since 1Jan1904=w875:timestamp)
        n475 = call "LV_UNIXTIME.vi"("current time"=w875) -> ("date/time string"=w874:string)  [unwired: 9 in, 1 out]
        n476 = Concatenate Strings(w874, "_" ("string"), w872) -> (→"RUN Identifier" →"RUN Identifier 2" →"RUN Identifier 3" →"RUN Identifier 4" →"RUN Identifier 5" →"RUN Identifier 6" →"RUN Identifier 7":string)
      }
    }
    n477 = Equal?(x=w779, y=i64 0) -> (x = y?=w776:bool)
    n478 = local read "LastData (LSI218)"() -> (w790:dbl[])
    n479 = local read "Last Data \nLSI336"() -> (w789:dbl[])
    n480 = And(x="Analog Out ON?", y=w773) -> (x .and. y?=w807:bool)
    n481 = case shown="True" w807 {
      tunnel: w806 -> [_ w1254]
      tunnel: [w1230 w1245] -> w805
      tunnel: w804 -> [w1230 w1244]
      frame False {
      }
      frame True {
        w1237 = "_raw" ("string")
        w1261 = 10.0 ("V_lim_max")
        w1260 = 0.0 ("V_lim_min")
        w1259 = -1 items=["Default"=-1, "RSE"=10083, "Differential"=10106, "Pseudodifferential"=12529] ("output terminal configuration")
        w1258 = 10348 items=["Volts"=10348, "From Custom Scale"=10065] ("units")
        n482 = local read "RUN Identifier"() -> (w1243:string)
        n483 = Concatenate Strings(w1243, "_AO" ("string")) -> (w1263:string)
        n484 = Concatenate Strings(w1243, "_", "USB_AOUT.csv" ("string")) -> (w1255:string)
        n485 = Array To Cluster(array="AOUT Labels") -> (cluster=w1241:T26)
        n486 = Unbundle By Name(w1241) -> ("AOUT Labels[0]"=w1240:string, "AOUT Labels[1]"=w1238:string)
        n487 = Build Path(base path=w1254, name or relative path=w1255) -> (appended path=w1251:path)
        n488 = Concatenate Strings(w1240, w1237) -> (w1239:string)
        n489 = Concatenate Strings(w1238, w1237) -> (w1236:string)
        n490 = Open/Create/Replace File(file path (use dialog)=w1251, operation (0:open)=T22."open or create") -> (refnum out=w1249:refnum<file>)  [unwired: 4 in, 2 out]
        n491 = Build Array(w1240, w1238, w1239, w1236) -> (w1247:string[])
        n492 = call "FileIntialize.vi"("Error In"=w1244, "Labels"=w1247, "refnum in"=w1249) -> ("Error Out"=w1246:errorcluster, "File Refnum"=→"File Refn USB AO":refnum<file>)  [unwired: 7 in]
        n493 = call <vilib>:"DAQmx Create Task.vi"("new task name"=w1263, "auto cleanup"=FALSE, "error in"=w1246) -> ("task out"=w1262:refnum<k21>, "error out"=w1264:errorcluster)  [unwired: 11 in]
        n494 = Index Array(array="AOUT assignment", index #1=0 ("index"), index #2=1 ("index")) -> (element #1=w1233:tag, element #2=w1231:tag)
        n495 = call-poly <vilib>:"DAQmx Create Virtual Channel.vi"("task in"=w1262, "maximum value"=w1261, "minimum value"=w1260, "output terminal configuration"=w1259, "physical channels"=w1233, "units"=w1258, "error in"=w1264) -> ("task out"=w1266:refnum<k21>, "error out"=w1267:errorcluster)  [unwired: 7 in]
        n496 = call-poly <vilib>:"DAQmx Create Virtual Channel.vi"("task in"=w1266, "maximum value"=w1261, "minimum value"=w1260, "physical channels"=w1231, "error in"=w1267) -> ("task out"=w1269:refnum<k21>, "error out"=w1268:errorcluster)  [unwired: 9 in]
        n497 = call <vilib>:"DAQmx Start Task.vi"("task/channels in"=w1269, "error in"=w1268) -> ("task out"=→"AO task out":refnum<k21>, "error out"=w1245:errorcluster)  [unwired: 12 in]
      }
    }
    "error out (USB6210/6218 AOUT)" <- w805
    n498 = And(x=w776, y="Automatic \nScreenshots?") -> (x .and. y?=w775:bool)
    n499 = Build Array (concatenate)(w790, w789) -> (w788:dbl[])
    "AllTemperatures" <- w788
    n500 = Build Array (concatenate)(w792, w793) -> (w791:T16)
    "TempSensorsLocations" <- w791
    n501 = case shown="True" w775 {
      frame False {
      }
      frame True {
        n502 = flat-sequence {
          frame #0 {
            n503 = property on="Frontpanel screenshots" class="Bool (strict)"("Val(Sgnl)"=TRUE ("Value (Signaling)")) -> ()  [unwired: 2 in, 2 out]
          }
        }
      }
    }
    n504 = flat-sequence {
      tunnel: w788 -> [w881]
      tunnel: w791 -> [w882]
      tunnel: w783 -> [w1134]
      tunnel: w782 -> [w1133]
      frame #0 {
        n505 = stacked-sequence {
          tunnel: w882 -> [w887 w892 w897 w902 w907 w912 w917 w922 w927 w932 w937 w942 w947 w952 w957 w962 w967 w972 w977 w982 w987 w992 w997 w1002 w1007 w1012 w1017 w1022 w1027 w1032 w1037 w1042 w1047 w1052 w1057 w1062 w1067 w1072 w1077 w1082 w1087 w1092 w1097 w1102 w1107 w1112 w1117 w1122 w1127 w1132]
          tunnel: w881 -> [w885 w890 w895 w900 w905 w910 w915 w920 w925 w930 w935 w940 w945 w950 w955 w960 w965 w970 w975 w980 w985 w990 w995 w1000 w1005 w1010 w1015 w1020 w1025 w1030 w1035 w1040 w1045 w1050 w1055 w1060 w1065 w1070 w1075 w1080 w1085 w1090 w1095 w1100 w1105 w1110 w1115 w1120 w1125 w1130]
          frame #0 {
            n506 = Search 1D Array(1D array=w887, element=T14."T3He1-1" ("SensorLocations")) -> (index of element=w884:i32)  [unwired: 1 in]
            n507 = Index Array(array=w885, index=w884) -> (element=→"T3He1-1":dbl)
          }
          frame #1 {
            n508 = Search 1D Array(1D array=w892, element=T14."T3He1-2" ("SensorLocations")) -> (index of element=w889:i32)  [unwired: 1 in]
            n509 = Index Array(array=w890, index=w889) -> (element=→"T3He1-2":dbl)
          }
          frame #2 {
            n510 = Search 1D Array(1D array=w897, element=T14."T3He1-3" ("SensorLocations")) -> (index of element=w894:i32)  [unwired: 1 in]
            n511 = Index Array(array=w895, index=w894) -> (element=→"T3He1-3":dbl)
          }
          frame #3 {
            n512 = Search 1D Array(1D array=w902, element=T14."T3He1-4" ("SensorLocations")) -> (index of element=w899:i32)  [unwired: 1 in]
            n513 = Index Array(array=w900, index=w899) -> (element=→"T3He1-4":dbl)
          }
          frame #4 {
            n514 = Search 1D Array(1D array=w907, element=T14."T3He2-1" ("SensorLocations")) -> (index of element=w904:i32)  [unwired: 1 in]
            n515 = Index Array(array=w905, index=w904) -> (element=→"T3He2-1":dbl)
          }
          frame #5 {
            n516 = Search 1D Array(1D array=w912, element=T14."T3He2-2" ("SensorLocations")) -> (index of element=w909:i32)  [unwired: 1 in]
            n517 = Index Array(array=w910, index=w909) -> (element=→"T3He2-2":dbl)
          }
          frame #6 {
            n518 = Search 1D Array(1D array=w917, element=T14."T3He3" ("SensorLocations")) -> (index of element=w914:i32)  [unwired: 1 in]
            n519 = Index Array(array=w915, index=w914) -> (element=→"T3He3":dbl)
          }
          frame #7 {
            n520 = Search 1D Array(1D array=w922, element=T14."T3He4" ("SensorLocations")) -> (index of element=w919:i32)  [unwired: 1 in]
            n521 = Index Array(array=w920, index=w919) -> (element=→"T3He4":dbl)
          }
          frame #8 {
            n522 = Search 1D Array(1D array=w927, element=T14."T3He5" ("SensorLocations")) -> (index of element=w924:i32)  [unwired: 1 in]
            n523 = Index Array(array=w925, index=w924) -> (element=→"T3He5":dbl)
          }
          frame #9 {
            n524 = Search 1D Array(1D array=w932, element=T14."T3He6-1" ("SensorLocations")) -> (index of element=w929:i32)  [unwired: 1 in]
            n525 = Index Array(array=w930, index=w929) -> (element=→"T3He6-1" →"T3He6-1/6-2 (HEX1)":dbl)
          }
          frame #10 {
            n526 = Search 1D Array(1D array=w937, element=T14."T3He6-2" ("SensorLocations")) -> (index of element=w934:i32)  [unwired: 1 in]
            n527 = Index Array(array=w935, index=w934) -> (element=→"T3He6-2" →"T3He6-1/6-2 (3He pot) 2":dbl)
          }
          frame #11 {
            n528 = Search 1D Array(1D array=w942, element=T14."T3He7-1" ("SensorLocations")) -> (index of element=w939:i32)  [unwired: 1 in]
            n529 = Index Array(array=w940, index=w939) -> (element=→"T3He7-1" →"T3He7-1/7-2 (HEX1)":dbl)
          }
          frame #12 {
            n530 = Search 1D Array(1D array=w947, element=T14."T3He7-2" ("SensorLocations")) -> (index of element=w944:i32)  [unwired: 1 in]
            n531 = Index Array(array=w945, index=w944) -> (element=→"T3He7-2" →"T3He7-1/6-2 (3He pot) 2":dbl)
          }
          frame #13 {
            n532 = Search 1D Array(1D array=w952, element=T14."T3He8" ("SensorLocations")) -> (index of element=w949:i32)  [unwired: 1 in]
            n533 = Index Array(array=w950, index=w949) -> (element=→"T3He8":dbl)
          }
          frame #14 {
            n534 = Search 1D Array(1D array=w957, element=T14."T3He9" ("SensorLocations")) -> (index of element=w954:i32)  [unwired: 1 in]
            n535 = Index Array(array=w955, index=w954) -> (element=→"T3He9":dbl)
          }
          frame #15 {
            n536 = Search 1D Array(1D array=w962, element=T14."T3He10" ("SensorLocations")) -> (index of element=w959:i32)  [unwired: 1 in]
            n537 = Index Array(array=w960, index=w959) -> (element=→"T3He10":dbl)
          }
          frame #16 {
            n538 = Search 1D Array(1D array=w967, element=T14."T4He1" ("SensorLocations")) -> (index of element=w964:i32)  [unwired: 1 in]
            n539 = Index Array(array=w965, index=w964) -> (element=→"T4He1" →"T4He1 (4K reservoir )":dbl)
          }
          frame #17 {
            n540 = Search 1D Array(1D array=w972, element=T14."T4He2-1" ("SensorLocations")) -> (index of element=w969:i32)  [unwired: 1 in]
            n541 = Index Array(array=w970, index=w969) -> (element=→"T4He2-1":dbl)
          }
          frame #18 {
            n542 = Search 1D Array(1D array=w977, element=T14."T4He2-2" ("SensorLocations")) -> (index of element=w974:i32)  [unwired: 1 in]
            n543 = Index Array(array=w975, index=w974) -> (element=→"T4He2-2":dbl)
          }
          frame #19 {
            n544 = Search 1D Array(1D array=w982, element=T14."T4He3-1" ("SensorLocations")) -> (index of element=w979:i32)  [unwired: 1 in]
            n545 = Index Array(array=w980, index=w979) -> (element=→"T4He3-1":dbl)
          }
          frame #20 {
            n546 = Search 1D Array(1D array=w987, element=T14."T4He3-2" ("SensorLocations")) -> (index of element=w984:i32)  [unwired: 1 in]
            n547 = Index Array(array=w985, index=w984) -> (element=→"T4He3-2":dbl)
          }
          frame #21 {
            n548 = Search 1D Array(1D array=w992, element=T14."T4He3-3" ("SensorLocations")) -> (index of element=w989:i32)  [unwired: 1 in]
            n549 = Index Array(array=w990, index=w989) -> (element=→"T4He3-3":dbl)
          }
          frame #22 {
            n550 = Search 1D Array(1D array=w997, element=T14."T4He3-4" ("SensorLocations")) -> (index of element=w994:i32)  [unwired: 1 in]
            n551 = Index Array(array=w995, index=w994) -> (element=→"T4He3-4":dbl)
          }
          frame #23 {
            n552 = Search 1D Array(1D array=w1002, element=T14."T4He4" ("SensorLocations")) -> (index of element=w999:i32)  [unwired: 1 in]
            n553 = Index Array(array=w1000, index=w999) -> (element=→"T4He4":dbl)
          }
          frame #24 {
            n554 = Search 1D Array(1D array=w1007, element=T14."T4He5" ("SensorLocations")) -> (index of element=w1004:i32)  [unwired: 1 in]
            n555 = Index Array(array=w1005, index=w1004) -> (element=→"T4He5":dbl)
          }
          frame #25 {
            n556 = Search 1D Array(1D array=w1012, element=T14."T4He6" ("SensorLocations")) -> (index of element=w1009:i32)  [unwired: 1 in]
            n557 = Index Array(array=w1010, index=w1009) -> (element=→"T4He6":dbl)
          }
          frame #26 {
            n558 = Search 1D Array(1D array=w1017, element=T14."T4He7" ("SensorLocations")) -> (index of element=w1014:i32)  [unwired: 1 in]
            n559 = Index Array(array=w1015, index=w1014) -> (element=→"T4He7":dbl)
          }
          frame #27 {
            n560 = Search 1D Array(1D array=w1022, element=T14."T4He8" ("SensorLocations")) -> (index of element=w1019:i32)  [unwired: 1 in]
            n561 = Index Array(array=w1020, index=w1019) -> (element=→"T4He8":dbl)
          }
          frame #28 {
            n562 = Search 1D Array(1D array=w1027, element=T14."T4He9" ("SensorLocations")) -> (index of element=w1024:i32)  [unwired: 1 in]
            n563 = Index Array(array=w1025, index=w1024) -> (element=→"T4He9":dbl)
          }
          frame #29 {
            n564 = Search 1D Array(1D array=w1032, element=T14."T4He10" ("SensorLocations")) -> (index of element=w1029:i32)  [unwired: 1 in]
            n565 = Index Array(array=w1030, index=w1029) -> (element=→"T4He10":dbl)
          }
          frame #30 {
            n566 = Search 1D Array(1D array=w1037, element=T14."T1K1" ("SensorLocations")) -> (index of element=w1034:i32)  [unwired: 1 in]
            n567 = Index Array(array=w1035, index=w1034) -> (element=→"T1K1":dbl)
          }
          frame #31 {
            n568 = Search 1D Array(1D array=w1042, element=T14."T1K2" ("SensorLocations")) -> (index of element=w1039:i32)  [unwired: 1 in]
            n569 = Index Array(array=w1040, index=w1039) -> (element=→"T1K2":dbl)
          }
          frame #32 {
            n570 = Search 1D Array(1D array=w1047, element=T14."T1K3-1" ("SensorLocations")) -> (index of element=w1044:i32)  [unwired: 1 in]
            n571 = Index Array(array=w1045, index=w1044) -> (element=→"T1K3-1" →"T1K3-1/3-2 (1K pot)":dbl)
          }
          frame #33 {
            n572 = Search 1D Array(1D array=w1052, element=T14."T1K3-2" ("SensorLocations")) -> (index of element=w1049:i32)  [unwired: 1 in]
            n573 = Index Array(array=w1050, index=w1049) -> (element=→"T1K3-2" →"T1K3-1/3-2 (1K pot) 2":dbl)
          }
          frame #34 {
            n574 = Search 1D Array(1D array=w1057, element=T14."T1K4" ("SensorLocations")) -> (index of element=w1054:i32)  [unwired: 1 in]
            n575 = Index Array(array=w1055, index=w1054) -> (element=→"T1K4":dbl)
          }
          frame #35 {
            n576 = Search 1D Array(1D array=w1062, element=T14."T1K5" ("SensorLocations")) -> (index of element=w1059:i32)  [unwired: 1 in]
            n577 = Index Array(array=w1060, index=w1059) -> (element=→"T1K5":dbl)
          }
          frame #36 {
            n578 = Search 1D Array(1D array=w1067, element=T14."T1K6" ("SensorLocations")) -> (index of element=w1064:i32)  [unwired: 1 in]
            n579 = Index Array(array=w1065, index=w1064) -> (element=→"T1K6":dbl)
          }
          frame #37 {
            n580 = Search 1D Array(1D array=w1072, element=T14."TIP1" ("SensorLocations")) -> (index of element=w1069:i32)  [unwired: 1 in]
            n581 = Index Array(array=w1070, index=w1069) -> (element=→"TIP1":dbl)
          }
          frame #38 {
            n582 = Search 1D Array(1D array=w1077, element=T14."TIP2" ("SensorLocations")) -> (index of element=w1074:i32)  [unwired: 1 in]
            n583 = Index Array(array=w1075, index=w1074) -> (element=→"TIP2":dbl)
          }
          frame #39 {
            n584 = Search 1D Array(1D array=w1082, element=T14."TIP3" ("SensorLocations")) -> (index of element=w1079:i32)  [unwired: 1 in]
            n585 = Index Array(array=w1080, index=w1079) -> (element=→"TIP3":dbl)
          }
          frame #40 {
            n586 = Search 1D Array(1D array=w1087, element=T14."TIP4" ("SensorLocations")) -> (index of element=w1084:i32)  [unwired: 1 in]
            n587 = Index Array(array=w1085, index=w1084) -> (element=→"TIP4":dbl)
          }
          frame #41 {
            n588 = Search 1D Array(1D array=w1092, element=T14."TIP5" ("SensorLocations")) -> (index of element=w1089:i32)  [unwired: 1 in]
            n589 = Index Array(array=w1090, index=w1089) -> (element=→"TIP5":dbl)
          }
          frame #42 {
            n590 = Search 1D Array(1D array=w1097, element=T14."TIP6" ("SensorLocations")) -> (index of element=w1094:i32)  [unwired: 1 in]
            n591 = Index Array(array=w1095, index=w1094) -> (element=→"TIP6":dbl)
          }
          frame #43 {
            n592 = Search 1D Array(1D array=w1102, element=T14."TIP7" ("SensorLocations")) -> (index of element=w1099:i32)  [unwired: 1 in]
            n593 = Index Array(array=w1100, index=w1099) -> (element=→"TIP7":dbl)
          }
          frame #44 {
            n594 = Search 1D Array(1D array=w1107, element=T14."TTH1" ("SensorLocations")) -> (index of element=w1104:i32)  [unwired: 1 in]
            n595 = Index Array(array=w1105, index=w1104) -> (element=→"TTH1":dbl)
          }
          frame #45 {
            n596 = Search 1D Array(1D array=w1112, element=T14."TTH2" ("SensorLocations")) -> (index of element=w1109:i32)  [unwired: 1 in]
            n597 = Index Array(array=w1110, index=w1109) -> (element=→"TTH2":dbl)
          }
          frame #46 {
            n598 = Search 1D Array(1D array=w1117, element=T14."TTH3" ("SensorLocations")) -> (index of element=w1114:i32)  [unwired: 1 in]
            n599 = Index Array(array=w1115, index=w1114) -> (element=→"TTH3":dbl)
          }
          frame #47 {
            n600 = Search 1D Array(1D array=w1122, element=T14."TTH4" ("SensorLocations")) -> (index of element=w1119:i32)  [unwired: 1 in]
            n601 = Index Array(array=w1120, index=w1119) -> (element=→"TTH4":dbl)
          }
          frame #48 {
            n602 = Search 1D Array(1D array=w1127, element="SensorLocation 1") -> (index of element=w1124:i32)  [unwired: 1 in]
            n603 = Index Array(array=w1125, index=w1124) -> (element=→"Temperature 1":dbl)
          }
          frame #49 {
            n604 = Search 1D Array(1D array=w1132, element="SensorLocation 2") -> (index of element=w1129:i32)  [unwired: 1 in]
            n605 = Index Array(array=w1130, index=w1129) -> (element=→"Temperature 2":dbl)
          }
        }
      }
      frame #1 {
        n606 = stacked-sequence {
          tunnel: w1134 -> [w1139 w1144 w1149 w1154 w1159 w1164 w1169 w1174 w1179 w1184 w1189 w1194 w1199 w1204 w1209 w1214 w1219 w1224 w1229]
          tunnel: w1133 -> [w1136 w1142 w1148 w1153 w1158 w1162 w1167 w1172 w1177 w1182 w1187 w1192 w1196 w1201 w1206 w1211 w1216 w1221 w1226]
          frame #0 {
            n607 = Search 1D Array(1D array=w1139, element="Insulation vacuum") -> (index of element=w1137:i32)  [unwired: 1 in]
            n608 = Index Array(array=w1136, index=w1137) -> (element=→"P_ins" →"P (insulation)":dbl)
          }
          frame #1 {
            n609 = Search 1D Array(1D array=w1144, element="4K reservoir pressure") -> (index of element=w1141:i32)  [unwired: 1 in]
            n610 = Index Array(array=w1142, index=w1141) -> (element=→"P_4Kres" →"P (4K reservoir)":dbl)
          }
          frame #2 {
            n611 = Search 1D Array(1D array=w1149, element="3He inlet pressure") -> (index of element=w1147:i32)  [unwired: 1 in]
            n612 = Index Array(array=w1148, index=w1147) -> (element=→"P_3HeIN" →"P (3He IN)":dbl)
          }
          frame #3 {
            n613 = Search 1D Array(1D array=w1154, element="Shield return press.") -> (index of element=w1152:i32)  [unwired: 1 in]
            n614 = Index Array(array=w1153, index=w1152) -> (element=→"P_SldRTN" →"P (shield return)":dbl)
          }
          frame #4 {
            n615 = Search 1D Array(1D array=w1159, element="3He pot pressure") -> (index of element=w1157:i32)  [unwired: 1 in]
            n616 = Index Array(array=w1158, index=w1157) -> (element=→"P_3Hepot" →"P (3He pot)":dbl)
          }
          frame #5 {
            n617 = Search 1D Array(1D array=w1164, element="1Kpot pressure") -> (index of element=w1161:i32)  [unwired: 1 in]
            n618 = Index Array(array=w1162, index=w1161) -> (element=→"P_1Kpot" →"P (1K pot)":dbl)
          }
          frame #6 {
            n619 = Search 1D Array(1D array=w1169, element="Dewar pressure") -> (index of element=w1166:i32)  [unwired: 1 in]
            n620 = Index Array(array=w1167, index=w1166) -> (element=→"P_Dewar" →"P (Dewar)":dbl)
          }
          frame #7 {
            n621 = Search 1D Array(1D array=w1174, element="HEX7 out pressure") -> (index of element=w1171:i32)  [unwired: 1 in]
            n622 = Index Array(array=w1172, index=w1171) -> (element=→"P_HEX7OUT" →"P (HEX7 out)":dbl)
          }
          frame #8 {
            n623 = Search 1D Array(1D array=w1179, element="Diff pressure HEX4") -> (index of element=w1176:i32)  [unwired: 1 in]
            n624 = Index Array(array=w1177, index=w1176) -> (element=→"DP_HEX4" →"DP HEX4":dbl)
          }
          frame #9 {
            n625 = Search 1D Array(1D array=w1184, element="Diff pressure HEX5") -> (index of element=w1181:i32)  [unwired: 1 in]
            n626 = Index Array(array=w1182, index=w1181) -> (element=→"DP_HEX5" →"DP HEX5":dbl)
          }
          frame #10 {
            n627 = Search 1D Array(1D array=w1189, element="1K pump exhaust flow") -> (index of element=w1186:i32)  [unwired: 1 in]
            n628 = Index Array(array=w1187, index=w1186) -> (element=→"F_1" →"F1 (1K pump exhaust) flow":dbl)
          }
          frame #11 {
            n629 = Search 1D Array(1D array=w1194, element="Shield flow") -> (index of element=w1191:i32)  [unwired: 1 in]
            n630 = Index Array(array=w1192, index=w1191) -> (element=→"F_2" →"F2 (shield flow)":dbl)
          }
          frame #12 {
            n631 = Search 1D Array(1D array=w1199, element="4He return flow from HEX7") -> (index of element=w1197:i32)  [unwired: 1 in]
            n632 = Index Array(array=w1196, index=w1197) -> (element=→"F_3" →"F3 (4He rtn flw via HEX7)":dbl)
          }
          frame #13 {
            n633 = Search 1D Array(1D array=w1204, element="3He incoming flow into HEX7") -> (index of element=w1202:i32)  [unwired: 1 in]
            n634 = Index Array(array=w1201, index=w1202) -> (element=→"F_4" →"F4 (3He in to HEX7)":dbl)
          }
          frame #14 {
            n635 = Search 1D Array(1D array=w1209, element="3He pump exhaust flow") -> (index of element=w1207:i32)  [unwired: 1 in]
            n636 = Index Array(array=w1206, index=w1207) -> (element=→"F_5" →"F5 (3He pump ex.)":dbl)
          }
          frame #15 {
            n637 = Search 1D Array(1D array=w1214, element="4K reservoir level") -> (index of element=w1212:i32)  [unwired: 1 in]
            n638 = Index Array(array=w1211, index=w1212) -> (element=→"L3" →"He level (4K)":dbl)
          }
          frame #16 {
            n639 = Search 1D Array(1D array=w1219, element="1K pot level") -> (index of element=w1217:i32)  [unwired: 1 in]
            n640 = Index Array(array=w1216, index=w1217) -> (element=→"L(1K) (a1)" →"He level (1K)":dbl)
          }
          frame #17 {
            n641 = Search 1D Array(1D array=w1224, element="1K pot (b)") -> (index of element=w1222:i32)  [unwired: 1 in]
            n642 = Index Array(array=w1221, index=w1222) -> (element=→"1K pot(b1)" →"He level (1K) b":dbl)
          }
          frame #18 {
            n643 = Search 1D Array(1D array=w1229, element="3He pot") -> (index of element=w1227:i32)  [unwired: 1 in]
            n644 = Index Array(array=w1226, index=w1227) -> (element=→"3He pot level" →"He level (3He)":dbl)
          }
        }
      }
    }
    n645 = case shown="True" w773 {
      tunnel: [w1896 w1911] -> w844
      tunnel: [w1891 w1910] -> w861
      tunnel: [w1894 w1909] -> w845
      tunnel: w781 -> [w1895 _]
      tunnel: w860 -> [w1885 w1904]
      tunnel: w859 -> [w1886 w1903]
      tunnel: w806 -> [_ w1902]
      tunnel: [w1883 timestamp[] [] ("TimeArray")] -> w858
      tunnel: [w1882 dbl[][] [] ("DataArray")] -> w857
      frame False {
        w1889 = 24 ("index")
        n646 = local read "Record interval"() -> (w1880:i64)
        n647 = call-dynamic "LSI218Data_measure.vi"("LSI218Data in"=w1886, "MeasurementIndex"=w1895, "error in (no error)"=w1885, "save every ... measurements"=w1880) -> ("TimeMeasuremeent"=→"Time of Last Measurement (LSI218)":timestamp, "Active?"=w1890:bool[], "LSI218Data out"=w1894:refnum<class "LSI218Data.lvclass">, "LastMeasurementConfig"=→"LastMeasurementConfig (218)":T15, "LastData"=w1884:dbl[], "Status"=w1891:u16, "TimeArray"=w1883:timestamp[], "DataArray"=w1882:dbl[][], "error out"=w1896:errorcluster)  [unwired: 3 in]
        "LastData (LSI218)" <- w1884
        n648 = Split 1D Array(array=w1890, index=w1889) -> (first subarray=→"Active?\n (1)":bool[], second subarray=→"Active?\n(2)":bool[])
        n649 = Split 1D Array(array=w1884, index=w1889) -> (first subarray=→"Last Data \nLSI218 (1)":dbl[], second subarray=→"Last Data \nLSI218 (2)":dbl[])
      }
      frame True {
        n650 = local read "RUN Identifier"() -> (w1898:string)
        n651 = call-dynamic "LSI218Data_initialize.vi"("LSI218Settings(A-F)"="LSI218Settings(A-F)", "FileFormat"="FileFormat (218)", "base path"=w1902, "error in (no error)"=w1904, "InstName"="InstName (LSI218)", "RunIdentifier"=w1898, "LSI218Data in"=w1903) -> ("error out"=w1911:errorcluster, "Status"=w1910:T7, "AllLabels"=w1901:string[], "LSI218Data out"=w1909:refnum<class "LSI218Data.lvclass">)  [unwired: 1 in]
        n652 = Split 1D Array(array=w1901, index=24) -> (first subarray=→"Labels LSI218 (1)":string[], second subarray=→"Labels LSI218 (2)":string[])
      }
    }
    "LSI218 Status" <- w861
    "error out (LSI218)" <- w844
    n653 = case shown="True" w773 {
      tunnel: [w1791 w1803] -> w831
      tunnel: [w1781 w1802] -> w839
      tunnel: [w1790 w1801] -> w832
      tunnel: [w1789 timestamp[] [] ("TimeArray")] -> w800
      tunnel: [w1788 dbl[][] [] ("DataArray")] -> w798
      tunnel: w841 -> [w1787 w1798]
      tunnel: w840 -> [w1786 w1797]
      tunnel: w781 -> [w1782 _]
      tunnel: w806 -> [_ w1793]
      frame False {
        n654 = local read "Record interval"() -> (w1779:i64)
        n655 = call-dynamic "LSI336Data_measure.vi"("LSI336Data in"=w1787, "MeasurementIndex"=w1782, "error in (no error)"=w1786, "save every ... measurements"=w1779) -> ("Active?"=→"Active?\n(LSI336)":bool[], "TimeMeasuremeent"=→"Time of Last Measurement (LSI336)":timestamp, "LSI336Data out"=w1790:refnum<class "LSI336Data.lvclass">, "LastData"=→"Last Data \nLSI336":dbl[], "LastMeasurementConfig"=→"LastMeasurementConfig (336)":T15, "DataArray"=w1788:dbl[][], "Status"=w1781:u16, "TimeArray"=w1789:timestamp[], "error out"=w1791:errorcluster)  [unwired: 3 in]
      }
      frame True {
        n656 = local read "RUN Identifier"() -> (w1792:string)
        n657 = call-dynamic "LSI336Data_initialize.vi"("LSI336Data in"=w1798, "RunIdentifier"=w1792, "InstName"="InstName (LSI336)", "FileFormat"="FileFormat (336)", "LSI336Settings(X, Y)"="LSI336Settings(X,Y)", "error in (no error)"=w1797, "base path"=w1793) -> ("LSI336Data out"=w1801:refnum<class "LSI336Data.lvclass">, "Status"=w1802:T7, "AllLabels"=→"Labels LSI336":string[], "error out"=w1803:errorcluster)  [unwired: 5 in]
      }
    }
    "LSI336 Status" <- w839
    "error out (LSI336)" <- w831
    "TimeArray (LSI336)" <- w800
    "DataArray (336)" <- w798
    n658 = local read "Last Data \n(USB6210)"() -> (w784:dbl[])
    n659 = local read "Last Data \n(USB6218)"() -> (w785:dbl[])
    n660 = local read "All Labels (USB6210)"() -> (w787:string[])
    n661 = local read "All Labels (USB6218)"() -> (w786:string[])
    n662 = flat-sequence {
      tunnel: w867 -> [w1369]
      tunnel: [w1364] -> w855
      tunnel: [w1362] -> w853
      tunnel: [w1361] -> w850
      tunnel: [w1360] -> w848
      tunnel: w819 -> [w1355]
      frame #0 {
        w1363 = T23 [] ("appended array")
        n663 = Unbundle By Name(w1355) -> ("TimeArray"=w1372:timestamp[], "DataArrayConv"=w1367:dbl[][], "LDArray"=w1366:dbl[])
        n664 = Unbundle By Name(w1369) -> ("ReadLeakDet?"=w1368:bool, "LabelLD"=w1371:string, "Labels"=w1365:string[])  [unwired: 1 out]
        n665 = case shown="True" w1368 {
          tunnel: w1371 -> [_ w1380]
          tunnel: w1367 -> [w1374 w1379]
          tunnel: w1366 -> [_ w1378]
          tunnel: [w1374 w1377] -> w1354
          tunnel: w1365 -> [w1373 w1376]
          tunnel: [w1373 w1375] -> w1357
          frame False {
          }
          frame True {
            n666 = Build Array (concatenate)(w1379, w1378) -> (w1377:dbl[][])
            n667 = Build Array (concatenate)(w1376, w1380) -> (w1375:string[])
          }
        }
        "All Labels (USB6210)" <- w1357
        "DataArrayConv (USB6210)" <- w1354
        n668 = control-ref of="Plot selecter (USB6210)\n    1      2     3     4"() -> (w1356:refnum<vi>)
        n669 = local read "Plot selecter (USB6210)\n    1      2     3     4"() -> (w1359:bool[][])
        n670 = Array Size(array=w1357) -> (size(s)=w1370:i32)
        n671 = Array Size(array=w1357) -> (size(s)=w1358:i32)
        n672 = Array Size(array=w1354) -> (size(s)=→"Data Array sizes (6210)":i32[])
        n673 = property on="Property Node" class="Arr (strict)"(reference=w1356, "Number of Rows"=w1358) -> ()  [unwired: 1 in, 2 out]
        n674 = for {
          N: w1370 -> [_]
          tunnel: w1354 -> [w1401]
          tunnel: w1372 -> [w1402]
          shift-right: [w1397] -> w1362
          shift-left: w1363 -> [w1400]
          shift-right: [w1395] -> w1360
          shift-left: w1363 -> [w1398]
          shift-right: [w1396] -> w1364
          shift-left: w1363 -> [w1394]
          shift-right: [w1393] -> w1361
          shift-left: w1363 -> [w1392]
          tunnel: w1359 -> [w1391]
          i -> [w1386]
          n675 = Index Array(array=w1401, index (col)=w1386) -> (element=w1381:dbl[])  [unwired: 1 in]
          n676 = Index Array(array=w1391, index (row) #1=w1386, index (col) #1=0 ("index (row)"), index (row) #2=w1386, index (col) #2=1 ("index (row)"), index (row) #3=w1386, index (col) #3=2 ("index (row)"), index (row) #4=w1386, index (col) #4=3 ("index (row)")) -> (element #1=w1385:bool, element #2=w1384:bool, element #3=w1383:bool, element #4=w1382:bool)
          n677 = Bundle("TimeArray"=w1402, "DataArrayConv"=w1381) -> (w1399:T27)  [unwired: 1 in]
          n678 = stacked-sequence {
            tunnel: w1385 -> [w1406 _ _ _]
            tunnel: w1400 -> [_ w1414 _ _]
            tunnel: w1383 -> [_ _ w1422 _]
            tunnel: w1399 -> [w1403 w1412 w1421 w1427]
            tunnel: w1382 -> [_ _ _ w1430]
            tunnel: w1398 -> [_ _ _ w1429]
            tunnel: [_ _ _ w1428] -> w1395
            tunnel: [_ w1413 _ _] -> w1397
            tunnel: [w1405 _ _ _] -> w1396
            tunnel: w1394 -> [w1404 _ _ _]
            tunnel: [_ _ w1420 _] -> w1393
            tunnel: w1392 -> [_ _ w1419 _]
            tunnel: w1384 -> [_ w1411 _ _]
            frame #0 {
              n679 = case shown="True" w1406 {
                tunnel: [w1407 w1410] -> w1405
                tunnel: w1403 -> [_ w1409]
                tunnel: w1404 -> [w1407 w1408]
                frame False {
                }
                frame True {
                  n680 = Build Array (concatenate)(w1408, w1409) -> (w1410:T23)
                }
              }
            }
            frame #1 {
              n681 = case shown="True" w1411 {
                tunnel: w1414 -> [w1415 w1418]
                tunnel: [w1415 w1417] -> w1413
                tunnel: w1412 -> [_ w1416]
                frame False {
                }
                frame True {
                  n682 = Build Array (concatenate)(w1418, w1416) -> (w1417:T23)
                }
              }
            }
            frame #2 {
              n683 = case shown="True" w1422 {
                tunnel: [w1423 w1426] -> w1420
                tunnel: w1421 -> [_ w1425]
                tunnel: w1419 -> [w1423 w1424]
                frame False {
                }
                frame True {
                  n684 = Build Array (concatenate)(w1424, w1425) -> (w1426:T23)
                }
              }
            }
            frame #3 {
              n685 = case shown="True" w1430 {
                tunnel: [w1431 w1434] -> w1428
                tunnel: w1427 -> [_ w1433]
                tunnel: w1429 -> [w1431 w1432]
                frame False {
                }
                frame True {
                  n686 = Build Array (concatenate)(w1432, w1433) -> (w1434:T23)
                }
              }
            }
          }
        }
      }
    }
    n687 = case shown="True" "Digital Out ON?" {
      tunnel: w773 -> [_ w1492]
      tunnel: w821 -> [w1485 w1491]
      tunnel: [w1485 w1490] -> w820
      tunnel: w819 -> [_ w1489]
      tunnel: w774 -> [_ w1488]
      tunnel: w806 -> [_ w1487]
      tunnel: w801 -> [_ w1486]
      frame False {
      }
      frame True {
        n688 = case shown="True" w1492 {
          tunnel: w1491 -> [w1510 w1692]
          tunnel: [w1510 w1706] -> w1490
          tunnel: w1489 -> [w1511 _]
          tunnel: w1488 -> [_ w1697]
          tunnel: w1487 -> [_ w1684]
          tunnel: w1486 -> [_ _]
          frame False {
            n689 = flat-sequence {
              frame #0 {
              }
            }
            n690 = case shown="\"USB6218AI\"" "AutoFill Source (P)" {
              tunnel: [w1514 w1515] -> w1496
              frame "USB6210", Default {
                n691 = local read "All Labels (USB6210)"() -> (w1514:string[])
              }
              frame "USB6218AI" {
                n692 = local read "All Labels (USB6218)"() -> (w1515:string[])
              }
            }
            n693 = case shown="\"USB6210\", Default" "AutoFill Source (L)" {
              tunnel: [w1512 w1513] -> w1493
              frame "USB6210", Default {
                n694 = local read "All Labels (USB6210)"() -> (w1512:string[])
              }
              frame "USB6218AI" {
                n695 = local read "All Labels (USB6218)"() -> (w1513:string[])
              }
            }
            n696 = Multiply(x="N for sampling", y=i64 2) -> (x*y=w1505:i64)
            n697 = local read "Cycle #"() -> (w1509:u32)
            n698 = Search 1D Array(1D array=w1496, element="Auto Fll Dewar P. label") -> (index of element=→"Target Index (P)":i32)  [unwired: 1 in]
            n699 = Search 1D Array(1D array=w1493, element="Auto Fll He L. label") -> (index of element=→"Target Index (L)":i32)  [unwired: 1 in]
            n700 = Add(x=w1505, y="Mov. Avg Interval") -> (x+y=w1507:i64)
            n701 = Greater?(x=w1509, y=w1507) -> (0:w1503:bool)
            n702 = And(x=w1503, y="Auto Fill ON?") -> (x .and. y?=w1501:bool)
            n703 = case shown="True" w1501 {
              tunnel: w1511 -> [_ w1549]
              tunnel: "Mov. Avg Interval" -> [_ w1535]
              tunnel: w1505 -> [_ w1522]
              tunnel: "N for sampling" -> [_ w1533]
              frame False {
              }
              frame True {
                n704 = local read "AutoFill Source (L)"() -> (w1516:T8)
                n705 = local read "AutoFill Source (P)"() -> (w1517:T8)
                n706 = case shown="\"USB6218AI\"" w1517 {
                  tunnel: [w1553 w1554] -> w1518
                  frame "USB6210", Default {
                    n707 = local read "DataArrayConv (USB6210)"() -> (w1553:dbl[][])
                  }
                  frame "USB6218AI" {
                    n708 = local read "DataArrayConv (USB6218)"() -> (w1554:dbl[][])
                  }
                }
                n709 = case shown="\"USB6210\", Default" w1516 {
                  tunnel: [w1551 w1552] -> w1520
                  frame "USB6210", Default {
                    n710 = local read "DataArrayConv (USB6210)"() -> (w1551:dbl[][])
                  }
                  frame "USB6218AI" {
                    n711 = local read "DataArrayConv (USB6218)"() -> (w1552:dbl[][])
                  }
                }
                n712 = local read "Pstd"() -> (→"Pstd history":dbl)
                n713 = local read "Lstd"() -> (→"Lstd history":dbl)
                n714 = local read "Target Index (L)"() -> (w1521:i32)
                n715 = local read "Pav (Pa)"() -> (→"Pav history":dbl)
                n716 = local read "Lav (%)"() -> (→"Lav history":dbl)
                n717 = Index Array(array=w1520, index (col)=w1521) -> (element=w1519:dbl[])  [unwired: 1 in]
                n718 = local read "Target Index (P)"() -> (w1550:i32)
                n719 = Unbundle By Name(w1549) -> ("TimeArray"=w1548:timestamp[])
                n720 = Index Array(array=w1518, index (col)=w1550) -> (element=w1537:dbl[])  [unwired: 1 in]
                n721 = Delete From Array(array=w1537, length=w1522) -> (deleted portion=w1545:dbl[])  [unwired: 1 in, 1 out]
                n722 = Delete From Array(array=w1519, length=w1522) -> (deleted portion=w1532:dbl[])  [unwired: 1 in, 1 out]
                n723 = call "MovingAverage.vi"("Moving Average interval"=w1535, "Input Array"=w1519) -> ("M.A. Array"=w1534:dbl[])  [unwired: 9 in]
                n724 = call "MovingAverage.vi"("Moving Average interval"=w1535, "Input Array"=w1537) -> ("M.A. Array"=w1536:dbl[])  [unwired: 9 in]
                n725 = Delete From Array(array=w1536, length=w1522) -> (deleted portion=w1546:dbl[])  [unwired: 1 in, 1 out]
                n726 = Delete From Array(array=w1536, length=w1522) -> (deleted portion=w1542:dbl[])  [unwired: 1 in, 1 out]
                "Last N M.A. Pressures" <- w1542
                n727 = Delete From Array(array=w1534, length=w1522) -> (deleted portion=w1527:dbl[])  [unwired: 1 in, 1 out]
                "Last N M.A. Levels" <- w1527
                n728 = Delete From Array(array=w1548, length=w1522) -> (deleted portion=w1529:timestamp[])  [unwired: 1 in, 1 out]
                n729 = Bundle("TimeArray"=w1529, "DataArrayConv (USB6218)"=w1545) -> (w1544:T28)  [unwired: 1 in]
                n730 = Bundle("TimeArray"=w1529, "M.A. Array"=w1546) -> (w1547:T29)  [unwired: 1 in]
                n731 = Bundle("TimeArray"=w1529, "DataArrayConv (USB6218)"=w1532) -> (w1531:T28)  [unwired: 1 in]
                n732 = Bundle("TimeArray"=w1529, "M.A. Array"=w1527) -> (w1528:T29)  [unwired: 1 in]
                n733 = Array Size(array=w1542) -> (size(s)=w1541:i32)
                n734 = Greater Or Equal?(x=w1541, y=w1533) -> (x >= y?=w1540:bool)
                n735 = Build Array(w1544, w1547) -> (→"Dewar Pressure":T30)
                n736 = Build Array(w1531, w1528) -> (→"He Level":T30)
                n737 = case shown="True" w1540 {
                  tunnel: [w1658 w1663] -> w1526
                  tunnel: w1542 -> [_ w1664]
                  tunnel: w1527 -> [_ w1661]
                  tunnel: [w1658 w1659] -> w1525
                  frame False {
                    w1658 = nan ("mean")
                  }
                  frame True {
                    n738 = call <vilib>:"Std Deviation and Variance.vi"("X"=w1664) -> ("mean"=w1663:dbl, "standard deviation"=w1662:dbl)  [unwired: 1 in, 1 out]
                    n739 = call <vilib>:"Std Deviation and Variance.vi"("X"=w1661) -> ("mean"=w1659:dbl, "standard deviation"=w1660:dbl)  [unwired: 1 in, 1 out]
                    n740 = local write "Pstd"(w1662) -> ()
                    n741 = local write "Lstd"(w1660) -> ()
                    n742 = local write "Pav (Pa)"(w1663) -> ()
                    n743 = local write "Lav (%)"(w1659) -> ()
                  }
                }
                n744 = flat-sequence {
                  tunnel: w1526 -> [w1555]
                  tunnel: w1525 -> [w1556]
                  frame #0 {
                    n745 = flat-sequence {
                      tunnel: w1556 -> [w1558]
                      tunnel: w1555 -> [w1557]
                      tunnel: w1555 -> [w1626]
                      frame #0 {
                        n746 = stacked-sequence {
                          tunnel: w1558 -> [w1565 w1569 _ _ _ _]
                          tunnel: w1557 -> [_ _ w1583 w1592 w1601 w1610]
                          frame #0 {
                            n747 = local read "L_low (%)"() -> (w1564:dbl)
                            n748 = local read "Fill state"() -> (w1562:bool)
                            n749 = Less?(x=w1565, y=w1564) -> (x < y?=w1561:bool)
                            n750 = Equal?(x=w1562, y=FALSE) -> (x = y?=w1560:bool)
                            n751 = And(x=w1561, y=w1560) -> (x .and. y?=w1559:bool)
                            n752 = case shown="False" w1559 {
                              frame False {
                              }
                              frame True {
                                w1567 = TRUE ("Value (Signaling)")
                                n753 = property on="Fill state" class="Bool (strict)"("Val(Sgnl)"=w1567) -> ()  [unwired: 2 in, 2 out]
                                n754 = Not(x=w1567) -> (.not. x?=w1566:bool)
                                n755 = property on="Fill (false)" class="Bool (strict)"("Val(Sgnl)"=w1566) -> ()  [unwired: 2 in, 2 out]
                              }
                            }
                          }
                          frame #1 {
                            n756 = local read "L_high (%)"() -> (w1570:dbl)
                            n757 = local read "Fill state"() -> (w1573:bool)
                            n758 = Greater?(x=w1569, y=w1570) -> (0:w1568:bool)
                            n759 = Equal?(x=w1573, y=TRUE) -> (x = y?=w1572:bool)
                            n760 = And(x=w1568, y=w1572) -> (x .and. y?=w1571:bool)
                            n761 = case shown="True" w1571 {
                              frame False {
                              }
                              frame True {
                                w1575 = FALSE ("Value (Signaling)")
                                n762 = property on="Fill state" class="Bool (strict)"("Val(Sgnl)"=w1575) -> ()  [unwired: 2 in, 2 out]
                                n763 = Not(x=w1575) -> (.not. x?=w1576:bool)
                                n764 = property on="Fill (false)" class="Bool (strict)"("Val(Sgnl)"=w1576) -> ()  [unwired: 2 in, 2 out]
                              }
                            }
                          }
                          frame #2 {
                            n765 = local read "P_1_low (Pa)"() -> (w1582:dbl)
                            n766 = property on="state 1" class="Bool (strict)"() -> ("Value"=w1580:bool)  [unwired: 2 in, 2 out]
                            n767 = Less?(x=w1583, y=w1582) -> (x < y?=w1579:bool)
                            n768 = Equal?(x=w1580, y=FALSE) -> (x = y?=w1578:bool)
                            n769 = And(x=w1578, y=w1579) -> (x .and. y?=w1577:bool)
                            n770 = case shown="True" w1577 {
                              frame False {
                              }
                              frame True {
                                w1585 = TRUE ("Value (Signaling)")
                                n771 = property on="state 1" class="Bool (strict)"("Val(Sgnl)"=w1585) -> ()  [unwired: 2 in, 2 out]
                                n772 = Not(x=w1585) -> (.not. x?=w1584:bool)
                                n773 = property on="state 1 (false)" class="Bool (strict)"("Val(Sgnl)"=w1584) -> ()  [unwired: 2 in, 2 out]
                              }
                            }
                          }
                          frame #3 {
                            n774 = local read "P_1_high (Pa)"() -> (w1591:dbl)
                            n775 = property on="state 1" class="Bool (strict)"() -> ("Value"=w1589:bool)  [unwired: 2 in, 2 out]
                            n776 = Greater?(x=w1592, y=w1591) -> (0:w1588:bool)
                            n777 = Equal?(x=w1589, y=TRUE) -> (x = y?=w1587:bool)
                            n778 = And(x=w1587, y=w1588) -> (x .and. y?=w1586:bool)
                            n779 = case shown="True" w1586 {
                              frame False {
                              }
                              frame True {
                                w1594 = FALSE ("Value (Signaling)")
                                n780 = property on="state 1" class="Bool (strict)"("Val(Sgnl)"=w1594) -> ()  [unwired: 2 in, 2 out]
                                n781 = Not(x=w1594) -> (.not. x?=w1593:bool)
                                n782 = property on="state 1 (false)" class="Bool (strict)"("Val(Sgnl)"=w1593) -> ()  [unwired: 2 in, 2 out]
                              }
                            }
                          }
                          frame #4 {
                            n783 = local read "P_2_low (Pa)"() -> (w1600:dbl)
                            n784 = property on="state 2" class="Bool (strict)"() -> ("Value"=w1595:bool)  [unwired: 2 in, 2 out]
                            n785 = Less?(x=w1601, y=w1600) -> (x < y?=w1598:bool)
                            n786 = Equal?(x=w1595, y=FALSE) -> (x = y?=w1597:bool)
                            n787 = And(x=w1597, y=w1598) -> (x .and. y?=w1596:bool)
                            n788 = case shown="True" w1596 {
                              frame False {
                              }
                              frame True {
                                w1602 = TRUE ("Value (Signaling)")
                                n789 = property on="state 2" class="Bool (strict)"("Val(Sgnl)"=w1602) -> ()  [unwired: 2 in, 2 out]
                                n790 = Not(x=w1602) -> (.not. x?=w1603:bool)
                                n791 = property on="state 2 (false)" class="Bool (strict)"("Val(Sgnl)"=w1603) -> ()  [unwired: 2 in, 2 out]
                              }
                            }
                          }
                          frame #5 {
                            n792 = local read "P_2_high (Pa)"() -> (w1609:dbl)
                            n793 = property on="state 2" class="Bool (strict)"() -> ("Value"=w1604:bool)  [unwired: 2 in, 2 out]
                            n794 = Greater?(x=w1610, y=w1609) -> (0:w1607:bool)
                            n795 = Equal?(x=w1604, y=TRUE) -> (x = y?=w1606:bool)
                            n796 = And(x=w1606, y=w1607) -> (x .and. y?=w1605:bool)
                            n797 = case shown="True" w1605 {
                              frame False {
                              }
                              frame True {
                                w1611 = FALSE ("Value (Signaling)")
                                n798 = property on="state 2" class="Bool (strict)"("Val(Sgnl)"=w1611) -> ()  [unwired: 2 in, 2 out]
                                n799 = Not(x=w1611) -> (.not. x?=w1612:bool)
                                n800 = property on="state 2 (false)" class="Bool (strict)"("Val(Sgnl)"=w1612) -> ()  [unwired: 2 in, 2 out]
                              }
                            }
                          }
                        }
                      }
                      frame #1 {
                        n801 = property on="Fill state" class="Bool (strict)"() -> ("Value"=w1613:bool)  [unwired: 2 in, 2 out]
                        n802 = case shown="True" w1613 {
                          frame False {
                            n803 = property on="V1 (N.O.)" class="Bool (strict)"("Val(Sgnl)"=TRUE ("V1 (N.O.)")) -> ()  [unwired: 2 in, 2 out]
                            n804 = property on="V2 (N.C.)" class="Bool (strict)"("Val(Sgnl)"=FALSE ("Value (Signaling)")) -> ()  [unwired: 2 in, 2 out]
                          }
                          frame True {
                            n805 = property on="state 1" class="Bool (strict)"() -> ("Value"=w1617:bool)  [unwired: 2 in, 2 out]
                            n806 = property on="state 2" class="Bool (strict)"() -> ("Value"=w1616:bool)  [unwired: 2 in, 2 out]
                            n807 = case shown="True" w1617 {
                              frame False {
                                n808 = property on="V1 (N.O.)" class="Bool (strict)"("Val(Sgnl)"=TRUE ("Value (Signaling)")) -> ()  [unwired: 2 in, 2 out]
                                n809 = local write "Status V1 CTRL"(enum16{"Pressurize", "Release"}."Release" ("Status V1 CTRL")) -> ()
                              }
                              frame True {
                                n810 = property on="V1 (N.O.)" class="Bool (strict)"("Val(Sgnl)"=FALSE ("V1 (N.O.)")) -> ()  [unwired: 2 in, 2 out]
                                n811 = local write "Status V1 CTRL"(enum16{"Pressurize", "Release"}."Pressurize" ("Status V1 CTRL")) -> ()
                              }
                            }
                            n812 = case shown="True" w1616 {
                              frame False {
                                n813 = property on="V2 (N.C.)" class="Bool (strict)"("Val(Sgnl)"=FALSE ("Value (Signaling)")) -> ()  [unwired: 2 in, 2 out]
                                n814 = local write "Status V2 CTRL"(enum16{"Pressurize", "Release"}."Release" ("Status V2 CTRL")) -> ()
                              }
                              frame True {
                                n815 = property on="V2 (N.C.)" class="Bool (strict)"("Val(Sgnl)"=TRUE ("Value (Signaling)")) -> ()  [unwired: 2 in, 2 out]
                                n816 = local write "Status V2 CTRL"(enum16{"Pressurize", "Release"}."Pressurize" ("Status V2 CTRL")) -> ()
                              }
                            }
                          }
                        }
                      }
                      frame #2 {
                        n817 = Greater?(x=w1626, y="P_safelimit_high (Pa)") -> (0:w1628:bool)
                        n818 = Less?(x=w1626, y="P_safelimit_low (Pa)") -> (x < y?=w1630:bool)
                        n819 = Or(x=w1628, y=w1630) -> (x .or. y?=w1631:bool)
                        n820 = case shown="False" w1631 {
                          frame False {
                          }
                          frame True {
                            w1632 = FALSE ("Value (Signaling)")
                            w1634 = FALSE ("Value (Signaling)")
                            n821 = property on="V2 (N.C.)" class="Bool (strict)"("Val(Sgnl)"=FALSE ("V1 (N.O.)")) -> ()  [unwired: 2 in, 2 out]
                            n822 = property on="state 1" class="Bool (strict)"("Val(Sgnl)"=w1632) -> ()  [unwired: 2 in, 2 out]
                            n823 = property on="V1 (N.O.)" class="Bool (strict)"("Val(Sgnl)"=TRUE ("V1 (N.O.)")) -> ()  [unwired: 2 in, 2 out]
                            n824 = property on="state 2" class="Bool (strict)"("Val(Sgnl)"=w1634) -> ()  [unwired: 2 in, 2 out]
                            n825 = Not(x=w1632) -> (.not. x?=w1633:bool)
                            n826 = Not(x=w1634) -> (.not. x?=w1635:bool)
                            n827 = property on="state 1 (false)" class="Bool (strict)"("Val(Sgnl)"=w1633) -> ()  [unwired: 2 in, 2 out]
                            n828 = property on="state 2 (false)" class="Bool (strict)"("Val(Sgnl)"=w1635) -> ()  [unwired: 2 in, 2 out]
                          }
                        }
                      }
                    }
                  }
                  frame #1 {
                    n829 = property on="V2 (N.C.)" class="Bool (strict)"() -> ("Value"=w1645:bool)  [unwired: 2 in, 2 out]
                    n830 = property on="V1 (N.O.)" class="Bool (strict)"() -> ("Value"=w1656:bool)  [unwired: 2 in, 2 out]
                    n831 = local read "P_1_high (Pa)"() -> (w1650:dbl)
                    n832 = local read "P_2_high (Pa)"() -> (w1648:dbl)
                    n833 = local read "P_1_low (Pa)"() -> (w1651:dbl)
                    n834 = local read "P_2_low (Pa)"() -> (w1649:dbl)
                    n835 = local read "L_high (%)"() -> (w1646:dbl)
                    n836 = local read "L_low (%)"() -> (w1647:dbl)
                    n837 = local read "Pav (Pa)"() -> (w1639:dbl)
                    n838 = local read "Lav (%)"() -> (w1638:dbl)
                    n839 = Boolean To (0,1)(Boolean=w1645) -> (0, 1=w1644:i16)
                    n840 = Boolean To (0,1)(Boolean=w1656) -> (0, 1=w1657:i16)
                    n841 = local read "File Refn DewarCTRL"() -> (w1652:refnum<file>)
                    n842 = local read "Cycle #"() -> (w1655:u32)
                    n843 = Build Array(w1639, w1638, w1651, w1650, w1649, w1648, w1647, w1646, w1657, w1644) -> (w1643:dbl[])
                    n844 = Get Date/Time In Seconds() -> (seconds since 1Jan1904=w1653:timestamp)
                    n845 = call "FileWrite.vi"("DataArray"=w1643, "Time Stamp"=w1653, "Error In"=errorcluster {"status"=FALSE, "code"=0, "source"=""}, "FileFormat"=string[] ["%4.5e", "%4.2f", "%4.4e", "%4.4e", "%4.4e", "%4.4e", "%4.4e", "%d", "%d"] ("Array"), "Index"=w1655, "refnum in"=w1652) -> ("Error Out"=→"Error Out (Dewar CTRL":errorcluster, "Byte Stream File Refnum"=w1642:refnum<file>)  [unwired: 4 in]
                    n846 = local write "File Refn DewarCTRL"(w1642) -> ()
                  }
                }
              }
            }
          }
          frame True {
            w1703 = "_"
            w1665 = FALSE ("auto cleanup")
            w1667 = 1 items=["one channel for each line", "one channel for all lines"] ("line grouping")
            n847 = flat-sequence {
              frame #0 {
                w1720 = FALSE ("V1 (N.O.)")
                n848 = local write "V2 (N.C.)"(FALSE ("V1 (N.O.)")) -> ()
                n849 = local write "V1 (N.O.)"(TRUE ("V1 (N.O.)")) -> ()
                n850 = local write "state 2"(w1720) -> ()
                n851 = local write "state 1"(w1720) -> ()
                n852 = local write "Fill state"(w1720) -> ()
                n853 = Not(x=w1720) -> (.not. x?=w1722:bool)
                n854 = Not(x=w1720) -> (.not. x?=w1721:bool)
                n855 = local write "state 1 (false)"(w1721) -> ()
                n856 = local write "state 2 (false)"(w1721) -> ()
                n857 = local write "Fill (false)"(w1722) -> ()
              }
            }
            n858 = Get Date/Time In Seconds() -> (seconds since 1Jan1904=w1717:timestamp)
            n859 = call "LV_UNIXTIME.vi"("current time"=w1717) -> ("date/time string"=w1698:string)  [unwired: 9 in, 1 out]
            n860 = Concatenate Strings(w1698, "_DO" ("new task name")) -> (w1714:string)
            n861 = Concatenate Strings(w1697, w1703, w1698, w1703) -> (w1683:string)
            n862 = Concatenate Strings(w1683, "DEWAR.csv" ("string")) -> (w1682:string)
            n863 = Concatenate Strings(w1683, "USB_DOUT.csv" ("string")) -> (w1686:string)
            n864 = Build Path(base path=w1684, name or relative path=w1682) -> (appended path=w1681:path)
            n865 = Build Path(base path=w1684, name or relative path=w1686) -> (appended path=w1702:path)
            n866 = Open/Create/Replace File(file path (use dialog)=w1702, error in=w1692, operation (0:open)=T22."open or create") -> (refnum out=w1700:refnum<file>, error out=w1691:errorcluster)  [unwired: 3 in, 1 out]
            n867 = call "FileIntialize.vi"("Error In"=w1691, "Labels"="DOUT Labels", "refnum in"=w1700) -> ("Error Out"=w1678:errorcluster, "File Refnum"=→"File Refn USB DO":refnum<file>)  [unwired: 7 in]
            n868 = Open/Create/Replace File(file path (use dialog)=w1681, error in=w1678, operation (0:open)=T22."open or create") -> (refnum out=w1689:refnum<file>, error out=w1690:errorcluster)  [unwired: 3 in, 1 out]
            n869 = call "FileIntialize.vi"("Error In"=w1690, "Labels"=string[] ["P_av", "L_av", "P_1_low", "P_1_high", "P_2_low", "P_2_high", "L_low", "L_high", "V1(NO)", "V2(NC)"], "refnum in"=w1689) -> ("Error Out"=w1677:errorcluster, "File Refnum"=→"File Refn DewarCTRL":refnum<file>)  [unwired: 7 in]
            n870 = Index Array(array="DOUT Physical CH", index #1=0 ("index"), index #2=1 ("index"), index #3=2 ("index"), index #4=3 ("index")) -> (element #1=w1695:tag, element #2=w1673:tag, element #3=w1672:tag, element #4=w1666:tag)
            n871 = call <vilib>:"DAQmx Create Task.vi"("new task name"=w1714, "auto cleanup"=FALSE, "error in"=w1677) -> ("task out"=w1715:refnum<k21>, "error out"=w1716:errorcluster)  [unwired: 11 in]
            n872 = call-poly <vilib>:"DAQmx Create Virtual Channel.vi"("task in"=w1715, "lines"=w1695, "line grouping"=w1667, "error in"=w1716) -> ("task out"=w1718:refnum<k21>, "error out"=w1719:errorcluster)  [unwired: 10 in]
            n873 = call-poly <vilib>:"DAQmx Create Virtual Channel.vi"("task in"=w1718, "lines"=w1673, "line grouping"=w1667, "error in"=w1719) -> ("task out"=w1705:refnum<k21>, "error out"=w1704:errorcluster)  [unwired: 10 in]
            n874 = call-poly <vilib>:"DAQmx Create Virtual Channel.vi"("task in"=w1705, "lines"=w1672, "line grouping"=w1667, "error in"=w1704) -> ("task out"=w1671:refnum<k21>, "error out"=w1670:errorcluster)  [unwired: 10 in]
            n875 = call-poly <vilib>:"DAQmx Create Virtual Channel.vi"("task in"=w1671, "lines"=w1666, "line grouping"=w1667, "error in"=w1670) -> ("task out"=w1668:refnum<k21>, "error out"=w1669:errorcluster)  [unwired: 10 in]
            n876 = call <vilib>:"DAQmx Start Task.vi"("task/channels in"=w1668, "error in"=w1669) -> ("task out"=w1709:refnum<k21>, "error out"=w1707:errorcluster)  [unwired: 12 in]
            n877 = Build Array(w1665, w1665, w1665, w1665) -> (w1710:bool[])
            n878 = call <vilib>:"DAQmx Write (Digital 1D Bool NChan 1Samp 1Line).vi"("task/channels in"=w1709, "data"=w1710, "timeout"=10.0, "error in"=w1707) -> ("task out"=→"DOUT task out":refnum<k21>, "error out"=w1706:errorcluster)  [unwired: 9 in, 1 out]
          }
        }
      }
    }
    "error out (USB6210/6218 DOUT)" <- w820
    n879 = flat-sequence {
      tunnel: w815 -> [w1288]
      tunnel: [w1283] -> w814
      tunnel: [w1281] -> w813
      tunnel: [w1280] -> w812
      tunnel: [w1279] -> w811
      tunnel: w816 -> [w1275]
      frame #0 {
        w1282 = T23 [] ("appended array")
        n880 = Unbundle By Name(w1275) -> ("TimeArray"=w1271:timestamp[], "DataArrayConv"=w1286:dbl[][], "LDArray"=w1285:dbl[])
        "TimeArray (USB6218)" <- w1271
        n881 = Unbundle By Name(w1288) -> ("ReadLeakDet?"=w1287:bool, "LabelLD"=w1290:string, "Labels"=w1284:string[])  [unwired: 1 out]
        n882 = case shown="True" w1287 {
          tunnel: w1290 -> [_ w1298]
          tunnel: w1286 -> [w1292 w1297]
          tunnel: w1285 -> [_ w1296]
          tunnel: [w1292 w1295] -> w1273
          tunnel: w1284 -> [w1291 w1294]
          tunnel: [w1291 w1293] -> w1276
          frame False {
          }
          frame True {
            n883 = Build Array (concatenate)(w1297, w1296) -> (w1295:dbl[][])
            n884 = Build Array (concatenate)(w1294, w1298) -> (w1293:string[])
          }
        }
        "All Labels (USB6218)" <- w1276
        "DataArrayConv (USB6218)" <- w1273
        n885 = Array Size(array=w1271) -> (size(s)=→"TimeArray size (6218)":i32)
        n886 = local read "Plot selecter (USB6218)\n    1      2     3     4"() -> (w1278:bool[][])
        n887 = control-ref of="Plot selecter (USB6218)\n    1      2     3     4"() -> (w1274:refnum<vi>)
        n888 = Array Size(array=w1276) -> (size(s)=w1277:i32)
        n889 = Array Size(array=w1276) -> (size(s)=w1289:i32)
        n890 = Array Size(array=w1273) -> (size(s)=→"DataArraySize (6218)":i32[])
        n891 = property on="Property Node" class="Arr (strict)"(reference=w1274, "Number of Rows"=w1277) -> ()  [unwired: 1 in, 2 out]
        n892 = for {
          N: w1289 -> [_]
          tunnel: w1273 -> [w1319]
          tunnel: w1271 -> [w1320]
          shift-right: [w1314] -> w1281
          shift-left: w1282 -> [w1317]
          shift-right: [w1312] -> w1279
          shift-left: w1282 -> [w1315]
          shift-right: [w1313] -> w1283
          shift-left: w1282 -> [w1311]
          shift-right: [w1310] -> w1280
          shift-left: w1282 -> [w1309]
          tunnel: w1278 -> [w1308]
          i -> [w1303]
          n893 = Index Array(array=w1319, index (col)=w1303) -> (element=w1318:dbl[])  [unwired: 1 in]
          n894 = Index Array(array=w1308, index (row) #1=w1303, index (col) #1=0 ("index (row)"), index (row) #2=w1303, index (col) #2=1 ("index (row)"), index (row) #3=w1303, index (col) #3=2 ("index (row)"), index (row) #4=w1303, index (col) #4=3 ("index (row)")) -> (element #1=w1302:bool, element #2=w1301:bool, element #3=w1300:bool, element #4=w1299:bool)
          n895 = Bundle("TimeArray"=w1320, "DataArrayConv"=w1318) -> (w1316:T27)  [unwired: 1 in]
          n896 = stacked-sequence {
            tunnel: w1302 -> [w1324 _ _ _]
            tunnel: w1317 -> [_ w1332 _ _]
            tunnel: w1300 -> [_ _ w1340 _]
            tunnel: w1316 -> [w1321 w1330 w1339 w1345]
            tunnel: w1299 -> [_ _ _ w1348]
            tunnel: w1315 -> [_ _ _ w1347]
            tunnel: [_ _ _ w1346] -> w1312
            tunnel: [_ w1331 _ _] -> w1314
            tunnel: [w1323 _ _ _] -> w1313
            tunnel: w1311 -> [w1322 _ _ _]
            tunnel: [_ _ w1338 _] -> w1310
            tunnel: w1309 -> [_ _ w1337 _]
            tunnel: w1301 -> [_ w1329 _ _]
            frame #0 {
              n897 = case shown="True" w1324 {
                tunnel: [w1325 w1328] -> w1323
                tunnel: w1321 -> [_ w1327]
                tunnel: w1322 -> [w1325 w1326]
                frame False {
                }
                frame True {
                  n898 = Build Array (concatenate)(w1326, w1327) -> (w1328:T23)
                }
              }
            }
            frame #1 {
              n899 = case shown="True" w1329 {
                tunnel: w1332 -> [w1333 w1336]
                tunnel: [w1333 w1335] -> w1331
                tunnel: w1330 -> [_ w1334]
                frame False {
                }
                frame True {
                  n900 = Build Array (concatenate)(w1336, w1334) -> (w1335:T23)
                }
              }
            }
            frame #2 {
              n901 = case shown="True" w1340 {
                tunnel: [w1341 w1344] -> w1338
                tunnel: w1339 -> [_ w1343]
                tunnel: w1337 -> [w1341 w1342]
                frame False {
                }
                frame True {
                  n902 = Build Array (concatenate)(w1342, w1343) -> (w1344:T23)
                }
              }
            }
            frame #3 {
              n903 = case shown="True" w1348 {
                tunnel: [w1349 w1352] -> w1346
                tunnel: w1345 -> [_ w1351]
                tunnel: w1347 -> [w1349 w1350]
                frame False {
                }
                frame True {
                  n904 = Build Array (concatenate)(w1350, w1351) -> (w1352:T23)
                }
              }
            }
          }
        }
      }
    }
    n905 = Build Array (concatenate)(w784, w785) -> (w782:dbl[])
    n906 = Build Array (concatenate)(w787, w786) -> (w783:string[])
    n907 = local read "Plot selecter LSI218(2)\n    1      2     3     4"() -> (w842:bool[][])
    n908 = local read "Plot selecter LSI218(1)\n    1      2     3     4"() -> (w843:bool[][])
    n909 = for {
      N: 48 -> [_]
      tunnel: w858 -> [w1824]
      tunnel: w857 -> [w1821]
      tunnel: w843 -> [w1805]
      tunnel: w842 -> [w1806]
      shift-right: [w1822] -> w856
      shift-left: w854 -> [w1823]
      shift-right: [w1817] -> w851
      shift-left: w854 -> [w1818]
      shift-right: [w1816] -> w849
      shift-left: w854 -> [w1815]
      shift-right: [w1814] -> w847
      shift-left: w854 -> [w1813]
      i -> [w1811]
      n910 = Index Array(array=w1821, index (col)=w1811) -> (element=w1820:dbl[])  [unwired: 1 in]
      n911 = Less?(x=w1811, y=24) -> (x < y?=w1812:bool)
      n912 = case shown="True" w1812 {
        tunnel: [w1829 w1847] -> w1810
        tunnel: [w1828 w1846] -> w1809
        tunnel: [w1827 w1844] -> w1808
        tunnel: [w1826 w1843] -> w1807
        tunnel: w1805 -> [_ w1842]
        tunnel: w1806 -> [w1836 _]
        tunnel: w1811 -> [w1831 w1839]
        frame False {
          n913 = Subtract(x=w1831, y=24) -> (x-y=w1835:i32)
          n914 = Index Array(array=w1836, index (row) #1=w1835, index (col) #1=0 ("index (row)"), index (row) #2=w1835, index (col) #2=1 ("index (row)"), index (row) #3=w1835, index (col) #3=2 ("index (row)"), index (row) #4=w1835, index (col) #4=3 ("index (row)")) -> (element #1=w1829:bool, element #2=w1828:bool, element #3=w1827:bool, element #4=w1826:bool)
        }
        frame True {
          n915 = Index Array(array=w1842, index (row) #1=w1839, index (col) #1=0 ("index (row)"), index (row) #2=w1839, index (col) #2=1 ("index (row)"), index (row) #3=w1839, index (col) #3=2 ("index (row)"), index (row) #4=w1839, index (col) #4=3 ("index (row)")) -> (element #1=w1847:bool, element #2=w1846:bool, element #3=w1844:bool, element #4=w1843:bool)
        }
      }
      n916 = Bundle("TimeArray"=w1824, "DataArray"=w1820) -> (w1819:T31)  [unwired: 1 in]
      n917 = stacked-sequence {
        tunnel: w1823 -> [w1851 _ _ _]
        tunnel: [w1850 _ _ _] -> w1822
        tunnel: w1819 -> [w1849 w1859 w1867 w1875]
        tunnel: w1818 -> [_ w1858 _ _]
        tunnel: [_ w1857 _ _] -> w1817
        tunnel: [_ _ w1866 _] -> w1816
        tunnel: w1815 -> [_ _ w1865 _]
        tunnel: [_ _ _ w1874] -> w1814
        tunnel: w1813 -> [_ _ _ w1873]
        tunnel: w1810 -> [w1848 _ _ _]
        tunnel: w1809 -> [_ w1856 _ _]
        tunnel: w1808 -> [_ _ w1864 _]
        tunnel: w1807 -> [_ _ _ w1872]
        frame #0 {
          n918 = case shown="False" w1848 {
            tunnel: w1849 -> [_ w1853]
            tunnel: w1851 -> [w1852 w1855]
            tunnel: [w1852 w1854] -> w1850
            frame False {
            }
            frame True {
              n919 = Build Array (concatenate)(w1855, w1853) -> (w1854:T4)
            }
          }
        }
        frame #1 {
          n920 = case shown="True" w1856 {
            tunnel: [w1860 w1863] -> w1857
            tunnel: w1859 -> [_ w1862]
            tunnel: w1858 -> [w1860 w1861]
            frame False {
            }
            frame True {
              n921 = Build Array (concatenate)(w1861, w1862) -> (w1863:T4)
            }
          }
        }
        frame #2 {
          n922 = case shown="True" w1864 {
            tunnel: [w1868 w1871] -> w1866
            tunnel: w1867 -> [_ w1870]
            tunnel: w1865 -> [w1868 w1869]
            frame False {
            }
            frame True {
              n923 = Build Array (concatenate)(w1869, w1870) -> (w1871:T4)
            }
          }
        }
        frame #3 {
          n924 = case shown="True" w1872 {
            tunnel: [w1876 w1879] -> w1874
            tunnel: w1875 -> [_ w1878]
            tunnel: w1873 -> [w1876 w1877]
            frame False {
            }
            frame True {
              n925 = Build Array (concatenate)(w1877, w1878) -> (w1879:T4)
            }
          }
        }
      }
    }
    n926 = local read "Labels LSI336"() -> (w830:string[])
    n927 = Array Size(array=w830) -> (size(s)=w829:i32)
    n928 = local read "Plot selecter LSI336 \n     1      2     3     4"() -> (w838:bool[][])
    n929 = for {
      N: w829 -> [_]
      tunnel: w838 -> [w1737]
      shift-right: [w1731] -> w836
      shift-left: w837 -> [w1746]
      shift-right: [w1727] -> w835
      shift-left: w837 -> [w1744]
      shift-right: [w1728] -> w834
      shift-left: w837 -> [w1743]
      shift-right: [w1726] -> w833
      shift-left: w837 -> [w1742]
      tunnel: w798 -> [w1734]
      tunnel: w800 -> [w1732]
      i -> [w1735]
      n930 = Index Array(array=w1734, index (col)=w1735) -> (element=w1733:dbl[])  [unwired: 1 in]
      n931 = Index Array(array=w1737, index (row) #1=w1735, index (col) #1=0 ("index (row)"), index (row) #2=w1735, index (col) #2=1 ("index (row)"), index (row) #3=w1735, index (col) #3=2 ("index (row)"), index (row) #4=w1735, index (col) #4=3 ("index (row)")) -> (element #1=w1736:bool, element #2=w1730:bool, element #3=w1729:bool, element #4=w1725:bool)
      n932 = Bundle("TimeArray"=w1732, "DataArray"=w1733) -> (w1745:T31)  [unwired: 1 in]
      n933 = stacked-sequence {
        tunnel: w1746 -> [w1750 _ _ _]
        tunnel: [w1749 _ _ _] -> w1731
        tunnel: w1745 -> [w1748 w1758 w1766 w1774]
        tunnel: w1744 -> [_ w1757 _ _]
        tunnel: [_ w1756 _ _] -> w1727
        tunnel: [_ _ w1765 _] -> w1728
        tunnel: w1743 -> [_ _ w1764 _]
        tunnel: [_ _ _ w1773] -> w1726
        tunnel: w1742 -> [_ _ _ w1772]
        tunnel: w1736 -> [w1747 _ _ _]
        tunnel: w1730 -> [_ w1755 _ _]
        tunnel: w1729 -> [_ _ w1763 _]
        tunnel: w1725 -> [_ _ _ w1771]
        frame #0 {
          n934 = case shown="False" w1747 {
            tunnel: w1748 -> [_ w1752]
            tunnel: w1750 -> [w1751 w1754]
            tunnel: [w1751 w1753] -> w1749
            frame False {
            }
            frame True {
              n935 = Build Array (concatenate)(w1754, w1752) -> (w1753:T4)
            }
          }
        }
        frame #1 {
          n936 = case shown="True" w1755 {
            tunnel: [w1759 w1762] -> w1756
            tunnel: w1758 -> [_ w1760]
            tunnel: w1757 -> [w1759 w1761]
            frame False {
            }
            frame True {
              n937 = Build Array (concatenate)(w1761, w1760) -> (w1762:T4)
            }
          }
        }
        frame #2 {
          n938 = case shown="True" w1763 {
            tunnel: [w1767 w1770] -> w1765
            tunnel: w1766 -> [_ w1768]
            tunnel: w1764 -> [w1767 w1769]
            frame False {
            }
            frame True {
              n939 = Build Array (concatenate)(w1769, w1768) -> (w1770:T4)
            }
          }
        }
        frame #3 {
          n940 = case shown="True" w1771 {
            tunnel: [w1775 w1778] -> w1773
            tunnel: w1774 -> [_ w1776]
            tunnel: w1772 -> [w1775 w1777]
            frame False {
            }
            frame True {
              n941 = Build Array (concatenate)(w1777, w1776) -> (w1778:T4)
            }
          }
        }
      }
    }
    n942 = Array Size(array=w800) -> (size(s)=→"TimeArray Size (336)":i32)
    n943 = Array Size(array=w798) -> (size(s)=→"DataArray size (336)":i32[])
    n944 = Build Array (concatenate)(w850, w849, w834, w812) -> (→"Graph 3":T23)
    n945 = Build Array (concatenate)(w855, w856, w836, w814) -> (→"Graph 1":T23)
    n946 = Build Array (concatenate)(w853, w851, w835, w813) -> (→"Graph 2":T23)
    n947 = Build Array (concatenate)(w848, w847, w833, w811) -> (→"Graph 4":T23)
    n948 = Send Notification(notification="Stop Button", notifier=w772, error in (no error)=w771) -> (notifier out=w768:refnum<notifier>, error out=w769:errorcluster)
    "Cycle #" <- w781
  }
  n949 = while {
    shift-right: [w1973] -> w2
    shift-left: refnum<class "DMMsData.lvclass"> refnum ("DMMsData.lvclass") -> [w1972]
    shift-right: [w1971] -> w1
    shift-left: errorcluster {"status"=FALSE, "code"=0, "source"=""} ("error in (no error)") -> [w1964]
    tunnel: w7 -> [w1969]
    tunnel: w6 -> [w1968]
    tunnel: [w1967] -> w5
    i -> [w1970]
    stop <- w1966 stop-if-true
    n950 = Equal?(x=w1970, y=0) -> (x = y?=w1974:bool)
    n951 = Wait (ms)(milliseconds to wait="Measurement Interval DMMs (ms)") -> ()  [unwired: 1 out]
    n952 = case shown="True" "Measure DMMs?" {
      tunnel: w1974 -> [_ w1985]
      tunnel: [w1978 w1983] -> w1973
      tunnel: w1972 -> [w1978 w1982]
      tunnel: w1964 -> [w1977 w1981]
      tunnel: [w1977 w1980] -> w1971
      tunnel: w1970 -> [_ w1979]
      frame False {
      }
      frame True {
        n953 = Or(x="Initialize (DMMs)", y=w1985) -> (x .or. y?=w1984:bool)
        n954 = case shown="True" w1984 {
          tunnel: w1982 -> [w2008 w2044]
          tunnel: [w2005 w2043] -> w1983
          tunnel: w1981 -> [w2007 w2040]
          tunnel: [w2006 w2037] -> w1980
          tunnel: w1979 -> [w2004 _]
          frame False {
            n955 = local read "VariableSources"() -> (w1995:T11)
            n956 = for {
              tunnel: w1995 -> [w2011] mode=indexing
              tunnel: [w2010] -> w1994 mode=indexing
              tunnel: [w2009] -> w1993 mode=indexing
              n957 = case shown="\"LSI336\"" w2011 {
                tunnel: [w2013 w2015 w2017 w2018 w2024] -> w2010
                tunnel: [w2012 w2014 w2016 w2019 w2025] -> w2009
                frame "USB6210" {
                  n958 = local read "All Labels (USB6210)"() -> (w2013:string[])
                  n959 = local read "Last Data \n(USB6210)"() -> (w2012:dbl[])
                }
                frame "USB6218AI" {
                  n960 = local read "Last Data \n(USB6218)"() -> (w2014:dbl[])
                  n961 = local read "All Labels (USB6218)"() -> (w2015:string[])
                }
                frame "USB6218AO" {
                  n962 = local read "USB 6218 AOUT"() -> (w2016:dbl[])
                  n963 = local read "AOUT Labels"() -> (w2017:string[])
                }
                frame "LSI218" {
                  n964 = local read "Last Data \nLSI218 (2)"() -> (w2020:dbl[])
                  n965 = local read "Last Data \nLSI218 (1)"() -> (w2021:dbl[])
                  n966 = local read "Labels LSI218 (2)"() -> (w2023:string[])
                  n967 = local read "Labels LSI218 (1)"() -> (w2022:string[])
                  n968 = Build Array (concatenate)(w2021, w2020) -> (w2019:dbl[])
                  n969 = Build Array (concatenate)(w2022, w2023) -> (w2018:string[])
                }
                frame "LSI336" {
                  n970 = local read "Last Data \nLSI336"() -> (w2025:dbl[])
                  n971 = local read "Labels LSI336"() -> (w2024:string[])
                }
              }
            }
            n972 = local read "DMMsConfig"() -> (w2001:T13)
            n973 = call-dynamic "DMMs_measure.vi"("DMMsData in"=w2008, "Sample #"="Sample #", "MeasurementIndex"=w2004, "SourceDataLabels"=w1994, "error in (no error)"=w2007, "SourceDataArray"=w1993) -> ("TimeArray"=w2003:timestamp[], "DMMsData out"=w2005:refnum<class "DMMsData.lvclass">, "LastData"=w1990:dbl[], "DataArray"=w1999:dbl[][], "DeviceActive?"=→"Active?":bool[], "error out"=w2006:errorcluster)  [unwired: 4 in]
            "DMM LastMeasurements" <- w1990
            n974 = Array Size(array=w2001) -> (size(s)=w2000:i32)
            n975 = for {
              N: w2000 -> [_]
              tunnel: w2003 -> [w2028]
              tunnel: w1999 -> [w2032]
              shift-right: [w2026] -> w1997
              shift-left: T4 [] -> [w2027]
              i -> [w2031]
              n976 = Index Array(array=w2032, index (col)=w2031) -> (element=w2030:dbl[])  [unwired: 1 in]
              n977 = Bundle("TimeArray"=w2028, "DataArray"=w2030) -> (w2029:T31)  [unwired: 1 in]
              n978 = Build Array (concatenate)(w2027, w2029) -> (w2026:T4)
            }
            "Graph DMMs 2" <- w1997
            "Graph DMMs 1" <- w1997
            n979 = Index Array(array=w1990, index #1="index V", index #2="index I") -> (element #1=w1989:dbl, element #2=w1988:dbl)
            n980 = Multiply(x=w1989, y=w1988) -> (x*y=→"Power":dbl)
          }
          frame True {
            n981 = local write "Initialize (DMMs)"(FALSE ("Initialize 2")) -> ()
            n982 = local read "RUN Identifier"() -> (w2035:string)
            n983 = local read "Base Path"() -> (w2041:path)
            n984 = call-dynamic "DMMs_initialize.vi"("DMMsConfig (variables)"="DMMsConfig (variables)", "DMMsConfig"="DMMsConfig", "InstName"="InstName DMMs", "error in (no error)"=w2040, "base path"=w2041, "RunIdentifier"=w2035, "DMMsData in"=w2044) -> ("error out"=w2037:errorcluster, "DMMsLabels"=w2038:string[], "FileName"=→"DMMFileName":string, "DMMsData out"=w2043:refnum<class "DMMsData.lvclass">, "VariableSources"=→"VariableSources":T11)
            "DMMsLabels" <- w2038
            n985 = stacked-sequence {
              tunnel: w2038 -> [w2046 w2069]
              frame #0 {
                n986 = Array Size(array=w2046) -> (size(s)=w2055:i32)
                n987 = control-ref of="Graph DMMs 1"() -> (w2052:refnum<vi>)
                n988 = property class="XYGraph (strict)"(reference=w2052, error in=errorcluster {"status"=FALSE, "code"=0, "source"=""} ("error in (no error)")) -> (reference out=w2048:refnum<vi>, error out=w2051:errorcluster, "LegNumRows"=w2053:u32)
                n989 = for {
                  N: w2053 -> [_]
                  shift-right: [w2064] -> w2054
                  shift-left: w2051 -> [w2065]
                  tunnel: w2048 -> [w2063]
                  tunnel: [w2062] -> w2047 mode=indexing
                  i -> [w2067]
                  n990 = property class="XYGraph (strict)"(reference=w2063, error in=w2065, "Active Plot"=w2067, "Plot.Plot Name"="") -> (reference out=w2062:refnum<vi>, error out=w2064:errorcluster)
                }
                n991 = for {
                  N: w2055 -> [_]
                  shift-right: [w2059] -> w2049
                  shift-left: w2054 -> [w2060]
                  tunnel: w2047 -> [w2057] mode=indexing
                  tunnel: w2046 -> [w2056] mode=indexing
                  i -> [w2061]
                  n992 = property class="XYGraph (strict)"(reference=w2057, error in=w2060, "Active Plot"=w2061, "Plot.Plot Name"=w2056, "Plot.Visible?"=TRUE ("Plot.Visible")) -> (error out=w2059:errorcluster)  [unwired: 1 out]
                }
                "error out (DMM graphs)" <- w2049
              }
              frame #1 {
                n993 = Array Size(array=w2069) -> (size(s)=w2077:i32)
                n994 = control-ref of="Graph DMMs 2"() -> (w2072:refnum<vi>)
                n995 = property class="XYGraph (strict)"(reference=w2072, error in=errorcluster {"status"=FALSE, "code"=0, "source"=""} ("error in (no error)")) -> (reference out=w2071:refnum<vi>, error out=w2074:errorcluster, "LegNumRows"=w2075:u32)
                n996 = for {
                  N: w2075 -> [_]
                  shift-right: [w2086] -> w2076
                  shift-left: w2074 -> [w2087]
                  tunnel: w2071 -> [w2085]
                  tunnel: [w2084] -> w2070 mode=indexing
                  i -> [w2089]
                  n997 = property class="XYGraph (strict)"(reference=w2085, error in=w2087, "Active Plot"=w2089, "Plot.Plot Name"="") -> (reference out=w2084:refnum<vi>, error out=w2086:errorcluster)
                }
                n998 = for {
                  N: w2077 -> [_]
                  shift-right: [w2081] -> w2068
                  shift-left: w2076 -> [w2082]
                  tunnel: w2070 -> [w2079] mode=indexing
                  tunnel: w2069 -> [w2078] mode=indexing
                  i -> [w2083]
                  n999 = property class="XYGraph (strict)"(reference=w2079, error in=w2082, "Active Plot"=w2083, "Plot.Plot Name"=w2078, "Plot.Visible?"=TRUE ("Plot.Visible")) -> (error out=w2081:errorcluster)  [unwired: 1 out]
                }
                n1000 = local write "error out (DMM graphs)"(w2068) -> ()
              }
            }
          }
        }
        "error out (DMMs)" <- w1980
      }
    }
    n1001 = Get Notifier Status(notifier=w1969, error in (no error)=w1968) -> (current notification=w1966:bool, error out=w1967:errorcluster)  [unwired: 3 out]
    "cycle # (DMMs)" <- w1970
  }
  n1002 = call-dynamic "USBData_terminate.vi"("error in (no error)"=w20, "USBData in"=w21) -> ("error out"=w22:errorcluster)  [unwired: 8 in, 1 out]
  n1003 = local write "error out (USB6210)"(w22) -> ()
  n1004 = call-dynamic "DMMs_terminate.vi"("error in (no error)"=w1, "DMMsData in"=w2) -> ()  [unwired: 8 in, 2 out]
  n1005 = call-dynamic "USBData_terminate.vi"("error in (no error)"=w37, "USBData in"=w38) -> ("error out"=w39:errorcluster)  [unwired: 8 in, 1 out]
  n1006 = call-dynamic "LSI336Data_terminate.vi"("error in (no error)"=w27, "LSI336Data in"=w28) -> ("error out"=w26:errorcluster)  [unwired: 8 in, 1 out]
  n1007 = Merge Errors(w5, w9) -> (w10:errorcluster)
  n1008 = local write "error out (USB6210)"(w39) -> ()
  n1009 = local write "error out (LSI336)"(w26) -> ()
  n1010 = call "LSI218Data_terminate.vi"("error in (no error)"=w31, "LSI218Data in"=w32) -> ("error out"=w30:errorcluster)  [unwired: 8 in, 1 out]
  n1011 = Release Notifier(notifier=w8, error in (no error)=w10) -> (error out=→"error out (notifier)":errorcluster)  [unwired: 1 in, 2 out]
  n1012 = local write "error out (LSI218)"(w30) -> ()
